vi "UHR-Fleezers Control (host) - Mau_02.vi"() -> ()   [LabVIEW 2012]
uses:
  <vilib>/Utility/miscctls.llb/LVPoint32TypeDef.ctl
  <vilib>/Utility/miscctls.llb/LVMinMaxIncTypeDef.ctl
  <vilib>/userdefined/High Color/nirio_resource_hc.ctl
  <vilib>/Platform/TimedLoop/XDataNode/timing_clust.ctl
  <vilib>/Platform/TimedLoop/XDataNode/nitl_modes.ctl
  <vilib>/Platform/TimedLoop/XDataNode/wakeup.ctl
  <vilib>/FPGAPlugInAG/PCIe-7852R/niLvFpga_Open_PCIe-7852R.vi
  <vilib>/FPGAPlugInAG/PCIe-7852R/niLvFpga_Reset_PCIe-7852R.vi
  <vilib>/Utility/error.llb/Error Cluster From Error Code.vi
  <vilib>/rvi/errors/niLvFpgaAdjustHostInterfaceError.vi
  <vilib>/FPGAPlugInAG/PCIe-7852R/niLvFpga_Run_PCIe-7852R.vi
  <vilib>/Analysis/baseanly.llb/Mean (DBL).vi
  <vilib>/express/express analysis/Spectral/Block/exnSpectralBlock spectral measurements PSD poly.vi
  <vilib>/express/express analysis/Spectral/Block/exnSpectralBlock spectral measurements PSD WFM.vi
  <vilib>/Waveform/WDTOps.llb/WDT Append Waveforms DBL.vi
  <vilib>/FPGAPlugInAG/PCIe-7852R/niLvFpga_Abort_PCIe-7852R.vi
  <vilib>/FPGAPlugInAG/PCIe-7852R/niLvFpga_Close_PCIe-7852R.vi
  openfpgaref.8.6.ctl
  <vilib>/Platform/TimedLoop/XDataNode/XDataNode.xnode
  <vilib>/rvi/interface/nirviOpenFPGA/nirviOpenFPGA.xnode
  FPGA Bitfiles/UHR-FleezersInst_FPGATarget_UHR-FleezersCont_0F5B06C4.lvbitx
  UHR-Fleezers Control (fpga) - 10.3.vi
  <vilib>/rvi/interface/nirviMethod/nirviMethod.xnode
  <vilib>/rvi/interface/nirviReadWriteControl/nirviReadWriteControl.xnode
  <vilib>/express/express analysis/Spectral/XNode/ExpressSpectralMeasurementsBlockNode.xnode
  <vilib>/rvi/interface/nirviCloseFPGA/nirviCloseFPGA.xnode
  <vilib>/Analysis/NI_AALBase.lvlib
  <vilib>/Platform/TimedLoop/XDataNode/XDNodeRunTimeDep.lvlib
  <vilib>/vision/NI_Vision_Development_Module.lvlib
  NiFpgaLv.dll
  <vilib>/FPGAPlugInAG/PCIe-7852R/niLvFpga_ConfigureFifo_PCIe-7852R.vi
  <vilib>/rvi/errors/niLvFpgaMergeErrorWithErrorCode.vi
  <vilib>/FPGAPlugInAG/PCIe-7852R/niLvFpga_ReadFifo_PCIe-7852R.vi
panel:
  out "Location path":path=path "D:/UnifiedHighRes_VIs/Locations.txt"
  out "Location Matrix":string[][](array[string])=[["N.D.\r\n", "N.D.\r\n", "N.D.\r\n"], ["0.19233\r\n", "0.00156\r\n", "0.20615\r\n"], ["N.D.\r\n", "N.D.\r\n", "N.D.\r\n"], ["N.D.\r\n", "N.D.\r\n", "N.D.\r\n"]]
  in  "radius":i32=10 min=1 max=20
  in  "clear markers":bool
  in  "trap\nmarkers?":bool
  in  "Sample Channel Flow":bool
  in  "Pump 3 contents":string="Bottom: ADig beads" caption="contents"
  in  "Pump 1 contents":string="Top: DNA beads" caption="contents"
  in  "Scripts":T1(tab)
  in  "Take Stepping Data":bool
  in  "Got DNA bead":bool
  in  "Got ADig bead":bool
  in  "Cap 1 Flow ON":bool=TRUE
  in  "Move Cap. 1 (DNA Top)":bool
  in  "Cal/Data Acq. Spot":bool
  in  "Dump Beads":bool
  in  "Cap 1 T ON":bool=TRUE
  in  "Cap 1 Samp Flow ON":bool=TRUE
  in  "Offset 2 Set":dbl=2.0
  in  "Offset 1 Set":dbl=1.0
  in  "Cal @ (MHz)":dbl=20.0
  in  "W/ Offset 1":bool=TRUE
  in  "Offset 1 Start (MHz)":dbl=13.0
  in  "W/ Offset 2":bool
  in  "Offset 2 Start (MHz)":dbl=16.0
  in  "Pause at Closest Delta (s)":dbl
  in  "Move to Delta 2 (MHz)":dbl=41.0
  in  "Attempt Limit":dbl=30.0 caption="Limit"
  out "Attempts":dbl=1.0
  in  "Wait Before Save (s)":u32=1
  in  "Fish for Tether":bool
  in  "Closest Delta (MHz)":dbl=13.0 step=0.25
  in  "Stop F (pN)":dbl=10.0
  in  "Then...":string(combo)="2"
  in  "Move to Delta 1 (MHz)":dbl=15.0
  in  "Tether Alarm?":bool=TRUE
  out "Tether":bool
  in  "TA Cancel Save?":bool=TRUE
  in  "TA Green Off?":bool=TRUE
  in  "Raster Set Upon Tether":u32=1
  in  "Save at end (5, 6)":bool
  in  "N Steps":dbl=20.0
  in  "Step Size (nm)":dbl=0.34
  in  "Save ave factor":dbl=1.0
  in  "Dip Trap Delta 1 (MHz)":dbl=15.0
  in  "Move Trap Before?":bool
  in  "Save Data After?":bool
  in  "Green ON After?":bool
  in  "Dip Trap Delta 2 (MHz)":dbl=15.0
  in  "Move Trap After?":bool
  in  "Duration (s)":dbl=1.0
  in  "Dip for Protein":bool
  in  "APD to Watch":bool
  out "Duration (s)":dbl
  in  "Action":string(combo)="Yank"
  in  "Fl. Triggered...":bool
  in  "Fl. Delta Thresh. (kHz)":dbl=0.6
  out "Waiting":bool
  out "Fl. High":bool
  in  "N pts to average":u16=6
  in  "Yank Delay (s)":dbl=3.5
  in  "Yank to Delta Array (MHz)":dbl[](array[numeric])=[16.3, 15.85, 14.85]
  in  "N Array El":u8=3 min=1 step=1
  in  "Random Choice":bool=TRUE
  in  "Force Yank":bool
  in  "Force Reset":bool
  in  "Y change (mm)":dbl
  in  "Profile":bool
  out "Sigma/Mean 2":dbl=nan caption="Sigma/Mean" format="%#_2g"
  out "Rate sigma (Hz) 2":dbl caption="Sigma (Hz)" format="%0.2f"
  out "APD 2 Rate (Hz)":dbl format="%#_3p"
  out "Primary Video Display":T2(plugin-control)
  out "Waveform Graph":dbl[](graph) caption="APD Line Scan"
  in  "Inject Top":bool caption="Inject Pump 3"
  in  "Inject Bottom":bool caption="Inject Pump 1"
  out "Messages":string="7:59 AM\tUHR-Fleezers ready.\r"
  in  "APD Ave N":dbl=10.0
  out "Int. Time (s)":dbl=3.0
  in  "Stop All":bool=TRUE
  out "Sigma/Mean":dbl=nan format="%#_2g"
  out "Rate sigma (Hz)":dbl caption="Sigma (Hz)" format="%0.2f"
  in  "Tab Control 6":T3(tab)=enum."Imaging"
  in  "APD 2 Offset":dbl
  in  "APD 1 Offset":dbl
  out "RMS (Ang)":dbl=nan format="%_2g"
  in  "Bead Sep. Int. Time (s)":dbl=5.0 caption="Int. Time (s)"
  in  "Below (kHz)":dbl=0.5
  in  "Above (kHz)":dbl=2.0
  in  "Adjust Scale\nto Mean":bool
  in  "Rescale on Mean":bool
  in  "Offset (nm)":dbl
  out "Mean":dbl=nan caption="Mean (V)" format="%#_3g"
  out "Force":waveform(dbl)[](graph)=[{"t0"=timestamp(12.90000000000001 s since 1904-01-01), "dt"=0.15, "Y"=[nan, nan], "attributes"=variant("NI_ChannelName"=variant(string "T1 X"))}, {"t0"=timestamp(12.90000000000001 s since 1904-01-01), "dt"=0.15, "Y"=[nan, nan], "attributes"=variant("NI_ChannelName"=variant(string "T2 X"))}]
  out "APD Chart":waveform(dbl)[](graph)=[{"t0"=timestamp(12.90000000000001 s since 1904-01-01), "dt"=0.02, "Y"=[0.0, 0.0, 0.0, 0.0, 0.0, 0.0, 0.0, 0.0, 0.0, 0.0, 0.0, 0.0, 0.0, 0.0, 0.0], "attributes"=variant("NI_ChannelName"=variant(string "APD 1"))}, {"t0"=timestamp(12.90000000000001 s since 1904-01-01), "dt"=0.02, "Y"=[0.0, 0.0, 0.0, 0.0, 0.0, 0.0, 0.0, 0.0, 0.0, 0.0, 0.0, 0.0, 0.0, 0.0, 0.0], "attributes"=variant("NI_ChannelName"=variant(string "APD 2"))}]
  in  "Calibration":u16(ring) items=["None", "Position", "Force"]
  out "T1 X":dbl=nan caption="T1 X (V)" format="%0.2f"
  out "T2 X":dbl=nan caption="T2 X (V)" format="%0.2f"
  out "Bead Separation":waveform(dbl)(graph)={"t0"=timestamp(12.90000000000001 s since 1904-01-01), "dt"=0.15, "Y"=[nan, nan], "attributes"=variant("NI_ChannelName"=variant(string "T1 X"))}
  in  "Amplitude (nm)":dbl=3.0
  out "Bead Mean (nm)":dbl=nan caption="Mean (nm)" format="%0.2f"
  out "Difference":dbl=nan caption="Difference (V)" format="%.2g"
  in  "Take Detection Laser\nImage":bool
  out "APD 2":T2(plugin-control) caption="APD 2 (Cy5)"
  in  "Flip Green Filter":bool
  in  "Set X Only":bool
  in  "Set Y Only":bool
  out "APD 1":T2(plugin-control) caption="APD 1 (Cy3)"
  out "Detection Laser Y":T2(plugin-control)
  out "Pointer Y (V)":dbl format="%_3g"
  out "Pointer X (V)":dbl format="%_3g"
  in  "Set Confocal Spot (X-Y)":bool
  out "Detection Laser X":T2(plugin-control)
  out "Saved APD":dbl[][](graph) caption="Most Recent Time Trace"
  out "Trap Delta Graph":dbl[](graph) caption="Most Recent Time Trace"
  out "Save APD Deriv":dbl[][](graph) caption="Most Recent Time Trace"
  out "Delta Fl. 1":dbl
  out "Delta Fl. 2":dbl
  out "All Signals":waveform(dbl)[](graph)=[{"t0"=timestamp(12.90000000000001 s since 1904-01-01), "dt"=0.02, "Y"=[0.0, 0.0, 0.0, 0.0, 0.0, 0.0, 0.0, 0.0, 0.0, 0.0, 0.0, 0.0, 0.0, 0.0, 0.0], "attributes"=variant("NI_ChannelName"=variant(string "APD 1"))}, {"t0"=timestamp(12.90000000000001 s since 1904-01-01), "dt"=0.02, "Y"=[0.0, 0.0, 0.0, 0.0, 0.0, 0.0, 0.0, 0.0, 0.0, 0.0, 0.0, 0.0, 0.0, 0.0, 0.0], "attributes"=variant("NI_ChannelName"=variant(string "APD 2"))}, {"t0"=timestamp(12.90000000000001 s since 1904-01-01), "dt"=0.15, "Y"=[nan, nan], "attributes"=variant("NI_ChannelName"=variant(string "T1 Y"))}, {"t0"=timestamp(12.90000000000001 s since 1904-01-01), "dt"=0.15, "Y"=[nan, nan], "attributes"=variant("NI_ChannelName"=variant(string "T1 X"))}, {"t0"=timestamp(12.90000000000001 s since 1904-01-01), "dt"=0.15, "Y"=[-0.0004235663930173644, -0.0004722739341410556], "attributes"=variant("NI_ChannelName"=variant(string "T1 Sum"))}, {"t0"=timestamp(12.90000000000001 s since 1904-01-01), "dt"=0.15, "Y"=[nan, nan], "attributes"=variant("NI_ChannelName"=variant(string "T2 Y"))}, {"t0"=timestamp(12.90000000000001 s since 1904-01-01), "dt"=0.15, "Y"=[nan, nan], "attributes"=variant("NI_ChannelName"=variant(string "T2 X"))}, {"t0"=timestamp(12.90000000000001 s since 1904-01-01), "dt"=0.15, "Y"=[-0.0005883053071687949, -0.0006281319620349712], "attributes"=variant("NI_ChannelName"=variant(string "T2 Sum"))}, {"t0"=timestamp(12.90000000000001 s since 1904-01-01), "dt"=0.15, "Y"=[nan, nan], "attributes"=variant("NI_ChannelName"=variant(string "T1 FB X"))}, {"t0"=timestamp(12.90000000000001 s since 1904-01-01), "dt"=0.15, "Y"=[-0.0004680013428144157, -0.0005167699209570592], "attributes"=variant("NI_ChannelName"=variant(string "T2 FB Sum"))}, {"t0"=timestamp(12.90000000000001 s since 1904-01-01), "dt"=0.15, "Y"=[nan, nan], "attributes"=variant("NI_ChannelName"=variant(string "T2 FB X"))}, {"t0"=timestamp(12.90000000000001 s since 1904-01-01), "dt"=0.15, "Y"=[-0.0006226691488387671, -0.0006504715109714008], "attributes"=variant("NI_ChannelName"=variant(string "T2 FB Sum"))}, {"t0"=timestamp(12.90000000000001 s since 1904-01-01), "dt"=0.15, "Y"=[-0.0007901852473525123, -0.0008601641895809732], "attributes"=variant("NI_ChannelName"=variant(string "PSD Y"))}, {"t0"=timestamp(12.90000000000001 s since 1904-01-01), "dt"=0.15, "Y"=[0.00031556138798181086, 0.0002525101474044007], "attributes"=variant("NI_ChannelName"=variant(string "PSD X"))}, {"t0"=timestamp(12.90000000000001 s since 1904-01-01), "dt"=0.15, "Y"=[-0.00019678334910122974, -0.0002453993346964931], "attributes"=variant("NI_ChannelName"=variant(string "PSD Sum"))}]
  in  "Signals to Plot":i32(listbox)
  out "Trap Disp. Freq. (Hz)":dbl=6.666666666666667 caption="Freq. (Hz)" format="%#_6p"
  out "Display Period (s)":dbl=0.15 caption="Period (s)" format="%#_6p"
  in  "Trap Disp. Downsample":dbl=10000.0 caption="Downsample" max=20000.0
  in  "APD Disp. Scale":dbl=0.1 caption="Scale (Divide,\nfor above plot only)"
  in  "APD Disp. Downsample":dbl=2.0 caption="Integrate" min=1.0 max=30.0 step=1.0
  out "APD Display Freq. (Hz)":dbl=50.0 caption="Freq. (Hz)"
  out "APD Display Period (s)":dbl=0.02 caption="Period (s)"
  out "FFT 1":cluster{"f0":dbl, "df":dbl, "magnitude":dbl[]}[](graph)=[{"f0"=0.0, "df"=16.666666666666668, "magnitude"=[-331.1367572010275, -79.05506245821404, -86.61411242440559, -88.4728176091699, -90.3181253945935, -94.12566333707997, -92.52740723119955, -94.92192587982518, -99.60936585245742, -96.87568627870715, -94.02570383337763, -83.8058550151726, -97.57441397235512, -101.59968530846606, -101.523049255742, -103.35038532190343, -101.58594091014982, -102.96098031851216, -91.39759462745924, -103.75019963279499, -104.45030075054324, -103.04245334279298, -104.0720279134107, -106.06482372394834, -103.69131867828104, -104.40395035115309, -105.96420043276396, -107.6735556337804, -106.673030006608, -107.34889066208132, -108.05626565233933, -106.25659018850432, -105.29934513380842, -105.43096056709592, -108.3728498841465, -106.0555440144992, -105.78001282181421, -107.48741857324953, -108.67624970548897, -105.39976667156175, -105.91413119232612, -109.4222808198164, -107.0898971593174, -107.91164191890915, -108.26032038855709, -107.58332347164534, -108.23559688234297, -108.01271040303237, -107.66511723652701, -106.51901583170391, -109.27249501469946, -108.55647681594805, -107.93499259231463, -107.05068166453935, -109.13641475410455, -109.29679733781423, -108.19360835527803, -109.57747591546632, -109.58364591011674, -110.47061433372711, -109.8144340420426, -108.79067462293897, -107.54887553357234, -107.99559866705923, -108.85023923652685, -109.68733225238618, -108.51101278437793, -108.51620475114115, -108.22212402200637, -104.63726950302143, -110.2989919678048, -107.61796444414897, -108.68882962798736, -104.79193983043893, -103.59504263746938, -93.64633660288543, -101.9191640501395, -105.73717393151816, -108.92572458793902, -107.43962662800902, -107.79595323081325, -107.0923101993207, -108.17603277205289, -107.87074270713183, -109.20899066381877, -108.61832060412445, -109.10072003106593, -105.76480632823524, -108.60877649218978, -109.67541158970121, -110.2286232768028, -109.84952155309578, -109.33772024076384, -109.95251642394683, -110.14777282585466, -109.13825677905699, -110.05989365698167, -109.39359990189426, -110.56255614635295, -109.66477183197163, -108.9397158528824, -110.26529907650465, -109.20049464984628, -108.20183857013548, -109.09752250184418, -108.00440442238454, -108.35465963524055, -111.16774134451799, -110.34812550238405, -108.94506763426756, -108.72845542102493, -109.41512344014713, -112.44661664432377, -110.35437330889101, -111.32939440655925, -109.42989530434981, -110.98084669076195, -111.92160561143541, -108.57755551751093, -111.40042616180912, -110.15284955891853, -112.21455132279115, -111.40787773511747, -108.82949641635288, -110.13442122547907, -111.42229298204664, -112.06314940885191, -110.6015308813694, -109.51144097251623, -111.15989713761475, -110.25535755335385, -109.65868178057926, -110.51649885452997, -109.77194745285269, -108.4234206864394, -109.50892632093968, -109.46471287444389, -107.92241289271415, -109.72283805386196, -108.63426821579918, -110.37316681536255, -111.09713996884652, -110.32903619589223, -105.32012665515045, -107.36858557554393, -108.00382215905725, -110.06430686942338, -108.81666625979916, -110.01277074453823, -110.94194741225512, -109.65934609082873, -107.80979136006962, -112.81333866824724, -111.61474300955487, -109.83998277184975, -109.45953946904639, -109.79640584952526, -108.19172301667324, -109.28894656674316, -107.61471301278785, -108.83814006090513, -109.08866847726084, -108.20250571862371, -107.96222236861584, -107.03811197900873, -108.93533000393974, -107.74482548035408, -110.79811544577694, -111.1387476496877, -107.42970105883512, -109.18442281176472, -108.73546184641192, -108.71800246690864, -108.51945944378063, -108.06825856571285, -107.27210712368412, -108.12304695877637, -107.84933283677306, -109.73682373154998, -109.32284761503395, -109.31328817453769, -106.68762108642842, -109.79203616876461, -109.9020278896408, -110.27080024357275, -108.54152101558762, -111.00464391726017, -112.42244020766577, -110.82707315747889, -111.00344011890857, -109.90461839395674, -109.42877207451863, -109.73549298167016, -111.67494793393293, -108.85799077901427, -108.5348443278263, -109.803781083881, -108.30644755543659, -108.5079527456017, -111.2055351312823, -108.53089994340155, -108.01739789012176, -108.70360662855235, -107.95873456794631, -109.58297170693093, -108.9372401694271, -110.15921663527153, -109.22399119911955, -110.89883651739237, -108.92840112258382, -110.0545300523626, -109.05961065387005, -109.45831398589371, -108.61239387653227, -110.13001256174265, -108.80060224137931, -109.46327400696283, -108.0177965824709, -109.29727944627197, -110.3237255895986, -109.03258262543821, -110.97880178489321, -109.70034895077919, -111.16405638194153, -109.17324451464711, -109.65698250854277, -108.96750235822178, -112.00534231585624, -108.69274607723942, -108.98110446396657, -108.40723795464795, -111.44459094807324, -111.74799245277113, -111.1601960491512, -108.92048232753773, -110.30506377784799, -111.33145973979093, -110.91850998672503, -110.33684985776448, -108.90206518366908, -109.28458878227542, -108.98773986023751, -110.85813863075646, -109.00041591105906, -110.84543686681204, -109.84382395806176, -109.69722434763266, -108.50915601095721, -107.80829925826895, -110.59736107582401, -109.75377770317087, -109.3992084496136, -110.51151565846742, -112.49753959826434, -109.7299632589479, -109.54070743868353, -109.90314341132164, -111.05974202976806, -109.03766862152392, -109.46667095459878, -109.52800799036197, -111.3163121356807, -110.07817134522178, -108.69251657453547, -109.40472158898045, -109.71400709815576, -110.60534468715097, -109.46937396724682, -107.70342491418788, -109.86331122597839, -108.64971387994616, -110.90117371097081, -108.34928840565928, -110.04172889660904, -111.52979926554961, -110.34759300823305, -109.62712781837159, -109.24131154553284, -110.23196152450447, -108.68509612326807, -108.0246905483419, -106.61876139289784, -101.5519630114271, -80.57695480953835, -102.03744443354402, -107.1449217193017, -110.0695213407169, -106.61597783999268, -110.79221011808191, -109.58974545931426, -109.1149802216988, -109.20993813088597, -109.63768480465863, -110.10428394219181, -109.08445084271477, -108.83472375362581, -109.69508502050168, -108.05588796178941, -110.62586360101581, -109.95315261676905, -107.52208264977473, -108.80708007514875, -110.43484881098874, -110.45942171588936, -107.83804717866751, -109.98973910294193, -109.3496496054193, -108.425252911127, -110.94579264380809, -108.54181722177951, -108.67696070083541, -108.4150202151644, -109.24973583101504, -112.0454922608961, -111.29046597340738, -110.75018248960077, -109.38326363603683, -109.2033340336957, -109.45076170874889, -109.52878049853727, -109.32340869724774, -110.98123395128233, -110.75736340635505, -109.7218385823809, -107.97422606064993, -109.77313701758703, -110.95948744392717, -110.08996774172691, -108.51011830110778, -109.78063140243836, -110.65996628628228, -109.83684298615616, -110.33329049188029, -110.13755118968292, -110.3717925645783, -108.55302219178951, -106.86811628734195, -108.6302156589162, -108.75341391045045, -108.32589578384841, -108.70061474734084, -112.30742263527534, -109.16842570592085, -109.29767035534508, -108.87829025017463, -108.2255616391397, -108.4316108616088, -108.82995906929271, -110.40135575415563, -109.51623498946435, -109.79409808792403, -107.03832759632121, -108.36534528684132, -109.72010868372905, -107.90933028179892, -106.95643597294047, -111.29929166165778, -110.23001135794706, -108.98838015381585, -109.79115357104436, -108.18627479511115, -108.14988122174307, -109.12074063466532, -109.41904850488358, -111.40409873721113, -108.83156790193294, -108.77032248953847, -108.88363158686694, -108.47515048290681, -105.94172147874599, -109.38146940214403, -109.21277078848794, -108.11309390545507, -110.70840012427504, -109.5504457849329, -109.52330684534209, -110.06776026911132, -108.21949434182314, -111.21266686269992, -108.78581501170974, -108.43115799297222, -109.63260325780062, -109.84070220619535, -109.72041980780126, -110.29615941882527, -110.60316734262464, -108.79165446414692, -110.95840439895592, -109.64926233107009, -109.16526769544322, -108.65292362430982, -109.56113898129935, -109.85693046339026, -108.92316027325207, -109.79492493553914, -109.38157962945887, -110.24545136266825, -109.30031463492487, -109.0795429936869, -111.4091719525013, -108.63499083917162, -108.43863465339358, -109.23207864880891, -111.21947487191643, -109.24525201480154, -109.56842406077318, -109.46711940800672, -111.91389548262572, -108.15655736690546, -108.71882059966947, -111.26328503478568, -110.95027143873176, -108.4853106242357, -110.36902802777546, -109.9314203579182, -108.77686164101732, -108.71871020068312, -111.04829661168574, -109.95072655339462, -109.88221342875462, -109.53241732756136, -108.2625005404823, -108.00677030040697, -110.19659317581693, -108.93858924796267, -109.46817875483995, -110.78063992017232, -111.11066570318451, -110.78774336696706, -109.19199744617812, -108.54914256407436, -109.28414960420909, -110.64143585101183, -110.5855350821307, -109.47578632252726, -108.89705360836223, -109.89214013612292, -107.93271261027171, -109.32631601340563, -108.60274611341092, -109.40110159872573, -110.889237682208, -110.01391165813328, -109.99747108785071, -108.65542819213674, -110.37211847668736, -110.44656500845738, -110.8128133834973, -108.8909299260433, -110.19551227077532, -111.37647266643523, -110.83802189730321, -109.98519377913681, -110.52378970770522, -108.16970420057817, -110.70974729773344, -110.76836765494402, -110.26884275594577, -109.22041044268806, -109.87809744746195, -107.76823252107832, -109.12119474042969, -110.28066108731146, -108.55000033509207, -110.18152097767907, -110.73030521152278, -111.49470908029893, -110.2320929919509, -110.03370979233021, -109.79181668155233, -108.6673501209991, -109.86695766650877, -107.88926518046961, -110.95525003776572, -109.18130359755742, -110.42618009658618, -107.90341931158893, -111.44736855661769, -110.72634267386593, -109.29945988519303, -107.67889101961411, -108.81148059987765, -109.13375212757057, -109.8122873383549, -109.80176697684155, -109.96342275204768, -109.90406635707086, -108.75674342748256, -110.12362902701081, -109.82151095527837, -108.62543344241836, -110.09171852771195, -110.21434637862887, -109.97254504855631, -109.27043209093468, -111.35149588204125, -110.12399876776051, -111.65983675538546, -109.28788875768564, -110.86554069990251, -111.26990906470603, -108.60956517491746, -111.49613890850938, -111.79685722966795, -109.26269485364045, -110.38555615546439, -109.40641023162068, -110.966136593156, -108.78892524584494, -110.29340727375603, -111.44032043281035, -109.95212021173755, -109.79233511584334, -112.41184021118175, -109.73687851881148, -108.65493879781806, -110.76132988919045, -108.43230346094671, -110.32968175895853, -110.29890782023821, -108.77609076424456, -110.3298662333555, -109.47734504217333, -108.2677295732245, -109.21234363352882, -107.83278941978479, -108.85136784424789, -108.43241251530755, -109.76609391460555, -108.53204373005357, -110.9660641972934, -110.3152512161094, -110.72570499399905, -109.23877906286317, -111.72407743101837, -109.20311421918561, -108.06021800233717, -109.29288625761943, -108.78395253409145, -111.85250172876302, -108.78827588901797, -109.79775055719482, -109.12089297455859, -109.49896359356035, -110.34432647103819, -107.94700097960238, -109.30489238477631, -108.89170290869342, -108.82574563272509, -110.11024077194833, -107.37946433552314, -109.60167933458756, -107.80625057819019, -110.11489057210264, -107.35436859378505, -105.69819484613895, -109.11280625683739, -109.27770293057978, -107.7053735252589, -109.75022444894368, -109.3310543596577, -107.87683693707739, -108.19931495338068, -109.26462246191564, -106.71885779297867, -100.00018022217961, -92.54434511397295, -107.20472143807373, -107.39203415155283, -110.04461177268398, -108.48860496315312, -109.0057168110333, -108.37627790492552, -108.4108380728248, -109.65509454313073, -109.64243000632982, -97.04219069306761, -109.0928856629964, -107.9760697315632, -107.52611064047497, -108.87702814778996, -109.08437599027614, -110.70097118837974, -109.00969860961283, -110.38275386163214, -110.0699155421545, -106.91498895181175, -106.22178738309017, -109.36827866896039, -107.59953130968307, -109.19516217272808, -108.31502495393616, -109.384158926223, -107.11670654202719, -108.09436312738853, -110.14559230873704, -109.84997663447679, -107.83465335309926, -108.60947100624459, -108.9932479423645, -109.17174810371898, -108.79457339828916, -109.40909327982367, -109.6328723628302, -109.51081854476179, -107.63054408568418, -109.63728404010122, -108.51163794839918, -107.55002282725216, -108.97796212764939, -107.24648164623483, -112.21470452291085, -108.74294024554423, -109.62070777514892, -108.05768666239368, -109.8224946685739, -109.34575507446003, -108.53536952609525, -109.60789300457671, -107.56681538208278, -109.22777325016398, -108.79047910308894, -110.10332477250668, -108.00206387955672, -108.45604004720035, -109.00645795765472, -109.81039564269616, -108.92785144634745, -108.3978471520567, -107.94411095685999, -110.53486519304262, -108.8773780319227, -109.03345093296107, -107.30746693745031, -108.54277704832029, -108.77629108166091, -108.91111762599647, -107.74965195880401, -109.97375370738439, -109.76326492689246, -107.91717581777407, -109.0730556927617, -107.66804873204664, -110.40438871064791, -108.05794247751498, -108.80206615156494, -107.51329354700796, -108.83687012994949, -107.57713176895379, -107.94774159581414, -109.41894615439651, -107.10869425078764, -110.51480854078629, -108.92221367099775, -109.91358786461535, -110.1744263092835, -109.30795472883494, -107.91359710691006, -109.77888185049835, -109.52060975706438, -108.66686651982212, -108.71041801553639, -110.13619546359467, -108.87957097273856, -109.72150387215271, -109.00776068810654, -109.70251113927438, -110.75769213896399, -108.53234896741436, -109.69439526582246, -110.15412541604617, -108.25183374628219, -107.97402569656481, -110.34920156998648, -108.45106995186384, -108.82031145748209, -111.38690005057539, -107.01968459818563, -110.3044500039584, -110.8755481852125, -111.08915057663255, -107.94824988655199, -110.21669144934839, -109.90539774633154, -109.58985438756767, -110.12258796623348, -109.41689951612143, -109.31128210476795, -109.00258476567323, -109.11093063041056, -108.83347064311234, -108.32685287566952, -109.44770946560935, -108.40145063144861, -109.68448193892085, -108.76525439243828, -107.62837139034596, -107.39300298848994, -109.36993934990318, -109.2465218489418, -106.66307369796812, -110.15891092764934, -109.57151745419041, -108.92425698310808, -109.8036704717834, -108.79751146756549, -109.25926431818017, -108.46260574057584, -109.1967554647261, -110.63319560262356, -109.02343067385144, -111.22073171487528, -109.4731095097105, -109.69335000085164, -109.48782989577005, -107.95204227683271, -108.19468255763758, -111.36195112053247, -109.55696116543685, -110.3130767640534, -108.9621824253354, -109.99735074896789, -109.20198058456344, -108.12100614259485, -111.27227490807289, -110.09248554008288, -109.14395535060149, -110.80882692379708, -109.22632926901655, -108.64497210802793, -111.00030482190711, -111.1317849358033, -107.43140429257826, -107.9783302193555, -109.2639893652291, -108.97008485446163, -108.66556668859064, -108.12995785876932, -109.73001061107855, -108.09691302413727, -110.68391499215569, -112.78583642012705, -108.7093037763389, -110.67868795924797, -109.0190959349128, -108.36247198231372, -109.82829353258869, -108.24916379311045, -109.84154533905823, -108.55470160833775, -109.75438989348815, -108.82865632118325, -107.63622268162582, -111.00943492886312, -110.81824358463759, -109.46028423652966, -107.52479398900992, -108.99087806823736, -109.94494831750349, -110.26788355564504, -109.8954055022304, -106.9478122391182, -108.91705388158901, -107.76095584490312, -109.28456723055147, -109.7982307261767, -108.98552661346622, -109.98937979783426, -110.57907422426224, -108.68113463944836, -108.06257240208589, -110.0707224529617, -109.19515280354733, -109.35868842818849, -110.37311467065695, -109.0404734478992, -108.16686395270187, -108.61859220485148, -109.19986437876149, -108.19707189725302, -110.06564239663074, -108.87850403465154, -110.63824157544798, -107.36918104067212, -108.7008736325543, -110.9359398265406, -111.08529123080929, -108.44209934821818, -109.79529621208783, -108.38917887958179, -108.169117639508, -109.24332926356216, -110.50584058811704, -109.63592524002665, -109.32261039377495, -109.16720880524552, -109.3084314664462, -109.5812223978583, -107.70213196487856, -108.0557884982431, -110.67058020007828, -111.68459781023608, -109.66270627185824, -110.52536245663693, -109.70208409132103, -108.78645420809342, -109.23122088059863, -109.24601474121832, -111.25604763816514, -109.50225851581177, -107.32434217163818, -109.28548556764925, -107.59972621660836, -110.46928774723048, -109.25950101547609, -110.32016453935465, -107.78482761561703, -107.89462895091089, -107.51366154391481, -108.08036891159172, -109.53371809947035, -101.2452927166745, -109.32763325689056, -107.52166868423687, -109.89648659445174, -109.11350200980485, -109.81336712738089, -110.02799517445062, -108.02767143538516, -107.97850220501483, -109.50772934896838, -109.31069875721964, -108.49991657749598, -105.60880911233095, -109.79128597340213, -106.91084537903113, -107.84880087118997, -109.63628170511824, -109.03203967193224, -110.64186113413658, -110.98027990365594, -112.33841002907062, -111.01793075565425, -108.58025797022215, -110.4259296883756, -110.38643255981424, -108.93051671115133, -110.97544177116494, -108.63883100482677, -108.37581711765226, -108.90240163126536, -107.94688047875466, -109.9482937437732, -110.09097112364414, -110.09805032265376, -111.44307114024532, -109.15483789122554, -110.9713708217832, -107.8548737634672, -111.41418477109195, -109.45699779859628, -97.03595099331734, -109.16746744169623, -109.66209204485918, -112.57048704774604, -109.73989735035725, -108.16252575067017, -110.7546980664636, -108.91536673403449, -109.20509151422344, -111.0260632167785, -109.62924582406518, -110.45466277291722, -110.2973970018937, -109.67550222925419, -108.84481022020094, -107.23686414357573, -111.79004633370906, -109.85453094194085, -109.45617270081004, -110.73920606732504, -108.90879956851099, -109.67774425528265, -109.4745715721361, -110.18080454693559, -109.26079184315502, -109.41692499885505, -109.02240975088358, -107.80833423058168, -109.32657361431549, -107.87138278655101, -110.910364670719, -109.70067156846706, -108.55301754282077, -109.4243252157005, -109.77567725161107, -107.83737232063925, -110.36509412773016, -109.6371048811367, -109.49430894422814, -108.55509251499753, -108.03996302911446, -110.4385715838736, -110.08864436068788, -109.48922484379962, -109.90865554258562, -109.7491963238264, -110.04796094537969, -107.413043439116, -108.54229076126079, -108.2522516728666, -109.75464941327974, -110.26795832300996, -109.28073673851144, -108.62990200974927, -109.89408067552287, -109.09160284731726, -109.90740624925795, -109.92534708896517, -109.79578862362752, -109.97278346890566, -107.80679350393824, -112.81728446281548, -108.09689504419987, -109.89549991422173, -108.43930976031248, -109.95153099843282, -108.18277483720716, -111.89607792605433, -109.52567003805, -109.17125106979698, -109.64300739407085, -108.21045178846524, -109.64036472149706, -109.02324448538845, -109.039163008889, -110.41006510134076, -109.50289952116489, -110.4732620447796, -110.08777181504614, -110.15589511434341, -109.55705089158471, -109.2547682932589, -110.86823885471617, -109.96330502176939, -109.85995369810554, -110.63211290903473, -112.08007783432191, -110.24725218052279, -107.62861148917592, -110.08691795849435, -108.89793794632287, -111.07702220466341, -109.46946126482341, -109.19747345337464, -110.70018609416007, -109.66366205691908, -110.78032312133551, -108.05724200456513, -108.195661625627, -110.90724508408255, -110.08307674771669, -110.76863516643007, -110.46620425061583, -109.16986788877276, -109.61921294239114, -108.51159432329543, -109.96308336765689, -107.38178944242856, -111.95930944846394, -109.3329826827624, -109.59119636368249, -108.83148571828912, -110.46194288788257, -105.87694286145472, -107.985886302892, -109.2975019660806, -111.05138725716857, -109.60005889204612, -110.92871351729086, -110.73480546964537, -108.41587420326718, -109.84275465824477, -108.8249071047676, -107.65358887817105, -108.3254150042995, -111.47362100321767, -112.7287536850025, -108.8217125660507, -109.50232320231771, -110.29587061625348, -109.30644535112089, -107.69178032077258, -110.84522325672016, -109.3735891463141, -109.12506388923123, -109.65582307934665, -111.11427272192576, -112.19827973435466, -109.11306367925813, -108.19203577968261, -107.89831568266465, -108.85805249169313, -109.51100049661844, -111.71546684086955, -109.53880495724334, -107.07739286222231, -110.66836728754211, -111.5415170557177, -110.16051267940297, -110.6107546662698, -111.36389129556191, -107.77888179117923, -110.34160392509817, -109.61287125994414, -110.23791773883013, -111.00669159903549, -110.97165069538953, -109.43965413392434, -110.6813161690388, -110.31441293654314, -111.96129906273796, -108.15998218707462, -110.08095912053633, -109.41084567452768, -109.28774416263552, -110.80159950384204, -110.41956747809755, -108.85005186267244, -107.9069227847757, -108.84249369063123, -109.92569208845894, -109.34109797584448, -109.41334788055491, -108.76462023086997, -108.22069272136177, -107.0786679601274, -108.30206755098202, -108.57613406368954, -110.83330887636482, -111.93966942736989, -109.76373713473264, -108.25782074884941, -108.16490627215555, -109.93351470267982, -110.75525684428368, -108.22814762283093, -109.73442331991602, -107.53145627482685, -108.27195221226805, -110.33032779278457, -109.48951857415828, -108.12599093700939, -107.97627415508097, -108.81426859968796, -111.21764717894752, -109.80856212352333, -110.92658779118501, -109.71551885834796, -110.38682741010847, -108.87671328341361, -109.68368600774755, -108.35359806351899, -111.7519400010676, -109.89407081573103, -108.24301180922755, -110.00646944788126, -108.6685299083706, -107.52856885980722, -111.7622363038509, -111.0025144494897, -108.64719599357296, -110.62968467177518, -108.821509935539, -107.94915453463719, -111.53070432277694, -109.87282048586256, -110.71167589371663, -109.79225006081626, -109.96203471712074, -110.29921092232489, -110.10644439440416, -111.28815007382043, -111.19165661703703, -108.46024117100558, -110.22528296512183, -110.32184972386672, -110.05120383416072, -109.78792549362107, -109.00355659956696, -108.85989369286315, -113.00899556732638, -110.91756826567867, -111.25016866167897, -111.84225040552181, -110.54451635944174, -110.72722829912917, -109.60759702177283, -110.49362602516815, -108.74419542915284, -110.3379671069179, -109.66259088220754, -110.45956400953156, -109.13956157147233, -109.27130155486806, -110.83015602667983, -109.17970724944131, -109.09662765889193, -108.0447366108107, -108.9536269357457, -110.35663108940085, -108.73418835472056, -113.42965806805827, -111.81270536656905, -110.06155590173537, -108.76582224646269, -106.7488061675813, -108.5700320158723, -111.11038264410035, -110.41435767488723, -109.12763443489911, -109.30517580756394, -111.61251165371237, -109.8116632664339, -109.36845864976851, -109.00390009629231, -110.54359197165573, -109.52629258465976, -110.75932197632896, -109.50903215359567, -107.42652056246085, -107.81146496533543, -103.22224383145215, -108.53803076819163, -109.78623360072066, -109.66306634612869, -110.80245829141279, -111.87835085452016, -102.27372781471168, -111.27763038431458, -108.45838423437681, -108.79077917058028, -109.31951755762685, -110.05415097017186, -109.5535934823387, -111.62732254641111, -110.73478247119641, -109.9468722686683, -110.39698367573979, -109.30612942398305, -109.7578384694043, -109.34817295524313, -105.56944757301993, -110.1940418750125, -109.27076023513962, -111.03491935225027, -112.2980497521063, -110.65725497955563, -109.0567530102422, -110.31700596563523, -109.64508026365678, -109.6190471404421, -110.52566833759428, -109.68595899227789, -109.7431160985074, -110.4798230300751, -109.45506977604765, -110.69504157940786, -110.63067849573177, -108.06456949500138, -107.99354148885966, -108.11349194720599, -109.15944121207349, -110.61766925164031, -110.14145801314527, -110.67420842201165, -111.91532881806512, -112.15901550030345, -109.94774413630104, -109.2819568305201, -110.94623189179737, -110.17685430287735, -110.39082916961016, -109.53953238698966, -110.76940623620611, -109.89327922318515, -109.10275695043765, -110.21445972656734, -110.58968777252528, -110.57016757660259, -109.59208496373341, -109.07946946465374, -109.10762003745964, -110.36892993974607, -109.81864495218393, -112.12972189864566, -109.26185849434863, -111.56305819991357, -111.36019621828058, -110.3397604159226, -109.58675612753163, -110.58041217474447, -106.34739062044932, -108.6722699609389, -110.03906060709869, -109.16794717548382, -109.65012481802809, -109.35377624077988, -110.51889143862303, -110.03397458059777, -110.7981307056636, -110.56653507062292, -107.61367005067231, -109.99279736988825, -111.79875182878175, -108.60382315996031, -109.71381533228038, -108.60388131505613, -107.0933685540362, -107.86037690830757, -108.40980028847238, -108.83869602763895, -110.76921375395764, -109.96766364716046, -110.8256171465781, -110.13805084291067, -108.5349140035878, -110.57158437465219, -110.8920694413417, -108.71646695477324, -108.33274238445665, -108.96152108305608, -111.03750932994224, -109.48915027983756, -110.29725207211165, -110.79527247268442, -109.47969936716117, -109.79306701834035, -110.16840035577498, -110.29840230783668, -109.15306387075587, -110.72651274964761, -109.08881658764956, -110.8349724030761, -110.64653625576447, -111.40392562616867, -109.94581588927414, -108.85136340231294, -109.77228546607624, -111.48297395390018, -109.7334001251941, -109.30537415590783, -109.63937411233408, -109.69785848648013, -109.3523781030017, -112.04667421182404, -111.56311816195343, -108.18548447362308, -110.63388993686104, -111.39768634137992, -109.87157345395542, -108.6734208287271, -109.46213300216168, -111.75774769437145, -110.10245994173216, -109.52385139033495, -110.96513097775451, -111.8709319163154, -111.54948269614047, -110.29760900080463, -108.52168175904663, -111.09033925738258, -111.14752744054172, -108.83074523709202, -109.05704141259113, -111.74377805749482, -109.57200906899736, -108.84121318623825, -110.86657990204343, -109.54363603755047, -110.89448416316372, -109.58965570570145, -110.21012263847972, -110.4063470702923, -109.5021950342969, -110.33648801598177, -110.90551031296536, -109.69205870504638, -109.8648503154861, -110.28183391384131, -109.65970942950766, -108.43615680946908, -111.11790511866548, -110.89043476451553, -113.64898442872548, -113.08004494963895, -110.81525412051718, -113.91009875719509, -110.95802128672312, -110.40944585634135, -110.33464695414992, -109.98984645778987, -110.18795067005652, -110.62364351231234, -110.44029833291248, -109.01598585569788, -110.95430216511514, -109.77987141110621, -108.54452361812068, -111.41780266439777, -110.47172771858405, -109.06084635984516, -109.30794593246578, -108.8764083815745, -108.18222749506985, -110.31330487887435, -109.04176821738014, -108.8558386035048, -109.47888284507395, -110.01459604573937, -110.48596659065309, -112.6781342298378, -109.85522803775775, -109.0569534499285, -109.08991286548698, -110.89485727880403, -109.18715778948663, -111.50381433568144, -111.3545424730884, -110.07710926239977, -111.99977850157067, -109.47444853853723, -109.81605328527645, -110.74995213151195, -112.56834665925544, -108.52052472391404, -110.89121213995557, -112.02004142355113, -108.66413739656008, -111.10053848695652, -110.41241079991636, -111.80152991764473, -110.21746151515111, -110.63265128607344, -109.483042128511, -112.78639954059729, -109.47114195846122, -109.23309637902875, -108.97133643967169, -110.08909147812822, -111.01105271457081, -111.18602432128249, -110.04633990216801, -109.53453538673071, -108.81939452082017, -111.13486114285661, -111.65877073200598, -111.63763706753498, -112.14107810664572, -113.6231865196724, -109.31743865878806, -109.18551713085722, -108.74951309653638, -109.28206426212142, -112.36687029711229, -110.10933061193728, -111.29501093502684, -108.19021080564794, -109.34497312126749, -110.37228033937312, -108.63277512903049, -110.61033993911002, -111.2975761598062, -111.49780004751436, -109.91019436685814, -109.32789992989028, -111.4482538110117, -110.1538439123475, -110.66347034043578, -110.05055133068794, -108.53002033538341, -111.7522199783972, -113.49108651193104, -108.03793940563418, -110.07108694011555, -110.83958739865201, -109.62805629409038, -112.69637731014087, -109.57996950503268, -110.104850643722, -108.83376203949506, -108.69400304840181, -110.59434352922563, -110.69121011800921, -110.18694553784364, -111.90598571547098, -110.30230802494223, -109.66810649416752, -112.6017099000434, -111.00296745333219, -110.64462650261785, -111.4775358707403, -111.98753241268494, -112.26574909791167, -112.04796822399412, -110.65853064447325, -109.6623218025264, -109.40559579075378, -110.42174451813142, -109.18991987957241, -111.02050178263048, -112.77950487440032, -110.42443751566815, -111.35440372400903, -108.5263524245987, -105.07498063939795, -107.15444425741984, -110.4508720018025, -110.25163264819463, -111.1383261104107, -109.91171620173931, -110.52200560606038, -110.5299174299573, -109.34628087255733, -110.26101817411786, -109.65071853372183, -109.66953335961068, -110.83590602054682, -110.980546313788, -109.4110066989163, -111.47223607390256, -110.00281523859483, -109.4088722967626, -109.00401922839337, -109.59655302543185, -109.7359970854586, -111.46016206343049, -110.23478747568004, -109.29441275295858, -109.82941912510167, -110.43088525283673, -108.21649744751299, -108.70220592702613, -105.2334473604296, -110.60620657984927, -107.97533820921146, -110.7664079806058, -110.56406610911355, -111.76465470250328, -108.84172809688911, -111.03661078143631, -109.85351980370237, -110.70091167176791, -109.52380717508088, -108.4356492672842, -112.25498760397127, -110.69648730540193, -110.36748838594507, -109.99090797924349, -111.2678642544111, -110.42541694325627, -111.4575545259775, -109.3211175669008, -112.7465573314208, -109.56208667784249, -111.59733497772172, -109.42295730962105, -108.55804089331346, -108.71397903286748, -110.09188290952392, -108.90810063278326, -110.31333217069538, -109.69794714542728, -109.06210020835357, -112.42465112160288, -111.74630553904855, -109.99304310093493, -108.93867687355595, -113.1669287525049, -109.09193568851137, -109.27500368450697, -108.99643325722404, -110.53962759110647, -111.2052088429852, -110.05855563908841, -110.30763723153481, -110.03411001268613, -109.6161415052669, -110.6304714466923, -110.17116005754627, -109.0753171640551, -110.92564270851628, -109.60831770517053, -110.25913363817017, -107.76644895378317, -109.2619309023068, -107.64198246311884, -107.37056168314048, -107.31978563121643, -107.68171928702894, -104.57515288104209, -104.75187637758803, -105.27246893266054, -106.96524396060869, -105.93920355631757, -103.66449995825586, -104.08476660009461, -104.53081578265315, -103.0148493379086, -106.74751670818362, -104.92309629919443, -103.98320340724693, -104.81633219413234, -105.77996356028235, -107.12559309216644, -107.28196039053535, -108.84583578337953, -109.4494696919565, -109.15525441177898, -109.7634811359225, -110.79433338587495, -108.44440079452527, -108.79597700117748, -109.98590735173822, -110.72144284267539, -109.30550753718086, -109.70072152916897, -109.65801130162137, -109.65949265997646, -109.82238573025273, -110.30669821947491, -109.83394128869384, -108.90433312205332, -110.664046708231, -110.39926453734134, -110.37725911098757, -112.12508639032839, -110.26795666332589, -108.98741993218054, -107.76168841100478, -109.82334992872889, -110.83516363498563, -112.60649745671253, -111.1960726449926, -111.03919163866381, -112.05129034965563, -108.83187987662883, -109.57240688505179, -109.32857861150738, -109.54934849013647, -108.29359879300195, -111.5179112931669, -109.52702486426027, -109.95429980789645, -110.7011078611564, -109.43204524997455, -105.56031249677113, -107.70609254346495, -108.78303653454363, -108.11457060956113, -110.44215460317537, -110.78267897406572, -110.33119812901934, -109.34449539666907, -108.82636558484161, -107.1834151347969, -108.83808254322192, -108.2542825327446, -108.80298057862501, -107.59922121598055, -108.9131916496929, -109.51519107961856, -107.7704986323755, -108.79678029009878, -111.13791068210752, -110.402746275919, -111.31702623823912, -108.49812727557243, -110.63723264798182, -109.32890666586829, -110.29721723278237, -111.66560929315017, -111.04227698307153, -111.36927505376269, -112.5203298417673, -109.93967930487354, -110.14533835678606, -110.3868348991775, -110.85413569165249, -108.44519725537315, -107.93391978795047, -109.82778679299085, -109.79311153223738, -109.25261055399044, -111.47738679135526, -111.11775495397512, -108.65898844492045, -110.26505495390529, -111.02017977446526, -110.34817965403467, -107.55161094495372, -110.21667403085983, -112.43970497917284, -110.70535338255132, -110.79438078890512, -109.81809822502822, -108.99167960596515, -106.5556893069368, -97.51736665041192, -105.29926513345109, -108.72453297392224, -108.23203912463346, -109.50324111400698, -110.9939986929772, -108.05367524487318, -108.37339392211176, -109.8553291283933, -110.46179639493138, -112.48795697163695, -111.88145079973545, -110.8678969738583, -110.62677605624849, -111.83824818603244, -109.76798658735359, -109.6654742351465, -112.58543522753767, -110.3406716250781, -109.55013159400883, -108.00481229232405, -109.90793236599207, -111.28597960985334, -110.54144527494444, -110.14704702870655, -111.2652554338908, -110.97520848958668, -108.63647576273343, -110.52472680617548, -113.16137826273847, -109.62457037485827, -109.53869420402964, -110.71399284283449, -108.55435337782664, -108.09492728294455, -112.2373886856363, -110.3693019226993, -111.65116752865308, -111.3223986412311, -109.67734725401074, -111.36420709226297, -109.14293108556625, -110.5982939020188, -110.29596476096043, -112.69847120697035, -108.39052787054206, -109.06205229490357, -110.00045399262885, -110.71775009467346, -110.69530760167493, -112.54144940754935, -109.55755373438097, -107.88943697845929, -109.98578587243783, -110.14202980613851, -110.80051915904802, -109.11327182471621, -109.50637030500913, -109.77023677605327, -109.98552825925917, -110.40235854896, -109.37603004890141, -111.36989177909379, -110.8399811877331, -109.30394670937987, -112.2769814990538, -109.10893172594731, -109.17733972841754, -108.35968166480572, -112.64492569586005, -110.13779257328873, -110.64439690778532, -108.45446935516622, -108.97325006911116, -110.54637968933774, -110.66412364132371, -111.38627695224784, -109.8942998516069, -110.36392017322382, -109.92355133054227, -109.61886697310419, -109.71969465343778, -109.85627196259388, -112.1407808286419, -111.1013489416651, -110.70428953307596, -109.3454280179969, -110.22984684615578, -109.53826801613613, -107.83673208330934, -108.72742563398342, -109.5745872123195, -108.83031823548816, -110.89059911076627, -109.87842545384129, -109.21980161063786, -109.07140273870678, -109.04628915564135, -108.79255665097845, -105.20875397856382, -110.0838008881032, -109.68293832806683, -111.24644641302518, -110.01257579497496, -110.99281477454484, -108.99296184719546, -110.96495665514604, -110.70404386182749, -108.25078498739035, -100.77667501455139, -107.61479263900088, -110.06600976399395, -110.02035637581871, -111.45524052052504, -109.975541184397, -111.07333860975358, -108.4808974233161, -109.59513524582242, -110.74711589861774, -109.50005300854993, -105.23071652566294, -111.81094849223531, -109.0168079712372, -111.89029991620679, -109.90672274216391, -109.30959446424889, -108.23718655264584, -110.10868108588909, -109.21139771899594, -110.33333323577992, -110.25792318324204, -110.67825932924109, -112.33148517950511, -108.9724848367048, -110.78371843797613, -111.40913868573313, -110.2930522718577, -111.9538408094371, -108.63639312641844, -112.4462941079034, -110.40266356498321, -108.66617580940074, -109.44306834729083, -111.08962916641603, -110.52132608161017, -110.53757698855654, -111.5587344449704, -109.77722315102946, -110.40060629757771, -109.45395807961631, -108.77558572395142, -109.0151938598724, -109.80739619986889, -108.9332873172888, -112.49933978358132, -111.28667321897437, -110.40629082858706, -109.9829216820938, -108.85102919990373, -110.84179127037925, -110.27309817549309, -109.88857884367955, -112.24517967927224, -110.23377125710859, -111.26951227953063, -110.09782138347559, -109.77508406986834, -110.55359722398646, -110.09534729906368, -109.96333904888587, -110.29372855476366, -111.36651812163072, -109.97141184588116, -110.16701683369045, -112.8562627359291, -110.66651146857079, -108.78873821095968, -108.59208174618087, -110.31784275318834, -109.43177042415276, -112.80272887161644, -111.79874205007107, -111.08216899537892, -110.73699224045636, -111.04738767291953, -110.43395896705012, -111.62106163510778, -111.32599933330843, -110.29360981749807, -109.66562228449096, -109.21316193790335, -110.06363162177448, -110.54480468587292, -109.31791670875509, -112.65386492377107, -109.91857609999171, -110.57233605624137, -110.7597333064856, -111.49767138733276, -109.36548654843229, -112.34145274183716, -110.52831153822652, -111.55802243871352, -111.81399803046556, -110.17680125962372, -111.23811621944807, -110.48042049674514, -112.43786993562033, -109.56507357271987, -110.67030752598993, -110.86377249100713, -109.06001892813467, -111.37023727930494, -109.52881096984436, -112.95107295160436, -110.49467818026214, -109.29804210589607, -109.89270706931751, -109.46354468058833, -112.10350702955014, -111.06083529077077, -110.49996587015904, -111.1617248913634, -108.84725633199014, -111.42852695852422, -110.01433866707184, -109.11616968390972, -110.76961079765468, -111.80403513904453, -109.84442686379181, -109.65447921666167, -111.3378640555306, -110.8882647652338, -112.58014202075226, -109.67128881545659, -111.73429980763389, -110.82258070774773, -110.71895931098041, -112.5117489008152, -109.16182299471309, -109.71651258790612, -109.7770618808562, -111.94294809571427, -111.1629115541574, -109.57489224865171, -109.8402445779754, -111.17931450307283, -110.09045865447595, -109.23658206733491, -112.54929616847242, -110.5150381158864, -111.32296447909377, -111.64472156295191, -111.65832771066007, -111.03359562742956, -110.85303206770837, -110.80655337650862, -109.3712696310075, -110.57313454785879, -111.18525355670417, -111.67423695430561, -112.00829831274282, -111.08915434609605, -110.3298290221436, -108.68552957386795, -112.11377370993225, -110.80288297661977, -110.33640536217185, -109.5907971201988, -107.9195263775506, -108.50223113159429, -111.91191347156142, -110.29585599512956, -109.50902788911351, -110.76819145749467, -108.86899533416589, -112.09963049260891, -110.13374376572433, -110.15881393584463, -110.87392107947531, -109.18658540731009, -109.72734703956934, -110.18732487568724, -108.76554115185057, -109.94122289815374, -110.39583285609643, -111.09540935727229, -110.6618176357367, -111.6281345666718, -109.69686483639367, -110.31633402076315, -110.61246951748903, -111.73300235294965, -111.34221378834899, -109.46708370903485, -110.70412671997354, -110.7007891485379, -110.31685483435038, -111.03016917417074, -110.94517365625376, -109.46580797053619, -111.20935248224806, -109.20661126636224, -109.50147037097533, -110.14241781654353, -109.8510950344643, -111.3794198224028, -111.28966889207122, -110.43347441663424, -109.86759980279523, -111.92101892013198, -109.31594011390644, -112.92253433794441, -110.74000829597605, -110.3690783911604, -111.9386136764295, -111.04196305034188, -110.41800427558245, -110.94287511448232, -111.66035388807579, -107.53723747644062, -110.68014818358719, -111.86628806511304, -110.12097497430523, -109.69880468221378, -111.4312783987915, -109.18240866486639, -111.45649839248873, -110.1242345454651, -113.75911576151633, -112.71747598882953, -110.9614554157337, -110.92294419716129, -110.87229098694876, -111.09943759113875, -109.48107247947176, -108.62783006742795, -110.8108025857779, -111.63342408317932, -112.0221522906341, -109.96411229549527, -111.29821085030613, -110.04566676239914, -108.41674583097112, -107.50256474992416, -108.68086611003493, -110.3738906060137, -108.86763212826641, -109.81681043446049, -111.04539822346567, -111.73290882980949, -109.75238769150758, -110.55268275367449, -110.48423701377924, -112.1116140908134, -109.53952175199518, -108.538611608547, -111.3788321484912, -110.36378736224961, -110.37712171023523, -109.82150687920334, -109.17046632238393, -105.1169578108227, -110.84067642540583, -112.91626789016587, -111.32030958133453, -108.93375913686056, -112.44450956563915, -111.1596840012794, -110.17380444915341, -109.634859036508, -110.68819277718731, -110.0648098825346, -108.87385575091399, -111.99676414571755, -111.32585405719519, -110.59892045991457, -110.32589048340424, -111.1172696292077, -109.79946399891651, -110.10030723919304, -110.71841081343656, -112.23013150012054, -108.94400401141407, -109.71044551701596, -111.77560214164039, -109.68779520039777, -110.96119601299907, -113.66477058855787, -110.17794649102234, -110.30159876509862, -110.11953836266514]}, ...(2 in all)]
  out "FFT 2":cluster{"f0":dbl, "df":dbl, "magnitude":dbl[]}[](graph)=[{"f0"=0.0, "df"=16.666666666666668, "magnitude"=[-324.19011195451765, -78.1272953812706, -85.85545438627958, -89.30587144190069, -92.90590394398903, -93.63083388385274, -91.8644929119412, -95.26924857401164, -97.0710469181336, -98.01148078956652, -99.33043660296804, -95.58776817681839, -99.9570097527269, -101.45494093095093, -101.51838334751548, -101.00386616525799, -103.01963069818913, -103.20223925731209, -103.53783076500916, -103.48065647812659, -103.97797518531912, -104.58942778240602, -104.46991277190502, -104.59813972158683, -104.56685024229951, -104.69893799348945, -105.05669000016238, -106.17061117835001, -106.43303821862656, -107.39468286383597, -106.2899368267905, -105.7863846168199, -105.17170638885071, -104.53818172761852, -106.70340956723133, -106.55444321137247, -106.67654843051936, -107.79888413750199, -107.86424326005849, -106.09722609215336, -107.71648639013972, -107.79500725395155, -106.17330953637067, -105.43663624517525, -108.04970689199158, -109.92106271611999, -106.2505251183406, -110.60221373795562, -107.11377887451098, -108.4126937286195, -108.37794745021417, -113.22457316369011, -106.38281814065472, -107.55385617652075, -108.93026538982782, -106.19334142366085, -108.90462602264525, -107.63084712174981, -109.12192537022624, -107.90627042480016, -109.44472079190832, -108.91731458372392, -105.74102972706788, -105.74407510394178, -107.5989477192235, -106.2838630137392, -107.46190542725505, -107.38881299750702, -109.08024783239452, -104.97871836903269, -106.65424712290651, -107.04966019632134, -106.16202578092883, -102.98374199247179, -99.1568704142098, -87.07383781389657, -96.41471411313154, -102.65176579899618, -107.65674867775193, -102.85397890306213, -107.58658613411464, -104.79044898833125, -106.65282019869865, -108.65027966345534, -109.46169054950127, -108.69969979291741, -110.4048706652988, -108.81020193837274, -109.42808902484134, -108.85398463561398, -108.3849716744813, -109.1844457168716, -109.32787859535676, -111.01992124870878, -106.64843449415699, -108.9926343573667, -111.59837822080355, -110.57121677672183, -111.17280164669164, -110.68901970586144, -111.69013245592781, -109.90200577018311, -109.3554172126163, -110.7515368822992, -109.2863324212524, -109.66209701262974, -108.50795548698007, -110.58126481096504, -112.36093896766921, -109.78612141282203, -108.85120530917233, -109.91424431080952, -109.84698632196245, -110.93960894966105, -109.77214706089354, -110.30762971422381, -108.77791302937449, -110.79522659679036, -108.47242514643455, -111.20629758187835, -109.05996769621125, -111.13574821570619, -107.79388178889101, -111.5768481279296, -110.52058839597171, -111.58729762739313, -108.99000864386126, -111.6585121505227, -110.50715371958135, -108.87151956974363, -110.30486244367107, -108.32392040018144, -108.1769507919999, -110.43198471512189, -109.81454097966842, -110.26717009815644, -110.82924135076777, -110.34103661156989, -110.0692667126265, -109.34555682020833, -109.1694484721415, -109.9940980324044, -110.81940616215803, -108.21162003366862, -107.97087538330561, -107.55312461506225, -110.60339321606872, -110.09004629292225, -109.05860430198882, -113.1412749514818, -109.81628200948371, -108.62343219429849, -109.48172424209761, -110.85978755785311, -109.47778611557064, -108.81728552967951, -107.47864241666747, -107.61735128422292, -109.62511618983821, -110.32417726356636, -108.24287897478176, -108.60460879530194, -110.2181558494026, -107.95550802888957, -110.80234484950323, -111.09955733353904, -109.43923052503506, -108.98949130235951, -110.05778199870154, -110.36224432927585, -108.13523430027999, -110.681114579241, -110.49106131529867, -108.73493328004297, -110.07663907252234, -109.9968931372618, -112.10715231091008, -108.80994125105168, -111.63774865669372, -111.54355694032755, -111.64024217585788, -109.34986300492378, -108.88053713185408, -111.14370830146245, -111.17327416167232, -110.36311492990576, -109.99414559884396, -112.96912007380595, -111.43191437097785, -111.71327312809349, -108.77202323682606, -110.25970374932486, -112.59574277180732, -109.77247894866957, -110.09219852365874, -111.7197662726775, -109.85454092697009, -110.06789440397942, -110.38055758638309, -111.04251386932805, -111.54279434240568, -109.74385329575985, -110.98924544863415, -111.17898077762852, -110.98364252730245, -110.75024385843372, -109.24766708578407, -109.67753987004863, -110.6537235844391, -111.84436313010086, -109.12654337292446, -109.65519521121124, -111.1845162935778, -110.5009101465602, -110.22980642268818, -110.88540043278346, -110.29249073109453, -108.80459864528464, -107.49372141121728, -108.50353962704821, -110.00730069533373, -112.012876492648, -109.01283702976382, -109.07442203290057, -108.2961442983685, -111.60962842680907, -108.84312815413224, -108.6276642979969, -108.75132871638827, -109.30004903844721, -107.20359872252604, -109.12175943862074, -110.43914247337625, -109.55954680842791, -110.37116786618797, -108.55907813251434, -110.19249995041955, -106.95269845697632, -111.07027929458712, -110.1073996792702, -110.61729280468039, -109.6419175310234, -109.47995019876329, -109.66602827275211, -110.01953864498805, -108.45989120418268, -109.79778555296474, -109.94663827736616, -109.52410616839379, -110.58014441463794, -110.09182359045897, -111.0487262011397, -110.49609187214915, -110.6114701312941, -111.17752423063314, -109.74965389041003, -108.58973724447526, -108.84292130035902, -108.90689510645983, -110.69840140049361, -111.30494362640982, -111.00224390075273, -110.50848328538423, -111.59232911931113, -109.30826761863756, -108.44510893127558, -109.63744704504391, -108.95037574307332, -111.36486409910674, -112.74508631930381, -111.03952454593811, -110.57133212903979, -110.59969855145111, -108.25570461975128, -110.44617635200193, -110.32190307214704, -110.95204704643322, -112.0595421753479, -110.45342552693265, -112.50183987758867, -110.08217804938009, -108.90353583389084, -107.02032313792242, -88.3334978919524, -107.92027625495886, -109.83148570028482, -110.30427997450572, -110.92855407802753, -109.67404674397338, -111.03606345823586, -110.58277018943096, -109.77692362669393, -109.39170901729935, -110.20711662408928, -109.41601946806779, -110.34213214925832, -111.2283900972803, -111.51682597931386, -110.47069117801351, -110.93808974285523, -111.11277478000933, -112.50698886748012, -112.12918507523611, -110.46316790252011, -109.9387334819968, -109.78723249688426, -107.13037722044297, -108.16132376075751, -109.07255491017162, -108.85068428558272, -110.28038153100799, -107.77611023481016, -110.69754506886444, -110.09495581837979, -109.21214884561816, -112.62718526248648, -109.22048725312992, -109.17793923163308, -110.87372121410577, -109.71902632604333, -112.61041177225496, -109.6374750969677, -110.74738952366951, -108.93404661877067, -109.84938675700889, -112.25316361679832, -110.30788094875312, -109.26929069321925, -111.20853536783942, -110.05212566057608, -111.72448131932816, -111.55474439772887, -111.81988954424324, -108.44452452934028, -109.21897824914645, -109.55634869894358, -111.36318572800242, -110.05777399011298, -109.64458567712875, -108.73315084760529, -108.93332091319675, -108.4816455312154, -108.80120578498936, -108.1804470361839, -109.7177707524778, -109.31977709844544, -109.33603116022124, -111.46120546572519, -111.7480378245176, -109.17907150677627, -110.47970652472505, -109.73718750984082, -109.7935026884937, -110.40458408612054, -110.91781389491092, -108.39352075861481, -108.27512197925346, -109.59155075404814, -110.40183121737397, -109.25423373270381, -108.37769008625712, -107.91335995938509, -109.5576520703013, -107.27392145737491, -110.98592762117059, -108.41809950647861, -111.48163889400448, -109.70961684769624, -109.22952568656495, -109.76504719131209, -108.86928627177666, -107.97855299877004, -109.8412204399902, -109.6690048999326, -112.28329030175193, -111.54977099314607, -109.55689540119126, -107.93716711232997, -109.84247640855929, -111.5098351445789, -109.14317615215809, -110.28319116384824, -110.57901069942578, -107.2890252845352, -109.66754569546274, -110.15708115946433, -108.83782190109405, -111.60783857760667, -111.46884385151185, -109.21985333366634, -109.63605494317056, -110.87999187262697, -112.26992029775087, -111.05491095860552, -109.22795442529183, -108.99135781712076, -110.46475190704264, -109.35746113713218, -109.29125989270668, -107.40922407684049, -109.24391685563656, -110.41554602144217, -110.68952735085914, -110.62457364102458, -110.39856310555466, -108.84256124354566, -110.01614601335088, -109.8071306678428, -110.2804500736802, -108.76205061238203, -110.3962440297242, -108.98253716257014, -109.32990745926702, -111.17276766165281, -110.41113652364085, -110.36616199963426, -112.09767002991742, -108.43599666470733, -110.91876588140981, -109.05329272502944, -107.07198690769708, -108.72934463903034, -108.6666471996132, -108.97529973794413, -109.68895260146817, -109.2658844652487, -109.75690097249196, -109.38585024123027, -110.17593039468063, -107.87223111061134, -108.15261097418302, -110.09277437980633, -110.8665497655964, -108.43061614348413, -110.3052458526819, -109.22446919161898, -110.51909692711594, -110.06620699121913, -109.53439413051383, -110.31952463872884, -111.4732125902982, -110.41443606663168, -109.9579358088152, -109.930778061577, -108.5473214465574, -109.34719220288939, -109.16964653934396, -110.04824158176345, -109.42616539603762, -108.3556027482992, -110.62331917617789, -111.3652147859356, -110.12362012120938, -110.13175448595814, -111.20110099151856, -111.50643914621541, -108.11659117128028, -111.06037600347967, -109.03822892917451, -108.25678204604324, -110.82608024151122, -109.15887945314851, -109.88255674562845, -111.18322672526185, -110.95836040044516, -107.91535345885436, -110.66285812468733, -109.61906549925033, -109.58059721670746, -109.65198009505977, -109.65950565672951, -108.95264505276342, -109.23343669003113, -110.74308548011575, -106.39170014998685, -109.61471203101753, -108.24258770956924, -109.84609566640096, -107.83834185503922, -108.93052854090027, -107.55568820082641, -109.758551082242, -110.65892780872205, -111.99907420485852, -110.71043004141137, -110.62257237494617, -109.15610413532767, -106.87403836327807, -108.19175324576331, -110.27819583792918, -110.23918003777561, -108.29703377268754, -110.07182881114713, -109.60256111108491, -111.00394752430006, -110.30750337485472, -108.78309624082331, -109.24103013025798, -108.76979253891403, -109.91618737478264, -108.83915940855513, -110.92536150834754, -109.72250903746432, -108.96533939688658, -111.08949280651164, -109.20335070860871, -109.37826578362439, -109.77953166722301, -110.1867310744785, -110.07114559821346, -110.7003631567182, -107.86455899696074, -108.94113264174617, -109.35999427135138, -109.33627364788704, -108.96588828808375, -109.08716536982254, -108.73575375369026, -109.47770132070654, -109.83726171472907, -110.73516506891792, -110.56827134787686, -107.65667508354096, -109.30200115708924, -109.28406803847896, -110.55374624323233, -111.2017766725333, -108.50851279608973, -109.79494403619485, -109.08320018013063, -110.21850624918747, -108.4652936555984, -108.74837610538873, -108.81326140648238, -108.83830180036702, -108.785270477003, -110.01845876259073, -108.76030368637825, -108.57879884880157, -110.6610608456059, -108.74669367794318, -111.55956030460833, -110.22906685783455, -110.48411613865359, -109.48060880085136, -112.77556331479562, -108.2676071206087, -108.8571136162698, -108.56944905160177, -109.16406757131058, -111.42259299295839, -108.25216316582294, -110.48487127684025, -109.69532331373831, -108.13992755196784, -109.2987762526628, -109.82536192480795, -111.28650061088359, -109.12820736404241, -109.37960655471406, -108.96014976926716, -107.97535047619023, -112.31953123574708, -109.06198330523004, -107.52722515967098, -107.31555373665437, -99.89671790804692, -107.44442600896275, -110.6549218761941, -108.02265794322076, -109.63582761762919, -110.00574746987859, -109.51565124961209, -109.3550083591902, -110.4541529175301, -107.85799722437162, -105.1197113090786, -110.25038075579738, -110.39710812865657, -109.3618876098789, -107.6131301952152, -109.21529527621463, -108.7995754403799, -108.48347353145697, -106.45678488065816, -109.60427918561142, -110.81194387812535, -109.52215044127382, -109.88751598659705, -109.30205143590227, -110.74984456751768, -109.03952092986351, -110.69170786328897, -110.39236248162467, -108.65456161733339, -107.60439764386904, -109.97367926606955, -110.2754359970249, -108.81546418006434, -106.99691398176165, -108.42047325825182, -107.24499915944605, -109.28116135603187, -108.70650358781573, -108.05516916105047, -107.20893100196241, -112.07029265690055, -109.38099990478445, -111.53461820465232, -108.11312509555277, -108.76714028655223, -109.89565008459624, -107.71879172001115, -108.08434857420214, -108.79142773619792, -107.25153085963885, -110.05595039449301, -109.31604222314259, -109.94405791565286, -109.04715370361387, -108.89278831045846, -108.84682466376424, -110.0067927716526, -107.63768959294084, -108.98109382020348, -111.4720219575084, -110.76023788797733, -108.78599647633777, -106.59726674064618, -108.66715709719243, -107.99134359630926, -110.11396713841884, -107.21091759882775, -108.08576824949941, -108.80217666857972, -111.72949572713338, -107.33126296136014, -107.33731660097102, -108.04470462977443, -109.42963925921418, -111.03517778720736, -109.55293581015796, -107.99948151285162, -106.59480934999681, -107.63777243313498, -108.96490626068824, -108.8948210299064, -108.30870516747477, -109.13612869658097, -109.59971429402015, -110.2571461001396, -108.7655464686992, -109.81144209568883, -109.80796806645141, -109.20948481699544, -108.68653880881129, -109.26329796696166, -109.22428132233863, -110.12571678351438, -109.14615461144786, -107.08261621308327, -109.11338327144382, -107.75421565039201, -107.45291780756361, -109.00477000647248, -107.41031480478154, -109.98948062864928, -107.45953654921264, -106.37522884807879, -107.7786128523167, -108.03610987358499, -108.05926797128022, -108.59400205554164, -109.89620453365603, -109.03811240487515, -109.96909236705363, -109.28212981785472, -109.6772152101994, -108.26493868190678, -110.55558039199732, -106.6252818398841, -110.19075011176416, -109.56520012524705, -109.8023423576176, -111.2697570480663, -108.26752571816566, -112.00337375484828, -109.85709226796116, -109.36922081321148, -108.8424844298318, -111.2512302139209, -110.61775974680471, -110.22501328999012, -107.76874906708105, -110.71023653476604, -109.4025656165291, -107.66667684986125, -107.59759854092948, -107.94763263251238, -107.3888591871119, -108.62692803125044, -109.18012867988286, -107.78662871481455, -108.5072814073944, -109.50348958982907, -109.95177634938378, -107.78756251182895, -108.03865042797304, -110.1814993556385, -109.34937567548833, -109.52162025123161, -109.50819015441117, -108.20953105254624, -110.52154040214435, -109.3324404469266, -109.2696617050831, -109.54675609195674, -108.5940367000989, -109.40184828664549, -108.2518305610941, -108.55972691669434, -109.03647225394408, -108.48166656251695, -107.42023429066523, -109.42453054302521, -110.09532345960083, -108.78315822119662, -109.97508586102265, -108.22687406536997, -109.17110028890058, -110.15390449992647, -107.88577458651508, -108.28851074361447, -108.52030295163331, -110.03496861709483, -109.40014319167584, -107.73048113044877, -108.17571683963915, -110.34839852994926, -108.55894048192191, -108.74107339998285, -111.17734138993401, -110.22946440841412, -109.45511941802884, -108.0657300641843, -109.33797363184166, -106.95974095511333, -107.93068343723691, -109.78867669512647, -107.2087297624043, -109.542665021243, -110.05035859052961, -110.30235238883523, -109.20586170783808, -109.2796396673401, -109.14260673746566, -108.22019460542734, -109.99011886871159, -109.89103038547285, -110.36964772493243, -108.62340319923602, -109.06779821699769, -109.21830861066148, -107.7402395759509, -107.7178850938205, -113.45665085929117, -109.24039191621704, -109.30387033426037, -107.61849760982835, -109.41430582703529, -109.11482836392241, -111.89328423764577, -111.84653367963301, -109.00674896486915, -109.84488648739638, -109.41914760797953, -108.53442910169935, -109.66883322968232, -107.68762956301386, -109.82583101109167, -107.83405397804887, -108.78052031141966, -107.37842078941692, -105.40843158543845, -108.81430898189338, -109.57374640194516, -109.41111270322058, -108.82621700188898, -110.2552502368822, -110.23903890097205, -110.52171662278697, -108.21249857906324, -109.97268479379733, -108.20088823960992, -108.85682002802234, -110.11642849164285, -109.94087886999255, -111.63180946270296, -108.20899499456195, -106.73341567332112, -109.90003508676807, -110.14688274481229, -109.62259307329889, -107.57811196819495, -106.88584597822792, -109.16132624528932, -109.78677836397806, -108.59319344451784, -108.55877448618652, -109.46883711353044, -108.47309455543844, -108.09487065732198, -109.82219079158135, -109.63780237877428, -109.28348848877269, -107.62893405379826, -109.46986737961593, -108.03089712610223, -110.3931917410696, -106.06970126043262, -109.41866550703786, -105.31710372440419, -109.20218082282653, -108.28467118008108, -108.80026326744611, -107.40729224715713, -111.07322915141532, -107.1057186510818, -107.98286374205958, -108.51298722989311, -108.69632670891366, -107.96509231988331, -108.15882223414738, -106.85862416470376, -109.70705792539056, -108.64519930633055, -106.78708421443504, -109.43552377900174, -109.4474526498122, -109.10135248755788, -111.43316642580763, -109.33457343739448, -110.23547887071898, -108.95690647379442, -109.21159903769149, -108.12969562680841, -110.82751409340537, -108.55724349027832, -109.8796329603075, -108.50369978374582, -107.43145467247209, -108.60003323209516, -108.77155705999647, -109.33806063660796, -108.37500858898439, -109.65641721611547, -109.81905873737344, -108.03483220769625, -110.48028107566635, -108.60527372219985, -109.28768201151478, -99.8804125587218, -108.8913334544964, -108.23534920737794, -111.07646463287153, -108.59029790589766, -110.3405916586831, -107.66387718565608, -108.73793152614131, -110.61440166477816, -108.76211382544581, -110.23236978486065, -109.10669297094852, -109.15247609779597, -109.00539004923506, -110.14424353412238, -110.55445060661157, -109.48721312920799, -108.17040942305823, -108.77592227268228, -108.77130256578067, -107.82494496098512, -109.57266989523707, -108.75767497229612, -108.13688624150026, -107.8280716764963, -105.676279602552, -107.6370316684844, -109.73508547021689, -109.25365178573009, -108.86767843317584, -109.70969944273735, -108.91917504090888, -109.97734866522867, -112.17308993943783, -110.28356299479682, -110.7927103729386, -110.30837645846702, -107.56364161860179, -109.50188349731121, -109.36065627483853, -109.75389877587511, -109.81713476007774, -108.14524057525358, -109.43832376796216, -110.89342891210596, -108.15657882822792, -106.84106061627887, -107.83091759905821, -108.61794662682962, -109.57142366843581, -109.85402645528154, -110.12877022469837, -109.19414429724044, -110.56168468006764, -108.74720588273881, -107.90448559921305, -108.54421401507743, -105.06700039841249, -109.17937358052484, -108.94317576365822, -107.79410219455083, -109.24955437598658, -108.23334395173994, -108.98759227946937, -107.05986359444529, -107.20956512998849, -109.00295831471958, -109.43119556916457, -108.93348410522628, -108.99932477701081, -106.6448790859128, -109.06877251308666, -107.67053918439544, -109.15052780608639, -110.16878033319385, -106.55101141640301, -108.02811045752685, -111.52173447126572, -110.16854119242062, -110.93164036911654, -111.25979320890855, -108.82629030379024, -108.52004501839738, -107.09697056562636, -108.94233383169858, -107.37962568194772, -109.1239201710643, -108.93949898577122, -110.62573772949195, -110.09592372075662, -107.56136391005947, -110.45600430869621, -108.79481000016084, -109.41462449554598, -109.30248158488335, -108.70735295493108, -109.9174743694956, -109.94232543385962, -110.71725446170196, -110.0346196158573, -110.34814317845934, -110.6651078322521, -107.55409880424479, -108.71734776861287, -109.50902203986271, -110.40207542979611, -108.7847687630861, -111.10599488129682, -109.30824728923263, -108.20134064331717, -110.55959112431609, -107.77099734327174, -110.23862843385446, -108.48520797666865, -108.54205896654946, -107.79288769037599, -109.84022250170581, -108.02758364115576, -109.35132492327935, -108.87009749667932, -109.86905123364855, -109.19826752168308, -106.835240323691, -109.37910022114056, -110.80633973102931, -109.12703823829597, -111.07432699570984, -111.8064506085314, -110.09349947650527, -108.66467295777367, -108.75119108236053, -112.63983351316729, -110.90940743670113, -110.27973159222081, -109.57141664526549, -108.61645363771719, -109.31742355616147, -109.5839599160637, -110.01188998365383, -110.01923429741011, -108.94779759137936, -108.26169431000017, -109.24553201026085, -109.95709526422822, -110.68677343596859, -108.7678734483002, -110.47090469179284, -110.31604700116512, -110.10256600741997, -109.76634647265719, -110.8830805828562, -109.94609564072982, -109.20662382740542, -108.12492970530919, -110.5274435478767, -108.02351960398035, -110.6264936805739, -107.14559226383577, -109.13821777857531, -111.05324489472586, -110.15190797512811, -107.96366234783144, -110.03950681967147, -109.17476300510336, -110.41251816187909, -111.39219865477246, -111.32530426869943, -109.97369363558423, -108.98666403063845, -109.62049358645565, -109.58130494498671, -111.72738873188874, -110.39825891106616, -108.57430325757545, -111.28625510212446, -108.77421250595326, -109.75025415031793, -109.51948456745635, -108.82129398637998, -109.81362137198361, -107.86292494316123, -107.49318292857053, -109.66948564589373, -109.54288390056654, -107.99912445612077, -110.3497559614379, -108.00549349666127, -110.01361420523357, -108.4977916421456, -109.67078387286976, -109.85678367732866, -112.01237658746248, -108.4855625950998, -110.84880875737286, -110.9178674382154, -110.44187536727453, -108.75076921971127, -110.04946286646651, -109.99780941000827, -110.14242932305507, -109.56343773672316, -109.6278993388131, -108.77419573790174, -109.10543670530926, -109.7801848627463, -110.30733124104881, -113.13440550301436, -109.32709134514755, -109.74136656933283, -110.01525283266193, -109.43924662938396, -110.25325289253, -107.75460576671303, -110.60057027395933, -110.71458404922404, -110.15788509050662, -110.69167485018224, -110.96006652476157, -111.01156633983031, -111.6058448010008, -109.51364005052672, -109.76058205940885, -108.43421621088261, -109.47973949170208, -109.25533250208288, -109.47422603921065, -111.36411644613841, -107.27566171102698, -110.45098686173688, -109.93589296291184, -109.03803734663714, -110.53118128434016, -110.2408872254969, -110.0532234862915, -109.94185495614619, -110.2662004220774, -109.51094016962288, -108.5210104215432, -108.13691752270934, -110.18460088390265, -108.32609309150783, -109.89652230508281, -109.80923900768477, -109.01917388968883, -110.01248300968739, -109.43415605440147, -108.09823485138017, -107.40637725320931, -109.40632232658412, -111.97981999127656, -111.16609811629485, -111.64500793960192, -110.99793748693381, -109.55531276386903, -110.2535662621666, -108.17429802469516, -109.09425673355422, -110.23187110421917, -110.55358397926925, -109.93461124753053, -109.55604345832225, -109.44569510408274, -109.72185151080762, -109.52963702944834, -109.2303630328152, -109.74819502244243, -109.3932530349457, -109.17096788339686, -110.46153727064616, -113.1073731246639, -109.43753070459397, -108.13332547768168, -109.42294574929969, -108.45798401969856, -110.29453435046327, -112.66249403705643, -108.78314667434937, -105.9634478773668, -109.14327524669528, -108.50645190860273, -100.81571594994128, -104.4482859840643, -110.68926237051092, -109.12362553230196, -109.45234390564677, -107.91461416156068, -110.67788819353727, -110.05744935668449, -111.78333392154664, -106.83628914455993, -110.11115457346548, -109.13434608275826, -110.80006861194663, -110.35323502651462, -112.29149906501372, -109.01656376530778, -109.30871662948859, -109.79736315392456, -109.17848983603582, -108.09752397056482, -111.6039030763455, -109.27008844877828, -110.84475733314184, -109.72393917557073, -111.31060762894991, -110.78858793807466, -107.12841545099752, -109.54510865218204, -105.2805426080281, -106.28514149354733, -109.50656759582803, -110.14700878401054, -110.49737016725709, -109.19811547071924, -109.92527399676051, -110.7961615015146, -109.7447227818197, -109.49432012009893, -108.714081576733, -110.09766801550917, -109.08448507943001, -110.36154838733857, -109.86328656267403, -109.21144237434696, -112.4145136888034, -108.57567151011159, -109.66748589540896, -109.72985837578446, -109.29989238126763, -109.85868902806475, -111.01778182304162, -111.23625326328558, -110.01270868104203, -109.27067928081415, -109.71171312410247, -109.28697459293629, -110.67868067201007, -110.91353786857455, -111.21479955051575, -109.11315965407708, -109.40418681804496, -107.80511819596003, -107.37201025889816, -111.81969609169838, -109.89875624306032, -110.29328043898657, -109.74853280072202, -111.39527865400605, -109.47746221101964, -111.75141177452517, -109.31325306583483, -109.30117448911659, -109.3997781364162, -109.45356931295724, -109.60585285774386, -111.33951689512735, -107.74187210470228, -109.62706021606415, -108.72139655505221, -109.79552836110567, -110.64354037499807, -110.96138240913136, -110.02215059889615, -110.92978442698893, -110.0620778287114, -110.85019647293322, -111.77397403227091, -109.81257196800128, -109.15643451383403, -110.72777566469594, -108.7463769025616, -109.80959395914073, -111.24500986151126, -110.48863498350322, -110.30863780110901, -109.79331354195703, -110.34087081762074, -109.45183222569266, -109.6440990067103, -111.15034876658994, -112.14912485578341, -111.8886180186196, -110.57054820211916, -111.07556239924551, -110.5872832735073, -110.28912501038172, -108.91501133754849, -111.44575118962761, -109.90799859177967, -109.74421995550023, -108.70941446115883, -110.28822893097275, -109.70039554000401, -110.33701797570251, -110.79445894683306, -109.57694314608153, -108.816904416038, -109.66517126767175, -109.39501469321644, -110.85775022889956, -109.3689402795614, -112.09107318723095, -110.67985626248422, -110.32971146814747, -112.08166943494875, -109.93955548712543, -109.31722953035252, -110.2062913031861, -108.22565380081006, -110.680898028151, -111.95386604441454, -110.83354130587097, -108.5873626748948, -111.97536144124408, -109.23944159551515, -111.57859477689586, -110.80135186615524, -110.4800953731021, -110.14040729648133, -109.25873050390551, -108.87000960474569, -110.97091597211167, -110.15787270199012, -111.62434537618091, -108.5421625277294, -110.42258666403919, -110.96896115868603, -108.98253068925274, -109.54245055160168, -110.28051096122468, -109.48060498658319, -109.77618362117276, -111.64513838754992, -111.13945484239875, -110.18094280356001, -110.43757222770748, -110.81588360154201, -110.11656805555333, -108.47936291282355, -109.16476249859961, -109.3549985917136, -110.77753190334253, -111.46065694661178, -110.40387985996301, -109.95673803226478, -111.58660981285446, -108.59894875229345, -109.37333363882607, -110.26849699991793, -109.30500469266264, -109.23789020998296, -110.82000706486865, -109.25927538839868, -111.03285659417519, -111.08899832832414, -110.69361682858042, -109.45187168573815, -109.9614018482838, -109.70209527974106, -112.11903952100165, -109.59713611623246, -110.70292028698111, -110.12743849746808, -110.63315585514292, -108.60450276298175, -109.32832664986026, -109.99753023477764, -109.46644696130294, -109.1781290160558, -111.58830180575129, -111.67229040267557, -111.3750024136205, -108.33616679452298, -109.99797067800029, -110.50892429124391, -108.66074740829372, -111.17094662568759, -109.87538933985836, -109.152526628291, -110.44623159817101, -110.21603106403009, -110.64376935639365, -109.36897426842583, -108.67303022227141, -109.89327693080823, -111.50442955563923, -111.37532237834381, -109.38132821290205, -109.73509680539144, -110.53918379735906, -111.22869870340647, -109.39977573957616, -110.3674665334106, -110.5366125953241, -109.99025356764304, -109.97300035646616, -109.87631077033762, -109.64608829594286, -113.02486102973394, -108.26250283140733, -109.62234918138763, -111.18766216512655, -110.33666026406992, -110.5808115327039, -108.2971671321189, -110.10964334161903, -110.61254021379767, -109.89852549557533, -110.16562049054073, -109.41433790018287, -111.2453823439446, -110.45554802599901, -113.11454453784393, -110.7333866145056, -110.00858191882439, -108.54745315874294, -110.08430415376903, -111.9006972727596, -110.3031506154679, -110.26331790366497, -109.36797925566673, -109.04860552478912, -111.83514212681175, -111.38960737633833, -109.01429665187288, -110.96404839103826, -108.95488871107163, -109.09652004914592, -111.884304581971, -110.57566691021339, -111.95113404442795, -110.13677174050159, -108.10078686353354, -107.69442565416006, -112.42676605669463, -109.12681161784135, -109.23120766087519, -110.57649395555585, -110.22143082743162, -108.40065951773644, -109.46923168308618, -111.39095086729745, -110.46375658526013, -111.45145283328486, -112.22610823637353, -110.61090190564383, -112.22250292674809, -111.7379343196361, -110.18530386733481, -108.93867365671692, -111.89304844956082, -109.06146134986984, -110.98405731832798, -109.76366821333497, -108.08326795663608, -109.95041147835065, -112.94140614324155, -111.79814935135965, -108.07337559063119, -109.13733403265212, -111.74906646037496, -111.12228668433455, -110.02899450462209, -110.22237716929811, -109.0224776891049, -110.18135850497721, -113.32516073881047, -111.3576490243877, -110.60510094465171, -109.6935518470342, -110.36313473154901, -111.95933240129618, -109.49625308071019, -109.18827910216122, -110.54311407822692, -108.4811035913567, -112.81280225723607, -108.86530665787413, -110.85796435061886, -110.40059714639627, -108.19250716343407, -108.96956521802292, -108.61281798886506, -109.78061525370413, -111.58885511891798, -109.06279169160345, -111.43043988466789, -111.63169336321079, -109.54702536206447, -109.62860636296405, -109.47865811135546, -108.02265793654806, -109.97461304995515, -110.72549884050886, -111.57309413919933, -110.03317891949746, -110.39570411598524, -110.27606115470397, -110.63294457306095, -110.71821689302902, -110.38076268941819, -111.51223508887897, -110.40703572670697, -112.24933273737743, -109.74954300082398, -108.46020292937696, -111.05315219575881, -110.38635148390118, -109.58268303790976, -112.34211536832117, -108.45894118755307, -108.96463982695337, -110.56040438523046, -110.67803313671729, -111.07349872375121, -110.42184162876096, -111.82081126435692, -108.85923651136297, -112.57723799596502, -113.65690874668172, -112.62314325834605, -110.70357529341362, -110.959925221544, -111.26336183001875, -108.1350700630152, -107.94545932312926, -111.17610778209841, -110.20386728310686, -108.55646511121591, -109.8400922569145, -111.73466587035968, -110.47272877573613, -108.33011124048193, -107.93042857580332, -108.60928277989103, -109.25240966798974, -108.96403833602028, -106.94222615757475, -109.37086694261907, -106.72743097285155, -109.03160193412796, -107.3549903889451, -106.8543848510082, -107.83503929060929, -106.30745467433752, -108.36915807168845, -107.13065938379303, -107.84769200880969, -106.08004345082777, -108.15244601930225, -108.37254117816573, -106.57863034819223, -108.1283698227614, -108.19776505569902, -107.58283412238643, -108.17365133196301, -108.6794309781181, -107.91552140588759, -111.60122989270022, -107.04360635941174, -111.55535949001795, -109.39870426166594, -109.55937904851662, -111.81389508925734, -109.88957041098786, -110.84764586896561, -110.59130246272693, -111.15944135223884, -110.19496154041607, -111.51861903129362, -110.74798816525838, -111.37312965175558, -110.10842817220238, -110.73198099204856, -111.36708667993291, -110.30840247819665, -110.11744489669044, -110.55237850846444, -108.2073528237766, -112.70750856801911, -110.99917956040802, -109.84949484779976, -111.3403161887679, -110.08924435263565, -110.17749213365616, -112.10849123224503, -110.94270741299202, -109.29350963424746, -110.33477486966507, -112.19620157705627, -111.45484078395934, -111.86858843505124, -110.22491147345858, -108.96177661263177, -108.67862820579893, -107.55155410582937, -108.27984439169573, -108.72682528077233, -110.64231212183269, -109.32873093119183, -112.98564364754564, -110.78933114228725, -108.50921025910479, -107.91087245586935, -112.57350030929283, -111.75871577457525, -108.42095298945462, -112.31266064114303, -110.1295657579673, -109.67444664474456, -110.33749884929306, -109.16098218724147, -109.63554874360221, -109.15892392675141, -111.90580809179818, -108.81196712336858, -111.42223552606656, -109.90571484965518, -109.99739812086352, -111.64103850263211, -111.31463957090885, -110.61247447444549, -110.20960333715526, -110.1707327818923, -109.70412636554525, -110.97278093107532, -110.24386747740314, -109.81378546061525, -110.83784085086458, -109.77357954318757, -111.22663832948885, -111.14563050139252, -110.87152231402447, -110.34246044319893, -109.97174570657546, -110.23599592972218, -111.08206161770731, -110.0073315341242, -111.11748366902188, -112.04005964728601, -109.81290191679287, -109.68543639040858, -112.01143296194752, -110.13641850530031, -108.19348942447623, -109.7534468948808, -109.36697824644176, -97.56454580435337, -104.97829040517887, -108.1539132982256, -110.048991273122, -107.46172505860011, -110.49269280640675, -109.94209901400029, -109.38576869679022, -111.43699124347364, -110.89973083498887, -111.2994445418276, -109.25144782032437, -113.25676258473536, -110.82078737428088, -109.97779571182073, -113.36294799183014, -111.38584551238931, -112.17267897274873, -108.56430946159155, -112.06841286528645, -110.36822473102735, -109.54758527532016, -110.48190506674653, -110.03535695860182, -109.3951469796576, -112.41910682256774, -111.38124138857238, -109.37850389100952, -111.65544568836181, -111.55876881606889, -109.3029209617236, -109.20030046194076, -108.82610577621037, -110.53329453526098, -109.96090595542142, -109.67834229432077, -110.62303603007352, -109.8388817181171, -109.22430039793213, -108.92749786663613, -110.05794249283548, -109.58534943218437, -110.50493887507297, -109.96373022997366, -111.0645036323456, -111.28501675364454, -109.77386932343008, -108.8952247140968, -110.09242801628717, -112.90943444063141, -110.72299296247249, -109.39094335967056, -110.95165384057718, -109.59809519359453, -110.4978602309597, -109.67109981692639, -111.2489619905986, -110.0937750887109, -109.76771021128954, -108.32976315018955, -111.3058145792439, -111.09464974601362, -110.99797900696136, -109.174315000222, -109.630351559617, -110.26289147175856, -110.22688407202517, -109.96748050100612, -112.13247633583758, -110.59994952890855, -110.93023020153811, -109.22457750926695, -110.26162558926984, -110.09713110375579, -111.73858994918328, -109.78183160058515, -109.7603471824367, -110.96016892586911, -111.23309626937036, -109.83093663960678, -114.05354944347246, -111.58202863059464, -110.42281828744524, -110.9521484732059, -112.5120328206343, -111.614891937737, -109.84428787405484, -111.61119567831453, -110.43095563229411, -111.71833448430398, -110.01132196809407, -109.37558169247951, -109.14091380022785, -110.42663661754088, -110.3598013572826, -109.78207135281417, -109.94058843992468, -109.88210328447205, -108.6217811850147, -107.17834387173707, -110.6447226986756, -111.10704778101115, -111.24396771977769, -110.47849395539598, -110.75150631628034, -109.67662689396347, -109.23145032835053, -108.83780193265358, -109.43468321661163, -102.22521103859944, -106.90009867479111, -108.91580608784525, -109.58671397003187, -110.56692028436989, -108.75103142680105, -111.00795573084157, -110.75039085328763, -109.48222099288613, -111.8621134816908, -110.26507966786443, -108.885924716389, -109.30841399453053, -112.3188631425597, -111.05677697153163, -108.8268571902449, -109.63028152237679, -114.82339015806369, -107.03435216376964, -111.34847692589166, -109.61354114874855, -112.32687758049907, -109.59816404231358, -111.64248480241805, -111.84075757907273, -110.44017657636552, -110.15181635726277, -111.93813663582833, -109.11826378836209, -109.99779889778326, -109.927119030584, -109.4389650887841, -111.52448814187727, -111.38736268499642, -110.51920914917922, -108.64230614681055, -108.90307263595304, -110.57246891832371, -109.65575340646116, -109.80359672370373, -108.83368585528197, -111.09385004343437, -108.83430005497769, -112.37784208819113, -109.50005381621696, -109.67421750136593, -111.39664088797532, -109.70867599669316, -109.52498993629875, -111.12341349673187, -110.0484037026941, -109.55138667646308, -111.06614422098669, -109.4785941493091, -110.25724082617013, -110.93950616855716, -110.53487953881397, -111.45722057988401, -110.32393446412904, -110.34361936710438, -108.6610336097813, -109.53631603696368, -108.06930707969195, -107.68056561368934, -108.73860971027449, -108.87111384617579, -108.40433837098611, -110.55999576884835, -106.83832061167207, -108.28786975902513, -109.18482905697472, -107.81071696594883, -107.91047268802457, -108.79613111673706, -111.05361322310213, -109.97897453479862, -109.12920563729425, -111.20538391490288, -109.26286135293664, -111.31400407177502, -109.92167984752287, -110.70854322826071, -108.59406515713611, -109.69371333227458, -109.36664873267313, -110.35521729513704, -110.40667924006368, -112.0181844636846, -111.01529188207431, -110.59246505728431, -109.95068312717868, -110.75807466894047, -109.58596443762707, -111.12127793384956, -109.59041634463125, -111.56255571372793, -110.43405578864342, -108.39660324329928, -111.1420710307505, -113.64788483868595, -111.67645688353934, -111.36878760365944, -109.68523694561108, -110.11608766310304, -109.25670490330123, -110.73546181099229, -111.77855039399805, -107.9662794718261, -109.67483334602832, -109.891258579519, -110.24757768183042, -109.50202895993814, -110.07763831916637, -109.96891925839451, -110.97268925927641, -109.31698133827767, -112.27933593506792, -110.36206721075725, -109.47379463718867, -110.27836850941338, -110.63738280998388, -111.3611682777485, -110.72689155959884, -111.55480904927032, -111.16689658479412, -110.35555645743601, -111.56609319131051, -110.88279459952174, -114.73607246523177, -109.95813757295693, -107.64639932425493, -111.26486783320321, -112.03946356928121, -111.8915972448334, -110.35245920812773, -110.83155104803564, -110.67437747473863, -110.9959682920065, -110.7815352345103, -111.13722283763049, -112.54797265493127, -110.06894780898469, -111.65186554925783, -111.83545188116254, -110.65894756123697, -108.48458025065264, -112.43760714427981, -114.1368408201927, -110.40065777895025, -110.1066998945526, -108.60654239598591, -110.5716060205154, -110.74257357180736, -111.1136089342442, -111.53539811075092, -113.2559601458872, -109.2003227548348, -110.42285840441025, -111.4086884998834, -111.61503050693868, -110.8194303494779, -108.9701587059964, -112.58521089509063, -110.10873915265242, -112.43440038319561, -110.03468788439882, -111.57896603236308, -110.21939233582523, -109.03614470500777, -110.11738923539659, -109.55359574898291, -110.416473622654, -109.4626868574157, -111.17164025076731, -110.3579689035081, -109.04338716157822, -112.36157114517567, -109.32125615922843, -112.71105693789394, -110.11019129547768, -108.96439402555632, -111.107663418839, -111.48306369859839, -110.9317530461794, -107.98628540532181, -111.1636972328743, -110.47837837583148, -109.04649309175733, -110.27110334963734, -111.35803630614352, -110.77259078859605, -111.46352820533895, -111.16789261049541, -109.2376344776325, -111.6795794983659, -111.74292205167644, -109.40835022991612, -111.02163652600731, -108.79482078001607, -110.6718658416566, -111.08747067599332, -112.15383726791498, -109.47049126158717, -109.061574046483, -111.23993049318979, -111.02521156588335, -109.46012868444186, -110.13918914826291, -112.08180381836377, -110.61929875223015, -111.4424805369965, -111.43420275069585, -109.71347556238717, -110.24726273025648, -109.7860268673935, -109.94126895018422, -111.41948668868926, -108.90555991781676, -110.81242861886172, -109.65007052722677, -112.12672329335953, -110.01123170946096, -111.13980448279096, -113.92013682657084, -108.6000853867411, -110.66793592761913, -110.61237681642844, -110.00839105230496, -109.38083187034974, -109.46119372195675, -110.3708067287448, -108.55518656223285, -113.33935987443276, -111.92184778392033, -111.80820718236087, -107.36852757311246, -109.51077803361602, -110.066791721019, -108.756710558672, -107.91391289865918, -110.72851430959301, -111.39074956442978, -112.928843679455, -109.87348280521556, -112.21371750380071, -110.82495902297394, -109.94006136010094, -110.58757785050143, -110.2790091349881, -111.43884888223081, -108.09540986530712, -109.63783244641691, -110.19577975613292, -110.01690033746098, -112.75938920157155, -109.27158857362184, -111.19519821680541, -110.14381902425255, -110.45955291199236, -111.55660330002316, -110.75604254261134, -111.02122553784838, -111.6490091060193, -110.93362819419399, -110.49033159684308, -110.70789549836027, -110.41991882034145, -110.0264093421208, -109.18432746063652, -110.15292268755287, -112.40733942236504, -111.32869665965416, -110.95418667871114, -111.14291568823575, -111.75555369152653, -112.98146297069803, -109.73870744292117, -111.33806139459435, -110.18838799491355, -112.60408243005732, -110.26112648646833, -110.58257045107274, -109.75155437454112]}, ...(2 in all)]
  in  "FFT 1 Choice 1":u16(ring) items=["T1 Y", "T1 X", "T1 Sum", "T2 Y", "T2 X", "T2 Sum", "T1 FB X", "T1 FB Sum", "T2 FB X", "T2 FB Sum", "PSD Y", "PSD X", "PSD Y Sum", "none"]
  in  "FFT 2 Choice 1":u16(ring)=3 items=["T1 Y", "T1 X", "T1 Sum", "T2 Y", "T2 X", "T2 Sum", "T1 FB X", "T1 FB Sum", "T2 FB X", "T2 FB Sum", "PSD Y", "PSD X", "PSD Y Sum", "none"]
  in  "FFT 1 Choice 2":u16(ring)=1 items=["T1 Y", "T1 X", "T1 Sum", "T2 Y", "T2 X", "T2 Sum", "T1 FB X", "T1 FB Sum", "T2 FB X", "T2 FB Sum", "PSD Y", "PSD X", "PSD Y Sum", "none"]
  in  "FFT 2 Choice 2":u16(ring)=4 items=["T1 Y", "T1 X", "T1 Sum", "T2 Y", "T2 X", "T2 Sum", "T1 FB X", "T1 FB Sum", "T2 FB X", "T2 FB Sum", "PSD Y", "PSD X", "PSD Y Sum", "none"]
  in  "Compute FFT":bool
  in  "Reset FFT":bool
  in  "# Spectra to Ave.":dbl=25.0
  out "Ave. Time (s)":dbl=1.5
  out "1 Channel":waveform(dbl)(graph)={"t0"=timestamp(0 s since 1904-01-01), "dt"=1.4999999999999999e-05, "Y"=array[20000 elements], "attributes"=variant("NI_ChannelName"=variant(string "T1 Y"))}
  out "Slow mean":dbl=nan format="%0.2f"
  in  "Slow mean N ave.":dbl=1.0 min=1.0 step=1.0
  out "Mean Intensity":dbl=nan
  out "Sigma":dbl=nan
  out "Sigma/Mean":dbl=nan
  in  "Subtract mean":bool
  in  "High Res. Display":u16(ring) items=["T1 Y", "T1 X", "T1 Sum", "T2 Y", "T2 X", "T2 Sum", "T1 FB X", "T1 FB Sum", "T2 FB X", "T2 FB Sum", "PSD Y", "PSD X", "PSD Y Sum"]
  out "APD 1 Rate (Hz)":dbl format="%#_3p"
  in  "Tab Control":T4(tab)
  out "Stage Moving":bool
  in  "Read Cal":bool
  in  "Confocal Linescan":bool
  in  "Speed (nm/s)":dbl=100.0
  in  "Furthest Withdraw (MHz)":dbl=15.0
  in  "Confocal Image":bool
  in  "Round T1 X":bool caption="Round"
  in  "T1 offset_x (mV)":dbl=nan format="%#_2g"
  in  "T1 kappa_x (pN/nm)":dbl=nan min=0.0 step=0.001 format="%#_2g"
  out "Time (s)":dbl=6.12
  out "Total Time (s)":dbl=60.0
  in  "Start Saving":bool
  in  "Cal sets to save":u32=50 min=1 step=1
  in  "Comment (data description)":string="testing confocal setup"
  out "Calibrating Trap...":bool
  in  "Trap 2 (ON/OFF)":bool=TRUE
  in  "Trap 1 (ON/OFF)":bool=TRUE
  in  "Save Calibration":bool
  in  "N sets to save":u32=200 caption="N Sets"
  in  "Save N Sets":bool
  out "Save file name":path=path "C:/Data/110526/110526_022.dat"
  in  "Save ave N":dbl=500.0 caption="Averaging Factor"
  out "Saving...":bool
  in  "Stop Saving":bool
  out "Progress":u16(slide) scale=0.0..100.0
  out "Manipulating Trap":bool
  out "Buffer Status":dbl(slide) scale=0.0..1.0
  out "Overflow (data lost)":bool
  in  "Reset":bool
  out "Data Rate (Hz)":dbl=66666.66666666667 caption="Trap Data Rate (Hz)" format="%#_3p"
  out "Data Period (s)":dbl=1.4999999999999999e-05 caption="Trap Data Period (s)" format="%#_6p"
  out "Save Data Rate (Hz)":dbl=133.33333333333334 caption="Rate (Hz)" format="%#_6p"
  out "Save Data Period (s)":dbl=0.0075 caption="Period (s)" format="%#_6p"
  in  "T1 alpha_x (nm/V)":dbl=nan step=10.0 format="%#_3g"
  in  "T2 alpha_x (nm/V)":dbl=nan step=10.0 format="%#_3g"
  in  "T2 kappa_x (pN/nm)":dbl=nan min=0.0 step=0.001 format="%#_2g"
  in  "T2 offset_x (mV)":dbl=nan format="%#_2g"
  in  "BD 1 Frequency 2 (MHz)":dbl=80.0 caption="T2 X (MHz)" min=50.0 max=100.0 step=1.0 format="%#_6p"
  in  "Green Laser ON/Interlacing":bool=TRUE
  in  "Round T2 X":bool caption="Round"
  in  "AO1":dbl(slide) caption="Confocal Y (V)" min=0.0 max=10.0 step=0.01 scale=0.0..10.0 scale format="%_1f"
  in  "AO2":dbl(slide) caption="Confocal X (V)" min=0.0 max=10.0 step=0.01 scale=0.0..10.0 scale format="%_1f"
  in  "Trap Raster Scan":bool
  out "Raster Scanning...":bool
  in  "Trap Delta (MHz)":dbl=20.0 step=1.0
  in  "Trap Intensity\nSetpoints (V)":cluster{"Set 1":dbl, "Set 2":dbl}={"Set 1"=5.2, "Set 2"=6.6}
  in  "Index":dbl=1.0 caption="Save File Index" min=1.0 step=1.0
  in  "BD 1 Frequency 1 (MHz)":dbl=65.0 caption="T1 X (MHz)" min=50.0 max=100.0 step=1.0 format="%#_6p"
  out "Current Position":dbl[](array[numeric])=[4.2944, 4.91027471, 2.9278058] format="%7_7g"
  in  "Position Label 5":string="upper flow spot" caption="5"
  in  "Position 1 Label":string="Top capillary (SA beads)" caption="1"
  in  "Position 2 Label":string="Bottom capillary (AD) beads)" caption="2"
  in  "Position 3 Label":string="lower flow spot (ATP)" caption="3"
  in  "Position 4 Label":string="Dump beads" caption="4"
  out "Pump 3 cont disp":string="Left: ADig beads"
  out "Pump 1 cont disp":string="Right: DNA beads "
  in  "Ch 1 Inject Rate (ul/h)":dbl=50.0
  in  "Pump write delay (ms)":dbl=300.0
  in  "All Pump Parameters":T5={"Pump 1"={"Diameter (mm)"=4.61, "Units"=4.0, "Volume"=100.0, "Rate"=50.0}, "Pump 2"={"Diameter (mm)"=4.61, "Units"=3.0, "Volume"=0.0, "Rate"=0.0}, "Pump 3"={"Diameter (mm)"=4.61, "Units"=4.0, "Volume"=100.0, "Rate"=250.0}}
  in  "Ch 2 Inject Volume (uL)":dbl=100.0
  in  "Pump pause delay (ms)":u32
  in  "Ch 3 Inject Volume (uL)":dbl=100.0
  in  "Ch 3 Inject Rate (ul/h)":dbl=250.0
  in  "Flush Center Ch Volume (uL)":dbl=15.0
  in  "Flush Center Ch Rate (ul/m)":dbl=100.0
  in  "Inject Valve B":bool caption="Inject Pump 2\n(Flush Center)"
  in  "Total Volume\nFlushed (uL)":dbl
  in  "Tab Control 2":T6(tab)=enum."Feedback on Trap Intensity"
  in  "Restart RF":bool
  out "Total Counts (ticks)":u32=600
  in  "Trap ON/OFF X or Y Amp?":bool=TRUE
  in  "Oscillate Set 2":bool
  in  "Trap 1 ON":bool=TRUE
  in  "Number Interlace Sets":u8=3 min=1 max=3
  in  "DIO count 3 (ticks)":u32=200
  in  "DIO count 2 (ticks)":u32=200
  in  "DIO count 1 (ticks)":u32=200
  in  "BD 2 Amplitude 3 (%)":dbl min=0.0 max=75.0 step=1.0
  in  "BD 2 Amplitude 2 (%)":dbl min=0.0 max=75.0 step=1.0
  in  "BD 2 Amplitude 1 (%)":dbl min=0.0 max=75.0 step=1.0
  in  "BD 1 Amplitude 3 (%)":dbl min=0.0 max=75.0 step=1.0
  in  "BD 1 Amplitude 2 (%)":dbl=30.0 min=0.0 max=75.0 step=1.0
  in  "BD 1 Amplitude 1 (%)":dbl=30.0 min=0.0 max=75.0 step=1.0
  in  "BD 2 Frequency 3 (MHz)":dbl=26.0 min=50.0 max=100.0 step=1.0 format="%#_6p"
  in  "BD 1 Frequency 3 (MHz)":dbl=70.0 min=50.0 max=100.0 step=1.0 format="%#_6p"
  in  "BD 2 Frequency 2 (MHz)":dbl=26.0 min=50.0 max=100.0 step=1.0 format="%#_6p"
  in  "BD 2 Frequency 1 (MHz)":dbl=26.0 min=50.0 max=100.0 step=1.0 format="%#_6p"
  in  "Not-Interlacing Set":enum32{"Set 1", "Set 2", "Set 3"}(radio)
  in  "Interlace":bool=TRUE
  in  "Trap 2 ON":bool=TRUE
  in  "Trap 3 ON":bool
  in  "Scan axis 2":bool=TRUE
  in  "Osc. freq. (Hz)":dbl=0.25
  in  "Osc. amp. (MHz)":dbl=2.0 format="%1_3g"
  out "Coords":T7
  in  "Manipulation Scaling":cluster{"Horizontal":dbl, "Vertical":dbl}={"Horizontal"=0.075, "Vertical"=0.01}
  in  "Freq or Amp switch first":bool=TRUE
  in  "Swap F1 and F2":bool
  in  "Freq switch delay":u16
  in  "Amp switch delay":u16=5
  in  "Period":i64=2
  in  "MCL Step Increment (V_int)":dbl=3.0
  out "Time to Finish All (min)":dbl=0.122877 format="%#_2p"
  in  "Scan Speed (nm/s)":dbl=100.0
  in  "Scan Range (nm)":dbl=369.00000000000034
  in  "Step Size (nm)":dbl=1.0
  in  "MCL/AOM Scale Tweak":dbl=1.0
  in  "MCL Step Position Ratio":dbl=0.5
  in  "Move MCL Also?":bool=TRUE
  out "Final sep (nm)":dbl=4587.0
  out "Initial sep (nm)":dbl=4218.0
  out "Save index":dbl=22.0
  out "Final delta (MHz)":dbl=44.0
  out "Initial delta (MHz)":dbl=41.0
  out "Final freq. (MHz)":dbl=50.0
  out "Initial freq. (MHz)":dbl=53.0
  in  "Saved AOD Raster Scan Parameter Sets":T8(array[cluster])=[{"Scan Range AOD (nm) 2"=500.0, "Step Size AOD (nm) 2"=1.0, "Scan Speed AOD (nm/s) 2"=100.0, "Number of scans (AOD) 2"=1, "Label"="offset curve"}, {"Scan Range AOD (nm) 2"=420.0, "Step Size AOD (nm) 2"=1.0, "Scan Speed AOD (nm/s) 2"=100.0, "Number of scans (AOD) 2"=1, "Label"="hp raster check"}, {"Scan Range AOD (nm) 2"=6.8, "Step Size AOD (nm) 2"=0.34, "Scan Speed AOD (nm/s) 2"=0.34, "Number of scans (AOD) 2"=1, "Label"="3.4 kbp - 1 bp steps"}]
  in  "Load parameters":bool
  out "Scan Range (MHz)":dbl=-3.0000000000000027
  in  "Restart DMA? (AOD)":bool=TRUE caption="Restart DMA?"
  out "Incr. int (AOD)":i64=-7759651845
  out "Time/Scan (s) (AOD)":dbl=3.68631 format="%#_2p"
  out "Data points/scans":dbl=491508.0
  out "Data points/scan (f/b)":dbl=491508.0
  in  "Save scans":bool=TRUE
  out "AOD Scan I":u64 caption="Scan I"
  in  "Continuous AOD Scanning":bool caption="Continuous Scanning"
  in  "Abort AOD Scan":bool caption="Abort Scan"
  in  "Scan BD":bool=TRUE
  out "Cycles/step (AOD)":u64=666 format="%.3p"
  in  "Number of F/B Scans (AOD)":u16=1 min=1
  out "Scan steps (AOD)":u64=369
  out "Scan Increment (MHz)":dbl=-0.008152173913043485
  out "AOD Scanning":bool caption="Scanning"
  in  "Start AOD Scan":bool caption="Start Scan"
  out "N sets should be saved":dbl=24.5754
  out "Progress 2":u16(slide) caption="Progress" scale=0.0..100.0
  in  "Abort save 2":bool caption="Abort save"
  in  "Trap 1 Bead Size (nm)":dbl=2100.0
  in  "Trap 2 Bead Size (nm)":dbl=2100.0
  out "MCL Count":dbl=230502201.82069838
  in  "All FB On/Off":bool
  in  "AI2 to Setpoint":cluster{"Set 1":bool, "Set 2":bool}
  out "AI2 (V)":cluster{"Set 1":dbl, "Set 2":dbl}={"Set 1"=-0.0012207403790398877, "Set 2"=0.004577776421399579}
  in  "Reset Feedback":cluster{"Set 1":bool, "Set 2":bool}
  in  "PID Gains":T9={"Set 1"={"proportional gain (Kc)"=0, "integral gain (Kc*Ts/Ti)"=5, "derivative gain (Kc*Td/Ts)"=0}, "Set 2"={"proportional gain (Kc)"=0, "integral gain (Kc*Ts/Ti)"=5, "derivative gain (Kc*Td/Ts)"=0}}
  in  "Feedback On/Off":cluster{"Set 1":bool, "Set 2":bool}={"Set 1"=TRUE, "Set 2"=TRUE}
  in  "Set SP to Reading":bool
  out "Trap X (AI1)":T10={"Trap 1"=-1.0, "Trap 2"=0.899993896484375}
  in  "Trap Pos FB SP":fxp<+/-,16,1>=-0.092803955078125 caption="Setpoint"
  in  "Trap Pos. FB ON":bool
  in  "Reset Trap Pos. FB":bool
  out "Trap Positions":waveform(dbl)[](graph)=[{"t0"=timestamp(12.90000000000001 s since 1904-01-01), "dt"=0.15, "Y"=[-1.7479351299698465e-12, -1.7479351299698465e-12], "attributes"=variant("NI_ChannelName"=variant(string "Trap 1 Pos."))}, {"t0"=timestamp(12.90000000000001 s since 1904-01-01), "dt"=0.15, "Y"=[6.991740519879386e-12, 6.991740519879386e-12], "attributes"=variant("NI_ChannelName"=variant(string "Trap 2 Pos."))}]
  in  "Tab Control 8":enum32{"Main Setting", "Details"}(tab)
  in  "Trap Pos FB Int Count":u16=100
  in  "Trap Pos. FB Gains":T11={"proportional gain (Kc)"=10.0, "integral gain (Kc*Ts/Ti)"=10.0, "derivative gain (Kc*Td/Ts)"=0.0} {"proportional gain (Kc)" format="%.11g"; "integral gain (Kc*Ts/Ti)" format="%.11g"; "derivative gain (Kc*Td/Ts)" format="%.11g"}
  in  "Trap Pos. FB Offset Factor":i64
  in  "Trap Pos FB Negate Action":bool
  in  "Trap Pos. FB Mult Factor":i64=33554432
  in  "Trap Pos. AI1 X Pre-scale":u16
  in  "Trap Pos. FB Range":T12={"output high"=0.999969482421875, "output low"=-1.0}
  out "Trap Pos FB Int Signal":fxp<+/-,24,9> format="%.18g"
  out "Trap Pos FB Int-Norm Signal":fxp<+/-,16,1> format="%.16g"
  in  "Set SP Using...":bool
  in  "Trap Pos FB Monitor\nT1 or T2":bool
  out "Trap X AI1 (DMA)":T13={"Set 1"=0.999969482421875, "Set 2"=0.999969482421875}
  in  "N El. to Ave.":dbl=10000.0
  out "Trap Pos FB Action":i64
  out "Action (%)":dbl(knob) scale=-100.0..100.0
  in  "Trap Pos. FB Out Scale 2^n":u8=23 caption="Action Scale"
  out "Mean T1 Position (nm)":dbl=-1.7479351299698465e-12 caption="Mean T1 (nm)" format="%0.2f"
  out "Trap 1 Position RMS (A)":dbl caption="RMS (Ang)"
  in  "Tab Control 3":enum32{"Timing", "MCL Scan", "Analog Out"}(tab)
  out "APD 2 Gate Late Counter":u32
  out "APD 2 Gate Relative Phase":i16
  in  "Phase Adj. (APD 2 Gate)":i16=20
  in  "Initial Phase Adjustment (APD 2 Gate)":i16=55
  out "APD 1 Gate Late Counter":u32
  in  "- phase (APD 1 Gate)":bool
  in  "+ phase (APD 1 Gate)":bool
  out "APD 1 Gate Relative Phase":i16
  in  "Phase Adj. (APD 1 Gate)":i16=20
  in  "Initial Phase Adjustment (APD 1 Gate)":i16=60
  in  "Save APD Data\nwith Trap Data":bool=TRUE
  out "APD FIFO Elements Remaining":u32
  in  "- phase (APD Acq)":bool
  in  "+ phase (APD Acq)":bool
  out "APD Acq Late Counter":u32
  out "APD Acq Relative Phase":i16
  in  "Phase Adj. (APD Acq)":i16=20
  in  "Initial Phase Adjustment (APD Acq)":i16
  in  "Invert APD Gate":bool caption="Invert Gate"
  in  "APD Gate OFF Count":u32=450 caption="Gate OFF Count"
  in  "APD Gate ON Count":u32=150 caption="Gate ON Count"
  in  "APD Gate":enum32{"ON", "OFF", "Interlace"}(radio)=enum."Interlace"
  in  "APD Integration Time (s)":dbl=0.01 caption="Integration Time (s)"
  out "APD Acq Rate (Hz)":dbl=100.0 caption="Rate (Hz)"
  out "APD Samples/FIFO Acq.":dbl=30.0
  out "APD Elements/DMA read":u32=60
  out "APD Int. Count":u32=400000 format="%.0p"
  in  "+ phase (APD 2 Gate)":bool
  in  "- phase (APD 2 Gate)":bool
  in  "Tab Control 5":enum32{"PSD X", "PSD Y", "Other Data Channel"}(tab)
  out "Data map":dbl[][](graph)
  in  "Channel":i32=4
  in  "Abort MCL Scan":bool
  out "MCL Scan I":u64
  out "MCL Scanning":bool
  in  "Start MCL Scan":bool
  out "wait to reset values":bool
  in  "Tab Control 4":enum32{"Scan Settings", "MCL FPGA Loop Timing"}(tab)
  out "Total Time (s)":dbl=48.0
  in  "Scan lines (y)":u64=20
  in  "Fast Scan Dir":bool=TRUE
  in  "2D or 1D Scan":bool=TRUE
  out "Initial X":dbl
  out "Initial Y":dbl
  out "Time/f+b scan (s) (MCL)":dbl=2.4 caption="Time/scan (s)"
  in  "Number of scans (MCL)":u64=1 caption="Scans"
  in  "Scan steps (MCL)":u64=40 caption="Scan steps (x)"
  in  "N APD Samp/step":dbl=3.0
  in  "Scan Range (V)\n(of steps)":dbl=3.5
  in  "Restart DMA? (MCL)":bool=TRUE caption="Restart DMA?"
  in  "Continuous MCL Scanning":bool caption="Cont. Scanning"
  in  "Center Scan":bool=TRUE
  in  "Save Data (MCL)":bool=TRUE caption="Save Data"
  out "Actual Incr. int (MCL)":i16=294 caption="Incr. int"
  out "Desired incr (int)":dbl=294.0628205128205
  out "Desired Scan Incr (V)":dbl=0.08974358974358974
  out "N sets should be saved (MCL)":dbl=160.0 caption="N sets should be saved"
  out "Data points/scans (MCL)":dbl=4800.0 caption="Data points/scans"
  out "Data points/scan (f+b)":dbl=240.0 caption="points/scan (f+b)"
  out "Cycles/step (MCL)":u64=2000 caption="Cycles/step" format="%.0p"
  out "Actual MCL Inc (V)":dbl=0.08972441785943175
  in  "Phase adjust (MCL)":i16 caption="Phase adjust"
  out "Relative Phase (MCL)":i16 caption="Relative Phase"
  in  "Initial Phase Adj. (MCL)":i16 caption="Initial Phase Adj."
  in  "Update Count (MCL)":u32=600
  in  "+ phase (MCL)":bool
  in  "- phase (MCL)":bool
  out "MCL Late Counter":u32
  in  "APD 1 AO Mult.":i16=1 min=1
  in  "APD 2 AO Mult.":i16=1 min=1
  in  "Tab Control 7":enum32{"Green FB Signals", "Slow MCL Scan"}(tab)
  out "Green FB Plot":dbl(graph)=10.0
  out "MCL Scan 2":cluster{"Begin (V)":dbl, dbl, dbl[]}(graph)
  out "MCL Scan":cluster{"Begin (V)":dbl, dbl, dbl[]}(graph)
  in  "Green laser mode":enum32{"Laser ON", "Laser OFF", "Interlace"}(radio)
  in  "GI Frequency, ON count":u32=150 min=1 step=1
  in  "Invert GI":bool
  out "GI Late Counter":u32
  in  "Phase adj. (GI)":i16=5
  out "GI relative phase":i16
  in  "+ phase (GI)":bool
  in  "Initial Phase Adjustment (GI)":i16=19
  in  "GI Frequency, OFF count":u32=450 min=1 step=1
  in  "- phase (GI)":bool
  out "Green FB Signals (V)":cluster{"Y":dbl, "X":dbl, "Sum":dbl}={"Y"=1.0, "X"=1.0, "Sum"=10.0}
  out "Relative phase (Green FB)":i16
  in  "+ phase (Green FB)":bool
  in  "- phase (Green FB)":bool
  in  "Green FB Count":u32=600
  in  "Phase adj. (Green FB)":i16=10
  in  "Initial Phase Adjustment (Green FB)":i16=50
  in  "Green FB On/Off":bool
  in  "Current When FB OFF (%)":dbl=10.0 min=0.0 max=100.0 step=1.0
  in  "Green int current ON count adj":u32=150
  in  "Green FB Gains":T14={"proportional gain (Kc)"=10, "integral gain (Kc*Ts/Ti)"=5, "derivative gain (Kc*Td/Ts)"=0}
  in  "Green FB Setpoint (mV)":dbl=100.0
  in  "- phase (GI) 2":bool
  in  "Initial Phase Adjustment (GI) 2":i16=-100
  in  "+ phase (GI) 2":bool
  out "GI relative phase 2":i16
  in  "Phase adj. (GI) 2":i16=20
  out "GI Late Counter 2":u32
  in  "Trap Position FIFO Depth":u32=300000 format="%.0p"
  in  "# Samples/trap":u32=20000 format="%.0p"
  out "Trap AI Elements/DMA read":u32=320000 format="%.0p"
  out "Ave. Rate (Hz)":dbl=200000.0 format="%#_6p"
  out "Trap AI FIFO El. Rem.":u32 format="%.0p"
  in  "Phase adj. (AI1)":i16
  out "Relative phase (AI1)":i16
  in  "+ phase (AI1)":bool
  in  "- phase (AI1)":bool
  out "Late Counter (AI1)":u32
  in  "Initial Phase Adjustment (AI1)":i16=180
  out "AI rate (Hz)":dbl=200000.0 format="%#_6p"
  in  "AI Count (ticks)":u32=200
  out "# Samples/channel":u32=40000 format="%.0p"
  in  "Trap AI FIFO Depth":u32=340000 format="%.0p"
  in  "Detector Type":string(combo)="UCB Fleezers 052511"
  in  "N Acq Sets (Traps + Fl.)":i16=3
  in  "Sets to FIFO (Traps)":T15={"Set 1"=TRUE, "Set 2"=TRUE, "Set 3"=FALSE}
  in  "FPGA Ave.":dbl=1.0 min=1.0 step=1.0
  out "Ave. Period (s)":dbl=5e-06 format="%#_6p"
  out "DMA Update Period (s)":dbl=0.3
  out "FPGA Averaging":bool
  out "Trap Sets":u32=2
  out "Counts/DMA":dbl=12000000.0 format="%#_6p"
  out "Trap Pos FIFO El Remaining":u32=141
  out "Trap Pos Elements/DMA read":u32=120000 format="%.0p"
  out "Trap AI FIFO Timeout":u16
  out "Trap Pos FIFO Timeout":u16
  out "Waveform Chart":i32(graph)=320000
  out "error out 2":errorcluster
  in  "Lost Tether Alarm Threshold (pN)":dbl=0.5
  in  "AOM X Cal (nm/MHz)":dbl=168.33
  in  "MCL X Cal (nm/V)":dbl=1070.0
  out "X RF Amplitude Limits (%)":T16={"Minimum"=0.0, "Maximum"=50.0, "Increment"=1.0}
  out "X RF Frequency Limits (MHz)":T16={"Minimum"=50.0, "Maximum"=100.0, "Increment"=1.0}
  out "Y RF Frequency Limits (MHz)":T16={"Minimum"=50.0, "Maximum"=100.0, "Increment"=1.0}
  out "Y RF Amplitude Limits (%)":T16={"Minimum"=0.0, "Maximum"=50.0, "Increment"=1.0}
  in  "Manip. X?":bool=TRUE
  in  "Manip. Y?":bool
  in  "Force Manip Abort":bool
  out "Read cal error":errorcluster
  in  "DAQ Delay (ms)":u32=1000
  in  "Start Scan":bool
  in  "Scan axis":bool
  in  "Osc. amp. (V)":dbl=5.0
  in  "Osc. center (V)":dbl=5.0
  in  "Osc. freq. (Hz) 2":dbl=1.0
  in  "MCL Mode":u16(ring) items=["Manual Positioning", "Sinusoidal Wave", "Linear Scan"]
  in  "Begin (V)":dbl
  in  "End (V)":dbl=10.0
  in  "N Points":dbl=20.0
  in  "Delay to Interlace (s)":dbl
  in  "Delayed Interlace Start":bool
  in  "Read Lateness and Rel Phase":bool
  out "Vec Mean of T1 T2":dbl[](array[numeric])=[nan, nan]
  in  "Cal read wait (s)":u32=5
  out "Time tether formed":timestamp=timestamp(3371146929.513132 s since 1904-01-01)
  in  "Chemyx Syringe Pump Serial Port":refnum<visa-resource-name>="ASRL3::INSTR"
  in  "Limit Min (MHz)":dbl=10.0 caption="Min (MHz)"
  in  "Limit Max (MHz)":dbl=16.0 caption="Max (MHz)"
  in  "Limits Enable":bool=TRUE caption="Enable"
  out "AI labels":string[](array[string])=["T1 Y", "T1 X", "T1 Sum", "T2 Y", "T2 X", "T2 Sum", "T1 FB X", "T2 FB Sum", "T2 FB X", "T2 FB Sum", "PSD Y", "PSD X", "PSD Sum"]
  in  "Save Trap Pos. Data":bool=TRUE
  in  "ESP Port":refnum<visa-resource-name>="COM22"
  in  "Locations":i32(listbox)=1
  out "Selected Location":cluster{"x":string, "y":string, "z":string}={"x"="0.19233\r\n", "y"="0.00156\r\n", "z"="0.20615\r\n"}
  in  "Capture":bool
  in  "Save":bool
  in  "Goto Top (F6)":bool
  in  "Goto Exp (F8)":bool
  in  "Goto Bottom (F7)":bool
  in  "Axis 3":string="0.00500\r\n"
  in  "Axis 2":string="0.00500\r\n"
  in  "Axis 1":string="0.00500\r\n"
  in  "Axis 3":string="0.20000\r\n"
  in  "Axis 2":string="0.20000\r\n"
  in  "Axis 1":string="0.20000\r\n"
  in  "Activate Joystick":bool
  in  "ESP ZL-Limit":string="-0.09900"
  in  "ESP ZR-Limit":string="0.09900"
  out "Z Pos Pos":string="0.21899\r\n"
  out "Y Pos":string="0.00713\r\n"
  out "X Pos":string="0.20503\r\n"
  in  "error in":errorcluster
  out "error out":errorcluster
  out "Z motion":string
  out "Y Motion":string
  out "X Motion":string
  # "After"
  # "During"
  # "Trap On?"
  # "BD Flow ON?"
  # "Samp Flow ON?"
  # "1"
  # "2"
  # "Trap Display:"
  # "APD Display:"
  # "originally 10k"
  # "Trap Manipulation"
  # "DAQ"
  # "Data Saving"
  # "Central frequency 75 MHz"
  # "F9"
  # "Bead Calibration"
  # "F10"
  # "F4"
  # "Press F12 to move stage\nwith the mouse. F12 to cancel."
  # "F5"
  # "F6"
  # "F7"
  # "F8"
  # "Harvard Pump\n(sample channel for flow exp)"
  # "Chemyx Pump 2"
  # "Units: \n1 = ml/m\n2 = ml/h\n3 = ul/m\n4 = ul/h"
  # "Rate param is ul/h\nVolume param is ul"
  # "X"
  # "Y"
  # "Oscillate Set 2 freq. (debugging)"
  # "BD 1"
  # "BD 2"
  # "AOD Raster Scan"
  # "Approx. trap separations"
  # "X"
  # "Y"
  # "DON'T TURN ON\nUNTIL YOU CLOSE\nTHE LOOP"
  # "FPGA\nreading"
  # "DMA\ntransfer"
  # "APD Gates"
  # "APD 2"
  # "APD 1"
  # "X"
  # "2D"
  # "Y"
  # "1D"
  # "Green Laser Interlacing"
  # "Green FB Measurement"
  # "Digital Gate"
  # "Current Analog Control"
  # "was 87"
  # "originally 600k"
  # "Total AI Rates (NOT rates/trap)"
  # "originally 20k"
  # "(Samples/trap x Trap Sets)"
  # "(Samples/channel x\n8 if averaging (8 channels)\n4 if no averaging)"
  # "Trap 1"
  # "Trap 2"
  # "Flour./Trap 3"
  # "External Video Window"
  # "MCL Position Debugging"
  # "Temporary Control Storage\n(these used to be somewhere else, still want to keep them)"
  # "Y"
  # "X"
  # "Trap Position Difference Limits"
  # "Joystick Control"
  # "Setting Limit for the z-axis"
  # "Current Location"
  # "Save Positions of Cambers"
  # "Errors detected in determing Current Location"
  # "High Jog Velocity"
  # "Low Jog Velocity"
  # "Select the chamber to go to"
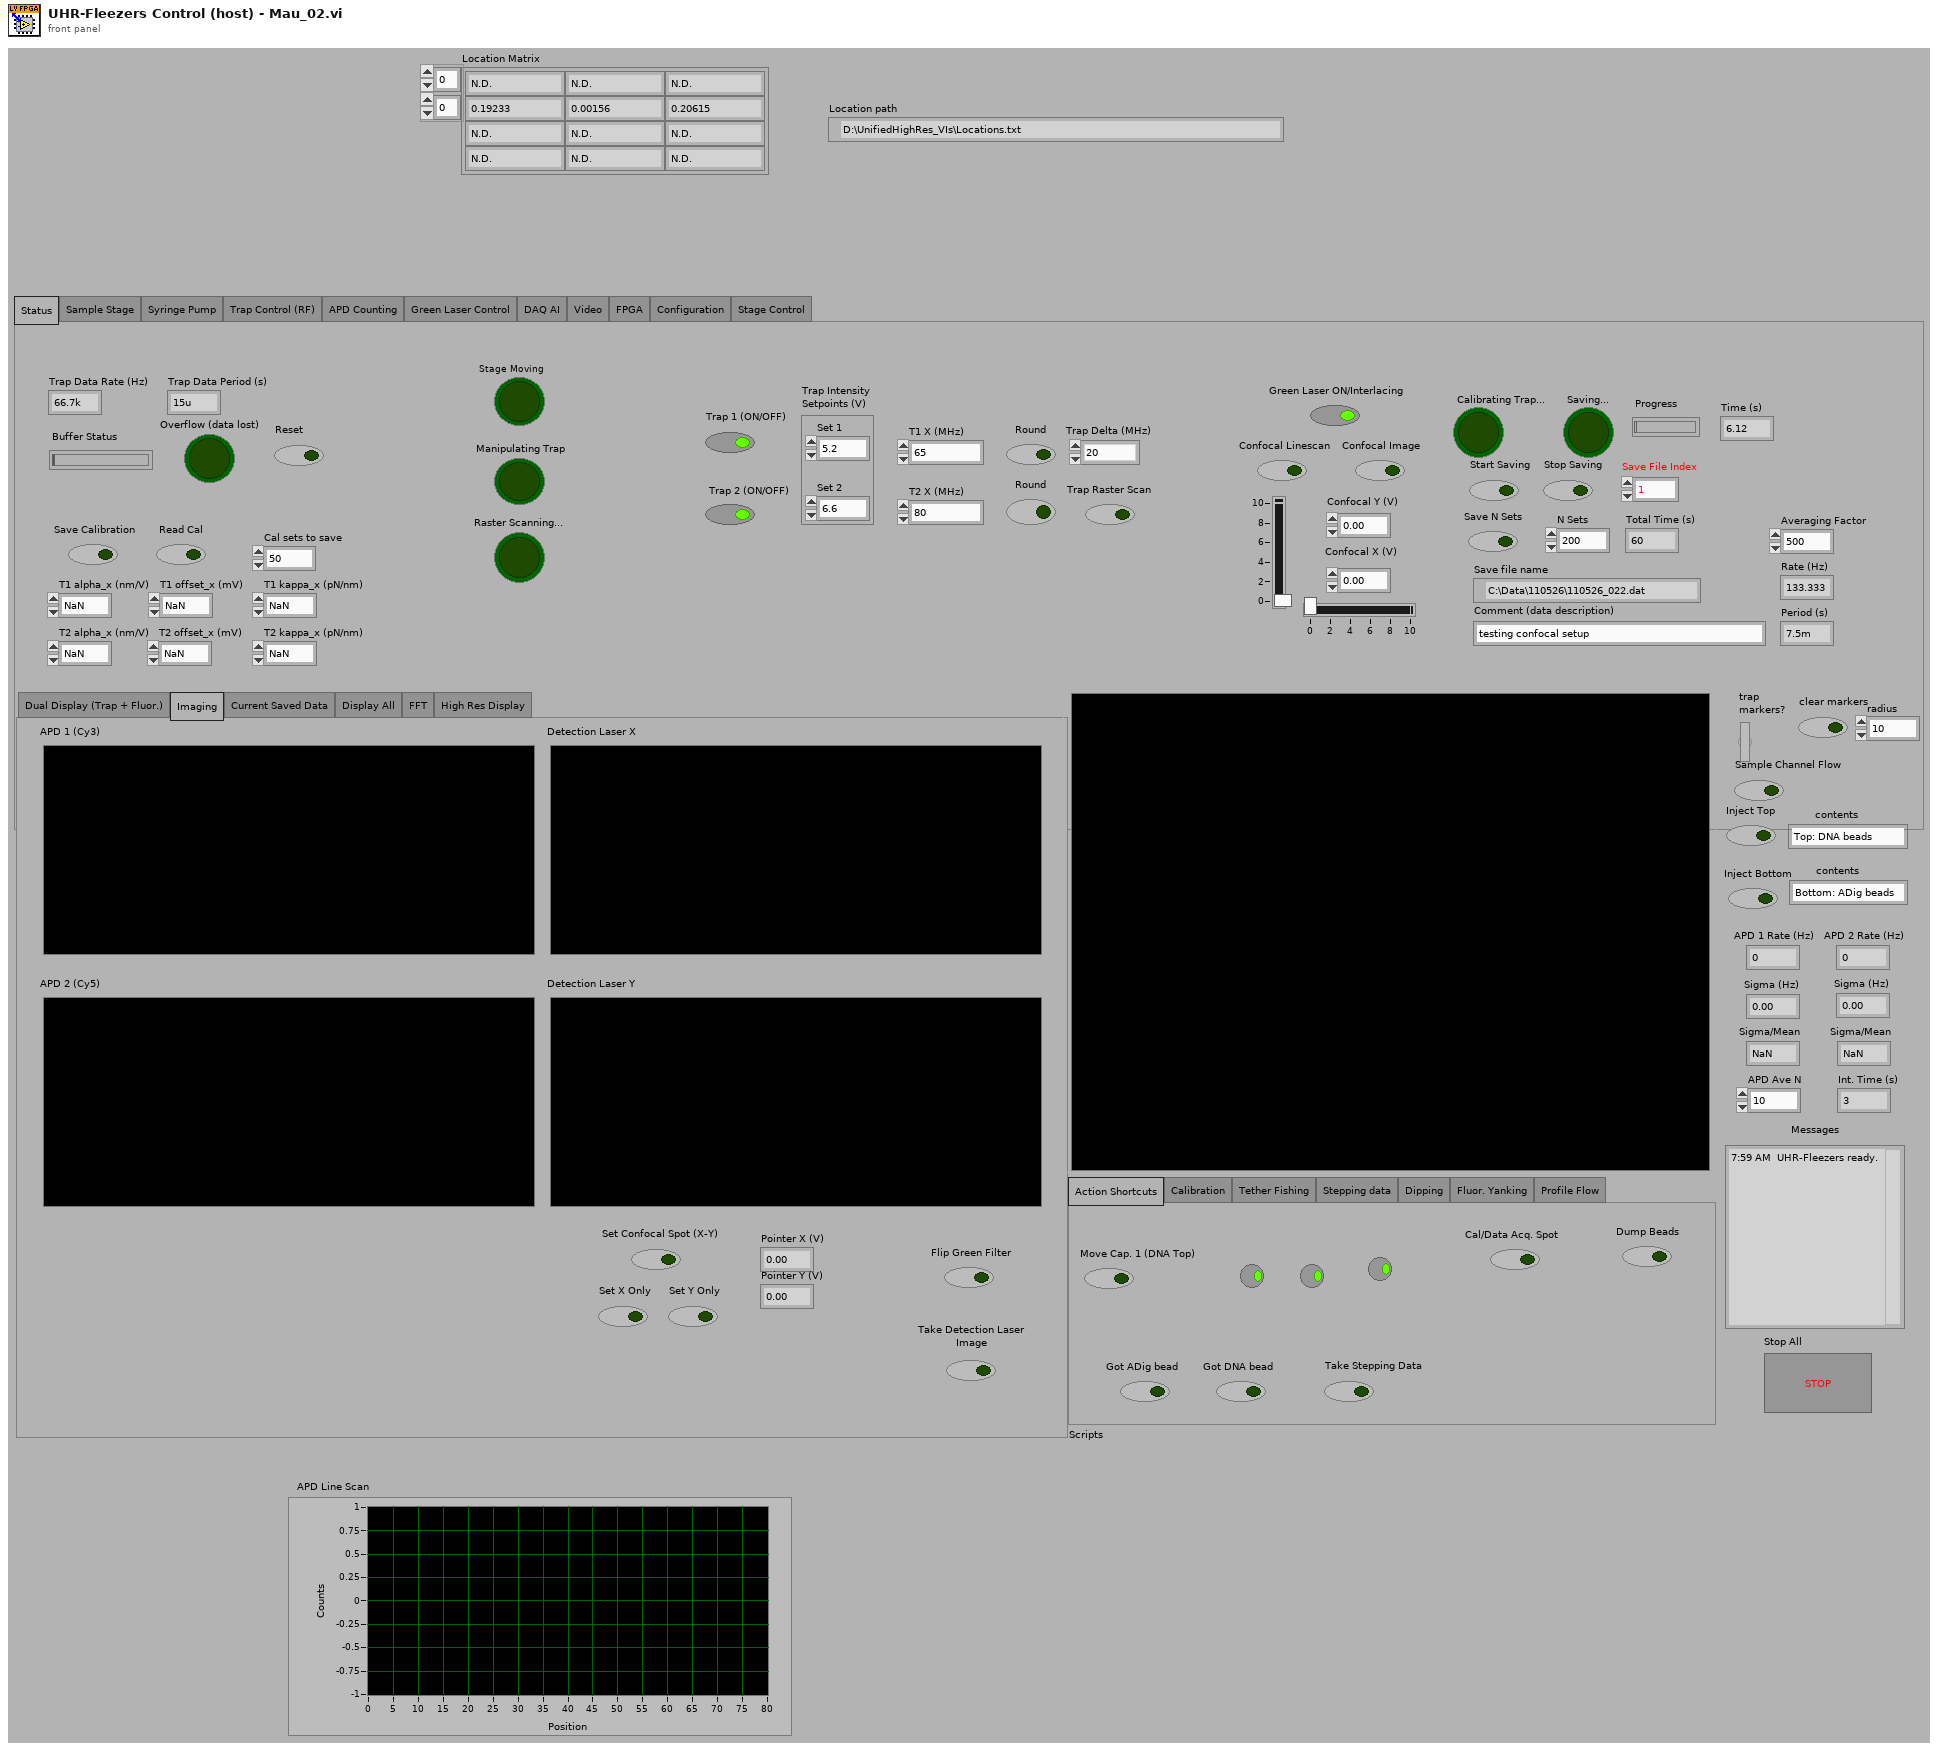
[diagram p1: front panel]
types:
  T1 = enum32{"Action Shortcuts", "Calibration", "Tether Fishing", "Stepping data", "Dipping", "Fluor. Yanking", "Profile Flow"}
  T2 = typedef "IMAQ Image.ctl" = refnum<image>
  T3 = enum32{"Dual Display (Trap + Fluor.)", "Imaging", "Current Saved Data", "Display All", "FFT", "High Res Display"}
  T4 = enum32{"Status", "Sample Stage", "Syringe Pump", "Trap Control (RF)", "APD Counting", "Green Laser Control", "DAQ AI", "Video", "FPGA", "Configuration", "Stage Control"}
  T5 = cluster{"Pump 1":cluster{"Diameter (mm)":dbl, "Units":dbl, "Volume":dbl, "Rate":dbl}, "Pump 2":cluster{"Diameter (mm)":dbl, "Units":dbl, "Volume":dbl, "Rate":dbl}, "Pump 3":cluster{"Diameter (mm)":dbl, "Units":dbl, "Volume":dbl, "Rate":dbl}}
  T6 = enum32{"IR Laser Interlacing (Direct RF Board Control Method)", "AOD Raster Scan", "Feedback on Trap Intensity", "Feedback on Trap Position"}
  T7 = typedef "LVPoint32TypeDef.ctl" = cluster{"Horizontal":i32, "Vertical":i32}
  T8 = cluster{"Scan Range AOD (nm) 2":dbl, "Step Size AOD (nm) 2":dbl, "Scan Speed AOD (nm/s) 2":dbl, "Number of scans (AOD) 2":u16, "Label":string}[]
  T9 = cluster{"Set 1":cluster{"proportional gain (Kc)":i16, "integral gain (Kc*Ts/Ti)":i16, "derivative gain (Kc*Td/Ts)":i16}, "Set 2":cluster{"proportional gain (Kc)":i16, "integral gain (Kc*Ts/Ti)":i16, "derivative gain (Kc*Td/Ts)":i16}}
  T10 = cluster{"Trap 1":fxp<+/-,16,1>, "Trap 2":fxp<+/-,16,1>}
  T11 = cluster{"proportional gain (Kc)":fxp<+/-,16,8>, "integral gain (Kc*Ts/Ti)":fxp<+/-,16,8>, "derivative gain (Kc*Td/Ts)":fxp<+/-,16,8>}
  T12 = cluster{"output high":fxp<+/-,16,1>, "output low":fxp<+/-,16,1>}
  T13 = cluster{"Set 1":fxp<+/-,16,1>, "Set 2":fxp<+/-,16,1>}
  T14 = cluster{"proportional gain (Kc)":i16, "integral gain (Kc*Ts/Ti)":i16, "derivative gain (Kc*Td/Ts)":i16}
  T15 = cluster{"Set 1":bool, "Set 2":bool, "Set 3":bool}
  T16 = typedef "LVMinMaxIncTypeDef.ctl" = cluster{"Minimum":dbl, "Maximum":dbl, "Increment":dbl}
  T17 = typedef "Image Type" = u32
  T18 = typedef "nirio_resource_hc.ctl" = tag
  T19 = typedef "openfpgaref.8.6.ctl" = refnum<k20>
  T20 = enum16{"CONNECT", "INITIALIZE VALVES", "DISCONNECT", "MOVE VALVE"}
  T21 = cluster{"New Image":T2, "New Image":T2, "New Image":T2, "New Image":T2}
  T22 = cluster{"Location Matrix[0]":string, "Location Matrix[1]":string, "Location Matrix[2]":string}
  T23 = enum16{"open", "replace", "create", "open or create", "replace or create", "replace or create with confirmation"}
  T24 = typedef "XDNodeRunTimeDep.lvlib/timing_clust.ctl" = cluster{"Expected End [f-1]":u64, "Actual End [f-1]":u64, "Finished Late? [f-1]":bool, "Expected End [i-1]":u64, "Actual End [i-1]":u64, "Finished Late? [i-1]":bool, "Expected Start [i]":u64, "Actual Start [i]":u64, "Expected Start [f]":u64, "Actual Start [f]":u64, "Source Name":string, "Structure Name":string, "Period":i64, "Deadline":i64, "Offset":i64, "Start":i64, "Priority":i32, "Timeout":i32, "Mode":T25, "Wakeup Reason":T26, "Error":errorcluster, "Source Type":string, "Secondary Source Type":string, "Global End Time":u64, "Global Start Time":u64, "Frame Duration":u64, "Iteration Duration":u64, "Assigned CPU":i32, "I/O Scan Engine Mode":u32}
  T25 = typedef "XDNodeRunTimeDep.lvlib/nitl_modes.ctl" = enum32{"No Change", "Process missed periods, maintain original phase", "Discard missed periods, maintain original phase", "Process missed periods, ignore original phase", "Discard missed periods, ignore original phase"}
  T26 = typedef "XDNodeRunTimeDep.lvlib/wakeup.ctl" = enum32{"Normal", "Aborted", "Asynchronous wakeup", "Timing source error", "Timed loop error", "Timeout"}
  T27 = cluster{"[0]":i32, "[1]":i32, "[2]":i32, "[3]":i32}
  T28 = cluster{"[0]":i32, "[1]":i32, "[2]":i32, "[3]":i32}[]
  T29 = enum16{"big-endian, network order", "native, host order", "little-endian"}
  T30 = cluster{"Scan Range AOD (nm) 2":dbl, "Step Size AOD (nm) 2":dbl, "Scan Speed AOD (nm/s) 2":dbl, "Number of scans (AOD) 2":u16, "Label":string}
  T31 = cluster{"[0]":dbl, "[1]":dbl, "[2]":dbl, "[3]":dbl, "[4]":dbl, "[5]":dbl}
  T32 = cluster{"Diameter (mm)":dbl, "Units":dbl, "Volume":dbl, "Rate":dbl}
  T33 = cluster{"Left":i32, "Top":i32, "Width":u32, "Height":u32}
  T34 = cluster{cluster{"Left":i32, "Top":i32, "Width":u32, "Height":u32}}[]
  T35 = enum32{"Normal Display", "Dual Display (APD)", "FFT", "High Res Display"}
  T36 = cluster{"Origin Pixel":cluster{"X":sgl, "Y":sgl}, "Angle Relative to Horizontal (deg)":sgl, "Axis Reference":u32}
  T37 = typedef "Simple Grid Descriptor" = cluster{"X Step":sgl, "Y Step":sgl, "Unit":T38}
  T38 = typedef "Image Unit" = enum32{"Undefined", "Angström", "Micrometer", "Millimeter", "Centimeter", "Meter", "Kilometer", "Microinch", "Inch", "Feet", "Nautical miles", "Standard miles", "Steps"}
  T39 = cluster{"averaging mode":u16, "weighting mode":u16, "number of averages":u32}
  T40 = cluster{"dB On (F)":bool, "unwrap phase (F)":bool, "convert to degree (F)":bool}
  T41 = cluster{string, string, string, string, string, string, string, string}
  T42 = cluster{string, string, string, string, string, string, string, string, string, string, string, string}
  T43 = cluster{string, string, string, string, string, string, string, string, string, string, string, string, string}
  T44 = cluster{string, string, string, string, string, string, string, string, string, string, string, string, string, string}
  T45 = cluster{"BD 1 Frequency 1 (MHz)":dbl, "BD 1 Frequency 2 (MHz)":dbl}
  T46 = cluster{"f0":dbl, "df":dbl, "magnitude":dbl[]}[][]
  T47 = cluster{"Green FB Ch 0":i16, "Green FB Ch 1":i16, "Green FB Ch 2":i16}
  T48 = cluster{"Green FB Ch 0":dbl, "Green FB Ch 1":dbl, "Green FB Ch 2":dbl}
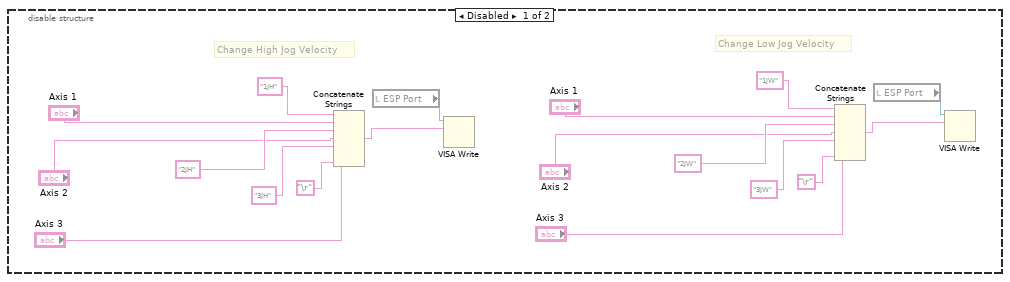
[diagram p2: hidden frame]
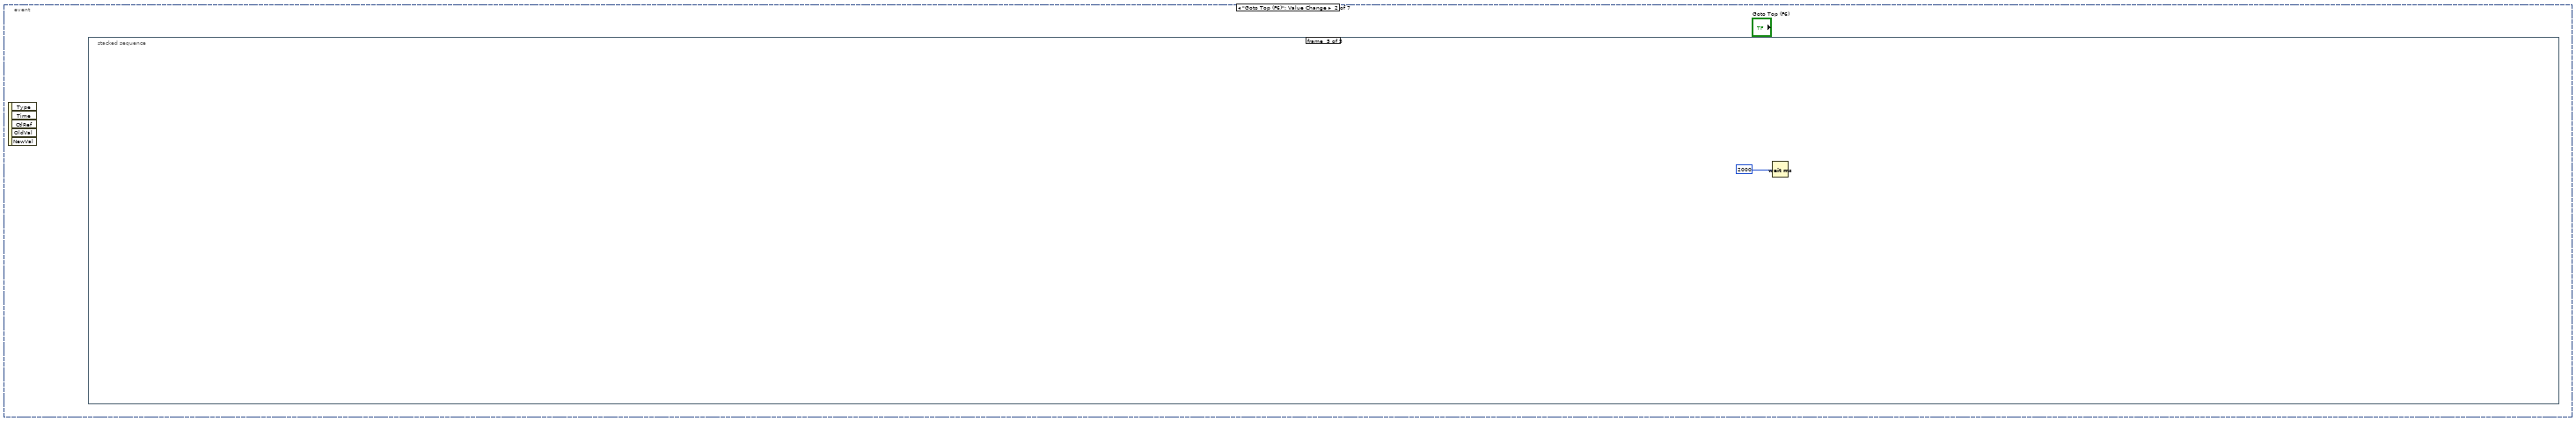
[diagram p4: hidden frame]
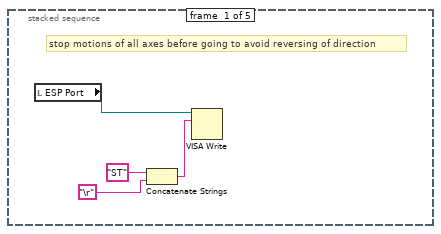
[diagram p5: hidden frame]
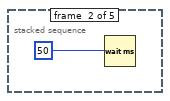
[diagram p6: hidden frame]
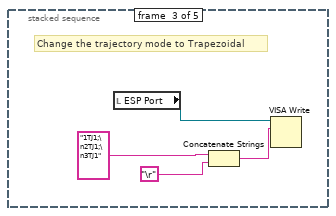
[diagram p7: hidden frame]
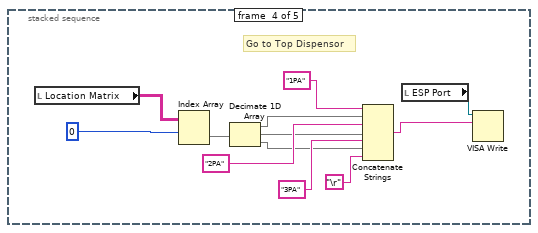
[diagram p8: hidden frame]
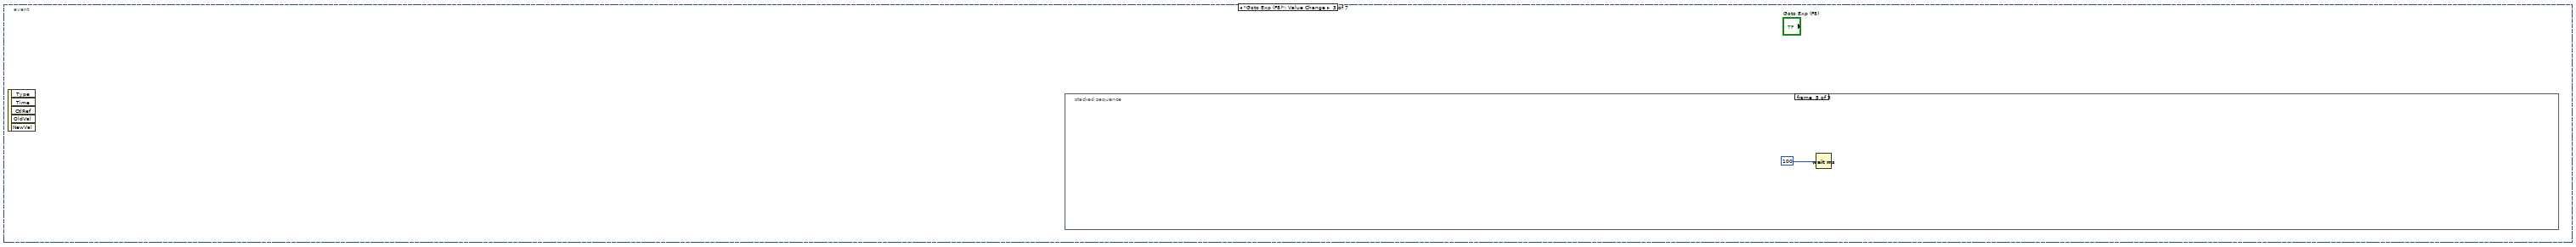
[diagram p9: hidden frame]
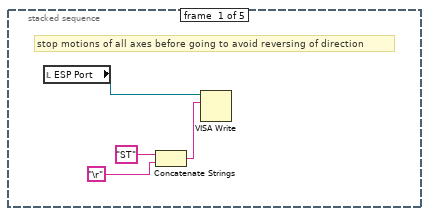
[diagram p10: hidden frame]
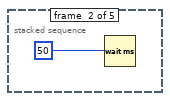
[diagram p11: hidden frame]
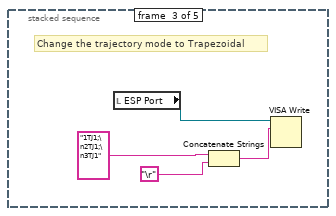
[diagram p12: hidden frame]
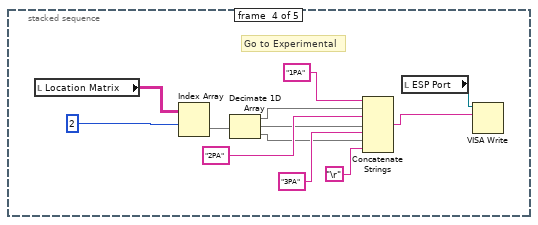
[diagram p13: hidden frame]
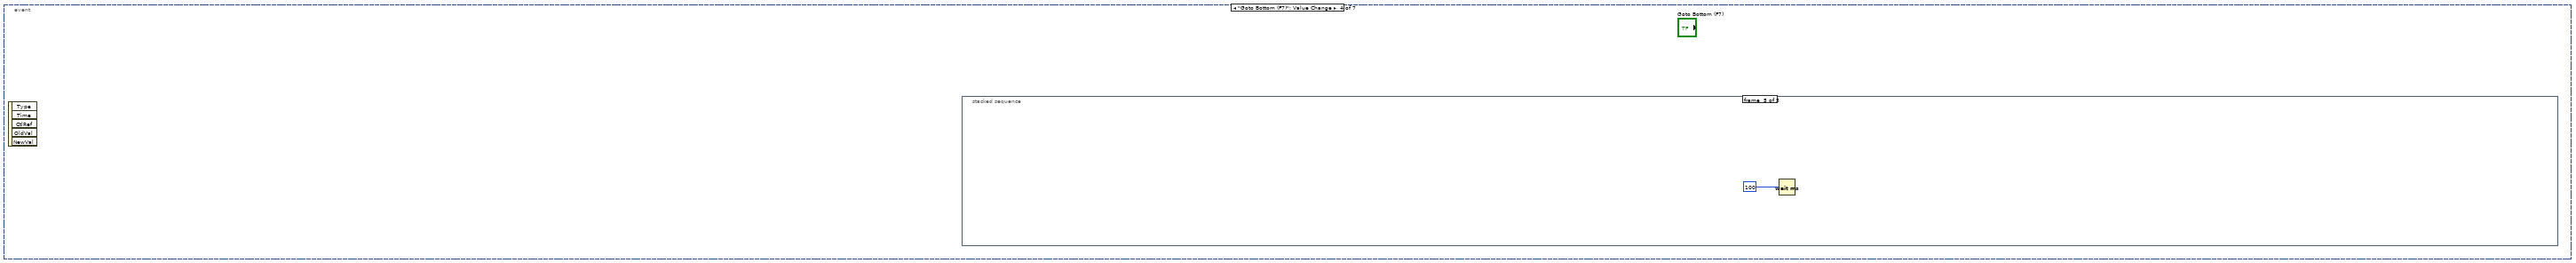
[diagram p14: hidden frame]
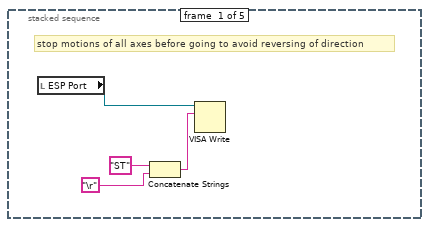
[diagram p15: hidden frame]
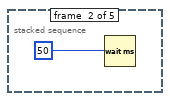
[diagram p16: hidden frame]
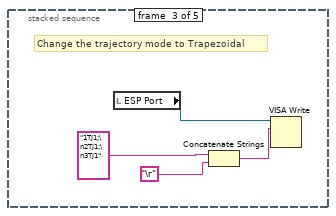
[diagram p17: hidden frame]
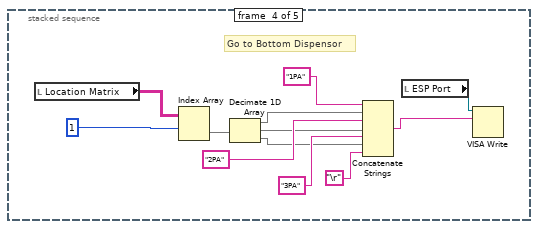
[diagram p18: hidden frame]
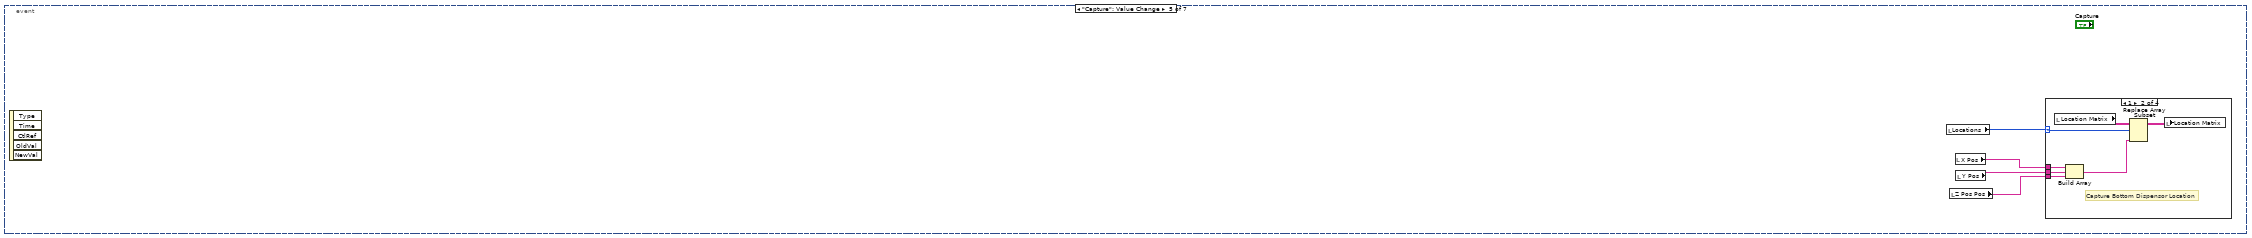
[diagram p19: hidden frame]
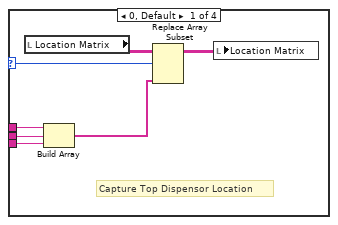
[diagram p20: hidden frame]
diagram:
  w64 = T17 2 items=["Grayscale (U8)", "Grayscale (I16)", "Grayscale (SGL)", "Complex (CSG)", "RGB (U32)", "HSL (U32)", "RGB (U64)", "Grayscale (U16)"] ("Image Type")
  w121 = cluster{"output high":i16, "output low":i16} {"output high"=3000, "output low"=0} ("FB output range 1")
  w196 = 10.0 ("y")
  w195 = 32767.0 ("y")
  w211 = 6.0  # clock mult.
  w212 = 49152000.0  # TCXO frequ.
  # "Initialize location matrix"
  n1 = Build Array("DIO count 1 (ticks)", "DIO count 2 (ticks)", "DIO count 3 (ticks)") -> (w110:u32[])
  n2 = Multiply(x="APD Integration Time (s)", y=40000000.0) -> (x*y=w128:dbl)
  n3 = Reciprocal(x="APD Integration Time (s)") -> (1/x=w125:dbl)
  n4 = local write "APD Acq Rate (Hz)"(w125) -> ()
  n5 = local read "AO1"() -> (w190:dbl)
  n6 = local read "AO2"() -> (w189:dbl)
  n7 = To Unsigned Long Integer(number=w128) -> (unsigned 32bit integer=w127:u32)
  "APD Int. Count" <- w127
  n8 = local read "Scan Increment (MHz)"() -> (w207:dbl)
  n9 = local read "Continuous MCL Scanning"() -> (w177:bool)
  n10 = local read "Fast Scan Dir"() -> (w176:bool)
  n11 = local read "Trap Intensity\nSetpoints (V)"() -> (w226:cluster{"Set 1":dbl, "Set 2":dbl})
  n12 = local read "Number of scans (MCL)"() -> (w178:u64)
  n13 = Multiply(x=w190, y=w195) -> (x*y=w192:dbl)
  n14 = Multiply(x=w189, y=w195) -> (x*y=w194:dbl)
  n15 = Divide(x=w192, y=w196) -> (x/y=w191:dbl)
  n16 = Divide(x=w194, y=w196) -> (x/y=w193:dbl)
  n17 = To Word Integer(number=w191) -> (16bit integer=w188:i16)
  n18 = To Word Integer(number=w193) -> (16bit integer=w187:i16)
  n19 = Not(x=w176) -> (.not. x?=w171:bool)
  n20 = local read "Cycles/step (MCL)"() -> (w179:u64)
  n21 = Multiply(x=w207, y=1000.0) -> (x*y=w214:dbl)
  n22 = local read "Scan steps (MCL)"() -> (w180:u64)
  n23 = local write "Trap Pos FIFO Timeout"(u16 0 ("Trap Pos FIFO Timeout")) -> ()
  n24 = local read "Desired Scan Incr (V)"() -> (w182:dbl)
  n25 = Scale By Power Of 2(n=48, x=w214) -> (x*2^n=w215:dbl)
  n26 = Multiply(x=w212, y=w211) -> (x*y=w210:dbl)
  n27 = Divide(x=w215, y=w210) -> (x/y=w209:dbl)
  n28 = local read "Number Interlace Sets"() -> (w103:u8)
  n29 = Split 1D Array(array=w110, index=w103) -> (first subarray=w112:u32[])  [unwired: 1 out]
  n30 = Add Array Elements(numeric array=w112) -> (sum=w111:u32)
  n31 = property on="AI Count (ticks)" class="DigNum (strict)"("Val(Sgnl)"="AI Count (ticks)") -> ()  [unwired: 2 in, 2 out]
  n32 = local read "# Samples/channel"() -> (w199:u32)
  n33 = local read "Number of F/B Scans (AOD)"() -> (w200:u16)
  n34 = To Quad Integer(1:w209) -> (0:w206:i64)
  n35 = local read "Not-Interlacing Set"() -> (w102:enum32{"Set 1", "Set 2", "Set 3"})
  n36 = To Unsigned Byte Integer(number=w102) -> (unsigned 8bit integer=w108:u8)
  n37 = Index Array(array=w110, index=w108) -> (element=w109:u32)
  n38 = local read "Feedback On/Off"() -> (w229:cluster{"Set 1":bool, "Set 2":bool})
  n39 = local read "PID Gains"() -> (w221:T9)
  n40 = Divide(x=40000000.0, y="AI Count (ticks)") -> (x/y=w168:dbl)
  n41 = Multiply(x=w182, y=32767.0) -> (x*y=w184:dbl)
  n42 = local read "Scan steps (AOD)"() -> (w205:u64)
  n43 = local read "All FB On/Off"() -> (w230:bool)
  n44 = local read "Cycles/step (AOD)"() -> (w204:u64)
  n45 = local write "AI rate (Hz)"(w168) -> ()
  n46 = Divide(x=w184, y=10.0) -> (x/y=w183:dbl)
  n47 = Multiply(x=w205, y=w204) -> (x*y=w203:u64)
  n48 = Multiply(x=3276.7, y=w226) -> (x*y=w225:cluster{"Set 1":dbl, "Set 2":dbl})
  n49 = To Word Integer(number=w183) -> (16bit integer=w181:i16)
  n50 = Multiply(x=w203, y=u64 2) -> (x*y=w201:u64)
  n51 = local read "Sets to FIFO (Traps)"() -> (w233:T15)
  n52 = Divide(x=w168, y="FPGA Ave.") -> (x/y=w169:dbl)
  n53 = To Word Integer(number=w225) -> (16bit integer=w224:cluster{"Set 1":i16, "Set 2":i16})
  n54 = xnode "Open FPGA VI Reference"("resource name"=T18 "750kHzDAQ") -> ("FPGA VI Reference Out"=w218:T19)  [unwired: 1 in, 1 out]
  n55 = Unbundle By Name(w221) -> ("Set 1"=w220:T14, "Set 2"=w219:T14)
  n56 = Multiply(x=w201, y=w200) -> (x*y=w198:u64)
  n57 = local write "Ave. Rate (Hz)"(w169) -> ()
  n58 = Divide(x=w198, y=w199) -> (x/y=w197:dbl)
  n59 = Unbundle By Name(w224) -> ("Set 1"=w223:i16, "Set 2"=w222:i16)
  n60 = local read "2D or 1D Scan"() -> (w122:bool)
  n61 = local write "Data points/scans"(w198) -> ()
  n62 = local read "Scan BD"() -> (w216:bool)
  n63 = And(x=w229, y=w230) -> (x .and. y?=w228:cluster{"Set 1":bool, "Set 2":bool})
  n64 = local write "Data points/scan (f/b)"(w201) -> ()
  n65 = Reciprocal(x=w169) -> (1/x=w170:dbl)
  n66 = local read "N Acq Sets (Traps + Fl.)"() -> (w161:i16)
  n67 = local write "N sets should be saved"(w197) -> ()
  n68 = Unbundle By Name(w228) -> ("Set 1"=w232:bool, "Set 2"=w231:bool)
  n69 = local read "Interlace"() -> (w104:bool)
  n70 = Select(t=w111, s=w104, f=w109) -> (s? t:f=w101:u32)
  n71 = local write "Update Count (MCL)"(w101) -> ()
  n72 = local write "Total Counts (ticks)"(w101) -> ()
  n73 = xnode "Invoke Method"("FPGA VI Reference In"=w218) -> ("FPGA VI Reference Out"=w120:T19, "error out"=w139:errorcluster)  [unwired: 1 in]
  n74 = local write "Ave. Period (s)"(w170) -> ()
  n75 = property on="2D or 1D Scan" class="Bool (strict)"("Val(Sgnl)"=w122) -> ()  [unwired: 2 in, 2 out]
  n76 = xnode "Read/Write Control"("FPGA VI Reference In"=w119, "error in"=w139, "ai count"="AI Count (ticks)", "Interlace ON/OFF"=w104, "Number Interlace Cycles"=w103, "AI1 Sets to FIFO"=w233, "FB On/Off Set 1"=w232, "FB On/Off Set 2"=w231, "Interlace Off Parameters"=w102, "FB Setpoint Set 1"=w223, "FB Setpoint Set 2"=w222, "FB Gains Set 1"=w220, "FB Gains Set 2"=w219, "FB output range 1"=w121, "FB output range 2"=w121, "Cycles per step"=w204, "Scan BD"=w216, "Number of scans"=w200, "Scan steps"=w205, "Scan freq.  increment"=w206, "AO1"=w188, "AO2"=w187, "Scan freq.  increment (MCL)"=w181, "Scan steps (MCL)"=w180, "Cycles per step (MCL)"=w179, "Number of scans (MCL)"=w178, "MCL count"=w101, "Cont. Scan (MCL)"=w177, "MCL Scan Axis"=w171, "1D or 2D Scan?"=w122, "N of AI1 Int Acq Sets"=w161, "Freq or Amp switch first"="Freq or Amp switch first", "Freq switch delay"="Freq switch delay", "Amp switch delay"="Amp switch delay", "Swap F1 and F2"="Swap F1 and F2", "APD Acq Rate Count"=w127, "APD to FIFO"=FALSE, "APD Gate Operating Mode"="APD Gate", "APD Gate ON Count"="APD Gate ON Count", "APD Gate OFF Count"="APD Gate OFF Count", "Invert APD Gate"="Invert APD Gate", "DIO count 1 (ticks)"="DIO count 1 (ticks)", "DIO count 2 (ticks)"="DIO count 2 (ticks)", "DIO count 3 (ticks)"="DIO count 3 (ticks)", "APD 1 AO scale factor"="APD 1 AO Mult.", "APD 2 AO scale factor"="APD 2 AO Mult.") -> ("FPGA VI Reference Out"=w96:T19, "error out"=w98:errorcluster)  [unwired: 1 in]
  n77 = local read "Green Laser ON/Interlacing"() -> (w99:bool)
  n78 = local read "Green laser mode"() -> (w100:enum32{"Laser ON", "Laser OFF", "Interlace"})
  n79 = local read "GI Frequency, OFF count"() -> (w92:u32)
  n80 = local read "GI Frequency, ON count"() -> (w91:u32)
  n81 = Multiply(x="Current When FB OFF (%)", y=655.35) -> (x*y=w82:dbl)
  n82 = local read "Green FB Count"() -> (w90:u32)
  n83 = Multiply(x="Green FB Setpoint (mV)", y=3.2767) -> (x*y=w79:dbl)
  n84 = To Unsigned Word Integer(number=w82) -> (unsigned 16bit integer=w80:u16)
  n85 = local read "Invert GI"() -> (w94:bool)
  n86 = To Word Integer(number=w79) -> (16bit integer=w77:i16)
  n87 = case shown="True" w99 {
    tunnel: w100 -> [_ w253]
    tunnel: [enum32{"Laser ON", "Laser OFF", "Interlace"}."Laser OFF" ("Green laser mode") w253] -> w93
    frame False {
    }
    frame True {
    }
  }
  n88 = local read "Trap Pos. AI1 X Pre-scale"() -> (w48:u16)
  n89 = local read "Trap Pos FB Monitor\nT1 or T2"() -> (w55:bool)
  n90 = local read "Trap Pos FB Int Count"() -> (w43:u16)
  n91 = local read "Trap Pos FB Negate Action"() -> (w54:bool)
  n92 = local read "Trap Pos. FB Offset Factor"() -> (w53:i64)
  n93 = local read "Trap Pos. FB Mult Factor"() -> (w52:i64)
  n94 = local read "Trap Pos. FB Gains"() -> (w50:T11)
  n95 = local read "Trap Pos. FB Range"() -> (w51:T12)
  n96 = xnode "Read/Write Control"("FPGA VI Reference In"=w96, "error in"=w98, "Green interlace ON count 2"=w91, "Green interlace OFF count 2"=w92, "Invert GI 2"=w94, "Operating Mode 2"=w93, "Green FB Gains"="Green FB Gains", "Green FB Setpoint"=w77, "Green FB On/Off"="Green FB On/Off", "Current Out"=w80, "Green int current ON count adj"="Green int current ON count adj", "Green FB Count"=w90, "Operating Mode"=w93, "Green interlace OFF count"=w92, "Green interlace ON count"=w91, "Invert GI"=w94, "Trap Pos FB Monitor T1 or T2"=w55, "Trap Pos FB Negate Action"=w54, "Trap Pos. FB Offset Factor"=w53, "Trap Pos. FB Mult Factor"=w52, "Trap Pos. FB Range"=w51, "Trap Pos. FB Gains"=w50, "Force feedback"=FALSE, "AI1 X Scale"=w48, "Trap Pos to FIFO"=TRUE, "Trap Pos FB Int Count"=w43) -> ("FPGA VI Reference Out"=w95:T19, "error out"=w97:errorcluster)
  n97 = xnode "Invoke Method"("FPGA VI Reference In"=w95, "error in"=w97, "Requested Depth"="Trap AI FIFO Depth") -> ("FPGA VI Reference Out"=w58:T19, "error out"=w57:errorcluster)  [unwired: 1 out]
  n98 = xnode "Invoke Method"("FPGA VI Reference In"=w58, "error in"=w57, "Requested Depth"="Trap Position FIFO Depth") -> ("FPGA VI Reference Out"=w45:T19, "error out"=w44:errorcluster)  [unwired: 1 out]
  n99 = flat-sequence {
    tunnel: w120 -> [w258]
    tunnel: [w258] -> w119
    tunnel: [w257] -> w118
    tunnel: [w256] -> w117
    tunnel: [w254] -> w115
    tunnel: [w255] -> w116
    frame #0 {
      w255 = T16 {"Minimum"=50.0, "Maximum"=100.0, "Increment"=1.0} ("Min Max Inc")
      w254 = T16 {"Minimum"=0.0, "Maximum"=75.0, "Increment"=1.0} ("Data Entry Limits")
      w257 = T16 {"Minimum"=50.0, "Maximum"=100.0, "Increment"=1.0} ("Min Max Inc")
      w256 = T16 {"Minimum"=0.0, "Maximum"=75.0, "Increment"=1.0} ("Data Entry Limits")
      n100 = property on="BD 2 Frequency 1 (MHz)" class="DigNum (strict)"("Data Range"=w255) -> ()  [unwired: 2 in, 2 out]
      n101 = property on="BD 2 Frequency 3 (MHz)" class="DigNum (strict)"("Data Range"=w255) -> ()  [unwired: 2 in, 2 out]
      n102 = property on="BD 2 Frequency 2 (MHz)" class="DigNum (strict)"("Data Range"=w255) -> ()  [unwired: 2 in, 2 out]
      n103 = property on="BD 1 Frequency 1 (MHz)" class="DigNum (strict)"("Data Range"=w257) -> ()  [unwired: 2 in, 2 out]
      n104 = property on="BD 1 Frequency 2 (MHz)" class="DigNum (strict)"("Data Range"=w257) -> ()  [unwired: 2 in, 2 out]
      n105 = property on="BD 1 Frequency 3 (MHz)" class="DigNum (strict)"("Data Range"=w257) -> ()  [unwired: 2 in, 2 out]
      n106 = property on="BD 2 Amplitude 1 (%)" class="DigNum (strict)"("Data Range"=w254) -> ()  [unwired: 2 in, 2 out]
      n107 = property on="BD 2 Amplitude 2 (%)" class="DigNum (strict)"("Data Range"=w254) -> ()  [unwired: 2 in, 2 out]
      n108 = property on="BD 2 Amplitude 3 (%)" class="DigNum (strict)"("Data Range"=w254) -> ()  [unwired: 2 in, 2 out]
      n109 = property on="BD 1 Amplitude 3 (%)" class="DigNum (strict)"("Data Range"=w256) -> ()  [unwired: 2 in, 2 out]
      n110 = property on="BD 1 Amplitude 2 (%)" class="DigNum (strict)"("Data Range"=w256) -> ()  [unwired: 2 in, 2 out]
      n111 = property on="BD 1 Amplitude 1 (%)" class="DigNum (strict)"("Data Range"=w256) -> ()  [unwired: 2 in, 2 out]
      "X RF Frequency Limits (MHz)" <- w257
      "X RF Amplitude Limits (%)" <- w256
      "Y RF Amplitude Limits (%)" <- w254
      "Y RF Frequency Limits (MHz)" <- w255
    }
  }
  n112 = xnode "Invoke Method"("FPGA VI Reference In"=w45, "error in"=w44) -> ("FPGA VI Reference Out"=w22:T19, "error out"=w21:errorcluster)  [unwired: 1 in]
  n113 = flat-sequence "Initial FPGA Loop Relative Phase Adjustment" {
    tunnel: "Initial Phase Adjustment (APD 2 Gate)" -> [w260]
    tunnel: "Initial Phase Adjustment (GI) 2" -> [w261]
    tunnel: "Initial Phase Adj. (MCL)" -> [w262]
    tunnel: w21 -> [w263]
    tunnel: w22 -> [w264]
    tunnel: "Initial Phase Adjustment (GI)" -> [w265]
    tunnel: "Initial Phase Adjustment (AI1)" -> [w266]
    tunnel: [w266] -> w31
    tunnel: [w265] -> w30
    tunnel: [w264] -> w29
    tunnel: [w263] -> w28
    tunnel: [w262] -> w27
    tunnel: [w261] -> w26
    tunnel: [w260] -> w25
    tunnel: [w278] -> w145
    tunnel: [w272] -> w143
    tunnel: "Initial Phase Adjustment (APD Acq)" -> [w271]
    tunnel: "Initial Phase Adjustment (APD 1 Gate)" -> [w270]
    tunnel: "Initial Phase Adjustment (Green FB)" -> [w269]
    tunnel: w31 -> [w277]
    tunnel: w30 -> [w276]
    tunnel: w29 -> [w275]
    tunnel: w28 -> [w274]
    tunnel: w27 -> [w273]
    tunnel: w26 -> [w268]
    tunnel: w25 -> [w267]
    tunnel: w145 -> [w280]
    tunnel: [w281] -> w144
    tunnel: w143 -> [w281]
    tunnel: [w280] -> w142
    tunnel: w144 -> [w284]
    tunnel: w142 -> [w283]
    tunnel: [w286] -> w141
    tunnel: [w285] -> w140
    tunnel: [w288] -> w20
    tunnel: [w289] -> w23
    tunnel: w141 -> [w289]
    tunnel: w140 -> [w288]
    frame #0 {
      n114 = Wait (ms)(milliseconds to wait=u32 1000) -> ()  [unwired: 1 out]
    }
    frame #1 {
      n115 = xnode "Read/Write Control"("FPGA VI Reference In"=w275, "error in"=w274, "Phase count adjustment"=w277, "Phase count adjustment (GI)"=w276, "Phase count adjustment (MCL)"=w273, "Phase Count Adjustment (APD Acq)"=w271, "Phase count adjustment (APD 1 Gate)"=w270, "Phase count adjustment (APD 2 Gate)"=w267, "Phase count adjustment (Green FB)"=w269, "Phase count adjustment (GI) 2"=w268) -> ("FPGA VI Reference Out"=w272:T19, "error out"=w278:errorcluster)
    }
    frame #2 {
      n116 = Wait (ms)(milliseconds to wait=u32 1000) -> ()  [unwired: 1 out]
    }
    frame #3 {
      w282 = TRUE
      n117 = xnode "Read/Write Control"("FPGA VI Reference In"=w284, "error in"=w283, "+ phase"=w282, "+ phase (GI)"=w282, "+ phase (MCL)"=w282, "+ phase (APD Acq)"=w282, "+ phase (APD 1 Gate)"=w282, "+ phase (APD 2 Gate)"=w282, "+ phase (Green FB)"=w282, "+ phase (GI) 2"=w282) -> ("FPGA VI Reference Out"=w285:T19, "error out"=w286:errorcluster)
    }
    frame #4 {
      n118 = Wait (ms)(milliseconds to wait=u32 1000) -> ()  [unwired: 1 out]
    }
  }
  n119 = local read "Phase adj. (Green FB)"() -> (w113:i16)
  n120 = local read "Phase adj. (GI) 2"() -> (w83:i16)
  n121 = local read "Phase adjust (MCL)"() -> (w172:i16)
  n122 = local read "Phase adj. (AI1)"() -> (w174:i16)
  n123 = local read "Phase adj. (GI)"() -> (w173:i16)
  n124 = xnode "Read/Write Control"("FPGA VI Reference In"=w20, "error in"=w23, "Phase count adjustment"=w174, "Phase count adjustment (GI)"=w173, "Phase count adjustment (MCL)"=w172, "Phase Count Adjustment (APD Acq)"="Phase Adj. (APD Acq)", "Phase count adjustment (APD 1 Gate)"="Phase Adj. (APD 1 Gate)", "Phase count adjustment (APD 2 Gate)"="Phase Adj. (APD 2 Gate)", "Phase count adjustment (Green FB)"=w113, "Phase count adjustment (GI) 2"=w83) -> ("FPGA VI Reference Out"=w19:T19, "error out"=w18:errorcluster)
  n125 = call "Initialize RF boards - interlace 3.vi"("error in"=w18, "FPGA VI Reference In"=w19) -> ("FPGA VI Reference Out"=w150:T19)  [unwired: 1 out]
  n126 = call "set RF board frequency - interlace.vi"("Board 2 Frequency Limits"=w116, "Board 1 Frequency Limits"=w118, "FPGA VI Reference In"=w150, "Board 2 Frequency 3 (MHz)"="BD 2 Frequency 3 (MHz)", "Board 1 Frequency 3 (MHz)"="BD 1 Frequency 3 (MHz)", "Board 2 Frequency 2 (MHz)"="BD 2 Frequency 2 (MHz)", "Board 2 Frequency 1 (MHz)"="BD 2 Frequency 1 (MHz)", "Board 1 Frequency 2 (MHz)"="BD 1 Frequency 2 (MHz)", "Board 1 Frequency 1  (MHz)"="BD 1 Frequency 1 (MHz)") -> ("error out"=w244:errorcluster, "FPGA VI Reference Out"=w245:T19)  [unwired: 1 in]
  n127 = call "set RF board amplitude - interlace.vi"("Board 2 Amplitude Limits"=w115, "Board 1 Amplitude Limits"=w117, "error in"=w244, "FPGA VI Reference In"=w245, "Board 2 Amplitude 3 (%)"="BD 2 Amplitude 3 (%)", "Board 1 Amplitude 3 (%)"="BD 1 Amplitude 3 (%)", "Board 2 Amplitude 2 (%)"="BD 2 Amplitude 2 (%)", "Board 2 Amplitude 1 (%)"="BD 2 Amplitude 1 (%)", "Board 1 Amplitude 2 (%)"="BD 1 Amplitude 2 (%)", "Board 1 Amplitude 1 (%)"="BD 1 Amplitude 1 (%)") -> ("error out"=w16:errorcluster, "FPGA VI Reference Out"=w17:T19)
  n128 = flat-sequence {
    tunnel: w17 -> [w298]
    tunnel: w16 -> [w297]
    tunnel: [w296] -> w237
    tunnel: [w295] -> w236
    tunnel: [w302] -> w235
    tunnel: w237 -> [w302]
    tunnel: [w301] -> w234
    tunnel: w236 -> [w301]
    tunnel: w235 -> [w311]
    tunnel: w234 -> [w310]
    tunnel: [w309] -> w12
    tunnel: [w304] -> w11
    tunnel: [w314] -> w40
    tunnel: [w318] -> w24
    tunnel: w12 -> [w318]
    tunnel: w11 -> [w313]
    frame #0 {
      n129 = local read "Trap 1 (ON/OFF)"() -> (w290:bool)
      n130 = xnode "Read/Write Control"("FPGA VI Reference In"=w298, "error in"=w297, "Direct RF Box  Communication"=FALSE) -> ("FPGA VI Reference Out"=w296:T19, "error out"=w295:errorcluster)
      n131 = local write "Saving..."(FALSE ("Saving Data")) -> ()
      n132 = local write "Stop All"(FALSE ("Stop All")) -> ()
      n133 = local write "Index"(1.0 ("Index")) -> ()
      n134 = property on="Trap 1 ON" class="Bool (strict)"("Value"=w290) -> ()  [unwired: 2 in, 2 out]
      "Manipulating Trap" <- FALSE ("Manipulating Trap")
    }
    frame #1 {
      n135 = local read "Trap 2 (ON/OFF)"() -> (w300:bool)
      n136 = Wait (ms)(milliseconds to wait=u32 50) -> ()  [unwired: 1 out]
      n137 = property on="Trap 2 ON" class="Bool (strict)"("Val(Sgnl)"=w300) -> ()  [unwired: 2 in, 2 out]
    }
    frame #2 {
      n138 = local read "Scan Range (nm)"() -> (w305:dbl)
      n139 = xnode "Read/Write Control"("FPGA VI Reference In"=w311, "error in"=w310, "FPGA Controls  RF Box"=TRUE ("Direct RF Box  Communication")) -> ("FPGA VI Reference Out"=w309:T19, "error out"=w304:errorcluster)
      n140 = call "Update messages.vi"("Message to add"="UHR-Fleezers ready.", "Old message string"="") -> ("New message string"=w308:string)
      n141 = local write "Messages"(w308) -> ()
      n142 = property on="Scan Range (nm)" class="DigNum (strict)"("Val(Sgnl)"=w305) -> ()  [unwired: 2 in, 2 out]
    }
    frame #3 {
      n143 = call "hamilton_controller.vi"("error in"=w313, "action"=T20."CONNECT") -> ("error out"=w315:errorcluster)  [unwired: 9 in]
      n144 = call "hamilton_controller.vi"("error in"=w315, "action"=T20."INITIALIZE VALVES") -> ("error out"=w314:errorcluster)  [unwired: 9 in]
    }
  }
  n145 = Subtract(x="BD 1 Frequency 1 (MHz)", y="BD 1 Frequency 2 (MHz)") -> (x-y=w160:dbl)
  n146 = Subtract(x="BD 2 Frequency 1 (MHz)", y="BD 2 Frequency 2 (MHz)") -> (x-y=w159:dbl)
  n147 = Square(x=w159) -> (x^2=w157:dbl)
  n148 = Square(x=w160) -> (x^2=w158:dbl)
  n149 = Add(x=w158, y=w157) -> (x+y=w156:dbl)
  n150 = Square Root(x=w156) -> (sqrt(x)=w155:dbl)
  n151 = local write "Trap Delta (MHz)"(w155) -> ()
  n152 = Current VI's Path() -> (path=w1:path)
  n153 = Strip Path(path=w1) -> (stripped path=w2:path)  [unwired: 1 out]
  n154 = Build Path(base path=w2, name or relative path="Locations.txt") -> (appended path=→"Location path":path)
  n155 = Concatenate Strings("N.D.", "\r\n") -> (w5:string)
  n156 = Initialize Array(w5, 4, 3) -> (w8:string[][])
  n157 = local write "Location Matrix"(w8) -> ()
  n158 = call "IMAQ Create"("Image Name"="APD 1 Image", "Image Type"=w64) -> ("New Image"=w63:T2)  [unwired: 3 in, 1 out]
  n159 = call "IMAQ Create"("Image Name"="APD 2 Image", "Image Type"=w64) -> ("New Image"=w62:T2)  [unwired: 3 in, 1 out]
  n160 = call "IMAQ Create"("Image Name"="Det. X Image", "Image Type"=w64) -> ("New Image"=w61:T2)  [unwired: 3 in, 1 out]
  n161 = call "IMAQ Create"("Image Name"="Det. Y Image", "Image Type"=w64) -> ("New Image"=w60:T2)  [unwired: 3 in, 1 out]
  n162 = Bundle("New Image"=w63, "New Image"=w62, "New Image"=w61, "New Image"=w60) -> (w59:T21)  [unwired: 1 in]
  n163 = while {
    stop <- w319 stop-if-true
    n164 = event shown="[0] Timeout" {
      selector: _ -> [_ _ _ _ _ _ _]
      dyn-events: _ -> [_ _ _ _ _ _ _]
      timeout: 10 -> [_ _ _ _ _ _ _]
      tunnel: [FALSE _ _ _ _ _ _] -> w319
      event Timeout {
        # "Query and display stage positions"
        # "Setting ESP300 left and right limits for Z-axis, input in mm"
        # "Display Selected Location"
        n165 = event-data() -> ()  [unwired: 1 in, 2 out]
        n166 = local read "ESP Port"() -> (w336:refnum<visa-resource-name>)
        n167 = Concatenate Strings("3SL" ("Substring"), "ESP ZL-Limit", ";3SR", "ESP ZR-Limit", "\r") -> (w335:string)
        n168 = VISA Write(VISA resource name=w336, write buffer=w335) -> ()  [unwired: 1 in, 3 out]
        n169 = disable-structure shown="Enabled" {
          frame Disabled {
            # "Change Low Jog Velocity"
            # "Change High Jog Velocity"
            n170 = Concatenate Strings("1JH" ("Substring"), "Axis 1", "2JH" ("Substring"), "Axis 2", "3JH" ("Substring"), "Axis 3", "\r") -> (w359:string)
            n171 = local read "ESP Port"() -> (w358:refnum<visa-resource-name>)
            n172 = VISA Write(VISA resource name=w358, write buffer=w359) -> ()  [unwired: 1 in, 3 out]
            n173 = Concatenate Strings("1JW" ("Substring"), "Axis 1", "2JW" ("Substring"), "Axis 2", "3JW" ("Substring"), "Axis 3", "\r") -> (w350:string)
            n174 = local read "ESP Port"() -> (w349:refnum<visa-resource-name>)
            n175 = VISA Write(VISA resource name=w349, write buffer=w350) -> ()  [unwired: 1 in, 3 out]
          }
          frame Enabled {
          }
        }
        n176 = local read "Location Matrix"() -> (w341:string[][])
        n177 = local read "Locations"() -> (w340:i32)
        n178 = Index Array(array=w341, index (row)=w340) -> (element=w339:string[])  [unwired: 1 in]
        n179 = Array To Cluster(array=w339) -> (cluster=w338:T22)
        n180 = local write "Selected Location"(w338) -> ()
        n181 = Concatenate Strings("1TP;\n2TP;\n3TP;\n1MD?;\n2MD?;\n3MD?" ("Substring"), "\r") -> (w324:string)
        n182 = local read "ESP Port"() -> (w327:refnum<visa-resource-name>)
        n183 = VISA Write(VISA resource name=w327, write buffer=w324, error in (no error)="error in") -> (VISA resource name out=w325:refnum<visa-resource-name>, error out=w323:errorcluster)  [unwired: 1 out]
        n184 = case shown="True" TRUE ("Case Constant\n(See Context Help)") {
          tunnel: w325 -> [_ w379]
          tunnel: w323 -> [w360 w378]
          tunnel: [w360 w362] -> w329
          frame False {
          }
          frame True {
            w372 = u16 10 items=["1.0"=10, "1.5"=15, "2.0"=20] ("Serial Settings:Stop Bits")
            w373 = u16 0 items=["None", "Odd", "Even", "Mark", "Space"] ("Serial Settings:Parity")
            n185 = property class="Instr"(reference=w379, error in=w378, "Baud"=u32 921600 ("Serial Settings:Baud Rate"), "Data Bits"=u16 8 ("Serial Settings:Data Bits"), "Parity"=w373, "Stop Bits"=w372) -> (reference out=w377:refnum<visa-resource-name>, error out=w376:errorcluster, "Bytes at Port"=w361:u32)
            n186 = Wait (ms)(milliseconds to wait=u32 10) -> ()  [unwired: 1 out]
            n187 = VISA Read(VISA resource name=w377, byte count=w361, error in (no error)=w376) -> (VISA resource name out=w385:refnum<visa-resource-name>, read buffer=→"X Pos":string, error out=w386:errorcluster)  [unwired: 1 out]
            n188 = VISA Read(VISA resource name=w385, byte count=w361, error in (no error)=w386) -> (VISA resource name out=w383:refnum<visa-resource-name>, read buffer=→"Y Pos":string, error out=w384:errorcluster)  [unwired: 1 out]
            n189 = VISA Read(VISA resource name=w383, byte count=w361, error in (no error)=w384) -> (VISA resource name out=w371:refnum<visa-resource-name>, read buffer=→"Z Pos Pos":string, error out=w370:errorcluster)  [unwired: 1 out]
            n190 = VISA Read(VISA resource name=w371, byte count=w361, error in (no error)=w370) -> (VISA resource name out=w367:refnum<visa-resource-name>, read buffer=→"X Motion":string, error out=w368:errorcluster)  [unwired: 1 out]
            n191 = VISA Read(VISA resource name=w367, byte count=w361, error in (no error)=w368) -> (VISA resource name out=w366:refnum<visa-resource-name>, read buffer=→"Y Motion":string, error out=w364:errorcluster)  [unwired: 1 out]
            n192 = VISA Read(VISA resource name=w366, byte count=w361, error in (no error)=w364) -> (read buffer=→"Z motion":string, error out=w362:errorcluster)  [unwired: 2 out]
          }
        }
        "error out" <- w329
      }
      event "Goto Top (F6)": Value Change {
        n193 = event-data() -> ()  [unwired: 1 in, 5 out]
        n194 = stacked-sequence {
          frame #0 {
            # "stop motions of all axes before going to avoid reversing of direction"
            n195 = local read "ESP Port"() -> (w391:refnum<visa-resource-name>)
            n196 = Concatenate Strings("ST" ("Substring"), "\r") -> (w388:string)
            n197 = VISA Write(VISA resource name=w391, write buffer=w388) -> ()  [unwired: 1 in, 3 out]
          }
          frame #1 {
            n198 = Wait (ms)(milliseconds to wait=u32 50) -> ()  [unwired: 1 out]
          }
          frame #2 {
            # "Change the trajectory mode to Trapezoidal"
            n199 = local read "ESP Port"() -> (w396:refnum<visa-resource-name>)
            n200 = Concatenate Strings("1TJ1;\n2TJ1;\n3TJ1" ("Substring"), "\r") -> (w393:string)
            n201 = VISA Write(VISA resource name=w396, write buffer=w393) -> ()  [unwired: 1 in, 3 out]
          }
          frame #3 {
            # "Go to Top Dispensor"
            n202 = local read "Location Matrix"() -> (w408:string[][])
            n203 = Index Array(array=w408, index (row)=0) -> (element=w404:string[])  [unwired: 1 in]
            n204 = Decimate 1D Array(w404) -> (w402:string[], w400:string[], w398:string[])
            n205 = Concatenate Strings("1PA" ("Substring"), w402, "2PA" ("Substring"), w400, "3PA" ("Substring"), w398, "\r") -> (w406:string)
            n206 = local read "ESP Port"() -> (w405:refnum<visa-resource-name>)
            n207 = VISA Write(VISA resource name=w405, write buffer=w406) -> ()  [unwired: 1 in, 3 out]
          }
          frame #4 {
            n208 = Wait (ms)(milliseconds to wait=u32 2000) -> ()  [unwired: 1 out]
          }
        }
      }
      event "Goto Exp (F8)": Value Change {
        n209 = event-data() -> ()  [unwired: 1 in, 5 out]
        n210 = stacked-sequence {
          frame #0 {
            # "stop motions of all axes before going to avoid reversing of direction"
            n211 = local read "ESP Port"() -> (w413:refnum<visa-resource-name>)
            n212 = Concatenate Strings("ST" ("Substring"), "\r") -> (w410:string)
            n213 = VISA Write(VISA resource name=w413, write buffer=w410) -> ()  [unwired: 1 in, 3 out]
          }
          frame #1 {
            n214 = Wait (ms)(milliseconds to wait=u32 50) -> ()  [unwired: 1 out]
          }
          frame #2 {
            # "Change the trajectory mode to Trapezoidal"
            n215 = local read "ESP Port"() -> (w418:refnum<visa-resource-name>)
            n216 = Concatenate Strings("1TJ1;\n2TJ1;\n3TJ1" ("Substring"), "\r") -> (w415:string)
            n217 = VISA Write(VISA resource name=w418, write buffer=w415) -> ()  [unwired: 1 in, 3 out]
          }
          frame #3 {
            # "Go to Experimental"
            n218 = local read "Location Matrix"() -> (w430:string[][])
            n219 = Index Array(array=w430, index (row)=2) -> (element=w426:string[])  [unwired: 1 in]
            n220 = Decimate 1D Array(w426) -> (w424:string[], w422:string[], w420:string[])
            n221 = Concatenate Strings("1PA" ("Substring"), w424, "2PA" ("Substring"), w422, "3PA" ("Substring"), w420, "\r") -> (w428:string)
            n222 = local read "ESP Port"() -> (w427:refnum<visa-resource-name>)
            n223 = VISA Write(VISA resource name=w427, write buffer=w428) -> ()  [unwired: 1 in, 3 out]
          }
          frame #4 {
            n224 = Wait (ms)(milliseconds to wait=u32 100) -> ()  [unwired: 1 out]
          }
        }
      }
      event "Goto Bottom (F7)": Value Change {
        n225 = event-data() -> ()  [unwired: 1 in, 5 out]
        n226 = stacked-sequence {
          frame #0 {
            # "stop motions of all axes before going to avoid reversing of direction"
            n227 = local read "ESP Port"() -> (w435:refnum<visa-resource-name>)
            n228 = Concatenate Strings("ST" ("Substring"), "\r") -> (w432:string)
            n229 = VISA Write(VISA resource name=w435, write buffer=w432) -> ()  [unwired: 1 in, 3 out]
          }
          frame #1 {
            n230 = Wait (ms)(milliseconds to wait=u32 50) -> ()  [unwired: 1 out]
          }
          frame #2 {
            # "Change the trajectory mode to Trapezoidal"
            n231 = local read "ESP Port"() -> (w440:refnum<visa-resource-name>)
            n232 = Concatenate Strings("1TJ1;\n2TJ1;\n3TJ1" ("Substring"), "\r") -> (w437:string)
            n233 = VISA Write(VISA resource name=w440, write buffer=w437) -> ()  [unwired: 1 in, 3 out]
          }
          frame #3 {
            # "Go to Bottom Dispensor"
            n234 = local read "Location Matrix"() -> (w452:string[][])
            n235 = Index Array(array=w452, index (row)=1) -> (element=w448:string[])  [unwired: 1 in]
            n236 = Decimate 1D Array(w448) -> (w446:string[], w444:string[], w442:string[])
            n237 = Concatenate Strings("1PA" ("Substring"), w446, "2PA" ("Substring"), w444, "3PA" ("Substring"), w442, "\r") -> (w450:string)
            n238 = local read "ESP Port"() -> (w449:refnum<visa-resource-name>)
            n239 = VISA Write(VISA resource name=w449, write buffer=w450) -> ()  [unwired: 1 in, 3 out]
          }
          frame #4 {
            n240 = Wait (ms)(milliseconds to wait=u32 100) -> ()  [unwired: 1 out]
          }
        }
      }
      event "Capture": Value Change {
        n241 = event-data() -> ()  [unwired: 1 in, 5 out]
        n242 = local read "Locations"() -> (w454:i32)
        n243 = local read "Z Pos Pos"() -> (w455:string)
        n244 = local read "X Pos"() -> (w457:string)
        n245 = local read "Y Pos"() -> (w456:string)
        n246 = case shown="1" w454 {
          selector: w454 -> [w461 w468 w475 w482]
          tunnel: w457 -> [w464 w471 w478 w485]
          tunnel: w456 -> [w463 w470 w477 w484]
          tunnel: w455 -> [w462 w469 w476 w483]
          frame 0, Default {
            # "Capture Top Dispensor Location"
            n247 = local read "Location Matrix"() -> (w460:string[][])
            n248 = Build Array(w464, w463, w462) -> (w459:string[])
            n249 = Replace Array Subset(array=w460, new element=w459, index (row)=w461) -> (w458:string[][])  [unwired: 1 in]
            n250 = local write "Location Matrix"(w458) -> ()
          }
          frame 1 {
            # "Capture Bottom Dispensor Location"
            n251 = local read "Location Matrix"() -> (w467:string[][])
            n252 = Build Array(w471, w470, w469) -> (w466:string[])
            n253 = Replace Array Subset(array=w467, new element=w466, index (row)=w468) -> (w465:string[][])  [unwired: 1 in]
            n254 = local write "Location Matrix"(w465) -> ()
          }
          frame 2 {
            # "Capture Experimental Region Location"
            n255 = local read "Location Matrix"() -> (w474:string[][])
            n256 = Build Array(w478, w477, w476) -> (w473:string[])
            n257 = Replace Array Subset(array=w474, new element=w473, index (row)=w475) -> (w472:string[][])  [unwired: 1 in]
            n258 = local write "Location Matrix"(w472) -> ()
          }
          frame 3 {
            # "Capture Other Location"
            n259 = local read "Location Matrix"() -> (w481:string[][])
            n260 = Build Array(w485, w484, w483) -> (w480:string[])
            n261 = Replace Array Subset(array=w481, new element=w480, index (row)=w482) -> (w479:string[][])  [unwired: 1 in]
            n262 = local write "Location Matrix"(w479) -> ()
          }
        }
      }
      event "Save": Value Change {
        # "reshape Location Matrix to 1-D array to write"
        n263 = event-data() -> ()  [unwired: 1 in, 5 out]
        n264 = local read "Location Matrix"() -> (w489:string[][])
        n265 = local read "Location path"() -> (w486:path)
        n266 = Reshape Array(w489, 12) -> (w487:string[])
        n267 = Write to Text File(file (use dialog)=w486, text=w487) -> ()  [unwired: 2 in, 3 out]
      }
      event "Activate Joystick": Value Change {
        n268 = event-data() -> ()  [unwired: 1 in, 5 out]
        n269 = case shown="True" "Activate Joystick" {
          frame False {
          }
          frame True {
            # "Change the trajectory mode to Jog"
            n270 = local read "ESP Port"() -> (w494:refnum<visa-resource-name>)
            n271 = Concatenate Strings("1TJ3;\n2TJ3;\n3TJ3" ("Substring"), "\r") -> (w491:string)
            n272 = VISA Write(VISA resource name=w494, write buffer=w491) -> ()  [unwired: 1 in, 3 out]
          }
        }
      }
    }
  }
  n273 = disable-structure shown="Disabled" {
    disable-tunnel: w24 -> [w523 _]
    frame Disabled {
      w518 = T17 0 items=["Grayscale (U8)", "Grayscale (I16)", "Grayscale (SGL)", "Complex (CSG)", "RGB (U32)", "HSL (U32)", "RGB (U64)", "Grayscale (U16)"] ("Image Type")
      n274 = call <vilib>:"IMAQ Init.vi"("Interface Name"="img0") -> ("error out"=w520:errorcluster, "IMAQ Session Out"=w522:refnum<k11>)  [unwired: 9 in]
      n275 = call <vilib>:"IMAQ Grab Setup.vi"("error in (no error)"=w520, "IMAQ Session In"=w522) -> ("error out"=w516:errorcluster, "IMAQ Session Out"=w517:refnum<k11>)  [unwired: 8 in]
      n276 = call "IMAQ Create"("Image Name"="untitled", "Image Type"=w518) -> ("New Image"=w515:T2)  [unwired: 3 in, 1 out]
      n277 = call <vilib>:"Application Directory.vi"() -> ("Application Directory"=w502:path)
      n278 = Build Path(base path=w502, name or relative path="_trap_screen_positions") -> (appended path=w510:path)
      n279 = Open/Create/Replace File(file path (use dialog)=w510, operation (0:open)=T23."open or create", access (0:read/write)=enum16{"read/write", "read-only", "write-only"}."read/write") -> (refnum out=w512:refnum<file>)  [unwired: 3 in, 2 out]
      n280 = local read "Trap Sets"() -> (w504:u32)
      n281 = for "Load trap positions on video screen from file." {
        N: w504 -> [_]
        tunnel: [w530] -> w505
        tunnel: w512 -> [w529]
        tunnel: [w526] -> w501 mode=indexing
        w528 = 4
        n282 = for {
          N: w528 -> [_]
          tunnel: [w534] -> w530
          tunnel: w529 -> [w533]
          tunnel: w528 -> [w532]
          tunnel: [w531] -> w527 mode=indexing
          n283 = Read from Binary File(5:w532, 11:w533) -> (2:w531:i32, 3:w534:refnum<file>)  [unwired: 4 in, 2 out]
        }
        n284 = Array To Cluster(array=w527) -> (cluster=w526:T27)
      }
      n285 = node-c288() -> (w525:T24)  [unwired: 4 in]
      n286 = timed-loop "acquire video and stage position" {
        timing: w525 -> [_]
        timing-out: [_] -> w524
        tunnel: w517 -> [w553]
        tunnel: w516 -> [w552]
        tunnel: w515 -> [w551]
        tunnel: [w550] -> w497
        tunnel: [w547] -> w498
        tunnel: [w548] -> w496
        tunnel: w523 -> [_]
        shift-right: [w544] -> w514
        shift-left: w501 -> [w545]
        tunnel: w504 -> [w542]
        stop <- w549 stop-if-true
        n287 = node-c288() -> ()  [unwired: 1 in, 1 out]
        n288 = event shown="[2] \"Primary Video Display\": Mouse Down" {
          selector: _ -> [_ _ _ _]
          dyn-events: _ -> [_ _ _ _]
          timeout: 10 -> [_ _ _ _]
          tunnel: w553 -> [w564 w579 w588 w607]
          tunnel: w552 -> [w563 w581 w586 w609]
          tunnel: w551 -> [w562 w580 w587 w608]
          tunnel: [w561 w579 w588 w607] -> w550
          tunnel: [w554 w583 FALSE FALSE] -> w549
          tunnel: [w558 w581 w586 w609] -> w548
          tunnel: [w557 w580 w587 w608] -> w547
          tunnel: "radius" -> [_ _ w593 _]
          tunnel: w545 -> [w555 w582 w591 _]
          tunnel: [w555 w582 w592 cluster{i32, i32, i32, i32}[] []] -> w544
          tunnel: w542 -> [_ _ w584 _]
          event Timeout {
            n289 = event-data() -> ()  [unwired: 1 in, 2 out]
            n290 = call <vilib>:"IMAQ Grab Acquire.vi"("error in (no error)"=w563, "Image In"=w562, "IMAQ Session In"=w564) -> ("error out"=w559:errorcluster, "Image Out"=w560:T2, "IMAQ Session Out"=w561:refnum<k11>)  [unwired: 5 in, 1 out]
            n291 = case shown="True" "trap\nmarkers?" {
              tunnel: w555 -> [_ w572]
              tunnel: w560 -> [w566 w571]
              tunnel: w559 -> [w565 w570]
              tunnel: [w565 w569] -> w558
              tunnel: [w566 w567] -> w557
              frame False {
              }
              frame True {
                n292 = for {
                  tunnel: w572 -> [w578] mode=indexing
                  shift-right: [w576] -> w567
                  shift-left: w571 -> [w577]
                  tunnel: w570 -> [w575]
                  tunnel: [w574] -> w569
                  tunnel: u32 16711680 ("Color") -> [w573]
                  n293 = call "IMAQ Overlay Oval"("Color"=w573, "error in (no error)"=w575, "Bounding Rectangle"=w578, "Image"=w577) -> ("error out"=w574:errorcluster, "Image Out"=w576:T2)  [unwired: 6 in]
                }
              }
            }
            "Primary Video Display" <- w557
            n294 = Unbundle By Name(w559) -> ("status"=w554:bool)
          }
          event "Stop All": Value Change {
            n295 = event-data() -> ()  [unwired: 1 in, 5 out]
            n296 = local read "Stop All"() -> (w583:bool)
          }
          event "Primary Video Display": Mouse Down {
            n297 = event-data() -> ()  [unwired: 1 in, 7 out]
            n298 = Array Size(array=w591) -> (size(s)=w590:i32)
            n299 = Less?(x=w590, y=w584) -> (x < y?=w589:bool)
            n300 = case shown="True" w589 {
              tunnel: w593 -> [_ w603]
              tunnel: w591 -> [w594 w597]
              tunnel: [w594 w596] -> w592
              frame False {
              }
              frame True {
                n301 = property on="Primary Video Display" class="ImageControl"() -> ("Last Mouse Position"=w595:cluster{"X":i32, "Y":i32})  [unwired: 2 in, 2 out]
                n302 = Unbundle By Name(w595) -> ("X"=w605:i32, "Y"=w604:i32)
                n303 = Add(x=w604, y=w603) -> (x+y=w601:i32)
                n304 = Subtract(x=w604, y=w603) -> (x-y=w599:i32)
                n305 = Add(x=w605, y=w603) -> (x+y=w600:i32)
                n306 = Subtract(x=w605, y=w603) -> (x-y=w602:i32)
                n307 = Bundle(w602, w601, w600, w599) -> (w598:cluster{i32, i32, i32, i32})  [unwired: 1 in]
                n308 = Build Array (concatenate)(w597, w598) -> (w596:T28)
              }
            }
          }
          event "clear markers": Value Change {
            n309 = event-data() -> ()  [unwired: 1 in, 5 out]
          }
        }
        n310 = node-c288() -> ()  [unwired: 1 in, 1 out]
      }
      n311 = node-c288(w524) -> ()  [unwired: 1 out]
      n312 = Set File Position(offset (in bytes) (0)=i64 0, refnum=w505, from (0:start)=enum16{"start", "end", "current"}."start") -> (refnum out=w506:refnum<file>)  [unwired: 1 in, 1 out]
      n313 = for "Write trap positions to file so they can be remembered\nwhen program is removed from memory" {
        tunnel: w514 -> [w538] mode=indexing
        tunnel: [w536] -> w513
        tunnel: w506 -> [w535]
        n314 = Cluster To Array(cluster=w538) -> (array=w537:i32[])
        n315 = for {
          tunnel: w537 -> [w541] mode=indexing
          tunnel: [w540] -> w536
          tunnel: w535 -> [w539]
          n316 = Write to Binary File(file (use dialog)=w539, data=w541) -> (refnum out=w540:refnum<file>)  [unwired: 4 in, 2 out]
        }
      }
      n317 = Close File(refnum=w513) -> ()  [unwired: 1 in, 2 out]
      n318 = call "IMAQ Dispose"("Image"=w498, "error in (no error)"=w496) -> ("error out"=w495:errorcluster)  [unwired: 4 in]
      n319 = call <vilib>:"IMAQ Stop.vi"("error in (no error)"=w495, "IMAQ Session In"=w497) -> ("error out"=w499:errorcluster, "IMAQ Session Out"=w500:refnum<k11>)  [unwired: 8 in]
      n320 = call <vilib>:"IMAQ Close.vi"("error in (no error)"=w499, "IMAQ Session In"=w500) -> ()  [unwired: 9 in, 1 out]
    }
    frame Enabled {
    }
  }
  n321 = node-c288(2 ("Processor")) -> (w15:T24)  [unwired: 3 in]
  n322 = node-c288() -> (w69:T24)  [unwired: 4 in]
  n323 = disable-structure shown="Enabled" {
    disable-tunnel: [w616 _] -> w35
    disable-tunnel: w24 -> [w615 _]
    frame Enabled {
      n324 = node-c288() -> (w618:T24)  [unwired: 4 out]
      n325 = timed-loop "Rough control of MCL mirror stage (debugging)" {
        tunnel: w615 -> [w621]
        tunnel: [w620] -> w616
        timing: w618 -> [_]
        timing-out: [_] -> w617
        stop <- w620 stop-if-true
        n326 = node-c288() -> ()  [unwired: 2 out]
        n327 = case shown="0, Default" "MCL Mode" {
          tunnel: w621 -> [_ w624 w671]
          frame 0, Default {
            # "manual positioning"
          }
          frame 1 {
            # "sinusoidal wave"
            n328 = node-c288() -> (w626:T24)  [unwired: 4 out]
            n329 = timed-loop "Oscillate MCL mirror" {
              timing: w626 -> [_]
              timing-out: [_] -> w625
              tunnel: w624 -> [w665]
              i -> [w664]
              stop <- w627 stop-if-true
              n330 = node-c288() -> (w663:i64)  [unwired: 1 out]
              n331 = Multiply(x="AO1", y=32767.0) -> (x*y=w659:dbl)
              n332 = Multiply(x="AO2", y=32767.0) -> (x*y=w654:dbl)
              n333 = Divide(x=w659, y=10.0) -> (x/y=w660:dbl)
              n334 = Divide(x=w654, y=10.0) -> (x/y=w655:dbl)
              n335 = To Word Integer(number=w660) -> (16bit integer=w652:i16)
              n336 = To Word Integer(number=w655) -> (16bit integer=w651:i16)
              n337 = Divide(x=w663, y=i64 1000) -> (x/y=w634:dbl)
              n338 = Multiply(x=w634, y=w664) -> (x*y=w645:dbl)
              n339 = Multiply(x="Osc. freq. (Hz) 2", y=6.283185307179586) -> (x*y=w646:dbl)
              n340 = Multiply(x=w646, y=w645) -> (x*y=w644:dbl)
              n341 = Sine(x=w644) -> (sin(x)=w643:dbl)
              n342 = Multiply(x=w643, y="Osc. amp. (V)") -> (x*y=w641:dbl)
              n343 = Add(x=w641, y="Osc. center (V)") -> (x+y=w639:dbl)
              n344 = Divide(x=w639, y=10.0) -> (x/y=w637:dbl)
              n345 = Multiply(x=w637, y=32767.0) -> (x*y=w632:dbl)
              n346 = Select(t=w632, s="Scan axis", f=w652) -> (s? t:f=w650:dbl)
              n347 = Select(t=w651, s="Scan axis", f=w632) -> (s? t:f=w649:dbl)
              n348 = local read "MCL Mode"() -> (w631:u16)
              n349 = Not Equal?(x=w631, y=u16 1) -> (x != y?=w628:bool)
              n350 = local read "Stop All"() -> (w629:bool)
              n351 = xnode "Read/Write Control"("FPGA VI Reference In"=w665, "AO1"=w650, "AO2"=w649) -> ()  [unwired: 1 in, 2 out]
              n352 = Compound Arithmetic op=OR(w629, w628) -> (w627:bool)
              n353 = node-c288() -> ()  [unwired: 2 out]
            }
            n354 = node-c288(w625) -> ()  [unwired: 1 out]
          }
          frame 2 {
            # "linear scan"
            n355 = case shown="True" "Start Scan" {
              tunnel: w671 -> [_ w683]
              frame False {
              }
              frame True {
                n356 = Subtract(x="End (V)", y="Begin (V)") -> (x-y=w679:dbl)
                n357 = Decrement(x="N Points") -> (x-1=w678:dbl)
                n358 = Divide(x=w679, y=w678) -> (x/y=w676:dbl)
                n359 = for {
                  N: "N Points" -> [_]
                  tunnel: "Begin (V)" -> [w696]
                  tunnel: w683 -> [w688]
                  tunnel: [w687] -> w682 mode=indexing
                  tunnel: w676 -> [w686]
                  tunnel: [w684] -> w675 mode=indexing
                  i -> [w695]
                  n360 = Multiply(x=w686, y=w695) -> (x*y=w694:dbl)
                  n361 = Add(x=w696, y=w694) -> (x+y=w691:dbl)
                  n362 = local read "Scan axis"() -> (w685:bool)
                  n363 = local read "AO1"() -> (w693:dbl)
                  n364 = local read "AO2"() -> (w692:dbl)
                  n365 = Select(t=w691, s=w685, f=w693) -> (s? t:f=w690:dbl)
                  n366 = Select(t=w692, s=w685, f=w691) -> (s? t:f=w689:dbl)
                  n367 = flat-sequence {
                    tunnel: w690 -> [w700]
                    tunnel: w689 -> [w699]
                    tunnel: w688 -> [w697]
                    tunnel: [w710] -> w687
                    tunnel: [w709] -> w684
                    frame #0 {
                      w703 = 10.0 ("y")
                      w698 = 32767.0 ("y")
                      n368 = Multiply(x=w700, y=w698) -> (x*y=w706:dbl)
                      n369 = Multiply(x=w699, y=w698) -> (x*y=w704:dbl)
                      n370 = Divide(x=w706, y=w703) -> (x/y=w707:dbl)
                      n371 = Divide(x=w704, y=w703) -> (x/y=w705:dbl)
                      n372 = To Word Integer(number=w707) -> (16bit integer=w701:i16)
                      n373 = To Word Integer(number=w705) -> (16bit integer=w702:i16)
                      n374 = xnode "Read/Write Control"("FPGA VI Reference In"=w697, "AO1"=w701, "AO2"=w702) -> ()  [unwired: 1 in, 2 out]
                    }
                    frame #1 {
                      n375 = Wait (ms)(milliseconds to wait="DAQ Delay (ms)") -> ()  [unwired: 1 out]
                    }
                    frame #2 {
                      n376 = local read "Slow mean"() -> (w710:dbl)
                      n377 = local read "Sigma"() -> (w709:dbl)
                    }
                  }
                }
                n378 = Bundle("Begin (V)"="Begin (V)", w676, w682) -> (→"MCL Scan":cluster{"Begin (V)":dbl, dbl, dbl[]})  [unwired: 1 out]
                n379 = Bundle("Begin (V)"="Begin (V)", w676, w675) -> (→"MCL Scan 2":cluster{"Begin (V)":dbl, dbl, dbl[]})  [unwired: 1 out]
              }
            }
          }
        }
        n380 = local read "Stop All"() -> (w620:bool)
        n381 = node-c288() -> ()  [unwired: 2 out]
      }
      n382 = node-c288(w617) -> ()  [unwired: 1 out]
    }
    frame Disabled {
    }
  }
  n383 = timed-loop "Control parameters (event loop)" {
    tunnel: w24 -> [w716]
    shift-right: [w715] -> _
    shift-left: errorcluster {"status"=FALSE, "code"=0, "source"=""} ("error out") -> [w714]
    tunnel: [w713] -> w37
    timing: w15 -> [_]
    timing-out: [_] -> w14
    stop <- w713 stop-if-true
    n384 = node-c288() -> ()  [unwired: 1 in, 1 out]
    n385 = event shown="[6] \"BD 1 Frequency 1 (MHz)\", \"BD 1 Frequency 2 (MHz)\", \"BD 1 Frequency 3 (MHz)\", \"BD 2 Frequency 1 (MHz)\", \"BD 2 Frequency 2 (MHz)\", \"BD 2 Frequency 3 (MHz)\", \"Trap Delta (MHz)\": Value Change" {
      selector: _ -> [_ _ _ _ _ _ _ _ _ _ _ _ _ _ _ _ _ _ _ _ _ _ _ _ _ _ _ _ _ _ _ _ _ _ _ _ _ _ _ _ _ _ _ _ _ _ _ _ _ _ _ _ _ _ _]
      dyn-events: _ -> [_ _ _ _ _ _ _ _ _ _ _ _ _ _ _ _ _ _ _ _ _ _ _ _ _ _ _ _ _ _ _ _ _ _ _ _ _ _ _ _ _ _ _ _ _ _ _ _ _ _ _ _ _ _ _]
      timeout: _ -> [_ _ _ _ _ _ _ _ _ _ _ _ _ _ _ _ _ _ _ _ _ _ _ _ _ _ _ _ _ _ _ _ _ _ _ _ _ _ _ _ _ _ _ _ _ _ _ _ _ _ _ _ _ _ _]
      tunnel: w716 -> [w754 _ _ _ w791 _ w813 _ w880 _ _ _ w923 _ _ w966 w972 w977 w983 w1019 w1037 w1044 w1062 w1073 w1084 w1095 w1106 w1117 w1135 w1141 w1235 _ w1244 w1282 _ w1317 w1321 w1332 w1336 w1340 _ w1348 _ _ _ _ w1481 _ w1498 w1501 w1510 w1513 w1517 _ w1534]
      tunnel: [w753 _ _ _ w781 _ w812 _ w843 _ w888 _ w902 _ _ w965 w968 w974 w980 w1018 w1035 w1043 w1056 w1067 w1078 w1089 w1100 w1111 w1133 w1140 w1233 _ w1242 w1280 _ w1315 w1319 w1322 w1334 w1338 _ w1346 _ _ _ _ w1479 _ _ _ _ _ _ _ _] -> w715
      tunnel: w714 -> [w752 _ _ _ w790 _ w811 _ w875 _ w888 _ w922 _ _ w964 w967 w973 w979 w1017 w1036 w1042 w1061 w1072 w1083 w1094 w1105 w1116 w1134 w1139 w1234 _ w1243 w1281 _ w1316 w1320 w1331 w1335 w1339 _ w1347 _ _ _ _ w1480 _ w1497 w1500 w1509 w1512 w1516 _ w1533]
      tunnel: [_ _ _ _ _ _ _ _ _ _ w887 _ _ _ _ _ _ _ _ _ _ _ _ _ _ _ _ _ _ _ _ _ _ _ _ _ _ _ _ _ _ _ _ _ _ _ _ _ _ _ _ _ _ _ _] -> w713
      tunnel: [_ _ _ _ _ _ _ "Round T1 X" _ _ _ _ _ _ _ _ _ _ _ _ _ _ _ _ _ _ _ _ _ _ _ _ _ _ _ _ _ _ _ _ _ _ _ _ _ _ _ _ _ _ _ _ _ _ _] -> _
      tunnel: [_ _ _ "Adjust Scale\nto Mean" _ _ _ _ _ _ _ _ _ _ _ _ _ _ _ _ _ _ _ _ _ _ _ _ _ _ _ _ _ _ _ _ _ _ _ _ _ _ _ _ _ _ _ _ _ _ _ _ "Set SP to Reading" _ _] -> _
      tunnel: [_ _ _ _ _ _ _ _ _ "Round T2 X" _ "Delayed Interlace Start" _ _ _ _ _ _ _ _ _ _ _ _ _ _ _ _ _ _ _ _ _ _ _ _ _ _ _ _ _ _ _ _ _ _ _ _ _ _ _ _ _ _ _] -> _
      event "AI Count (ticks)", "Sets to FIFO (Traps)", "Save ave N", "FPGA Ave.", "# Samples/channel", "N sets to save": Value Change {
        # "So that if 'Save ave N' is updated, the AOD scanning code updates too."
        n386 = event-data() -> ()  [unwired: 6 out]
        n387 = local read "AI Count (ticks)"() -> (w734:u32)
        n388 = Boolean To (0,1)(Boolean="Sets to FIFO (Traps)") -> (0, 1=w744:cluster{"Set 1":i16, "Set 2":i16, "Set 3":i16})
        n389 = xnode "Read/Write Control"("FPGA VI Reference In"=w754, "error in"=w752, "ai count"=w734, "AI1 Sets to FIFO"="Sets to FIFO (Traps)", "N of AI1 Int Acq Sets"="N Acq Sets (Traps + Fl.)") -> ("error out"=w753:errorcluster)  [unwired: 1 out]
        n390 = Cluster To Array(cluster=w744) -> (array=w743:i16[])
        n391 = To Unsigned Long Integer(number=w743) -> (unsigned 32bit integer=w723:u32[])
        n392 = local read "Scan steps (AOD)"() -> (w745:u64)
        n393 = Multiply(x=w734, y="N Acq Sets (Traps + Fl.)") -> (x*y=w732:u32)
        n394 = Divide(x=40000000.0, y=w734) -> (x/y=w726:dbl)
        "AI rate (Hz)" <- w726
        "Ave. Rate (Hz)" <- w726
        n395 = Add Array Elements(numeric array=w723) -> (sum=w735:u32)
        "Trap Sets" <- w735
        n396 = Reciprocal(x=w726) -> (1/x=→"Ave. Period (s)":dbl)
        n397 = property on="Scan steps (AOD)" class="DigNum (strict)"("Val(Sgnl)"=w745) -> ()  [unwired: 2 in, 2 out]
        n398 = Divide(x=w726, y="N Acq Sets (Traps + Fl.)") -> (x/y=w749:dbl)
        "Data Rate (Hz)" <- w749
        n399 = Reciprocal(x=w749) -> (1/x=→"Data Period (s)":dbl)
        n400 = local read "Save ave N"() -> (w748:dbl)
        n401 = Divide(x=w749, y=w748) -> (x/y=w747:dbl)
        "Save Data Rate (Hz)" <- w747
        n402 = Reciprocal(x=w747) -> (1/x=→"Save Data Period (s)":dbl)
        n403 = Multiply(x=w732, y="# Samples/trap") -> (x*y=w730:u32)
        "Counts/DMA" <- w730
        n404 = property on="Trap Disp. Downsample" class="DigNum (strict)"("Maximum"="# Samples/trap") -> ()  [unwired: 2 in, 2 out]
        n405 = Multiply(x=w735, y="# Samples/trap") -> (x*y=w724:u32)
        "# Samples/channel" <- w724
        n406 = Multiply(x=w724, y=u32 8) -> (x*y=→"Trap AI Elements/DMA read":u32)
        n407 = local read "APD Int. Count"() -> (w731:u32)
        n408 = Multiply(x=w724, y=u32 3) -> (x*y=→"Trap Pos Elements/DMA read":u32)
        n409 = Divide(x=w730, y=w731) -> (x/y=w721:dbl)
        "APD Samples/FIFO Acq." <- w721
        n410 = Divide(x=w730, y=40000000.0) -> (x/y=w728:dbl)
        "DMA Update Period (s)" <- w728
        n411 = Multiply(x=2.0, y=w721) -> (x*y=→"APD Elements/DMA read":dbl)
        n412 = property on="APD Disp. Downsample" class="DigNum (strict)"("Maximum"=w721) -> ()  [unwired: 2 in, 2 out]
        n413 = local read "N sets to save"() -> (w741:u32)
        n414 = Multiply(x=w728, y=w741) -> (x*y=→"Total Time (s)":dbl)
        "FPGA Averaging" <- FALSE ("FPGA Averaging")
      }
      event "Rescale on Mean": Value Change {
        n415 = event-data() -> ()  [unwired: 7 out]
        n416 = And(x=FALSE, y="Rescale on Mean") -> (x .and. y?=w756:bool)
        n417 = local write "Rescale on Mean"(w756) -> ()
        n418 = local read "Bead Mean (nm)"() -> (w761:dbl)
        n419 = Add(x="Amplitude (nm)", y=w761) -> (x+y=w759:dbl)
        n420 = Subtract(x=w761, y="Amplitude (nm)") -> (x-y=w758:dbl)
        n421 = property on="Bead Separation" class="WFChart (strict)"("YScale.Minimum"=w758) -> ()  [unwired: 2 in, 2 out]
        n422 = property on="Bead Separation" class="WFChart (strict)"("YScale.Maximum"=w759) -> ()  [unwired: 2 in, 2 out]
      }
      event "Detector Type": Value Change {
        n423 = event-data() -> ()  [unwired: 7 out]
        n424 = local read "AI labels"() -> (w762:string[])
        n425 = property on="High Res. Display" class="Ring (strict)"("Strings []"=w762) -> ()  [unwired: 2 in, 2 out]
        n426 = Build Array (concatenate)(w762, "none") -> (w763:string[])
        n427 = property on="FFT 1 Choice 1" class="Ring (strict)"("Strings []"=w763) -> ()  [unwired: 2 in, 2 out]
        n428 = property on="FFT 1 Choice 2" class="Ring (strict)"("Strings []"=w763) -> ()  [unwired: 2 in, 2 out]
        n429 = property on="FFT 2 Choice 1" class="Ring (strict)"("Strings []"=w763) -> ()  [unwired: 2 in, 2 out]
        n430 = property on="FFT 2 Choice 2" class="Ring (strict)"("Strings []"=w763) -> ()  [unwired: 2 in, 2 out]
        n431 = Bundle("APD 1", "APD 2") -> (w766:cluster{string, string})  [unwired: 1 out]
        n432 = Cluster To Array(cluster=w766) -> (array=w764:string[])
        n433 = Build Array (concatenate)(w764, w763) -> (w768:string[])
        n434 = Array Size(array=w768) -> (size(s)=w769:i32)
        n435 = property on="Signals to Plot" class="LstBox (strict)"("Item Names"=w768) -> ()  [unwired: 2 in, 2 out]
        n436 = property on="Signals to Plot" class="LstBox (strict)"("Number of Rows"=w769) -> ()  [unwired: 2 in, 2 out]
        n437 = property on="All Signals" class="WFChart (strict)"("LegNumRows"=w769) -> ()  [unwired: 2 in, 2 out]
      }
      event "Adjust Scale\nto Mean": Value Change {
        n438 = event-data() -> ()  [unwired: 7 out]
        n439 = local read "APD 1 Rate (Hz)"() -> (w778:dbl)
        n440 = Multiply(x=1000.0, y="Above (kHz)") -> (x*y=w776:dbl)
        n441 = Multiply(x=1000.0, y="Below (kHz)") -> (x*y=w774:dbl)
        n442 = Add(x=w776, y=w778) -> (x+y=w771:dbl)
        n443 = Subtract(x=w778, y=w774) -> (x-y=w772:dbl)
        n444 = property on="APD Chart" class="WFChart (strict)"("YScale.Minimum"=w772) -> ()  [unwired: 2 in, 2 out]
        n445 = property on="APD Chart" class="WFChart (strict)"("YScale.Maximum"=w771) -> ()  [unwired: 2 in, 2 out]
      }
      event "Phase adj. (AI1)", "+ phase (AI1)", "- phase (AI1)": Value Change {
        n446 = event-data() -> ()  [unwired: 7 out]
        n447 = Negate(x="Phase adj. (AI1)") -> (-x=w788:i16)
        n448 = Select(t=w788, s="- phase (AI1)", f="Phase adj. (AI1)") -> (s? t:f=w787:i16)
        n449 = xnode "Read/Write Control"("FPGA VI Reference In"=w791, "error in"=w790, "Phase count adjustment"=w787) -> ("FPGA VI Reference Out"=w786:T19, "error out"=w785:errorcluster)
        n450 = Or(x="- phase (AI1)", y="+ phase (AI1)") -> (x .or. y?=w782:bool)
        n451 = xnode "Read/Write Control"("FPGA VI Reference In"=w786, "error in"=w785, "+ phase"=w782) -> ("error out"=w781:errorcluster)  [unwired: 1 out]
      }
      event "Signals to Plot": Double Click {
        w794 = u32 9868950 ("Color Box")
        n452 = event-data() -> ("Row"=w796:i32)  [unwired: 9 out]
        n453 = property on="All Signals" class="WFChart (strict)"("Active Plot"=w796) -> (error out=w807:errorcluster)  [unwired: 2 in, 1 out]
        n454 = property on="All Signals" class="WFChart (strict)" props=["Plot", "Visible?", "Plot", "Plot Color"](error in=w807) -> (error out=w806:errorcluster, "Plot.Visible?"=w805:bool)  [unwired: 1 in, 2 out]
        n455 = Select(t=FALSE ("Plot.Visible"), s=w805, f=TRUE ("Plot.Visible")) -> (s? t:f=w800:bool)
        n456 = property on="All Signals" class="WFChart (strict)"(error in=w806, "Plot.Visible?"=w800) -> (error out=w802:errorcluster)  [unwired: 1 in, 1 out]
        n457 = property on="All Signals" class="WFChart (strict)"(error in=w802) -> (error out=w797:errorcluster, "Plot.Plot Color"=w801:u32)  [unwired: 1 in, 1 out]
        n458 = property on="Signals to Plot" class="LstBox (strict)"(error in=w797, "Active Row"=w796) -> (error out=w795:errorcluster)  [unwired: 1 in, 1 out]
        n459 = Select(t=w801, s=w800, f=u32 0) -> (s? t:f=w798:u32)
        n460 = property on="Signals to Plot" class="LstBox (strict)"(error in=w795, "CellFontColor"=w798, "SelColor"=w794, "CellBG"=w794, "CellFontSize"=u32 20 ("Active Row:Cell Font:Size"), "CellFontBold"=TRUE ("Active Row:Cell Font:Bold")) -> ()  [unwired: 1 in, 2 out]
      }
      event "BD 1 Frequency 1 (MHz)", "BD 1 Frequency 2 (MHz)", "BD 1 Frequency 3 (MHz)", "BD 2 Frequency 1 (MHz)", "BD 2 Frequency 2 (MHz)", "BD 2 Frequency 3 (MHz)", "Trap Delta (MHz)": Value Change {
        # "anytime one of the frequencies is changed, write it to the RF board UNLESS Set 2 is being oscillated. The oscillation\nscript writes the frequencies to the RF board."
        n461 = event-data() -> ("CtlRef"=w810:refnum<vi>)  [unwired: 6 out]
        n462 = control-ref of="Trap Delta (MHz)"() -> (w809:refnum<vi>)
        n463 = Equal?(x=w809, y=w810) -> (x = y?=w808:bool)
        n464 = case shown="False" "Oscillate Set 2" {
          tunnel: w813 -> [w836 _]
          tunnel: [w835 w839] -> w812
          tunnel: w811 -> [w834 w839]
          tunnel: w808 -> [w821 _]
          frame False {
            w815 = 75
            n465 = local read "BD 1 Frequency 2 (MHz)"() -> (w823:dbl)
            n466 = Divide(x="Trap Delta (MHz)", y=2) -> (x/y=w817:dbl)
            n467 = Subtract(x=w815, y=w817) -> (x-y=w816:dbl)
            n468 = local write "BD 1 Frequency 1 (MHz)"(w816) -> ()
            n469 = Add(x=w815, y=w817) -> (x+y=w822:dbl)
            n470 = Select(t=w822, s=w821, f=w823) -> (s? t:f=w820:dbl)
            n471 = local read "Y RF Frequency Limits (MHz)"() -> (w824:T16)
            n472 = local read "X RF Frequency Limits (MHz)"() -> (w825:T16)
            n473 = local read "BD 1 Frequency 3 (MHz)"() -> (w837:dbl)
            n474 = local write "BD 1 Frequency 2 (MHz)"(w820) -> ()
            n475 = local read "BD 2 Frequency 1 (MHz)"() -> (w828:dbl)
            n476 = local read "BD 2 Frequency 2 (MHz)"() -> (w827:dbl)
            n477 = local read "BD 2 Frequency 3 (MHz)"() -> (w838:dbl)
            n478 = call "set RF board frequency - interlace.vi"("Board 2 Frequency Limits"=w824, "Board 1 Frequency Limits"=w825, "error in"=w834, "FPGA VI Reference In"=w836, "Board 2 Frequency 3 (MHz)"=w838, "Board 1 Frequency 3 (MHz)"=w837, "Board 2 Frequency 2 (MHz)"=w827, "Board 2 Frequency 1 (MHz)"=w828, "Board 1 Frequency 2 (MHz)"=w820, "Board 1 Frequency 1  (MHz)"=w816) -> ("error out"=w835:errorcluster)  [unwired: 1 out]
            n479 = Subtract(x=w828, y=w827) -> (x-y=w832:dbl)
            n480 = Subtract(x=w820, y=w816) -> (x-y=w833:dbl)
            n481 = Square(x=w832) -> (x^2=w830:dbl)
            n482 = Square(x=w833) -> (x^2=w831:dbl)
            n483 = Add(x=w831, y=w830) -> (x+y=w829:dbl)
            n484 = Square Root(x=w829) -> (sqrt(x)=w826:dbl)
            n485 = local write "Trap Delta (MHz)"(w826) -> ()
            n486 = property on="Initial delta (MHz)" class="DigNum (strict)"("Val(Sgnl)"=w826) -> ()  [unwired: 2 in, 2 out]
          }
          frame True {
          }
        }
      }
      event "Round T1 X": Value Change {
        n487 = event-data() -> ()  [unwired: 7 out]
        n488 = local read "BD 1 Frequency 1 (MHz)"() -> (w842:dbl)
        n489 = Round To Nearest(number=w842) -> (nearest integer value=w841:dbl)
        n490 = property on="BD 1 Frequency 1 (MHz)" class="DigNum (strict)"("Val(Sgnl)"=w841) -> ()  [unwired: 2 in, 2 out]
      }
      event "Restart RF": Value Change {
        n491 = event-data() -> ()  [unwired: 7 out]
        n492 = xnode "Read/Write Control"("FPGA VI Reference In"=w880, "error in"=w875, "FPGA Controls  RF Box"=FALSE) -> ("FPGA VI Reference Out"=w879:T19, "error out"=w874:errorcluster)
        n493 = local read "Y RF Amplitude Limits (%)"() -> (w855:T16)
        n494 = local read "X RF Amplitude Limits (%)"() -> (w856:T16)
        n495 = local read "X RF Frequency Limits (MHz)"() -> (w858:T16)
        n496 = local read "Y RF Frequency Limits (MHz)"() -> (w857:T16)
        n497 = xnode "Read/Write Control"("FPGA VI Reference In"=w879, "error in"=w874, "Direct RF Box  Communication"=TRUE) -> ("FPGA VI Reference Out"=w878:T19, "error out"=w873:errorcluster)
        n498 = local read "BD 2 Frequency 3 (MHz)"() -> (w865:dbl)
        n499 = local read "BD 2 Frequency 2 (MHz)"() -> (w866:dbl)
        n500 = local read "BD 1 Frequency 3 (MHz)"() -> (w869:dbl)
        n501 = local read "BD 1 Frequency 1 (MHz)"() -> (w870:dbl)
        n502 = local read "BD 2 Frequency 1 (MHz)"() -> (w867:dbl)
        n503 = local read "BD 1 Frequency 2 (MHz)"() -> (w868:dbl)
        n504 = call "Initialize RF boards - interlace 3.vi"("error in"=w873, "FPGA VI Reference In"=w878) -> ("error out"=w872:errorcluster, "FPGA VI Reference Out"=w877:T19)
        n505 = local read "BD 2 Amplitude 2 (%)"() -> (w860:dbl)
        n506 = local read "BD 2 Amplitude 1 (%)"() -> (w861:dbl)
        n507 = local read "BD 2 Amplitude 3 (%)"() -> (w859:dbl)
        n508 = local read "BD 1 Amplitude 3 (%)"() -> (w864:dbl)
        n509 = local read "BD 1 Amplitude 1 (%)"() -> (w863:dbl)
        n510 = local read "BD 1 Amplitude 2 (%)"() -> (w862:dbl)
        n511 = call "set RF board frequency - interlace.vi"("Board 2 Frequency Limits"=w857, "Board 1 Frequency Limits"=w858, "error in"=w872, "FPGA VI Reference In"=w877, "Board 2 Frequency 3 (MHz)"=w865, "Board 1 Frequency 3 (MHz)"=w869, "Board 2 Frequency 2 (MHz)"=w866, "Board 2 Frequency 1 (MHz)"=w867, "Board 1 Frequency 2 (MHz)"=w868, "Board 1 Frequency 1  (MHz)"=w870) -> ("error out"=w871:errorcluster, "FPGA VI Reference Out"=w876:T19)
        n512 = call "set RF board amplitude - interlace.vi"("Board 2 Amplitude Limits"=w855, "Board 1 Amplitude Limits"=w856, "error in"=w871, "FPGA VI Reference In"=w876, "Board 2 Amplitude 3 (%)"=w859, "Board 1 Amplitude 3 (%)"=w864, "Board 2 Amplitude 2 (%)"=w860, "Board 2 Amplitude 1 (%)"=w861, "Board 1 Amplitude 2 (%)"=w862, "Board 1 Amplitude 1 (%)"=w863) -> ("error out"=w848:errorcluster, "FPGA VI Reference Out"=w852:T19)
        n513 = xnode "Read/Write Control"("FPGA VI Reference In"=w852, "error in"=w848, "Direct RF Box  Communication"=FALSE) -> ("FPGA VI Reference Out"=w851:T19, "error out"=w850:errorcluster)
        n514 = flat-sequence {
          tunnel: w850 -> [w881]
          tunnel: [w881] -> w849
          frame #0 {
            n515 = Wait (ms)(milliseconds to wait=u32 50) -> ()  [unwired: 1 out]
          }
        }
        n516 = xnode "Read/Write Control"("FPGA VI Reference In"=w851, "error in"=w849, "FPGA Controls  RF Box"=TRUE) -> ("error out"=w844:errorcluster)  [unwired: 1 out]
        n517 = property on="Restart RF" class="Bool (strict)"(error in=w844, "Value"=FALSE ("Restart RF")) -> (error out=w843:errorcluster)  [unwired: 1 in, 1 out]
      }
      event "Round T2 X": Value Change {
        n518 = event-data() -> ()  [unwired: 7 out]
        n519 = local read "BD 1 Frequency 2 (MHz)"() -> (w884:dbl)
        n520 = Round To Nearest(number=w884) -> (nearest integer value=w883:dbl)
        n521 = property on="BD 1 Frequency 2 (MHz)" class="DigNum (strict)"("Val(Sgnl)"=w883) -> ()  [unwired: 2 in, 2 out]
      }
      event "Stop All": Value Change {
        n522 = event-data() -> ()  [unwired: 7 out]
        n523 = call "hamilton_controller.vi"("action"=T20."DISCONNECT") -> ()  [unwired: 10 in, 1 out]
        n524 = local read "Stop All"() -> (w887:bool)
      }
      event "Delayed Interlace Start": Value Change {
        n525 = event-data() -> ()  [unwired: 7 out]
        n526 = flat-sequence {
          frame #0 {
            n527 = Multiply(x="Delay to Interlace (s)", y=1000.0) -> (x*y=w890:dbl)
            n528 = Wait (ms)(milliseconds to wait=w890) -> ()  [unwired: 1 out]
          }
          frame #1 {
            n529 = property on="Green laser mode" class="RadioBtnsControl (strict)"("Val(Sgnl)"=enum32{"Laser ON", "Laser OFF", "Interlace"}."Interlace" ("Value (Signaling)")) -> ()  [unwired: 2 in, 2 out]
          }
        }
      }
      event "BD 1 Amplitude 1 (%)", "BD 1 Amplitude 2 (%)", "BD 1 Amplitude 3 (%)", "BD 2 Amplitude 1 (%)", "BD 2 Amplitude 2 (%)", "BD 2 Amplitude 3 (%)", "Trap 1 ON", "Trap 2 ON", "Trap 3 ON", "Feedback On/Off", "All FB On/Off": Value Change {
        w914 = i16 1 ("f")
        n530 = event-data() -> ()  [unwired: 7 out]
        n531 = local write "Trap 1 (ON/OFF)"("Trap 1 ON") -> ()
        n532 = local write "Trap 2 (ON/OFF)"("Trap 2 ON") -> ()
        n533 = Boolean To (0,1)(Boolean="Trap 3 ON") -> (0, 1=w915:i16)
        n534 = Boolean To (0,1)(Boolean="Trap 1 ON") -> (0, 1=w916:i16)
        n535 = Boolean To (0,1)(Boolean="Trap 2 ON") -> (0, 1=w917:i16)
        n536 = Select(t=w917, s="Trap ON/OFF X or Y Amp?", f=w914) -> (s? t:f=w912:i16)
        n537 = Select(t=w916, s="Trap ON/OFF X or Y Amp?", f=w914) -> (s? t:f=w913:i16)
        n538 = Select(t=w915, s="Trap ON/OFF X or Y Amp?", f=w914) -> (s? t:f=w911:i16)
        n539 = Select(t=w914, s="Trap ON/OFF X or Y Amp?", f=w917) -> (s? t:f=w909:i16)
        n540 = Select(t=w914, s="Trap ON/OFF X or Y Amp?", f=w916) -> (s? t:f=w910:i16)
        n541 = Select(t=w914, s="Trap ON/OFF X or Y Amp?", f=w915) -> (s? t:f=w908:i16)
        n542 = And(x="All FB On/Off", y="Feedback On/Off") -> (x .and. y?=w906:cluster{"Set 1":bool, "Set 2":bool})
        n543 = local read "BD 1 Amplitude 1 (%)"() -> (w926:dbl)
        n544 = local read "BD 1 Amplitude 2 (%)"() -> (w925:dbl)
        n545 = local read "BD 1 Amplitude 3 (%)"() -> (w924:dbl)
        n546 = Unbundle By Name(w906) -> ("Set 1"=w901:bool, "Set 2"=w898:bool)
        n547 = local read "Y RF Amplitude Limits (%)"() -> (w894:T16)
        n548 = local read "X RF Amplitude Limits (%)"() -> (w895:T16)
        n549 = local read "BD 2 Amplitude 1 (%)"() -> (w927:dbl)
        n550 = local read "BD 2 Amplitude 2 (%)"() -> (w928:dbl)
        n551 = local read "BD 2 Amplitude 3 (%)"() -> (w929:dbl)
        n552 = And(x="Trap 2 ON", y=w898) -> (x .and. y?=w896:bool)
        n553 = And(x="Trap 1 ON", y=w901) -> (x .and. y?=w899:bool)
        n554 = Multiply(x=w913, y=w926) -> (x*y=w921:dbl)
        n555 = Multiply(x=w925, y=w912) -> (x*y=w919:dbl)
        n556 = Multiply(x=w924, y=w911) -> (x*y=w920:dbl)
        n557 = Multiply(x=w927, y=w910) -> (x*y=w930:dbl)
        n558 = Multiply(x=w928, y=w909) -> (x*y=w931:dbl)
        n559 = Multiply(x=w929, y=w908) -> (x*y=w932:dbl)
        n560 = call "set RF board amplitude - interlace.vi"("Board 2 Amplitude Limits"=w894, "Board 1 Amplitude Limits"=w895, "error in"=w922, "FPGA VI Reference In"=w923, "Board 2 Amplitude 3 (%)"=w932, "Board 1 Amplitude 3 (%)"=w920, "Board 2 Amplitude 2 (%)"=w931, "Board 2 Amplitude 1 (%)"=w930, "Board 1 Amplitude 2 (%)"=w919, "Board 1 Amplitude 1 (%)"=w921) -> ("error out"=w903:errorcluster, "FPGA VI Reference Out"=w904:T19)
        n561 = xnode "Read/Write Control"("FPGA VI Reference In"=w904, "error in"=w903, "FB On/Off Set 1"=w899, "FB On/Off Set 2"=w896) -> ("error out"=w902:errorcluster)  [unwired: 1 out]
      }
      event "Load parameters": Value Change {
        n562 = event-data() -> ()  [unwired: 7 out]
        n563 = property on="Saved AOD Raster Scan Parameter Sets" class="Arr (strict)"() -> ("Index Values"=w943:u32[])  [unwired: 2 in, 2 out]
        n564 = Index Array(array=w943, index=0) -> (element=w940:u32)
        n565 = local write "Load parameters"(FALSE ("Load parameters")) -> ()
        n566 = Index Array(array="Saved AOD Raster Scan Parameter Sets", index=w940) -> (element=w939:T30)
        n567 = Unbundle By Name(w939) -> ("Scan Range AOD (nm) 2"=w938:dbl, "Step Size AOD (nm) 2"=w937:dbl, "Scan Speed AOD (nm/s) 2"=w936:dbl, "Number of scans (AOD) 2"=w935:u16)
        n568 = flat-sequence {
          tunnel: w938 -> [w946]
          tunnel: w937 -> [w945]
          tunnel: w936 -> [w944]
          tunnel: w935 -> [w947]
          frame #0 {
            n569 = local write "Scan Speed (nm/s)"(w944) -> ()
            n570 = local write "Scan Range (nm)"(w946) -> ()
            n571 = local write "Step Size (nm)"(w945) -> ()
          }
          frame #1 {
            n572 = property on="Number of F/B Scans (AOD)" class="DigNum (strict)"("Val(Sgnl)"=w947) -> ()  [unwired: 2 in, 2 out]
          }
        }
      }
      event "Trap 1 (ON/OFF)", "Trap 2 (ON/OFF)": Value Change {
        n573 = event-data() -> ()  [unwired: 7 out]
        n574 = property on="Trap 2 ON" class="Bool (strict)"("Val(Sgnl)"="Trap 2 (ON/OFF)") -> ()  [unwired: 2 in, 2 out]
        n575 = property on="Trap 1 ON" class="Bool (strict)"("Val(Sgnl)"="Trap 1 (ON/OFF)") -> ()  [unwired: 2 in, 2 out]
      }
      event "DIO count 1 (ticks)", "DIO count 2 (ticks)", "DIO count 3 (ticks)", "Interlace", "Number Interlace Sets", "Not-Interlacing Set": Value Change {
        n576 = event-data() -> ()  [unwired: 7 out]
        n577 = local read "DIO count 3 (ticks)"() -> (w960:u32)
        n578 = local read "DIO count 1 (ticks)"() -> (w962:u32)
        n579 = local read "DIO count 2 (ticks)"() -> (w961:u32)
        n580 = To Unsigned Byte Integer(number="Not-Interlacing Set") -> (unsigned 8bit integer=w951:u8)
        n581 = Add(x=w951, y=u8 1) -> (x+y=w955:u8)
        n582 = xnode "Read/Write Control"("FPGA VI Reference In"=w966, "error in"=w964, "DIO count 1 (ticks)"=w962, "DIO count 2 (ticks)"=w961, "DIO count 3 (ticks)"=w960, "Interlace ON/OFF"="Interlace", "Number Interlace Cycles"="Number Interlace Sets", "Interlace Off Parameters"=w955) -> ("error out"=w965:errorcluster)  [unwired: 1 out]
        n583 = Build Array(w962, w961, w960) -> (w953:u32[])
        n584 = Split 1D Array(array=w953, index="Number Interlace Sets") -> (first subarray=w963:u32[])  [unwired: 1 out]
        n585 = Index Array(array=w953, index=w951) -> (element=w952:u32)
        n586 = Add Array Elements(numeric array=w963) -> (sum=w957:u32)
        n587 = Select(t=w957, s="Interlace", f=w952) -> (s? t:f=→"Total Counts (ticks)":u32)
      }
      event "Reset Feedback": Value Change {
        n588 = event-data() -> ()  [unwired: 7 out]
        n589 = Unbundle By Name("Reset Feedback") -> ("Set 1"=w970:bool, "Set 2"=w969:bool)
        n590 = xnode "Read/Write Control"("FPGA VI Reference In"=w972, "error in"=w967, "FB Reset Set 1"=w970, "FB Reset Set 2"=w969) -> ("error out"=w968:errorcluster)  [unwired: 1 out]
      }
      event "PID Gains": Value Change {
        n591 = event-data() -> ()  [unwired: 7 out]
        n592 = Unbundle By Name("PID Gains") -> ("Set 1"=w976:T14, "Set 2"=w975:T14)
        n593 = xnode "Read/Write Control"("FPGA VI Reference In"=w977, "error in"=w973, "FB Gains Set 1"=w976, "FB Gains Set 2"=w975) -> ("error out"=w974:errorcluster)  [unwired: 1 out]
      }
      event "AI2 to Setpoint", "Trap Intensity\nSetpoints (V)": Value Change {
        n594 = event-data() -> ()  [unwired: 7 out]
        n595 = xnode "Read/Write Control"("FPGA VI Reference In"=w983, "error in"=w979) -> ("FPGA VI Reference Out"=w982:T19, "error out"=w981:errorcluster, "AI2 Y Sum Set 1"=w990:i16, "AI2 Y Sum Set 2"=w989:i16)
        n596 = Cluster To Array(cluster="AI2 to Setpoint") -> (array=w993:bool[])
        n597 = local read "AI2 (V)"() -> (w991:cluster{"Set 1":dbl, "Set 2":dbl})
        n598 = Or Array Elements(Boolean array=w993) -> (logical OR=w994:bool)
        n599 = Bundle By Name(cluster=w991, "Set 1"=w990, "Set 2"=w989) -> (w988:cluster{"Set 1":dbl, "Set 2":dbl})
        n600 = Divide(x=w988, y=3276.7) -> (x/y=w987:cluster{"Set 1":dbl, "Set 2":dbl})
        "AI2 (V)" <- w987
        n601 = case shown="True" w994 {
          tunnel: [w997 w1014] -> w986
          tunnel: "AI2 to Setpoint" -> [_ w1010]
          tunnel: "Trap Intensity\nSetpoints (V)" -> [w998 w1013]
          tunnel: w987 -> [_ w1007]
          frame False {
            n602 = Multiply(x=3276.7, y=w998) -> (x*y=w999:cluster{"Set 1":dbl, "Set 2":dbl})
            n603 = To Word Integer(number=w999) -> (16bit integer=w997:cluster{"Set 1":i16, "Set 2":i16})
          }
          frame True {
            n604 = Unbundle By Name(w1007) -> ("Set 1"=w1006:dbl, "Set 2"=w1005:dbl)
            n605 = Unbundle By Name(w1013) -> ("Set 1"=w1012:dbl, "Set 2"=w1011:dbl)
            n606 = Unbundle By Name(w1010) -> ("Set 1"=w1009:bool, "Set 2"=w1008:bool)
            n607 = Select(t=w1006, s=w1009, f=w1012) -> (s? t:f=w1004:dbl)
            n608 = Select(t=w1005, s=w1008, f=w1011) -> (s? t:f=w1003:dbl)
            n609 = Bundle By Name(cluster=w1013, "Set 1"=w1004, "Set 2"=w1003) -> (w1001:cluster{"Set 1":dbl, "Set 2":dbl})
            n610 = local write "Trap Intensity\nSetpoints (V)"(w1001) -> ()
            n611 = Multiply(x=3276.7, y=w1001) -> (x*y=w1002:cluster{"Set 1":dbl, "Set 2":dbl})
            n612 = To Word Integer(number=w1002) -> (16bit integer=w1014:cluster{"Set 1":i16, "Set 2":i16})
          }
        }
        n613 = Unbundle By Name(w986) -> ("Set 1"=w985:i16, "Set 2"=w984:i16)
        n614 = xnode "Read/Write Control"("FPGA VI Reference In"=w982, "error in"=w981, "FB Setpoint Set 1"=w985, "FB Setpoint Set 2"=w984) -> ("error out"=w980:errorcluster)  [unwired: 1 out]
      }
      event "Invert GI": Value Change {
        n615 = event-data() -> ()  [unwired: 7 out]
        n616 = xnode "Read/Write Control"("FPGA VI Reference In"=w1019, "error in"=w1017, "Invert GI"="Invert GI", "Invert GI 2"="Invert GI") -> ("error out"=w1018:errorcluster)  [unwired: 1 out]
      }
      event "Green FB Setpoint (mV)", "Green FB Gains", "Green FB On/Off", "Current When FB OFF (%)", "Green int current ON count adj": Value Change {
        n617 = event-data() -> ()  [unwired: 7 out]
        n618 = local read "Green FB Setpoint (mV)"() -> (w1026:dbl)
        n619 = local read "Current When FB OFF (%)"() -> (w1029:dbl)
        n620 = Multiply(x=w1026, y=3.2767) -> (x*y=w1025:dbl)
        n621 = Multiply(x=w1029, y=655.35) -> (x*y=w1030:dbl)
        n622 = To Unsigned Word Integer(number=w1030) -> (unsigned 16bit integer=w1028:u16)
        n623 = local read "Green int current ON count adj"() -> (w1033:u32)
        n624 = local read "Green FB Gains"() -> (w1032:T14)
        n625 = local read "Green Laser ON/Interlacing"() -> (w1023:bool)
        n626 = local read "Green laser mode"() -> (w1022:enum32{"Laser ON", "Laser OFF", "Interlace"})
        n627 = local read "Green FB On/Off"() -> (w1034:bool)
        n628 = Equal?(x=w1022, y=enum32{"Laser ON", "Laser OFF", "Interlace"}."Interlace") -> (x = y?=w1020:bool)
        n629 = Compound Arithmetic op=AND(w1020, w1034, w1023) -> (w1024:bool)
        n630 = xnode "Read/Write Control"("FPGA VI Reference In"=w1037, "error in"=w1036, "Green FB Setpoint"=w1025, "Green FB On/Off"=w1024, "Current Out"=w1028, "Green int current ON count adj"=w1033, "Green FB Gains"=w1032) -> ("error out"=w1035:errorcluster)  [unwired: 1 out]
      }
      event "Green laser mode", "Green Laser ON/Interlacing": Value Change {
        n631 = event-data() -> ()  [unwired: 7 out]
        n632 = case shown="True" "Green Laser ON/Interlacing" {
          tunnel: "Green laser mode" -> [_ w1051]
          tunnel: [enum32{"Laser ON", "Laser OFF", "Interlace"}."Laser OFF" ("Green laser mode") w1051] -> w1039
          tunnel: [FALSE w1047] -> w1038
          frame False {
          }
          frame True {
            n633 = local read "Green FB On/Off"() -> (w1048:bool)
            n634 = Equal?(x=w1051, y=enum32{"Laser ON", "Laser OFF", "Interlace"}."Interlace") -> (x = y?=w1049:bool)
            n635 = And(x=w1049, y=w1048) -> (x .and. y?=w1047:bool)
          }
        }
        n636 = xnode "Read/Write Control"("FPGA VI Reference In"=w1044, "error in"=w1042, "Operating Mode"=w1039, "Operating Mode 2"=w1039, "Green FB On/Off"=w1038) -> ("error out"=w1043:errorcluster)  [unwired: 1 out]
      }
      event "- phase (APD 1 Gate)", "+ phase (APD 1 Gate)": Value Change {
        n637 = event-data() -> ()  [unwired: 7 out]
        n638 = local read "Phase Adj. (APD 1 Gate)"() -> (w1052:i16)
        n639 = Negate(x=w1052) -> (-x=w1060:i16)
        n640 = Select(t=w1060, s="- phase (APD 1 Gate)", f=w1052) -> (s? t:f=w1059:i16)
        n641 = Or(x="- phase (APD 1 Gate)", y="+ phase (APD 1 Gate)") -> (x .or. y?=w1055:bool)
        n642 = xnode "Read/Write Control"("FPGA VI Reference In"=w1062, "error in"=w1061, "Phase count adjustment (APD 1 Gate)"=w1059) -> ("FPGA VI Reference Out"=w1057:T19, "error out"=w1058:errorcluster)
        n643 = xnode "Read/Write Control"("FPGA VI Reference In"=w1057, "error in"=w1058, "+ phase (APD 1 Gate)"=w1055) -> ("error out"=w1056:errorcluster)  [unwired: 1 out]
      }
      event "+ phase (APD 2 Gate)", "- phase (APD 2 Gate)": Value Change {
        n644 = event-data() -> ()  [unwired: 7 out]
        n645 = local read "Phase Adj. (APD 2 Gate)"() -> (w1063:i16)
        n646 = Negate(x=w1063) -> (-x=w1071:i16)
        n647 = Select(t=w1071, s="- phase (APD 2 Gate)", f=w1063) -> (s? t:f=w1070:i16)
        n648 = Or(x="- phase (APD 2 Gate)", y="+ phase (APD 2 Gate)") -> (x .or. y?=w1066:bool)
        n649 = xnode "Read/Write Control"("FPGA VI Reference In"=w1073, "error in"=w1072, "Phase count adjustment (APD 2 Gate)"=w1070) -> ("FPGA VI Reference Out"=w1068:T19, "error out"=w1069:errorcluster)
        n650 = xnode "Read/Write Control"("FPGA VI Reference In"=w1068, "error in"=w1069, "+ phase (APD 2 Gate)"=w1066) -> ("error out"=w1067:errorcluster)  [unwired: 1 out]
      }
      event "Phase Adj. (APD Acq)", "+ phase (APD Acq)", "- phase (APD Acq)": Value Change {
        n651 = event-data() -> ()  [unwired: 7 out]
        n652 = local read "Phase Adj. (APD Acq)"() -> (w1076:i16)
        n653 = Negate(x=w1076) -> (-x=w1082:i16)
        n654 = Select(t=w1082, s="+ phase (APD Acq)", f=w1076) -> (s? t:f=w1081:i16)
        n655 = Or(x="+ phase (APD Acq)", y="- phase (APD Acq)") -> (x .or. y?=w1077:bool)
        n656 = xnode "Read/Write Control"("FPGA VI Reference In"=w1084, "error in"=w1083, "Phase Count Adjustment (APD Acq)"=w1081) -> ("FPGA VI Reference Out"=w1079:T19, "error out"=w1080:errorcluster)
        n657 = xnode "Read/Write Control"("FPGA VI Reference In"=w1079, "error in"=w1080, "+ phase (APD Acq)"=w1077) -> ("error out"=w1078:errorcluster)  [unwired: 1 out]
      }
      event "Phase adj. (GI)", "+ phase (GI)", "- phase (GI)": Value Change {
        n658 = event-data() -> ()  [unwired: 7 out]
        n659 = Negate(x="Phase adj. (GI)") -> (-x=w1093:i16)
        n660 = Select(t=w1093, s="+ phase (GI)", f="Phase adj. (GI)") -> (s? t:f=w1092:i16)
        n661 = Or(x="+ phase (GI)", y="- phase (GI)") -> (x .or. y?=w1088:bool)
        n662 = xnode "Read/Write Control"("FPGA VI Reference In"=w1095, "error in"=w1094, "Phase count adjustment (GI)"=w1092) -> ("FPGA VI Reference Out"=w1090:T19, "error out"=w1091:errorcluster)
        n663 = xnode "Read/Write Control"("FPGA VI Reference In"=w1090, "error in"=w1091, "+ phase (GI)"=w1088) -> ("error out"=w1089:errorcluster)  [unwired: 1 out]
      }
      event "Phase adj. (GI) 2", "+ phase (GI) 2", "- phase (GI) 2": Value Change {
        n664 = event-data() -> ()  [unwired: 7 out]
        n665 = Negate(x="Phase adj. (GI) 2") -> (-x=w1104:i16)
        n666 = Select(t=w1104, s="+ phase (GI) 2", f="Phase adj. (GI) 2") -> (s? t:f=w1103:i16)
        n667 = Or(x="+ phase (GI) 2", y="- phase (GI) 2") -> (x .or. y?=w1099:bool)
        n668 = xnode "Read/Write Control"("FPGA VI Reference In"=w1106, "error in"=w1105, "Phase count adjustment (GI) 2"=w1103) -> ("FPGA VI Reference Out"=w1101:T19, "error out"=w1102:errorcluster)
        n669 = xnode "Read/Write Control"("FPGA VI Reference In"=w1101, "error in"=w1102, "+ phase (GI) 2"=w1099) -> ("error out"=w1100:errorcluster)  [unwired: 1 out]
      }
      event "Phase adj. (Green FB)", "- phase (Green FB)", "+ phase (Green FB)": Value Change {
        n670 = event-data() -> ()  [unwired: 7 out]
        n671 = Negate(x="Phase adj. (Green FB)") -> (-x=w1115:i16)
        n672 = Select(t=w1115, s="+ phase (Green FB)", f="Phase adj. (Green FB)") -> (s? t:f=w1114:i16)
        n673 = Or(x="+ phase (Green FB)", y="- phase (Green FB)") -> (x .or. y?=w1110:bool)
        n674 = xnode "Read/Write Control"("FPGA VI Reference In"=w1117, "error in"=w1116, "Phase count adjustment (Green FB)"=w1114) -> ("FPGA VI Reference Out"=w1112:T19, "error out"=w1113:errorcluster)
        n675 = xnode "Read/Write Control"("FPGA VI Reference In"=w1112, "error in"=w1113, "+ phase (Green FB)"=w1110) -> ("error out"=w1111:errorcluster)  [unwired: 1 out]
      }
      event "Invert APD Gate", "APD Gate ON Count", "APD Gate OFF Count", "APD Gate", "APD Integration Time (s)", "APD 1 AO Mult.", "APD 2 AO Mult.": Value Change {
        n676 = event-data() -> ()  [unwired: 7 out]
        n677 = local read "APD Integration Time (s)"() -> (w1118:dbl)
        n678 = local read "APD Gate ON Count"() -> (w1131:u32)
        n679 = local read "APD Gate OFF Count"() -> (w1130:u32)
        n680 = local read "Invert APD Gate"() -> (w1132:bool)
        n681 = local read "APD Gate"() -> (w1129:enum32{"ON", "OFF", "Interlace"})
        n682 = Multiply(x=w1118, y=40000000.0) -> (x*y=w1127:dbl)
        n683 = Reciprocal(x=w1118) -> (1/x=→"APD Acq Rate (Hz)":dbl)
        n684 = To Unsigned Long Integer(number=w1127) -> (unsigned 32bit integer=w1126:u32)
        n685 = local read "DMA Update Period (s)"() -> (w1119:dbl)
        n686 = Divide(x=w1119, y=w1118) -> (x/y=w1122:dbl)
        n687 = local read "APD 1 AO Mult."() -> (w1124:i16)
        n688 = local read "APD 2 AO Mult."() -> (w1123:i16)
        n689 = Multiply(x=2.0, y=w1122) -> (x*y=w1121:dbl)
        n690 = local write "APD Samples/FIFO Acq."(w1122) -> ()
        n691 = local write "APD Elements/DMA read"(w1121) -> ()
        n692 = xnode "Read/Write Control"("FPGA VI Reference In"=w1135, "error in"=w1134, "Invert APD Gate"=w1132, "APD Gate ON Count"=w1131, "APD Gate OFF Count"=w1130, "APD Acq Rate Count"=w1126, "APD Gate Operating Mode"=w1129, "APD 1 AO scale factor"=w1124, "APD 2 AO scale factor"=w1123) -> ("error out"=w1133:errorcluster)  [unwired: 1 out]
      }
      event "GI Frequency, ON count", "Green FB Count", "GI Frequency, OFF count": Value Change {
        n693 = event-data() -> ()  [unwired: 7 out]
        n694 = xnode "Read/Write Control"("FPGA VI Reference In"=w1141, "error in"=w1139, "Green interlace ON count"="GI Frequency, ON count", "Green interlace OFF count"="GI Frequency, OFF count", "Green interlace ON count 2"="GI Frequency, ON count", "Green interlace OFF count 2"="GI Frequency, OFF count", "Green FB Count"="Green FB Count") -> ("error out"=w1140:errorcluster)  [unwired: 1 out]
      }
      event "Number of F/B Scans (AOD)", "Scan Speed (nm/s)", "Scan BD", "Initial delta (MHz)", "Step Size (nm)", "Scan Range (nm)": Value Change {
        w1203 = 123.0  # AOM cal (nm/MHz)
        n695 = event-data() -> ()  [unwired: 7 out]
        n696 = local read "BD 1 Frequency 1 (MHz)"() -> (w1186:dbl)
        n697 = local read "AOM X Cal (nm/MHz)"() -> (w1178:dbl)
        n698 = local read "X RF Frequency Limits (MHz)"() -> (w1190:T16)
        n699 = local read "Y RF Frequency Limits (MHz)"() -> (w1187:T16)
        n700 = local read "BD 2 Frequency 1 (MHz)"() -> (w1192:dbl)
        n701 = Negate(x="Scan Range (nm)") -> (-x=w1156:dbl)
        n702 = Divide(x=w1156, y=w1178) -> (x/y=w1160:dbl)
        n703 = Select(t=w1190, s="Scan BD", f=w1187) -> (s? t:f=w1189:T16)
        n704 = Select(t=w1186, s="Scan BD", f=w1192) -> (s? t:f=w1191:dbl)
        n705 = Unbundle By Name(w1189) -> ("Maximum"=w1198:dbl, "Minimum"=w1197:dbl)
        n706 = Add(x=w1160, y=w1191) -> (x+y=w1195:dbl)
        n707 = Divide(x=w1156, y="Step Size (nm)") -> (x/y=w1175:dbl)
        n708 = Divide(x="Step Size (nm)", y=w1178) -> (x/y=w1184:dbl)
        n709 = Absolute Value(x=w1175) -> (abs(x)=w1159:dbl)
        n710 = Sign(1:w1156) -> (0:w1157:dbl)
        n711 = In Range and Coerce(upper limit=w1198, x=w1195, lower limit=w1197) -> (coerced(x)=w1194:dbl, In Range?=w1196:bool)
        n712 = To Unsigned Quad Integer(1:w1159) -> (0:w1174:u64)
        "Scan steps (AOD)" <- w1174
        n713 = call "IR AOM freq to word.vi"("Frequency In (MHz)"=w1184) -> ("Frequency Word Out (double)"=w1181:dbl)
        n714 = Multiply(x=w1157, y=w1181) -> (x*y=w1158:dbl)
        n715 = Subtract(x=w1195, y=w1194) -> (x-y=w1193:dbl)
        n716 = To Quad Integer(1:w1158) -> (0:w1180:i64)
        "Incr. int (AOD)" <- w1180
        n717 = Subtract(x=w1160, y=w1193) -> (x-y=w1179:dbl)
        "Scan Range (MHz)" <- w1179
        n718 = Select(t=w1160, s=w1196, f=w1179) -> (s? t:f=w1199:dbl)
        n719 = Multiply(x=w1179, y=w1178) -> (x*y=w1177:dbl)
        n720 = Decrement(x=w1174) -> (x-1=w1227:u64)
        n721 = Negate(x=w1177) -> (-x=w1173:dbl)
        n722 = local write "Scan Range (nm)"(w1173) -> ()
        n723 = Divide(x=w1199, y=w1227) -> (x/y=w1183:dbl)
        "Scan Increment (MHz)" <- w1183
        n724 = call "IR AOM freq to word.vi"("Frequency In (MHz)"=w1183) -> ("Frequency Word Out (double)"=w1182:dbl)
        n725 = Divide(x="Step Size (nm)", y="Scan Speed (nm/s)") -> (x/y=w1170:dbl)
        n726 = To Quad Integer(1:w1182) -> ()  [unwired: 1 out]
        n727 = local read "Number Interlace Sets"() -> (w1154:u8)
        n728 = local read "AI Count (ticks)"() -> (w1155:u32)
        n729 = local read "Total Counts (ticks)"() -> (w1153:u32)
        n730 = local read "# Samples/trap"() -> (w1185:u32)
        n731 = Multiply(x=w1155, y=w1154) -> (x*y=w1152:u32)
        n732 = Divide(x=w1153, y=w1152) -> (x/y=w1151:dbl)
        n733 = Select(t=w1186, s="Scan BD", f=w1192) -> (s? t:f=w1224:dbl)
        "Initial freq. (MHz)" <- w1224
        n734 = Add(x=w1199, y=w1224) -> (x+y=→"Final freq. (MHz)":dbl)
        n735 = Divide(x=w1153, y=40000000.0) -> (x/y=w1169:dbl)
        n736 = Divide(x=w1170, y=w1169) -> (x/y=w1168:dbl)
        n737 = To Unsigned Quad Integer(1:w1168) -> (0:w1143:u64)
        n738 = Quotient & Remainder(x=w1143, y=u64 2) -> (x-y*floor(x/y)=w1147:u64)  [unwired: 1 out]
        n739 = Equal?(x=w1147, y=u64 0) -> (x = y?=w1145:bool)
        n740 = Decrement(x=w1143) -> (x-1=w1144:u64)
        n741 = Select(t=w1143, s=w1145, f=w1144) -> (s? t:f=w1142:u64)
        "Cycles/step (AOD)" <- w1142
        n742 = xnode "Read/Write Control"("FPGA VI Reference In"=w1235, "error in"=w1234, "Scan steps"=w1174, "Number of scans"="Number of F/B Scans (AOD)", "Cycles per step"=w1142, "Scan freq.  increment"=w1180, "Scan BD"="Scan BD") -> ("error out"=w1233:errorcluster)  [unwired: 1 out]
        n743 = Multiply(x=w1174, y=w1142) -> (x*y=w1228:u64)
        n744 = Multiply(x=w1228, y=u64 2) -> (x*y=w1150:u64)
        n745 = Multiply(x=w1151, y=w1150) -> (x*y=w1149:dbl)
        "Data points/scan (f/b)" <- w1149
        n746 = Multiply(x=w1149, y="Number of F/B Scans (AOD)") -> (x*y=w1231:dbl)
        "Data points/scans" <- w1231
        n747 = Divide(x=w1231, y=w1185) -> (x/y=→"N sets should be saved":dbl)
        n748 = Multiply(x=w1228, y=w1169) -> (x*y=w1167:dbl)
        "Time/Scan (s) (AOD)" <- w1167
        n749 = Select(t=w1199, s="Scan BD", f=0.0) -> (s? t:f=w1225:dbl)
        n750 = Select(t=0.0, s="Scan BD", f=w1199) -> (s? t:f=w1221:dbl)
        n751 = local read "BD 2 Frequency 2 (MHz)"() -> (w1217:dbl)
        n752 = local read "BD 1 Frequency 2 (MHz)"() -> (w1220:dbl)
        n753 = Add(x=w1221, y=w1192) -> (x+y=w1218:dbl)
        n754 = Add(x=w1186, y=w1225) -> (x+y=w1219:dbl)
        n755 = Multiply(x=w1167, y=2.0) -> (x*y=w1166:dbl)
        n756 = Multiply(x=w1166, y="Number of F/B Scans (AOD)") -> (x*y=w1163:dbl)
        n757 = Divide(x=w1163, y=60.0) -> (x/y=→"Time to Finish All (min)":dbl)
        n758 = Add(x="Trap 2 Bead Size (nm)", y="Trap 1 Bead Size (nm)") -> (x+y=w1207:dbl)
        n759 = local read "Initial delta (MHz)"() -> (w1204:dbl)
        n760 = Divide(x=w1207, y=2.0) -> (x/y=w1201:dbl)
        n761 = Subtract(x=w1218, y=w1217) -> (x-y=w1215:dbl)
        n762 = Subtract(x=w1219, y=w1220) -> (x-y=w1216:dbl)
        n763 = Square(x=w1215) -> (x^2=w1214:dbl)
        n764 = Square(x=w1216) -> (x^2=w1213:dbl)
        n765 = Add(x=w1213, y=w1214) -> (x+y=w1212:dbl)
        n766 = Square Root(x=w1212) -> (sqrt(x)=w1211:dbl)
        "Final delta (MHz)" <- w1211
        n767 = Multiply(x=w1203, y=w1211) -> (x*y=w1210:dbl)
        n768 = Multiply(x=w1204, y=w1203) -> (x*y=w1202:dbl)
        n769 = Subtract(x=w1202, y=w1201) -> (x-y=→"Initial sep (nm)":dbl)
        n770 = Subtract(x=w1210, y=w1201) -> (x-y=→"Final sep (nm)":dbl)
      }
      event "Raster Scanning...": Value Change {
        n771 = event-data() -> ("NewVal"=w1236:bool)  [unwired: 6 out]
        n772 = case shown="True" w1236 {
          frame False {
          }
          frame True {
            n773 = property on="BD 1 Frequency 1 (MHz)" class="DigNum (strict)"("Val(Sgnl)"=65.0 ("Value (Signaling)")) -> ()  [unwired: 2 in, 2 out]
          }
        }
      }
      event "Freq or Amp switch first", "Swap F1 and F2", "Freq switch delay", "Amp switch delay": Value Change {
        n774 = event-data() -> ()  [unwired: 7 out]
        n775 = local read "Freq or Amp switch first"() -> (w1238:bool)
        n776 = local read "Amp switch delay"() -> (w1239:u16)
        n777 = local read "Freq switch delay"() -> (w1241:u16)
        n778 = local read "Swap F1 and F2"() -> (w1240:bool)
        n779 = xnode "Read/Write Control"("FPGA VI Reference In"=w1244, "error in"=w1243, "Freq switch delay"=w1241, "Swap F1 and F2"=w1240, "Amp switch delay"=w1239, "Freq or Amp switch first"=w1238) -> ("error out"=w1242:errorcluster)  [unwired: 1 out]
      }
      event "Scan steps (MCL)", "Number of scans (MCL)", "Scan Range (V)\n(of steps)", "2D or 1D Scan", "N APD Samp/step", "Fast Scan Dir", "Continuous MCL Scanning", "Scan lines (y)": Value Change {
        w1246 = 32767.0 ("y")
        n780 = event-data() -> ()  [unwired: 7 out]
        n781 = Select(t="Scan lines (y)", s="2D or 1D Scan", f="Number of scans (MCL)") -> (s? t:f=w1251:u64)
        n782 = Decrement(x="Scan steps (MCL)") -> (x-1=w1267:u64)
        n783 = Divide(x="Scan Range (V)\n(of steps)", y=w1267) -> (x/y=w1266:dbl)
        "Desired Scan Incr (V)" <- w1266
        n784 = local read "APD Integration Time (s)"() -> (w1259:dbl)
        n785 = Multiply(x=w1266, y=w1246) -> (x*y=w1275:dbl)
        n786 = Divide(x=w1275, y=10.0) -> (x/y=w1265:dbl)
        "Desired incr (int)" <- w1265
        n787 = local read "Update Count (MCL)"() -> (w1271:u32)
        n788 = Round Toward -Infinity(1:w1265) -> (0:w1274:dbl)
        n789 = To Word Integer(number=w1274) -> (16bit integer=w1249:i16)
        "Actual Incr. int (MCL)" <- w1249
        n790 = Multiply(x=w1259, y=40000000.0) -> (x*y=w1272:dbl)
        n791 = Divide(x=w1272, y=w1271) -> (x/y=w1270:dbl)
        n792 = Multiply(x=i16 10, y=w1249) -> (x*y=w1247:i16)
        n793 = Multiply(x="N APD Samp/step", y=w1270) -> (x*y=w1269:dbl)
        "Cycles/step (MCL)" <- w1269
        n794 = Divide(x=w1247, y=w1246) -> (x/y=→"Actual MCL Inc (V)":dbl)
        n795 = Multiply(x="N APD Samp/step", y="Scan steps (MCL)") -> (x*y=w1261:dbl)
        n796 = local read "APD Samples/FIFO Acq."() -> (w1258:dbl)
        n797 = Multiply(x=w1261, y=u64 2) -> (x*y=w1260:dbl)
        "Data points/scan (f+b)" <- w1260
        n798 = Multiply(x=w1260, y=w1251) -> (x*y=w1278:dbl)
        "Data points/scans (MCL)" <- w1278
        n799 = Multiply(x=w1259, y=w1260) -> (x*y=w1252:dbl)
        "Time/f+b scan (s) (MCL)" <- w1252
        n800 = Divide(x=w1278, y=w1258) -> (x/y=→"N sets should be saved (MCL)":dbl)
        n801 = Multiply(x=w1252, y=w1251) -> (x*y=→"Total Time (s)":dbl)
        n802 = Not(x="Fast Scan Dir") -> (.not. x?=w1256:bool)
        n803 = xnode "Read/Write Control"("FPGA VI Reference In"=w1282, "error in"=w1281, "Scan steps (MCL)"="Scan steps (MCL)", "Number of scans (MCL)"=w1251, "Cycles per step (MCL)"=w1269, "Scan freq.  increment (MCL)"=w1249, "1D or 2D Scan?"="2D or 1D Scan", "MCL Scan Axis"=w1256, "Cont. Scan (MCL)"="Continuous MCL Scanning") -> ("error out"=w1280:errorcluster)  [unwired: 1 out]
      }
      event "Read Cal": Value Change {
        w1284 = 1000.0 ("y")
        n804 = event-data() -> ()  [unwired: 7 out]
        n805 = local read "Save file name"() -> (w1309:path)
        n806 = local write "Read Cal"(FALSE ("Read Cal")) -> ()
        n807 = Strip Path(path=w1309) -> (stripped path=w1308:path)  [unwired: 1 out]
        n808 = Path To String(path=w1308) -> (string=w1307:string)
        n809 = Concatenate Strings(w1307, "\\current.cal" ("string")) -> (w1305:string)
        n810 = String To Path(string=w1305) -> (path=w1304:path)
        n811 = Open/Create/Replace File(file path (use dialog)=w1304, operation (0:open)=T23."open", access (0:read/write)=enum16{"read/write", "read-only", "write-only"}."read-only") -> (refnum out=w1312:refnum<file>, error out=w1298:errorcluster)  [unwired: 1 in, 3 out]
        n812 = Deny Access(4:w1298, 7:w1312) -> (0:w1297:errorcluster, 3:w1303:refnum<file>)  [unwired: 1 out]
        n813 = Read from Binary File(5:0.0, 8:w1297, 9:T29."big-endian, network order" ("byte order (0:big-endian, network order)"), 10:-1 ("count (1)"), 11:w1303) -> (0:w1296:errorcluster, 2:w1294:dbl[], 3:w1299:refnum<file>)  [unwired: 2 out]
        n814 = Array To Cluster(array=w1294) -> (cluster=w1293:T31)
        n815 = Unbundle(w1293) -> ("[0]"=w1292:dbl, "[1]"=w1291:dbl, "[2]"=w1290:dbl, "[3]"=w1289:dbl, "[4]"=w1288:dbl, "[5]"=w1287:dbl)
        n816 = Close File(refnum=w1299, error in=w1296) -> (error out=→"Read cal error":errorcluster)  [unwired: 1 out]
        n817 = Multiply(x=w1287, y=w1284) -> (x*y=w1285:dbl)
        n818 = local write "T2 kappa_x (pN/nm)"(w1289) -> ()
        n819 = local write "T1 kappa_x (pN/nm)"(w1290) -> ()
        n820 = local write "T1 alpha_x (nm/V)"(w1292) -> ()
        n821 = local write "T2 alpha_x (nm/V)"(w1291) -> ()
        n822 = Multiply(x=w1288, y=w1284) -> (x*y=w1286:dbl)
        n823 = local write "T1 offset_x (mV)"(w1286) -> ()
        n824 = local write "T2 offset_x (mV)"(w1285) -> ()
      }
      event "Abort MCL Scan": Value Change {
        n825 = event-data() -> ()  [unwired: 7 out]
        n826 = local write "MCL Scanning"(FALSE ("MCL Scanning")) -> ()
        n827 = xnode "Read/Write Control"("FPGA VI Reference In"=w1317, "error in"=w1316, "Abort scan (MCL)"="Abort MCL Scan") -> ("error out"=w1315:errorcluster)  [unwired: 1 out]
      }
      event "Update Count (MCL)": Value Change {
        n828 = event-data() -> ()  [unwired: 7 out]
        n829 = xnode "Read/Write Control"("FPGA VI Reference In"=w1321, "error in"=w1320, "MCL count"="Update Count (MCL)") -> ("error out"=w1319:errorcluster)  [unwired: 1 out]
      }
      event "Phase adjust (MCL)", "+ phase (MCL)", "- phase (MCL)": Value Change {
        n830 = event-data() -> ()  [unwired: 7 out]
        n831 = Negate(x="Phase adjust (MCL)") -> (-x=w1330:i16)
        n832 = Select(t=w1330, s="- phase (MCL)", f="Phase adjust (MCL)") -> (s? t:f=w1328:i16)
        n833 = Or(x="- phase (MCL)", y="+ phase (MCL)") -> (x .or. y?=w1323:bool)
        n834 = xnode "Read/Write Control"("FPGA VI Reference In"=w1332, "error in"=w1331, "Phase count adjustment (MCL)"=w1328) -> ("FPGA VI Reference Out"=w1324:T19, "error out"=w1325:errorcluster)
        n835 = xnode "Read/Write Control"("FPGA VI Reference In"=w1324, "error in"=w1325, "+ phase (MCL)"=w1323) -> ("error out"=w1322:errorcluster)  [unwired: 1 out]
      }
      event "Abort AOD Scan": Value Change {
        n836 = event-data() -> ()  [unwired: 7 out]
        n837 = xnode "Read/Write Control"("FPGA VI Reference In"=w1336, "error in"=w1335, "Abort scan"="Abort AOD Scan") -> ("error out"=w1334:errorcluster)  [unwired: 1 out]
      }
      event "Continuous AOD Scanning": Value Change {
        n838 = event-data() -> ()  [unwired: 7 out]
        n839 = xnode "Read/Write Control"("FPGA VI Reference In"=w1340, "error in"=w1339, "Cont. Scan"="Continuous AOD Scanning") -> ("error out"=w1338:errorcluster)  [unwired: 1 out]
      }
      event "Index": Value Change {
        n840 = event-data() -> ()  [unwired: 7 out]
        n841 = call "Create new save file.vi"("Insert"="", "Ext"=".dat" ("string"), "Index In"="Index") -> ("Path Out"=→"Save file name":path, "Index Out"=w1341:dbl)
        "Save index" <- w1341
        n842 = local write "Index"(w1341) -> ()
      }
      event "AO1", "AO2": Value Change {
        w1356 = 10.0 ("y")
        w1355 = 32767.0 ("y")
        n843 = event-data() -> ()  [unwired: 7 out]
        n844 = local read "AO2"() -> (w1354:dbl)
        n845 = local read "AO1"() -> (w1351:dbl)
        n846 = Multiply(x=w1351, y=w1355) -> (x*y=w1350:dbl)
        n847 = Multiply(x=w1354, y=w1355) -> (x*y=w1353:dbl)
        n848 = Divide(x=w1350, y=w1356) -> (x/y=w1349:dbl)
        n849 = Divide(x=w1353, y=w1356) -> (x/y=w1352:dbl)
        n850 = To Word Integer(number=w1349) -> (16bit integer=w1357:i16)
        n851 = To Word Integer(number=w1352) -> (16bit integer=w1358:i16)
        n852 = xnode "Read/Write Control"("FPGA VI Reference In"=w1348, "error in"=w1347, "AO1"=w1357, "AO2"=w1358) -> ("error out"=w1346:errorcluster)  [unwired: 1 out]
      }
      event "Inject Bottom": Value Change {
        n853 = event-data() -> ()  [unwired: 7 out]
        n854 = disable-structure shown="Enabled" {
          disable-tunnel: "Inject Bottom" -> [w1360 w1400]
          frame Disabled {
            n855 = local read "Chemyx Syringe Pump Serial Port"() -> (w1361:refnum<visa-resource-name>)
            n856 = local read "Pump write delay (ms)"() -> (w1362:dbl)
            n857 = case shown="True" w1360 {
              tunnel: w1362 -> [w1368 w1382]
              tunnel: w1361 -> [w1365 w1381]
              frame False {
                n858 = flat-sequence {
                  tunnel: w1365 -> [w1369]
                  tunnel: [w1369] -> w1366
                  tunnel: w1368 -> [_]
                  tunnel: [w1372] -> w1367
                  tunnel: w1366 -> [w1372]
                  tunnel: w1367 -> [w1373]
                  tunnel: [w1373] -> w1363
                  tunnel: [w1375] -> w1364
                  tunnel: w1363 -> [w1375]
                  tunnel: w1364 -> [w1377]
                  frame #0 {
                    n859 = call "Write to pump.vi"("string"="enter pump1", "VISA resource name"=w1369) -> ()  [unwired: 1 out]
                  }
                  frame #1 {
                    n860 = Wait (ms)(milliseconds to wait="Pump pause delay (ms)") -> ()  [unwired: 1 out]
                  }
                  frame #2 {
                    n861 = call "Write to pump.vi"("string"="stop", "VISA resource name"=w1373) -> ()  [unwired: 1 out]
                  }
                  frame #3 {
                    n862 = Wait (ms)(milliseconds to wait=u32 500) -> ()  [unwired: 1 out]
                  }
                  frame #4 {
                    n863 = call "Write to pump.vi"("string"="stop", "VISA resource name"=w1377) -> ()  [unwired: 1 out]
                  }
                }
              }
              frame True {
                n864 = flat-sequence {
                  tunnel: w1381 -> [w1391]
                  tunnel: w1382 -> [w1386]
                  tunnel: w1382 -> [w1393]
                  tunnel: w1381 -> [w1394]
                  tunnel: [w1394] -> w1379
                  tunnel: [w1396] -> w1380
                  tunnel: w1379 -> [w1396]
                  tunnel: w1380 -> [w1398]
                  frame #0 {
                    n865 = local read "All Pump Parameters"() -> (w1385:T5)
                    n866 = Unbundle By Name(w1385) -> ("Pump 1"=w1392:T32)
                    n867 = call "Set pump parameters.vi"("Pump write delay (ms)"=w1386, "Volume (uL)"="Ch 2 Inject Volume (uL)", "Rate (uL/h)"="Ch 1 Inject Rate (ul/h)", "Units"=4.0, "Pump #"=1.0, "Pump Parameters In"=w1392, "VISA resource name"=w1391) -> ("Pump Parameters Out"=w1384:T32)  [unwired: 3 in]
                    n868 = Bundle By Name(cluster=w1385, "Pump 1"=w1384) -> (w1383:T5)
                    n869 = local write "All Pump Parameters"(w1383) -> ()
                  }
                  frame #1 {
                    n870 = Wait (ms)(milliseconds to wait=w1393) -> ()  [unwired: 1 out]
                  }
                  frame #2 {
                    n871 = call "Write to pump.vi"("string"="start", "VISA resource name"=w1394) -> ()  [unwired: 1 out]
                  }
                  frame #3 {
                    n872 = Wait (ms)(milliseconds to wait=u32 500) -> ()  [unwired: 1 out]
                  }
                  frame #4 {
                    n873 = call "Write to pump.vi"("string"="start", "VISA resource name"=w1398) -> ()  [unwired: 1 out]
                  }
                }
              }
            }
          }
          frame Enabled {
            n874 = call "hamilton_controller.vi"("Open?"=w1400, "valve"=enum16{"A", "B", "C", "D", "ALL"}."B", "action"=T20."MOVE VALVE") -> ()  [unwired: 8 in, 1 out]
          }
        }
      }
      event "Inject Top": Value Change {
        n875 = event-data() -> ()  [unwired: 7 out]
        n876 = disable-structure shown="Disabled" {
          disable-tunnel: "Inject Top" -> [_ w1444]
          frame Disabled {
            n877 = local read "Pump write delay (ms)"() -> (w1405:dbl)
            n878 = case shown="False" w1406 {
              tunnel: w1405 -> [w1412 w1426]
              tunnel: "Chemyx Syringe Pump Serial Port" -> [w1409 w1425]
              frame False {
                n879 = flat-sequence {
                  tunnel: w1409 -> [w1413]
                  tunnel: [w1413] -> w1410
                  tunnel: w1412 -> [_]
                  tunnel: [w1416] -> w1411
                  tunnel: w1410 -> [w1416]
                  tunnel: w1411 -> [w1417]
                  tunnel: [w1417] -> w1407
                  tunnel: [w1419] -> w1408
                  tunnel: w1407 -> [w1419]
                  tunnel: w1408 -> [w1421]
                  frame #0 {
                    n880 = call "Write to pump.vi"("string"="enter pump3", "VISA resource name"=w1413) -> ()  [unwired: 1 out]
                  }
                  frame #1 {
                    n881 = local read "Pump pause delay (ms)"() -> (w1415:u32)
                    n882 = Wait (ms)(milliseconds to wait=w1415) -> ()  [unwired: 1 out]
                  }
                  frame #2 {
                    n883 = call "Write to pump.vi"("string"="stop", "VISA resource name"=w1417) -> ()  [unwired: 1 out]
                  }
                  frame #3 {
                    n884 = Wait (ms)(milliseconds to wait=u32 0) -> ()  [unwired: 1 out]
                  }
                  frame #4 {
                    n885 = call "Write to pump.vi"("string"="stop", "VISA resource name"=w1421) -> ()  [unwired: 1 out]
                  }
                }
              }
              frame True {
                n886 = flat-sequence {
                  tunnel: w1425 -> [w1435]
                  tunnel: w1426 -> [w1430]
                  tunnel: w1426 -> [w1437]
                  tunnel: w1425 -> [w1438]
                  tunnel: [w1438] -> w1423
                  tunnel: [w1441] -> w1424
                  tunnel: w1423 -> [w1441]
                  tunnel: w1424 -> [w1442]
                  frame #0 {
                    n887 = local read "All Pump Parameters"() -> (w1429:T5)
                    n888 = Unbundle By Name(w1429) -> ("Pump 3"=w1436:T32)
                    n889 = call "Set pump parameters.vi"("Pump write delay (ms)"=w1430, "Volume (uL)"="Ch 3 Inject Volume (uL)", "Rate (uL/h)"="Ch 3 Inject Rate (ul/h)", "Units"=4.0, "Pump #"=3.0, "Pump Parameters In"=w1436, "VISA resource name"=w1435) -> ("Pump Parameters Out"=w1428:T32)  [unwired: 3 in]
                    n890 = Bundle By Name(cluster=w1429, "Pump 3"=w1428) -> (w1427:T5)
                    n891 = local write "All Pump Parameters"(w1427) -> ()
                  }
                  frame #1 {
                    n892 = Wait (ms)(milliseconds to wait=w1437) -> ()  [unwired: 1 out]
                  }
                  frame #2 {
                    n893 = call "Write to pump.vi"("string"="start", "VISA resource name"=w1438) -> ()  [unwired: 1 out]
                  }
                  frame #3 {
                    n894 = Wait (ms)(milliseconds to wait=u32 500) -> ()  [unwired: 1 out]
                  }
                  frame #4 {
                    n895 = call "Write to pump.vi"("string"="start", "VISA resource name"=w1442) -> ()  [unwired: 1 out]
                  }
                }
              }
            }
          }
          frame Enabled {
            n896 = call "hamilton_controller.vi"("Open?"=w1444, "valve"=enum16{"A", "B", "C", "D", "ALL"}."A", "action"=T20."MOVE VALVE") -> ()  [unwired: 8 in, 1 out]
          }
        }
      }
      event "Inject Valve B": Value Change {
        n897 = event-data() -> ()  [unwired: 7 out]
        n898 = disable-structure shown="Enabled" {
          disable-tunnel: "Inject Valve B" -> [w1448 w1468]
          frame Disabled {
            n899 = local read "Pump write delay (ms)"() -> (w1450:dbl)
            n900 = flat-sequence {
              tunnel: w1449 -> [w1463]
              tunnel: w1450 -> [w1459]
              tunnel: w1448 -> [_]
              tunnel: w1450 -> [w1465]
              tunnel: w1449 -> [w1466]
              frame #0 {
                n901 = local read "All Pump Parameters"() -> (w1458:T5)
                n902 = Multiply(x=60.0, y="Flush Center Ch Rate (ul/m)") -> (x*y=w1455:dbl)
                n903 = Unbundle By Name(w1458) -> ("Pump 2"=w1464:T32)
                n904 = call "Set pump parameters.vi"("Pump write delay (ms)"=w1459, "Volume (uL)"="Flush Center Ch Volume (uL)", "Rate (uL/h)"=w1455, "Units"=3.0, "Pump #"=2.0, "Pump Parameters In"=w1464, "VISA resource name"=w1463) -> ("Pump Parameters Out"=w1457:T32)  [unwired: 3 in]
                n905 = Bundle By Name(cluster=w1458, "Pump 2"=w1457) -> (w1456:T5)
                n906 = local write "All Pump Parameters"(w1456) -> ()
                n907 = Add(x="Flush Center Ch Volume (uL)", y="Total Volume\nFlushed (uL)") -> (x+y=w1452:dbl)
                n908 = local write "Total Volume\nFlushed (uL)"(w1452) -> ()
              }
              frame #1 {
                n909 = Wait (ms)(milliseconds to wait=w1465) -> ()  [unwired: 1 out]
              }
              frame #2 {
                n910 = call "Write to pump.vi"("string"="start", "VISA resource name"=w1466) -> ()  [unwired: 1 out]
              }
            }
            n911 = local read "Chemyx Syringe Pump Serial Port"() -> (w1449:refnum<visa-resource-name>)
          }
          frame Enabled {
            n912 = call "hamilton_controller.vi"("Open?"=w1468, "valve"=enum16{"A", "B", "C", "D", "ALL"}."B", "action"=T20."MOVE VALVE") -> ()  [unwired: 8 in, 1 out]
          }
        }
      }
      event "Sample Channel Flow": Value Change {
        n913 = event-data() -> ()  [unwired: 7 out]
        n914 = call "hamilton_controller.vi"("Open?"="Sample Channel Flow", "valve"=enum16{"A", "B", "C", "D", "ALL"}."C", "action"=T20."MOVE VALVE") -> ()  [unwired: 8 in, 1 out]
      }
      event "Flip Green Filter": Value Change {
        n915 = event-data() -> ()  [unwired: 7 out]
        n916 = local write "Flip Green Filter"("Flip Green Filter") -> ()
        n917 = flat-sequence {
          tunnel: w1481 -> [w1486]
          tunnel: w1480 -> [w1485]
          tunnel: [w1483] -> w1478
          tunnel: [w1482] -> w1477
          tunnel: [w1488] -> w1476
          tunnel: w1478 -> [w1488]
          tunnel: [w1487] -> w1475
          tunnel: w1477 -> [w1487]
          tunnel: w1476 -> [w1492]
          tunnel: w1475 -> [w1491]
          tunnel: [w1490] -> w1479
          frame #0 {
            n918 = xnode "Read/Write Control"("FPGA VI Reference In"=w1486, "error in"=w1485, "Green Filter Flipper"=TRUE) -> ("FPGA VI Reference Out"=w1483:T19, "error out"=w1482:errorcluster)
          }
          frame #1 {
            n919 = Wait (ms)(milliseconds to wait=u32 100) -> ()  [unwired: 1 out]
          }
          frame #2 {
            n920 = xnode "Read/Write Control"("FPGA VI Reference In"=w1492, "error in"=w1491, "Green Filter Flipper"=FALSE) -> ("error out"=w1490:errorcluster)  [unwired: 1 out]
          }
        }
      }
      event "Pump 1 contents", "Pump 3 contents": Value Change {
        n921 = event-data() -> ()  [unwired: 7 out]
        n922 = local read "Pump 1 contents"() -> (→"Pump 1 cont disp":string)
        n923 = local read "Pump 3 contents"() -> (→"Pump 3 cont disp":string)
      }
      event "Reset Trap Pos. FB": Value Change {
        n924 = event-data() -> ()  [unwired: 7 out]
        n925 = xnode "Read/Write Control"("FPGA VI Reference In"=w1498, "error in"=w1497, "Trap Pos. FB Reset"="Reset Trap Pos. FB") -> ()  [unwired: 2 out]
      }
      event "Trap Pos. FB ON": Value Change {
        n926 = event-data() -> ()  [unwired: 7 out]
        n927 = xnode "Read/Write Control"("FPGA VI Reference In"=w1501, "error in"=w1500, "Force feedback"="Trap Pos. FB ON") -> ()  [unwired: 2 out]
      }
      event "Trap Pos. FB Range", "Trap Pos. FB Gains", "Trap Pos. FB Mult Factor", "Trap Pos. FB Offset Factor", "Trap Pos FB Negate Action", "Trap Pos FB Monitor\nT1 or T2": Value Change {
        n928 = event-data() -> ()  [unwired: 7 out]
        n929 = xnode "Read/Write Control"("FPGA VI Reference In"=w1510, "error in"=w1509, "Trap Pos. FB Range"="Trap Pos. FB Range", "Trap Pos. FB Gains"="Trap Pos. FB Gains", "Trap Pos. FB Mult Factor"="Trap Pos. FB Mult Factor", "Trap Pos. FB Offset Factor"="Trap Pos. FB Offset Factor", "Trap Pos FB Negate Action"="Trap Pos FB Negate Action", "Trap Pos FB Monitor T1 or T2"="Trap Pos FB Monitor\nT1 or T2", "AI1 X Scale"="Trap Pos. AI1 X Pre-scale") -> ()  [unwired: 2 out]
      }
      event "Trap Pos FB SP": Value Change {
        n930 = event-data() -> ()  [unwired: 7 out]
        n931 = xnode "Read/Write Control"("FPGA VI Reference In"=w1513, "error in"=w1512, "Trap Pos. FB SP"="Trap Pos FB SP") -> ()  [unwired: 2 out]
      }
      event "Set SP to Reading": Value Change {
        n932 = event-data() -> ()  [unwired: 7 out]
        n933 = local read "Trap Pos FB Monitor\nT1 or T2"() -> (w1521:bool)
        n934 = local read "Trap X AI1 (DMA)"() -> (w1524:T13)
        n935 = local read "Trap X (AI1)"() -> (w1527:T10)
        n936 = Unbundle By Name(w1527) -> ("Trap 1"=w1526:fxp<+/-,16,1>, "Trap 2"=w1525:fxp<+/-,16,1>)
        n937 = Unbundle By Name(w1524) -> ("Set 1"=w1523:fxp<+/-,16,1>, "Set 2"=w1522:fxp<+/-,16,1>)
        n938 = Select(t=w1526, s=w1521, f=w1525) -> (s? t:f=w1520:fxp<+/-,16,1>)
        n939 = Select(t=w1523, s=w1521, f=w1522) -> (s? t:f=w1519:fxp<+/-,16,1>)
        n940 = Not(x="Set SP Using...") -> (.not. x?=w1514:bool)
        n941 = Select(t=w1520, s=w1514, f=w1519) -> (s? t:f=w1515:fxp<+/-,16,1>)
        n942 = xnode "Read/Write Control"("FPGA VI Reference In"=w1517, "error in"=w1516, "Trap Pos. FB SP"=w1515) -> ()  [unwired: 2 out]
        n943 = local write "Trap Pos FB SP"(w1515) -> ()
      }
      event "Trap Pos. FB Out Scale 2^n": Value Change {
        n944 = event-data() -> ()  [unwired: 7 out]
        n945 = Scale By Power Of 2(n="Trap Pos. FB Out Scale 2^n", x=ext 1.0) -> (x*2^n=w1529:ext)
        n946 = property on="Trap Pos. FB Mult Factor" class="DigNum (strict)"("Val(Sgnl)"=w1529) -> ()  [unwired: 2 in, 2 out]
      }
      event "Trap Pos FB Int Count": Value Change {
        n947 = event-data() -> ()  [unwired: 7 out]
        n948 = xnode "Read/Write Control"("FPGA VI Reference In"=w1534, "error in"=w1533, "Trap Pos FB Int Count"="Trap Pos FB Int Count") -> ()  [unwired: 2 out]
      }
    }
    "error out 2" <- w715
    n949 = node-c288() -> ()  [unwired: 1 in, 1 out]
  }
  n950 = timed-loop "Run Scripts, including: stage motion" {
    timing: w69 -> [_]
    timing-out: [_] -> w68
    tunnel: w24 -> [_]
    stop <- w1536 stop-if-true
    n951 = node-c288() -> ()  [unwired: 1 in, 1 out]
    n952 = event shown="[1] Timeout" {
      selector: _ -> [_ _ _ _ _ _ _ _ _ _ _ _]
      dyn-events: _ -> [_ _ _ _ _ _ _ _ _ _ _ _]
      timeout: 50 -> [_ _ _ _ _ _ _ _ _ _ _ _]
      tunnel: ["Move Cap. 1 (DNA Top)" _ "Cal/Data Acq. Spot" "Dump Beads" "Dip for Protein" _ "Got ADig bead" "Got DNA bead" "Take Stepping Data" _ "Take Detection Laser\nImage" _] -> _
      tunnel: [_ _ _ _ _ _ _ _ _ _ _ w1744] -> w1536
      event "Move Cap. 1 (DNA Top)": Value Change {
        n953 = event-data() -> ()  [unwired: 1 in, 5 out]
        n954 = local write "Move Cap. 1 (DNA Top)"(FALSE ("Move Cap. 1 (DNA Right)")) -> ()
        n955 = flat-sequence {
          tunnel: "Cap 1 Samp Flow ON" -> [w1542]
          frame #0 {
            n956 = local write "Stage Moving"(FALSE ("Stage Moving")) -> ()
            n957 = case "stop flow" shown="True" w1542 {
              frame False {
              }
              frame True {
                n958 = call "hamilton_controller.vi"("Open?"=FALSE, "valve"=enum16{"A", "B", "C", "D", "ALL"}."C", "action"=T20."MOVE VALVE") -> ()  [unwired: 8 in, 1 out]
              }
            }
            n959 = case shown="True" TRUE {
              tunnel: "Cap 1 T ON" -> [w1551 w1552]
              frame False {
                n960 = property on="Trap 1 (ON/OFF)" class="Bool (strict)"("Val(Sgnl)"=w1551) -> ()  [unwired: 2 in, 2 out]
              }
              frame True {
                n961 = property on="Trap 2 (ON/OFF)" class="Bool (strict)"("Val(Sgnl)"=w1552) -> ()  [unwired: 2 in, 2 out]
              }
            }
            n962 = call <vilib>:"Beep.vi"() -> ()  [unwired: 3 in, 9 out]
            n963 = case shown="True" "Cap 1 Flow ON" {
              frame False {
              }
              frame True {
                n964 = property on="Inject Top" class="Bool (strict)"("Val(Sgnl)"=TRUE ("Value (Signaling)")) -> ()  [unwired: 2 in, 2 out]
              }
            }
          }
        }
      }
      event Timeout {
        n965 = event-data() -> ()  [unwired: 1 in, 2 out]
      }
      event "Cal/Data Acq. Spot": Value Change {
        # "wait for calibration file\nto be written"
        # "signal save cal true\nthis tells the data \nacquisition loop to\nstart sending the data\nto a calibration file"
        # "separate traps to\nthe desired trap delta"
        # "move stage to data acquisition spot"
        # "CHANGE FISH FOR TETHER BACK\nTO TRUE VALUE HERE."
        n966 = event-data() -> ()  [unwired: 1 in, 5 out]
        n967 = local write "Cal/Data Acq. Spot"(FALSE ("Cal/Data Acq. Spot")) -> ()
        n968 = flat-sequence {
          tunnel: ["Cal @ (MHz)"] -> w1553
          tunnel: w1553 -> [w1563]
          tunnel: w1553 -> [w1584]
          frame #0 {
            n969 = property on="Trap Delta (MHz)" class="DigNum (strict)"("Val(Sgnl)"="Cal @ (MHz)") -> ()  [unwired: 2 in, 2 out]
            n970 = call <vilib>:"Beep.vi"() -> ()  [unwired: 3 in, 9 out]
          }
          frame #1 {
            n971 = Wait (ms)(milliseconds to wait=u32 100) -> ()  [unwired: 1 out]
          }
          frame #2 {
            n972 = property on="Save Calibration" class="Bool (strict)"("Val(Sgnl)"=TRUE ("Value (Signaling)")) -> ()  [unwired: 2 in, 2 out]
          }
          frame #3 {
            n973 = Wait (ms)(milliseconds to wait=u32 4000) -> ()  [unwired: 1 out]
          }
          frame #4 {
            n974 = while {
              stop <- w1560 stop-if-true
              n975 = local read "Saving..."() -> (w1561:bool)
              n976 = Wait (ms)(milliseconds to wait=u32 100) -> ()  [unwired: 1 out]
              n977 = Not(x=w1561) -> (.not. x?=w1560:bool)
            }
          }
          frame #5 {
            n978 = case shown="True" "W/ Offset 1" {
              tunnel: w1563 -> [_ w1565]
              frame False {
              }
              frame True {
                n979 = stacked-sequence {
                  tunnel: w1565 -> [_ _ _ _ _ _ _ w1582]
                  frame #0 {
                    n980 = Replace Array Subset(array=u32[] [0] ("Index Values"), new element="Offset 1 Set", index=0) -> (w1566:u32[])
                    n981 = property on="Saved AOD Raster Scan Parameter Sets" class="Arr (strict)"("Index Values"=w1566) -> ()  [unwired: 2 in, 2 out]
                    n982 = property on="Trap Delta (MHz)" class="DigNum (strict)"("Val(Sgnl)"="Offset 1 Start (MHz)") -> ()  [unwired: 2 in, 2 out]
                  }
                  frame #1 {
                    n983 = Wait (ms)(milliseconds to wait=u32 200) -> ()  [unwired: 1 out]
                  }
                  frame #2 {
                    n984 = property on="Load parameters" class="Bool (strict)"("Val(Sgnl)"=TRUE ("Value (Signaling)")) -> ()  [unwired: 2 in, 2 out]
                  }
                  frame #3 {
                    n985 = Wait (ms)(milliseconds to wait=u32 200) -> ()  [unwired: 1 out]
                  }
                  frame #4 {
                    n986 = property on="Trap Raster Scan" class="Bool (strict)"("Val(Sgnl)"=TRUE ("Value (Signaling)")) -> ()  [unwired: 2 in, 2 out]
                  }
                  frame #5 {
                    n987 = Wait (ms)(milliseconds to wait=u32 2000) -> ()  [unwired: 1 out]
                  }
                  frame #6 {
                    n988 = while {
                      stop <- w1579 stop-if-true
                      n989 = local read "Raster Scanning..."() -> (w1581:bool)
                      n990 = local read "Saving..."() -> (w1577:bool)
                      n991 = Wait (ms)(milliseconds to wait=u32 100) -> ()  [unwired: 1 out]
                      n992 = Not(x=w1577) -> (.not. x?=w1576:bool)
                      n993 = Not(x=w1581) -> (.not. x?=w1578:bool)
                      n994 = And(x=w1578, y=w1576) -> (x .and. y?=w1579:bool)
                    }
                  }
                  frame #7 {
                    n995 = property on="Trap Delta (MHz)" class="DigNum (strict)"("Val(Sgnl)"=w1582) -> ()  [unwired: 2 in, 2 out]
                  }
                }
              }
            }
          }
          frame #6 {
            n996 = local read "Save ave N"() -> (w1583:dbl)
            n997 = case shown="True" "W/ Offset 2" {
              tunnel: w1584 -> [_ w1590]
              tunnel: w1583 -> [_ w1589]
              frame False {
                n998 = Multiply(x="Cal read wait (s)", y=u32 1000 ("milliseconds to wait")) -> (x*y=w1587:u32)
                n999 = Wait (ms)(milliseconds to wait=w1587) -> ()  [unwired: 1 out]
              }
              frame True {
                n1000 = stacked-sequence {
                  tunnel: w1590 -> [_ _ _ _ _ _ _ _ _ w1611 _ _]
                  tunnel: w1589 -> [_ _ _ _ _ _ _ _ _ w1609 _ _]
                  frame #0 {
                    n1001 = property on="Save ave N" class="DigNum (strict)"("Val(Sgnl)"=1.0 ("Value (Signaling)")) -> ()  [unwired: 2 in, 2 out]
                  }
                  frame #1 {
                    n1002 = Wait (ms)(milliseconds to wait=u32 500) -> ()  [unwired: 1 out]
                  }
                  frame #2 {
                    n1003 = property on="Trap Delta (MHz)" class="DigNum (strict)"("Val(Sgnl)"="Offset 2 Start (MHz)") -> ()  [unwired: 2 in, 2 out]
                    n1004 = Replace Array Subset(array=u32[] [0] ("Index Values"), new element="Offset 2 Set", index=0) -> (w1595:u32[])
                    n1005 = property on="Saved AOD Raster Scan Parameter Sets" class="Arr (strict)"("Index Values"=w1595) -> ()  [unwired: 2 in, 2 out]
                  }
                  frame #3 {
                    n1006 = Wait (ms)(milliseconds to wait=u32 500) -> ()  [unwired: 1 out]
                  }
                  frame #4 {
                    n1007 = property on="Load parameters" class="Bool (strict)"("Val(Sgnl)"=TRUE ("Value (Signaling)")) -> ()  [unwired: 2 in, 2 out]
                  }
                  frame #5 {
                    n1008 = Wait (ms)(milliseconds to wait=u32 500) -> ()  [unwired: 1 out]
                  }
                  frame #6 {
                    n1009 = property on="Trap Raster Scan" class="Bool (strict)"("Val(Sgnl)"=TRUE ("Value (Signaling)")) -> ()  [unwired: 2 in, 2 out]
                  }
                  frame #7 {
                    n1010 = Wait (ms)(milliseconds to wait=u32 2000) -> ()  [unwired: 1 out]
                  }
                  frame #8 {
                    n1011 = while {
                      stop <- w1604 stop-if-true
                      n1012 = local read "Raster Scanning..."() -> (w1607:bool)
                      n1013 = local read "Saving..."() -> (w1605:bool)
                      n1014 = Wait (ms)(milliseconds to wait=u32 100) -> ()  [unwired: 1 out]
                      n1015 = Not(x=w1605) -> (.not. x?=w1603:bool)
                      n1016 = Not(x=w1607) -> (.not. x?=w1606:bool)
                      n1017 = And(x=w1606, y=w1603) -> (x .and. y?=w1604:bool)
                    }
                  }
                  frame #9 {
                    n1018 = property on="Trap Delta (MHz)" class="DigNum (strict)"("Val(Sgnl)"=w1611) -> ()  [unwired: 2 in, 2 out]
                    n1019 = property on="Saved AOD Raster Scan Parameter Sets" class="Arr (strict)"("Index Values"=u32[] [0]) -> ()  [unwired: 2 in, 2 out]
                    n1020 = property on="Save ave N" class="DigNum (strict)"("Val(Sgnl)"=w1609) -> ()  [unwired: 2 in, 2 out]
                  }
                  frame #10 {
                    n1021 = Wait (ms)(milliseconds to wait=u32 500) -> ()  [unwired: 1 out]
                  }
                  frame #11 {
                    n1022 = property on="Load parameters" class="Bool (strict)"("Val(Sgnl)"=TRUE ("Value (Signaling)")) -> ()  [unwired: 2 in, 2 out]
                  }
                }
              }
            }
          }
          frame #7 {
            n1023 = property on="Read Cal" class="Bool (strict)"("Val(Sgnl)"=TRUE ("Value (Signaling)")) -> ()  [unwired: 2 in, 2 out]
          }
          frame #8 {
            n1024 = Wait (ms)(milliseconds to wait=u32 500) -> ()  [unwired: 1 out]
          }
          frame #9 {
            n1025 = property on="Fish for Tether" class="Bool (strict)"("Val(Sgnl)"=FALSE ("Value (Signaling)")) -> ()  [unwired: 2 in, 2 out]
          }
        }
      }
      event "Dump Beads": Value Change {
        # "SCRIPT TO REMOVE BOTH BEADS FROM THE TRAPS. TURNS ON LIGHT WHICH INDICATES THAT STAGE IS MOVING. THEN STOPS SAVING DATA. \nSETS Sample Channel Flow TO TRUE. STOPS INTERLACING GREEN FLUORESCENCE. TURNS OFF Tether INDICATOR BECAUSE WE ARE THROWING IT\nAWAY. SHUTS OFF TRAP POSITION FEEDBACK."
        n1026 = event-data() -> ()  [unwired: 1 in, 5 out]
        n1027 = flat-sequence {
          frame #0 {
            w1618 = FALSE ("Fl. Triggered...")
            w1619 = TRUE ("Stage Moving")
            n1028 = local read "Saving..."() -> (w1620:bool)
            n1029 = local write "Fl. Triggered..."(w1618) -> ()
            n1030 = local write "Stage Moving"(w1619) -> ()
            n1031 = local write "Tether"(w1618) -> ()
            n1032 = property on="Green Laser ON/Interlacing" class="Bool (strict)"("Val(Sgnl)"=w1618) -> ()  [unwired: 2 in, 2 out]
            n1033 = property on="Trap Pos. FB ON" class="Bool (strict)"("Val(Sgnl)"=w1618) -> ()  [unwired: 2 in, 2 out]
            n1034 = property on="Sample Channel Flow" class="Bool (strict)"("Val(Sgnl)"=w1619) -> ()  [unwired: 2 in, 2 out]
            n1035 = local write "Stop Saving"(w1620) -> ()
          }
          frame #1 {
            w1621 = FALSE ("Value (Signaling)")
            # "TURNS TRAPS OFF SO THAT\nBEADS REMAIN AT DUMP \nBEADS POSITION"
            n1036 = property on="Trap 1 (ON/OFF)" class="Bool (strict)"("Val(Sgnl)"=w1621) -> ()  [unwired: 2 in, 2 out]
            n1037 = property on="Trap 2 (ON/OFF)" class="Bool (strict)"("Val(Sgnl)"=w1621) -> ()  [unwired: 2 in, 2 out]
            n1038 = call <vilib>:"Beep.vi"() -> ()  [unwired: 3 in, 9 out]
          }
          frame #2 {
            n1039 = property on="Goto Bottom (F7)" class="Bool (strict)"("Val(Sgnl)"=TRUE ("Value (Signaling)")) -> ()  [unwired: 2 in, 2 out]
          }
          frame #3 {
            n1040 = Wait (ms)(milliseconds to wait=u32 8000) -> ()  [unwired: 1 out]
          }
          frame #4 {
            n1041 = property on="Trap Delta (MHz)" class="DigNum (strict)"("Val(Sgnl)"=20.0 ("Value (Signaling)")) -> ()  [unwired: 2 in, 2 out]
          }
          frame #5 {
            n1042 = property on="Trap 2 (ON/OFF)" class="Bool (strict)"("Val(Sgnl)"=TRUE ("Value (Signaling)")) -> ()  [unwired: 2 in, 2 out]
          }
          frame #6 {
            n1043 = property on="Sample Channel Flow" class="Bool (strict)"("Val(Sgnl)"=FALSE ("Value (Signaling)")) -> ()  [unwired: 2 in, 2 out]
          }
        }
      }
      event "Dip for Protein": Value Change {
        n1044 = event-data() -> ()  [unwired: 1 in, 5 out]
        n1045 = flat-sequence {
          frame #0 {
            n1046 = case shown="True" "Move Trap Before?" {
              frame False {
              }
              frame True {
                n1047 = property on="Trap Delta (MHz)" class="DigNum (strict)"("Val(Sgnl)"="Dip Trap Delta 1 (MHz)") -> ()  [unwired: 2 in, 2 out]
              }
            }
          }
          frame #1 {
            n1048 = Multiply(x="Duration (s)", y=1000.0) -> (x*y=w1630:dbl)
            n1049 = Wait (ms)(milliseconds to wait=w1630) -> ()  [unwired: 1 out]
          }
          frame #2 {
            n1050 = case shown="True" "Move Trap After?" {
              frame False {
              }
              frame True {
                n1051 = property on="Trap Delta (MHz)" class="DigNum (strict)"("Val(Sgnl)"="Dip Trap Delta 2 (MHz)") -> ()  [unwired: 2 in, 2 out]
              }
            }
          }
          frame #3 {
            n1052 = case shown="True" "Green ON After?" {
              frame False {
              }
              frame True {
                n1053 = property on="Green Laser ON/Interlacing" class="Bool (strict)"("Val(Sgnl)"=TRUE ("Value (Signaling)")) -> ()  [unwired: 2 in, 2 out]
              }
            }
          }
          frame #4 {
            n1054 = Wait (ms)(milliseconds to wait=u32 500) -> ()  [unwired: 1 out]
          }
          frame #5 {
            n1055 = case shown="True" "Save Data After?" {
              frame False {
              }
              frame True {
                n1056 = property on="Start Saving" class="Bool (strict)"("Val(Sgnl)"=TRUE ("Value (Signaling)")) -> ()  [unwired: 2 in, 2 out]
              }
            }
          }
        }
      }
      event "Profile": Value Change {
        n1057 = event-data() -> ()  [unwired: 1 in, 5 out]
        n1058 = flat-sequence {
          frame #0 {
            w1640 = 0.0 ("element")
            n1059 = Build Array(w1640, "Y change (mm)", w1640) -> ()  [unwired: 1 out]
          }
          frame #1 {
            # "stop saving"
            n1060 = local write "Stop Saving"(TRUE ("Stop Saving")) -> ()
            n1061 = local write "Stage Moving"(FALSE ("Stage Moving")) -> ()
          }
        }
      }
      event "Got ADig bead": Value Change {
        n1062 = event-data() -> ()  [unwired: 1 in, 5 out]
        n1063 = property on="Move Cap. 1 (DNA Top)" class="Bool (strict)"("Val(Sgnl)"=TRUE ("Value (Signaling)")) -> ()  [unwired: 2 in, 2 out]
        n1064 = property on="Inject Bottom" class="Bool (strict)"("Val(Sgnl)"=FALSE ("Value (Signaling)")) -> ()  [unwired: 2 in, 2 out]
      }
      event "Got DNA bead": Value Change {
        n1065 = event-data() -> ()  [unwired: 1 in, 5 out]
        n1066 = property on="Cal/Data Acq. Spot" class="Bool (strict)"("Val(Sgnl)"=TRUE ("Value (Signaling)")) -> ()  [unwired: 2 in, 2 out]
        n1067 = property on="Inject Top" class="Bool (strict)"("Val(Sgnl)"=FALSE ("Value (Signaling)")) -> ()  [unwired: 2 in, 2 out]
      }
      event "Take Stepping Data": Value Change {
        n1068 = event-data() -> ()  [unwired: 1 in, 5 out]
        n1069 = local read "Save ave N"() -> (w1658:dbl)
        n1070 = flat-sequence {
          tunnel: w1658 -> [w1660]
          tunnel: [w1660] -> w1653
          tunnel: [w1662] -> w1654
          tunnel: w1653 -> [w1662]
          tunnel: [w1664] -> w1655
          tunnel: w1654 -> [w1664]
          tunnel: [w1667] -> w1656
          tunnel: w1655 -> [w1667]
          tunnel: [w1669] -> w1657
          tunnel: w1656 -> [w1669]
          tunnel: [w1671] -> w1651
          tunnel: w1657 -> [w1671]
          tunnel: w1651 -> [w1674]
          tunnel: [w1674] -> w1650
          tunnel: w1650 -> [w1675]
          tunnel: [w1675] -> w1652
          tunnel: w1652 -> [w1681]
          frame #0 {
            n1071 = property on="Save ave N" class="DigNum (strict)"("Val(Sgnl)"="Save ave factor") -> ()  [unwired: 2 in, 2 out]
          }
          frame #1 {
            n1072 = Wait (ms)(milliseconds to wait=u32 100) -> ()  [unwired: 1 out]
          }
          frame #2 {
            n1073 = local read "Offset 2 Start (MHz)"() -> (w1666:dbl)
            n1074 = property on="Saved AOD Raster Scan Parameter Sets" class="Arr (strict)"("Index Values"=u32[] [2]) -> ()  [unwired: 2 in, 2 out]
            n1075 = property on="Trap Delta (MHz)" class="DigNum (strict)"("Val(Sgnl)"=w1666) -> ()  [unwired: 2 in, 2 out]
          }
          frame #3 {
            n1076 = property on="Load parameters" class="Bool (strict)"("Val(Sgnl)"=TRUE ("Value (Signaling)")) -> ()  [unwired: 2 in, 2 out]
          }
          frame #4 {
            n1077 = Wait (ms)(milliseconds to wait=u32 100) -> ()  [unwired: 1 out]
          }
          frame #5 {
            n1078 = property on="Trap Raster Scan" class="Bool (strict)"("Val(Sgnl)"=TRUE ("Value (Signaling)")) -> ()  [unwired: 2 in, 2 out]
          }
          frame #6 {
            n1079 = Wait (ms)(milliseconds to wait=u32 1000) -> ()  [unwired: 1 out]
          }
          frame #7 {
            n1080 = while {
              stop <- w1678 stop-if-true
              n1081 = local read "Raster Scanning..."() -> (w1680:bool)
              n1082 = local read "Saving..."() -> (w1679:bool)
              n1083 = Not(x=w1679) -> (.not. x?=w1676:bool)
              n1084 = Not(x=w1680) -> (.not. x?=w1677:bool)
              n1085 = And(x=w1677, y=w1676) -> (x .and. y?=w1678:bool)
            }
          }
          frame #8 {
            n1086 = property on="Save ave N" class="DigNum (strict)"("Val(Sgnl)"=w1681) -> ()  [unwired: 2 in, 2 out]
          }
        }
      }
      event "Step Size (nm)": Value Change {
        n1087 = event-data() -> ()  [unwired: 1 in, 5 out]
        n1088 = flat-sequence {
          frame #0 {
            n1089 = property on="Saved AOD Raster Scan Parameter Sets" class="Arr (strict)"("Index Values"=u32[] [1]) -> ()  [unwired: 2 in, 2 out]
          }
          frame #1 {
            n1090 = Multiply(x="N Steps", y="Step Size (nm)") -> (x*y=w1683:dbl)
            n1091 = property on="Scan Speed AOD (nm/s) 2" class="DigNum (strict)"("Value"="Step Size (nm)") -> ()  [unwired: 2 in, 2 out]
            n1092 = property on="Step Size AOD (nm) 2" class="DigNum (strict)"("Value"="Step Size (nm)") -> ()  [unwired: 2 in, 2 out]
            n1093 = property on="Scan Range AOD (nm) 2" class="DigNum (strict)"("Value"=w1683) -> ()  [unwired: 2 in, 2 out]
          }
        }
      }
      event "Take Detection Laser\nImage": Value Change {
        n1094 = event-data() -> ()  [unwired: 1 in, 5 out]
        n1095 = flat-sequence {
          tunnel: [w1711] -> w1701
          tunnel: [w1710] -> w1694
          tunnel: [w1709] -> w1686
          tunnel: [w1714] -> w1702
          tunnel: w1701 -> [w1714]
          tunnel: [w1713] -> w1695
          tunnel: w1694 -> [w1713]
          tunnel: [w1712] -> w1687
          tunnel: w1686 -> [w1712]
          tunnel: [w1718] -> w1703
          tunnel: w1702 -> [w1718]
          tunnel: [w1717] -> w1696
          tunnel: w1695 -> [w1717]
          tunnel: [w1716] -> w1688
          tunnel: w1687 -> [w1716]
          tunnel: [w1724] -> w1704
          tunnel: w1703 -> [w1724]
          tunnel: [w1723] -> w1697
          tunnel: w1696 -> [w1723]
          tunnel: [w1722] -> w1689
          tunnel: w1688 -> [w1722]
          tunnel: [w1728] -> w1705
          tunnel: w1704 -> [w1728]
          tunnel: [w1727] -> w1698
          tunnel: w1697 -> [w1727]
          tunnel: [w1726] -> w1690
          tunnel: w1689 -> [w1726]
          tunnel: [w1732] -> w1706
          tunnel: w1705 -> [w1732]
          tunnel: [w1731] -> w1699
          tunnel: w1698 -> [w1731]
          tunnel: [w1730] -> w1691
          tunnel: w1690 -> [w1730]
          tunnel: [w1736] -> w1707
          tunnel: w1706 -> [w1736]
          tunnel: [w1735] -> w1700
          tunnel: w1699 -> [w1735]
          tunnel: [w1734] -> w1692
          tunnel: w1691 -> [w1734]
          tunnel: w1707 -> [w1742]
          tunnel: w1700 -> [w1741]
          tunnel: [w1739] -> w1693
          tunnel: w1692 -> [w1739]
          tunnel: w1693 -> [w1743]
          frame #0 {
            n1096 = local read "Green Laser ON/Interlacing"() -> (w1711:bool)
            n1097 = local read "Green laser mode"() -> (w1710:enum32{"Laser ON", "Laser OFF", "Interlace"})
            n1098 = local read "Green FB On/Off"() -> (w1709:bool)
          }
          frame #1 {
            n1099 = property on="Green FB On/Off" class="Bool (strict)"("Val(Sgnl)"=FALSE ("Value (Signaling)")) -> ()  [unwired: 2 in, 2 out]
          }
          frame #2 {
            n1100 = property on="Green Laser ON/Interlacing" class="Bool (strict)"("Val(Sgnl)"=TRUE ("Value (Signaling)")) -> ()  [unwired: 2 in, 2 out]
            n1101 = property on="Flip Green Filter" class="Bool (strict)"("Val(Sgnl)"=TRUE ("Value (Signaling)")) -> ()  [unwired: 2 in, 2 out]
            n1102 = property on="Green laser mode" class="RadioBtnsControl (strict)"("Val(Sgnl)"=enum32{"Laser ON", "Laser OFF", "Interlace"}."Laser ON" ("Value (Signaling)")) -> ()  [unwired: 2 in, 2 out]
          }
          frame #3 {
            n1103 = Wait (ms)(milliseconds to wait=u32 500) -> ()  [unwired: 1 out]
          }
          frame #4 {
            n1104 = property on="Confocal Image" class="Bool (strict)"("Val(Sgnl)"=TRUE ("Value (Signaling)")) -> ()  [unwired: 2 in, 2 out]
          }
          frame #5 {
            n1105 = Wait (ms)(milliseconds to wait=u32 2000) -> ()  [unwired: 1 out]
          }
          frame #6 {
            n1106 = while {
              stop <- w1737 stop-if-true
              n1107 = local read "Saving..."() -> (w1738:bool)
              n1108 = Not(x=w1738) -> (.not. x?=w1737:bool)
            }
          }
          frame #7 {
            n1109 = property on="Flip Green Filter" class="Bool (strict)"("Val(Sgnl)"=TRUE ("Value (Signaling)")) -> ()  [unwired: 2 in, 2 out]
            n1110 = property on="Green Laser ON/Interlacing" class="Bool (strict)"("Val(Sgnl)"=w1742) -> ()  [unwired: 2 in, 2 out]
            n1111 = property on="Green laser mode" class="RadioBtnsControl (strict)"("Val(Sgnl)"=w1741) -> ()  [unwired: 2 in, 2 out]
          }
          frame #8 {
            n1112 = property on="Green FB On/Off" class="Bool (strict)"("Val(Sgnl)"=w1743) -> ()  [unwired: 2 in, 2 out]
          }
        }
      }
      event "Stop All": Value Change {
        n1113 = event-data() -> ()  [unwired: 1 in, 5 out]
        n1114 = local read "Stop All"() -> (w1744:bool)
      }
    }
    n1115 = node-c288() -> ()  [unwired: 1 in, 1 out]
  }
  n1116 = node-c288() -> (w76:T24)  [unwired: 4 out]
  n1117 = timed-loop "Mouse control: trap position (AOM deflection), set confocal spot from image" {
    tunnel: [w1746] -> w34
    tunnel: w24 -> [w1745]
    timing: w76 -> [_]
    timing-out: [_] -> w75
    stop <- w1746 stop-if-true
    n1118 = node-c288() -> ()  [unwired: 2 out]
    n1119 = event shown="[1] \"Pane\": Mouse Move" {
      selector: _ -> [_ _]
      dyn-events: _ -> [_ _]
      timeout: _ -> [_ _]
      tunnel: w1745 -> [w1749 _]
      event Mouse Down {
        n1120 = event-data() -> ("Time"=w1751:u32, "Coords"=w1750:T7, "Button"=w1752:u16)  [unwired: 6 out]
        n1121 = case shown="1" w1752 {
          tunnel: w1751 -> [_ _ w1855]
          tunnel: w1750 -> [_ w1789 w1853]
          tunnel: w1749 -> [_ _ w1851]
          frame 0, Default {
          }
          frame 1 {
            n1122 = property on="APD 2" class="ImageControl"() -> ("Displayed Image Position"=w1759:cluster{"Left":i32, "Top":i32})  [unwired: 2 in, 2 out]
            n1123 = property on="APD 1" class="ImageControl"() -> ("Displayed Image Position"=w1788:cluster{"Left":i32, "Top":i32})  [unwired: 2 in, 2 out]
            n1124 = property on="Detection Laser X" class="ImageControl"() -> ("Displayed Image Position"=w1785:cluster{"Left":i32, "Top":i32})  [unwired: 2 in, 2 out]
            n1125 = property on="Detection Laser Y" class="ImageControl"() -> ("Displayed Image Position"=w1784:cluster{"Left":i32, "Top":i32})  [unwired: 2 in, 2 out]
            n1126 = property on="APD 2" class="ImageControl"() -> ("Displayed Image Size"=w1758:cluster{"Width":u32, "Height":u32})  [unwired: 2 in, 2 out]
            n1127 = property on="APD 1" class="ImageControl"() -> ("Displayed Image Size"=w1786:cluster{"Width":u32, "Height":u32})  [unwired: 2 in, 2 out]
            n1128 = property on="Detection Laser X" class="ImageControl"() -> ("Displayed Image Size"=w1787:cluster{"Width":u32, "Height":u32})  [unwired: 2 in, 2 out]
            n1129 = property on="Detection Laser Y" class="ImageControl"() -> ("Displayed Image Size"=w1783:cluster{"Width":u32, "Height":u32})  [unwired: 2 in, 2 out]
            n1130 = Unbundle By Name(w1758) -> ("Width"=w1755:u32, "Height"=w1754:u32)
            n1131 = Unbundle By Name(w1759) -> ("Left"=w1757:i32, "Top"=w1756:i32)
            n1132 = Unbundle By Name(w1786) -> ("Width"=w1780:u32, "Height"=w1779:u32)
            n1133 = Unbundle By Name(w1787) -> ("Width"=w1776:u32, "Height"=w1775:u32)
            n1134 = Unbundle By Name(w1783) -> ("Width"=w1772:u32, "Height"=w1771:u32)
            n1135 = Unbundle By Name(w1788) -> ("Left"=w1782:i32, "Top"=w1781:i32)
            n1136 = Unbundle By Name(w1785) -> ("Left"=w1778:i32, "Top"=w1777:i32)
            n1137 = Unbundle By Name(w1784) -> ("Left"=w1774:i32, "Top"=w1773:i32)
            n1138 = Bundle("Left"=w1757, "Top"=w1756, "Width"=w1755, "Height"=w1754) -> (w1753:T33)  [unwired: 1 in]
            n1139 = Bundle("Left"=w1782, "Top"=w1781, "Width"=w1780, "Height"=w1779) -> (w1770:T33)  [unwired: 1 in]
            n1140 = Bundle("Left"=w1778, "Top"=w1777, "Width"=w1776, "Height"=w1775) -> (w1769:T33)  [unwired: 1 in]
            n1141 = Bundle("Left"=w1774, "Top"=w1773, "Width"=w1772, "Height"=w1771) -> (w1768:T33)  [unwired: 1 in]
            n1142 = Build Cluster Array(w1753, w1770, w1769, w1768) -> (w1767:T34)
            n1143 = for {
              tunnel: w1789 -> [w1800]
              tunnel: w1767 -> [w1801] mode=indexing
              shift-right: [w1798] -> w1765
              shift-left: TRUE -> [w1799]
              shift-right: [w1797] -> w1763
              shift-left: _ -> [w1793]
              shift-right: [w1796] -> w1762
              shift-left: _ -> [w1792]
              shift-right: [w1795] -> w1761
              shift-left: _ -> [w1791]
              shift-right: [w1794] -> w1760
              shift-left: _ -> [w1790]
              n1144 = case shown="True" w1799 {
                selector: w1799 -> [w1806 _]
                tunnel: w1801 -> [_ w1815]
                tunnel: w1800 -> [_ w1813]
                tunnel: [w1806 w1811] -> w1798
                tunnel: [w1805 w1810] -> w1797
                tunnel: [w1804 w1809] -> w1796
                tunnel: [w1803 w1808] -> w1795
                tunnel: [w1802 w1807] -> w1794
                tunnel: w1793 -> [w1805 _]
                tunnel: w1792 -> [w1804 _]
                tunnel: w1791 -> [w1803 _]
                tunnel: w1790 -> [w1802 _]
                frame False {
                }
                frame True {
                  n1145 = Unbundle(w1815) -> (w1814:T33)
                  n1146 = call "isclickinwindow.vi"("Image Param"=w1814, "Point32"=w1813) -> ("4 Y"=w1807:i32, "3 Height"=w1808:i32, "2 X"=w1809:i32, "1 Width"=w1810:i32, "In image?"=w1812:bool)  [unwired: 1 in]
                  n1147 = Not(x=w1812) -> (.not. x?=w1811:bool)
                }
              }
            }
            n1148 = Not(x=w1765) -> (.not. x?=w1764:bool)
            n1149 = case shown="True" w1764 {
              tunnel: w1762 -> [_ w1828]
              tunnel: w1760 -> [_ w1827]
              tunnel: w1763 -> [_ w1826]
              tunnel: w1761 -> [_ w1825]
              frame False {
              }
              frame True {
                w1821 = FALSE ("Get Point")
                n1150 = local read "Scan lines (y)"() -> (w1830:u64)
                n1151 = local read "Actual MCL Inc (V)"() -> (w1822:dbl)
                n1152 = local read "Scan steps (MCL)"() -> (w1829:u64)
                n1153 = Divide "Y Pix/step"(x=w1825, y=w1830) -> (x/y=w1837:dbl)
                n1154 = Divide "Y V/pix"(x=w1822, y=w1837) -> (x/y=w1836:dbl)
                n1155 = Divide "Y half step offset"(x=w1822, y=2.0) -> (x/y=w1838:dbl)
                n1156 = Divide "X pix/step"(x=w1826, y=w1829) -> (x/y=w1835:dbl)
                n1157 = Negate(x=w1838) -> (-x=w1839:dbl)
                n1158 = local read "Initial Y"() -> (w1845:dbl)
                n1159 = Multiply(x=w1827, y=w1836) -> (x*y=w1846:dbl)
                n1160 = Divide "X half step offset"(x=w1822, y=2.0) -> (x/y=w1832:dbl)
                n1161 = Divide "X V/pix"(x=w1822, y=w1835) -> (x/y=w1834:dbl)
                n1162 = Multiply(x=w1822, y=w1829) -> (x*y=w1841:dbl)
                n1163 = Compound Arithmetic op=ADD(w1839, w1846, w1845) -> (w1823:dbl)
                "Pointer Y (V)" <- w1823
                n1164 = Multiply(x=w1834, y=w1828) -> (x*y=w1843:dbl)
                n1165 = Negate(x=w1832) -> (-x=w1831:dbl)
                n1166 = local read "Initial X"() -> (w1844:dbl)
                n1167 = Negate(x=w1843) -> (-x=w1842:dbl)
                n1168 = Compound Arithmetic op=ADD(w1831, w1841, w1844, w1842) -> (w1824:dbl)
                "Pointer X (V)" <- w1824
                n1169 = Or(x="Set X Only", y="Set Confocal Spot (X-Y)") -> (x .or. y?=w1817:bool)
                n1170 = Or(x="Set Confocal Spot (X-Y)", y="Set Y Only") -> (x .or. y?=w1816:bool)
                n1171 = case shown="True" w1817 {
                  tunnel: w1824 -> [_ w1847]
                  frame False {
                  }
                  frame True {
                    n1172 = property on="AO2" class="Slide (strict)"("Val(Sgnl)"=w1847) -> ()  [unwired: 2 in, 2 out]
                  }
                }
                n1173 = case shown="True" w1816 {
                  tunnel: w1823 -> [_ w1848]
                  frame False {
                  }
                  frame True {
                    n1174 = property on="AO1" class="Slide (strict)"("Val(Sgnl)"=w1848) -> ()  [unwired: 2 in, 2 out]
                  }
                }
                n1175 = local write "Set Confocal Spot (X-Y)"(w1821) -> ()
                n1176 = local write "Set X Only"(w1821) -> ()
                n1177 = local write "Set Y Only"(w1821) -> ()
              }
            }
          }
          frame 3 {
            n1178 = local read "BD 2 Frequency 1 (MHz)"() -> (w1849:dbl)
            n1179 = local read "BD 1 Frequency 1 (MHz)"() -> (w1850:dbl)
            n1180 = local write "Manipulating Trap"(TRUE ("Manipulating Trap")) -> ()
            n1181 = local write "Coords"(T7 {"Horizontal"=0, "Vertical"=0} ("Coords")) -> ()
            n1182 = while {
              tunnel: w1855 -> [w1860]
              tunnel: w1853 -> [w1859]
              tunnel: w1851 -> [w1858]
              tunnel: w1850 -> [w1857]
              tunnel: w1849 -> [w1856]
              stop <- w1861 stop-if-true
              n1183 = event shown="[0] \"Pane\": Mouse Move" {
                selector: _ -> [_ _]
                dyn-events: _ -> [_ _]
                timeout: _ -> [_ _]
                tunnel: ["Force Manip Abort" w1925] -> w1861
                tunnel: w1860 -> [w1868 _]
                tunnel: w1859 -> [w1866 _]
                tunnel: w1858 -> [w1865 _]
                tunnel: w1857 -> [w1864 _]
                tunnel: w1856 -> [w1863 _]
                event Mouse Move {
                  n1184 = event-data() -> ("Time"=w1869:u32, "Coords"=w1870:T7)  [unwired: 3 out]
                  n1185 = Less?(x=w1869, y=w1868) -> (x < y?=w1867:bool)
                  n1186 = case "Makes sure old motion events prior to mouse click aren't used" shown="False" w1867 {
                    tunnel: w1870 -> [w1912 _]
                    tunnel: w1866 -> [w1913 _]
                    tunnel: w1865 -> [w1890 _]
                    tunnel: w1864 -> [w1886 _]
                    tunnel: w1863 -> [w1885 _]
                    frame False {
                      n1187 = Subtract(x=w1912, y=w1913) -> (x-y=w1911:T7)
                      "Coords" <- w1911
                      n1188 = local read "Y RF Frequency Limits (MHz)"() -> (w1871:T16)
                      n1189 = To Double Precision Float(number=w1911) -> (double precision float=w1910:cluster{"Horizontal":dbl, "Vertical":dbl})
                      n1190 = Multiply(x=cluster{"Horizontal":dbl, "Vertical":dbl} {"Horizontal"=-1.0, "Vertical"=1.0}, y="Manipulation Scaling") -> (x*y=w1906:cluster{"Horizontal":dbl, "Vertical":dbl})
                      n1191 = local read "X RF Frequency Limits (MHz)"() -> (w1872:T16)
                      n1192 = Multiply(x=w1910, y=w1906) -> (x*y=w1908:cluster{"Horizontal":dbl, "Vertical":dbl})
                      n1193 = Unbundle By Name(w1908) -> ("Horizontal"=w1903:dbl, "Vertical"=w1907:dbl)
                      n1194 = Unbundle By Name(w1871) -> ("Maximum"=w1874:dbl, "Minimum"=w1873:dbl)
                      n1195 = Boolean To (0,1)(Boolean="Manip. X?") -> (0, 1=w1901:i16)
                      n1196 = Boolean To (0,1)(Boolean="Manip. Y?") -> (0, 1=w1898:i16)
                      n1197 = local read "BD 1 Frequency 2 (MHz)"() -> (w1888:dbl)
                      n1198 = Multiply(x=w1907, y=w1898) -> (x*y=w1900:dbl)
                      n1199 = Multiply(x=w1901, y=w1903) -> (x*y=w1904:dbl)
                      n1200 = local read "BD 2 Frequency 2 (MHz)"() -> (w1887:dbl)
                      n1201 = Unbundle By Name(w1872) -> ("Maximum"=w1876:dbl, "Minimum"=w1875:dbl)
                      n1202 = Add(x=w1885, y=w1900) -> (x+y=w1878:dbl)
                      n1203 = Add(x=w1886, y=w1904) -> (x+y=w1880:dbl)
                      n1204 = In Range and Coerce(upper limit=w1876, x=w1880, lower limit=w1875) -> (coerced(x)=w1879:dbl)  [unwired: 1 out]
                      n1205 = In Range and Coerce(upper limit=w1874, x=w1878, lower limit=w1873) -> (coerced(x)=w1877:dbl)  [unwired: 1 out]
                      n1206 = Subtract(x=w1879, y=w1888) -> (x-y=w1897:dbl)
                      n1207 = Subtract(x=w1877, y=w1887) -> (x-y=w1896:dbl)
                      n1208 = Square(x=w1897) -> (x^2=w1895:dbl)
                      n1209 = Square(x=w1896) -> (x^2=w1894:dbl)
                      n1210 = Add(x=w1895, y=w1894) -> (x+y=w1893:dbl)
                      n1211 = Square Root(x=w1893) -> (sqrt(x)=w1889:dbl)
                      n1212 = In Range and Coerce(upper limit="Limit Max (MHz)", x=w1889, lower limit="Limit Min (MHz)") -> (In Range?=w1882:bool)  [unwired: 1 out]
                      n1213 = Not(x="Limits Enable") -> (.not. x?=w1881:bool)
                      n1214 = Or(x=w1882, y=w1881) -> (x .or. y?=w1883:bool)
                      n1215 = case shown="True" w1883 {
                        tunnel: w1890 -> [_ w1923]
                        tunnel: w1889 -> [_ w1914]
                        tunnel: w1879 -> [_ w1921]
                        tunnel: w1888 -> [_ w1920]
                        tunnel: w1877 -> [_ w1919]
                        tunnel: w1887 -> [_ w1918]
                        tunnel: w1872 -> [_ w1916]
                        tunnel: w1871 -> [_ w1915]
                        frame False {
                        }
                        frame True {
                          n1216 = local read "BD 1 Frequency 3 (MHz)"() -> (w1922:dbl)
                          n1217 = local read "BD 2 Frequency 3 (MHz)"() -> (w1917:dbl)
                          n1218 = local write "Trap Delta (MHz)"(w1914) -> ()
                          n1219 = property on="Initial delta (MHz)" class="DigNum (strict)"("Val(Sgnl)"=w1914) -> ()  [unwired: 2 in, 2 out]
                          n1220 = call "set RF board frequency - interlace.vi"("Board 2 Frequency Limits"=w1915, "Board 1 Frequency Limits"=w1916, "FPGA VI Reference In"=w1923, "Board 2 Frequency 3 (MHz)"=w1917, "Board 1 Frequency 3 (MHz)"=w1922, "Board 2 Frequency 2 (MHz)"=w1918, "Board 2 Frequency 1 (MHz)"=w1919, "Board 1 Frequency 2 (MHz)"=w1920, "Board 1 Frequency 1  (MHz)"=w1921) -> ()  [unwired: 1 in, 2 out]
                          n1221 = local write "BD 2 Frequency 1 (MHz)"(w1919) -> ()
                          n1222 = local write "BD 1 Frequency 1 (MHz)"(w1921) -> ()
                        }
                      }
                    }
                    frame True {
                    }
                  }
                }
                event Mouse Up {
                  n1223 = event-data() -> ("Button"=w1924:u16)  [unwired: 8 out]
                  n1224 = case shown="3" w1924 {
                    tunnel: [FALSE TRUE] -> w1925
                    frame 0, Default {
                    }
                    frame 3 {
                      n1225 = local write "Manipulating Trap"(FALSE ("Manipulating Trap")) -> ()
                    }
                  }
                }
              }
            }
          }
        }
      }
      event Mouse Move {
        n1226 = event-data() -> ()  [unwired: 6 out]
      }
    }
    n1227 = local read "Stop All"() -> (w1746:bool)
    n1228 = node-c288() -> ()  [unwired: 2 out]
  }
  n1229 = node-c288(i64 1 ("Period"), 1 ("Processor")) -> (w164:T24)  [unwired: 2 out]
  n1230 = timed-loop "Acquire Data" {
    tunnel: w24 -> [w2183]
    tunnel: w40 -> [w2182]
    tunnel: [w2213] -> w33
    tunnel: [w2207] -> w32
    timing: w164 -> [_]
    timing-out: [_] -> w163
    tunnel: w59 -> [w2011]
    stop <- "Stop All" stop-if-true
    (unwired) u32 0 ("Number of Elements")
    w1998 = "NI_ChannelName" ("name")
    n1231 = node-c288() -> ()  [unwired: 2 out]
    n1232 = First Call?() -> (First Call?: T/F=w1964:bool)
    n1233 = Or(x="Reset", y=w1964) -> (x .or. y?=w1965:bool)
    n1234 = case "Reset data stream" shown="True" w1965 {
      tunnel: w2183 -> [w2229 w2237]
      tunnel: w2182 -> [w2228 w2236]
      tunnel: [w2229 w2231] -> w2178
      tunnel: [w2228 w2230] -> w2177
      frame False {
      }
      frame True {
        w2234 = TRUE ("AI to FIFO")
        n1235 = local write "Overflow (data lost)"(FALSE ("Overflow (data lost)")) -> ()
        n1236 = call "reset FPGA DMA.vi"("error in"=w2236, "FPGA VI Reference In"=w2237) -> ("error out"=w2232:errorcluster, "FPGA VI Reference Out"=w2233:T19)
        n1237 = xnode "Read/Write Control"("FPGA VI Reference In"=w2233, "error in"=w2232, "AI to FIFO"=w2234, "APD to FIFO"=w2234) -> ("FPGA VI Reference Out"=w2231:T19, "error out"=w2230:errorcluster)
      }
    }
    n1238 = Or(x="Start AOD Scan", y="Trap Raster Scan") -> (x .or. y?=w2128:bool)
    n1239 = case "Start AOM raster scan" shown="True" w2128 {
      tunnel: w2178 -> [w2966 w2976]
      tunnel: w2177 -> [w2965 w2975]
      tunnel: [w2966 w2969] -> w2176
      tunnel: [w2965 w2968] -> w2175
      frame False {
      }
      frame True {
        n1240 = case shown="True" "Restart DMA? (AOD)" {
          tunnel: [w3014 w3016] -> w2970
          tunnel: [w3013 w3015] -> w2971
          tunnel: w2976 -> [w3014 w3018]
          tunnel: w2975 -> [w3013 w3017]
          frame False {
          }
          frame True {
            n1241 = local write "Overflow (data lost)"(FALSE ("Overflow (data lost)")) -> ()
            n1242 = call "reset FPGA DMA.vi"("error in"=w3017, "FPGA VI Reference In"=w3018) -> ("error out"=w3015:errorcluster, "FPGA VI Reference Out"=w3016:T19)
          }
        }
        n1243 = local write "Trap Raster Scan"(FALSE ("Trap Raster Scan")) -> ()
        n1244 = case shown="False" "Move MCL Also?" {
          tunnel: w2971 -> [w2979 w3008]
          tunnel: w2970 -> [w2980 w3009]
          tunnel: [w2978 w3012] -> w2969
          tunnel: [w2977 w3011] -> w2968
          frame False {
            w2981 = TRUE ("AI to FIFO")
            n1245 = xnode "Read/Write Control"("FPGA VI Reference In"=w2980, "error in"=w2979, "AI to FIFO"=w2981, "APD to FIFO"=w2981, "Start scan"=w2981) -> ("FPGA VI Reference Out"=w2978:T19, "error out"=w2977:errorcluster)
          }
          frame True {
            w3005 = FALSE ("1D or 2D Scan?")
            w3010 = TRUE ("AI to FIFO")
            # "Count for MCL loop"
            # "N total cycles"
            # "N steps"
            # "V_int"
            n1246 = local read "Scan Range (nm)"() -> (w2987:dbl)
            n1247 = local read "Number of F/B Scans (AOD)"() -> (w3004:u16)
            n1248 = Sign(1:w2987) -> (0:w2986:dbl)
            n1249 = Compound Arithmetic op=MULTIPLY(w2987, "MCL Step Position Ratio", "MCL/AOM Scale Tweak") -> (w2991:dbl)
            n1250 = Negate(x=w2986) -> (-x=w2983:dbl)
            n1251 = Multiply(x=w2983, y="MCL Step Increment (V_int)") -> (x*y=w2985:dbl)
            n1252 = Divide(x=w2991, y="MCL X Cal (nm/V)") -> (x/y=w2997:dbl)
            n1253 = Multiply(x=32767.0 ("y"), y=w2997) -> (x*y=w3003:dbl)
            n1254 = local read "Total Counts (ticks)"() -> (w2988:u32)
            n1255 = local read "Cycles/step (AOD)"() -> (w2999:u64)
            n1256 = local read "Scan steps (AOD)"() -> (w3000:u64)
            n1257 = Divide(x=w3003, y=10.0) -> (x/y=w2996:dbl)
            n1258 = Divide(x=w2996, y="MCL Step Increment (V_int)") -> (x/y=w2994:dbl)
            n1259 = Absolute Value(x=w2994) -> (abs(x)=w2982:dbl)
            n1260 = Compound Arithmetic op=MULTIPLY(w3000, w2999, w2988) -> (w2995:u64)
            n1261 = local write "wait to reset values"(w3010) -> ()
            n1262 = local write "MCL Scanning"(w3010) -> ()
            n1263 = Divide(x=w2995, y=w2982) -> (x/y=w2992:dbl)
            "MCL Count" <- w2992
            n1264 = xnode "Read/Write Control"("FPGA VI Reference In"=w3009, "error in"=w3008, "Scan steps (MCL)"=w2982, "Number of scans (MCL)"=w3004, "Cycles per step (MCL)"=u64 1, "Scan freq.  increment (MCL)"=w2985, "1D or 2D Scan?"=w3005, "MCL Scan Axis"=w3005, "Cont. Scan (MCL)"=w3005, "MCL count"=w2992) -> ("FPGA VI Reference Out"=w3007:T19, "error out"=w3006:errorcluster)
            n1265 = xnode "Read/Write Control"("FPGA VI Reference In"=w3007, "error in"=w3006, "AI to FIFO"=w3010, "APD to FIFO"=w3010, "Start scan"=w3010, "Start scan (MCL)"=w3010) -> ("FPGA VI Reference Out"=w3012:T19, "error out"=w3011:errorcluster)
          }
        }
        "Raster Scanning..." <- TRUE ("Scanning...")
      }
    }
    n1266 = And(x="Save scans", y=w2128) -> (x .and. y?=w2174:bool)
    n1267 = Compound Arithmetic op=OR("Start MCL Scan", "Confocal Image", "Confocal Linescan") -> (w2126:bool)
    n1268 = And(x="Save Data (MCL)", y=w2126) -> (x .and. y?=w2173:bool)
    n1269 = case "Start MCL raster scan" shown="True" w2126 {
      tunnel: w2176 -> [w2520 w2535]
      tunnel: w2175 -> [w2519 w2534]
      tunnel: [w2520 w2530] -> w1933
      tunnel: [w2519 w2529] -> w1932
      tunnel: [FALSE w2528] -> w2159
      tunnel: "Start MCL Scan" -> [_ w2523]
      tunnel: "Confocal Image" -> [_ w2522]
      tunnel: "Confocal Linescan" -> [_ _]
      frame False {
      }
      frame True {
        w2528 = TRUE
        n1270 = case shown="True" "Restart DMA? (MCL)" {
          tunnel: [w2580 w2582] -> w2533
          tunnel: [w2579 w2581] -> w2532
          tunnel: w2535 -> [w2580 w2585]
          tunnel: w2534 -> [w2579 w2584]
          frame False {
          }
          frame True {
            n1271 = call "reset FPGA DMA.vi"("error in"=w2584, "FPGA VI Reference In"=w2585) -> ("error out"=w2581:errorcluster, "FPGA VI Reference Out"=w2582:T19)
            n1272 = local write "Overflow (data lost)"(FALSE ("Overflow (data lost)")) -> ()
          }
        }
        n1273 = case shown="False" w2523 {
          selector: w2523 -> [_ w2539]
          tunnel: w2522 -> [w2538 _]
          tunnel: [w2538 w2539] -> w2521
          frame False {
            n1274 = property on="2D or 1D Scan" class="Bool (strict)"("Val(Sgnl)"=w2538) -> ()  [unwired: 2 in, 2 out]
            n1275 = property on="Confocal Image" class="Bool (strict)"("Value"=FALSE ("Start Confocal Map")) -> ()  [unwired: 2 in, 2 out]
          }
          frame True {
          }
        }
        n1276 = local write "MCL Scanning"(w2528) -> ()
        n1277 = local read "AO1"() -> (w2525:dbl)
        n1278 = local read "AO2"() -> (w2524:dbl)
        n1279 = case shown="True" "Center Scan" {
          tunnel: w2533 -> [w2546 w2578]
          tunnel: w2532 -> [w2545 w2577]
          tunnel: [w2544 w2576] -> w2530
          tunnel: [w2543 w2575] -> w2529
          tunnel: [w2541 w2562] -> w2527
          tunnel: [w2540 w2561] -> w2526
          tunnel: w2525 -> [w2541 w2567]
          tunnel: w2524 -> [w2540 w2570]
          tunnel: w2521 -> [_ _]
          frame False {
            w2542 = TRUE ("AI to FIFO")
            n1280 = xnode "Read/Write Control"("FPGA VI Reference In"=w2546, "error in"=w2545, "AI to FIFO"=w2542, "APD to FIFO"=w2542, "Start scan (MCL)"=w2542) -> ("FPGA VI Reference Out"=w2544:T19, "error out"=w2543:errorcluster)
          }
          frame True {
            w2574 = TRUE ("AI to FIFO")
            n1281 = local read "Scan steps (MCL)"() -> (w2553:u64)
            n1282 = local read "Scan lines (y)"() -> (w2549:u64)
            n1283 = local read "Fast Scan Dir"() -> (w2560:bool)
            n1284 = local read "Actual MCL Inc (V)"() -> (w2550:dbl)
            n1285 = Decrement(x=w2549) -> (x-1=w2548:u64)
            n1286 = Decrement(x=w2553) -> (x-1=w2552:u64)
            n1287 = Multiply(x=w2550, y=w2548) -> (x*y=w2547:dbl)
            n1288 = Divide(x=w2547, y=2.0) -> (x/y=w2557:dbl)
            n1289 = Multiply(x=w2550, y=w2552) -> (x*y=w2551:dbl)
            n1290 = Divide(x=w2551, y=2.0) -> (x/y=w2556:dbl)
            n1291 = Select(t=w2556, s=w2560, f=w2557) -> (s? t:f=w2555:dbl)
            n1292 = Select(t=w2557, s=w2560, f=w2556) -> (s? t:f=w2559:dbl)
            n1293 = Subtract(x=w2567, y=w2559) -> (x-y=w2558:dbl)
            n1294 = Subtract(x=w2570, y=w2555) -> (x-y=w2554:dbl)
            n1295 = local read "2D or 1D Scan"() -> (w2572:bool)
            n1296 = Not(x=w2560) -> (.not. x?=w2566:bool)
            n1297 = Not(x=w2572) -> (.not. x?=w2568:bool)
            n1298 = And(x=w2560, y=w2568) -> (x .and. y?=w2569:bool)
            n1299 = And(x=w2568, y=w2566) -> (x .and. y?=w2571:bool)
            n1300 = Select(t=w2570, s=w2571, f=w2554) -> (s? t:f=w2561:dbl)
            n1301 = Select(t=w2567, s=w2569, f=w2558) -> (s? t:f=w2562:dbl)
            n1302 = call "Volt to I16.vi"("Voltage In"=w2562) -> ("I16 Voltage Out"=w2565:i16)
            n1303 = call "Volt to I16.vi"("Voltage In"=w2561) -> ("I16 Voltage Out"=w2564:i16)
            n1304 = xnode "Read/Write Control"("FPGA VI Reference In"=w2578, "error in"=w2577, "AI to FIFO"=w2574, "APD to FIFO"=w2574, "Start scan (MCL)"=w2574, "AO1"=w2565, "AO2"=w2564) -> ("FPGA VI Reference Out"=w2576:T19, "error out"=w2575:errorcluster)
          }
        }
        "Initial Y" <- w2527
        "Initial X" <- w2526
        "wait to reset values" <- w2528
      }
    }
    n1305 = local read "Trap Pos Elements/DMA read"() -> (w2007:u32)
    n1306 = local read "Trap AI Elements/DMA read"() -> (w1931:u32)
    n1307 = local read "APD Elements/DMA read"() -> (w2050:u32)
    n1308 = local read "Trap AI FIFO Depth"() -> (w2223:u32)
    n1309 = xnode "Invoke Method"("FPGA VI Reference In"=w1933, "error in"=w1932, "Number of Elements"=w2007, "Timeout (ms)"=-1) -> ("Data"=w1971:u16[], "Elements Remaining"=→"Trap Pos FIFO El Remaining":u32)  [unwired: 2 out]
    n1310 = xnode "Invoke Method"("FPGA VI Reference In"=w1933, "error in"=w1932, "Number of Elements"=w1931, "Timeout (ms)"=-1 ("Timeout")) -> ("FPGA VI Reference Out"=w1935:T19, "error out"=w1934:errorcluster, "Data"=w1930:i16[], "Elements Remaining"=w1936:u32)
    "Trap AI FIFO El. Rem." <- w1936
    n1311 = xnode "Get APD Data"("FPGA VI Reference In"=w1933, "error in"=w1932, "Number of Elements"=w2050, "Timeout (ms)"=-1) -> ("Data"=w2049:u32[], "Elements Remaining"=→"APD FIFO Elements Remaining":u32)  [unwired: 2 out]
    n1312 = Subtract(x=w2223, y=w1931) -> (x-y=w2222:u32)
    n1313 = Decimate 1D Array(w1971) -> (w1968:u16[], w1970:u16[], w1969:u16[])
    n1314 = Divide(x=w1936, y=w2222) -> (x/y=w2221:dbl)
    "Buffer Status" <- w2221
    n1315 = To Unsigned Long Integer(number=w1968) -> (unsigned 32bit integer=w1967:u32[])
    n1316 = Join Numbers(hi=w1970, lo=w1969) -> ((hi.lo)=w1966:u32[])
    n1317 = Equal?(x=w2221, y=1.0) -> (x = y?=w2219:bool)
    n1318 = Join Numbers(hi=w1967, lo=w1966) -> ((hi.lo)=w1960:u64[])
    n1319 = call "IR AOM word to freq - vec.vi"("Frequency Word In (double vec)"=w1960) -> ("Frequency Out"=w2006:dbl[])
    n1320 = case "Alert buffer overflow" shown="False" w2219 {
      frame False {
      }
      frame True {
        n1321 = call <vilib>:"Beep.vi"() -> ()  [unwired: 3 in, 9 out]
        "Overflow (data lost)" <- TRUE ("Overflow (data lost)")
      }
    }
    n1322 = Decimate 1D Array(w2006) -> (w2005:dbl[], w2004:dbl[])
    n1323 = Array Size(array=w1930) -> (size(s)=→"Waveform Chart":i32)
    n1324 = Build Array(w2005, w2004) -> (w2003:dbl[][])
    n1325 = local read "Trap Sets"() -> (w2087:u32)
    n1326 = case "Deinterlace trap data, average down PSD" shown="2" w2087 {
      tunnel: w1930 -> [w2615 w2680]
      tunnel: [w2612 w2677] -> w2080
      tunnel: [w2615 w2679] -> w1963
      tunnel: "Detector Type" -> [w2614 w2675]
      tunnel: [w2613 w2678] -> w2079
      tunnel: [w2611 w2676] -> w2194
      frame 1, Default {
        n1327 = Divide(x=w2615, y=3276.7) -> (x/y=w2616:dbl[])
        n1328 = Decimate 1D Array(w2616) -> (w2625:dbl[], w2624:dbl[], w2623:dbl[], w2622:dbl[], w2621:dbl[], w2620:dbl[], w2619:dbl[], w2618:dbl[])
        n1329 = case shown="\"IR-QPD + PSD + FB-QPD position\"" w2614 {
          tunnel: w2625 -> [w2649 w2674]
          tunnel: w2624 -> [w2648 w2673]
          tunnel: w2623 -> [w2633 w2651]
          tunnel: w2622 -> [w2634 w2661]
          tunnel: w2621 -> [w2647 w2672]
          tunnel: w2620 -> [w2646 w2671]
          tunnel: w2619 -> [w2630 w2652]
          tunnel: w2618 -> [w2629 w2650]
          tunnel: [w2628 w2658] -> w2613
          tunnel: [w2627 w2657] -> w2612
          tunnel: [w2626 w2656] -> w2611
          frame "IR-QPD + PSD + FB-QPD", Default {
            w2626 = 0  # Channel pattern
            n1330 = Divide(x=w2649, y=w2634) -> (x/y=w2636:dbl[])
            n1331 = Divide(x=w2648, y=w2634) -> (x/y=w2635:dbl[])
            n1332 = Divide(x=w2647, y=w2630) -> (x/y=w2632:dbl[])
            n1333 = Divide(x=w2646, y=w2629) -> (x/y=w2631:dbl[])
            n1334 = Build Array(w2636, w2635, w2634, w2633, w2632, w2631, w2630, w2629) -> (w2627:dbl[][])
            n1335 = Bundle("T1 Y", "T1 X", "T1 Sum", "FB Sum", "PSD Y", "PSD X", "PSD Y Sum", "PSD X Sum") -> (w2645:T41)  [unwired: 1 out]
            n1336 = Cluster To Array(cluster=w2645) -> (array=w2628:string[])
          }
          frame "IR-QPD + PSD + FB-QPD position" {
            w2656 = 3  # Channel pattern
            n1337 = Negate(x=w2652) -> (-x=w2653:dbl[])
            n1338 = Divide(x=w2674, y=w2661) -> (x/y=w2663:dbl[])
            n1339 = Divide(x=w2673, y=w2661) -> (x/y=w2662:dbl[])
            n1340 = Divide(x=w2672, y=w2652) -> (x/y=w2660:dbl[])
            n1341 = Divide(x=w2671, y=w2653) -> (x/y=w2659:dbl[])
            n1342 = Build Array(w2663, w2662, w2661, w2650, w2651, w2660, w2659, w2652) -> (w2657:dbl[][])
            n1343 = Bundle("T1 Y", "T1 X", "T1 Sum", "FB X", "FB Sum", "PSD Y", "PSD X", "PSD Y Sum") -> (w2670:T41)  [unwired: 1 out]
            n1344 = Cluster To Array(cluster=w2670) -> (array=w2658:string[])
          }
        }
      }
      frame 2 {
        n1345 = case shown="\"UCB Fleezers 052511\"" w2675 {
          tunnel: w2680 -> [w2742 w2809 w2837 w2944]
          tunnel: [w2681 w2801 w2832 w2875] -> w2679
          tunnel: [w2708 w2792 w2834 w2922] -> w2678
          tunnel: [w2707 w2756 w2811 w2889] -> w2677
          tunnel: [w2701 w2791 w2874 w2920] -> w2676
          frame "IR-QPD + PSD + FB-QPD", Default {
            w2701 = 1  # Channel pattern
            # "time average x2 the 4th signal and the 4 psd signals (detection laser)"
            # "deinterlace 3 signals from qpd"
            n1346 = Decimate 1D Array(w2742) -> (w2741:i16[], w2740:i16[], w2706:i16[], w2739:i16[], w2729:i16[], w2727:i16[], w2726:i16[], w2724:i16[])
            n1347 = call "downsample 1D array - double.vi"("Ave N"=2.0, "Array In"=w2729) -> ("Array Out"=w2728:dbl[])  [unwired: 1 out]
            n1348 = call "downsample 1D array - double.vi"("Ave N"=2.0, "Array In"=w2724) -> ("Array Out"=w2723:dbl[])  [unwired: 1 out]
            n1349 = call "downsample 1D array - double.vi"("Ave N"=2.0, "Array In"=w2726) -> ("Array Out"=w2725:dbl[])  [unwired: 1 out]
            n1350 = call "downsample 1D array - double.vi"("Ave N"=2.0, "Array In"=w2727) -> ("Array Out"=w2709:dbl[])  [unwired: 1 out]
            n1351 = Decimate 1D Array(w2741) -> (w2738:i16[], w2710:i16[])
            n1352 = Decimate 1D Array(w2740) -> (w2737:i16[], w2735:i16[])
            n1353 = Decimate 1D Array(w2739) -> (w2736:i16[], w2734:i16[])
            n1354 = Decimate 1D Array(w2706) -> (w2705:i16[], w2704:i16[])
            n1355 = Interleave 1D Arrays(w2738, w2737, w2736, w2710, w2735, w2734, w2705, w2704, w2728, w2709, w2725, w2723) -> (w2722:dbl[])
            n1356 = To Word Integer(number=w2722) -> (16bit integer=w2681:i16[])
            n1357 = Divide(x=w2722, y=3276.7) -> (x/y=w2721:dbl[])
            n1358 = Decimate 1D Array(w2721) -> (w2720:dbl[], w2719:dbl[], w2718:dbl[], w2717:dbl[], w2716:dbl[], w2715:dbl[], w2703:dbl[], w2702:dbl[], w2714:dbl[], w2713:dbl[], w2712:dbl[], w2711:dbl[])
            n1359 = Divide(x=w2720, y=w2718) -> (x/y=w2688:dbl[])
            n1360 = Divide(x=w2719, y=w2718) -> (x/y=w2687:dbl[])
            n1361 = Divide(x=w2717, y=w2715) -> (x/y=w2686:dbl[])
            n1362 = Divide(x=w2716, y=w2715) -> (x/y=w2685:dbl[])
            n1363 = Divide(x=w2714, y=w2712) -> (x/y=w2684:dbl[])
            n1364 = Divide(x=w2713, y=w2711) -> (x/y=w2683:dbl[])
            n1365 = Bundle("T1 Y", "T1 X", "T1 Sum", "T2 Y", "T2 X", "T2 Sum", "T1 FB Sum", "T2 FB Sum", "PSD Y", "PSD X", "PSD Y Sum", "PSD X Sum") -> (w2689:T42)  [unwired: 1 out]
            n1366 = Build Array(w2688, w2687, w2718, w2686, w2685, w2715, w2703, w2702, w2684, w2683, w2712, w2711) -> (w2707:dbl[][])
            n1367 = Cluster To Array(cluster=w2689) -> (array=w2708:string[])
          }
          frame "IR-QPD + PSD + FB-QPD X position" {
            w2791 = 2  # Channel pattern
            # "convert\nADC numbers\nto volts"
            # "time average x2 the 3 psd signals (detection laser)"
            # "deinterlace 3 signals from qpds"
            n1368 = Decimate 1D Array(w2809) -> (w2808:i16[], w2807:i16[], w2744:i16[], w2745:i16[], w2754:i16[], w2751:i16[], w2748:i16[], w2779:i16[])
            n1369 = Decimate 1D Array(w2808) -> (w2806:i16[], w2793:i16[])
            n1370 = call "downsample 1D array - I16.vi"("Ave N"=2.0, "Array In"=w2754) -> ("Array Out"=w2752:i16[])  [unwired: 1 in]
            n1371 = call "downsample 1D array - I16.vi"("Ave N"=2.0, "Array In"=w2751) -> ("Array Out"=w2749:i16[])  [unwired: 1 in]
            n1372 = Decimate 1D Array(w2807) -> (w2805:i16[], w2803:i16[])
            n1373 = Decimate 1D Array(w2745) -> (w2804:i16[], w2802:i16[])
            n1374 = Decimate 1D Array(w2779) -> (w2778:i16[], w2776:i16[])
            n1375 = Decimate 1D Array(w2744) -> (w2777:i16[], w2775:i16[])
            n1376 = call "downsample 1D array - I16.vi"("Ave N"=2.0, "Array In"=w2748) -> ("Array Out"=w2746:i16[])  [unwired: 1 in]
            n1377 = Interleave 1D Arrays(w2806, w2805, w2804, w2793, w2803, w2802, w2778, w2777, w2776, w2775, w2752, w2749, w2746) -> (w2801:i16[])
            n1378 = Divide(x=w2801, y=3276.7) -> (x/y=w2800:dbl[])
            n1379 = Decimate 1D Array(w2800) -> (w2799:dbl[], w2798:dbl[], w2797:dbl[], w2796:dbl[], w2795:dbl[], w2794:dbl[], w2767:dbl[], w2765:dbl[], w2764:dbl[], w2762:dbl[], w2761:dbl[], w2760:dbl[], w2757:dbl[])
            n1380 = Divide(x=w2799, y=w2797) -> (x/y=w2783:dbl[])
            n1381 = Divide(x=w2798, y=w2797) -> (x/y=w2782:dbl[])
            n1382 = Divide(x=w2796, y=w2794) -> (x/y=w2781:dbl[])
            n1383 = Divide(x=w2795, y=w2794) -> (x/y=w2780:dbl[])
            n1384 = Divide(x=w2767, y=w2765) -> (x/y=w2766:dbl[])
            n1385 = Divide(x=w2764, y=w2762) -> (x/y=w2763:dbl[])
            n1386 = Divide(x=w2761, y=w2757) -> (x/y=w2759:dbl[])
            n1387 = Negate(x=w2757) -> (-x=w2755:dbl[])
            n1388 = Divide(x=w2760, y=w2755) -> (x/y=w2758:dbl[])
            n1389 = Bundle("T1 Y", "T1 X", "T1 Sum", "T2 Y", "T2 X", "T2 Sum", "T1 FB X", "T1 FB Sum", "T2 FB X", "T2 FB Sum", "PSD Y", "PSD X", "PSD Y Sum") -> (w2784:T43)  [unwired: 1 out]
            n1390 = Build Array(w2783, w2782, w2797, w2781, w2780, w2794, w2766, w2765, w2763, w2762, w2759, w2758, w2757) -> (w2756:dbl[][])
            n1391 = Cluster To Array(cluster=w2784) -> (array=w2792:string[])
          }
          frame "UCB Fleezers 052511" {
            w2874 = 2  # Channel pattern
            n1392 = Decimate 1D Array(w2837) -> (w2872:i16[], w2871:i16[], w2836:i16[], w2835:i16[], w2829:i16[], w2826:i16[], w2825:i16[], w2824:i16[])
            n1393 = Decimate 1D Array(w2872) -> (w2870:i16[], w2855:i16[])
            n1394 = Decimate 1D Array(w2871) -> (w2869:i16[], w2867:i16[])
            n1395 = Decimate 1D Array(w2836) -> (w2868:i16[], w2866:i16[])
            n1396 = Decimate 1D Array(w2835) -> (w2831:i16[], w2830:i16[])
            n1397 = Decimate 1D Array(w2829) -> (w2828:i16[], w2827:i16[])
            n1398 = call "downsample 1D array - I16.vi"("Ave N"=2.0, "Array In"=w2826) -> ("Array Out"=w2823:i16[])  [unwired: 1 in]
            n1399 = call "downsample 1D array - I16.vi"("Ave N"=2.0, "Array In"=w2825) -> ("Array Out"=w2822:i16[])  [unwired: 1 in]
            n1400 = call "downsample 1D array - I16.vi"("Ave N"=2.0, "Array In"=w2824) -> ("Array Out"=w2821:i16[])  [unwired: 1 in]
            n1401 = Interleave 1D Arrays(w2870, w2869, w2868, w2855, w2867, w2866, w2831, w2828, w2830, w2827, w2823, w2822, w2821) -> (w2832:i16[])
            n1402 = Divide(x=w2832, y=3276.7) -> (x/y=w2862:dbl[])
            n1403 = Decimate 1D Array(w2862) -> (w2861:dbl[], w2860:dbl[], w2859:dbl[], w2858:dbl[], w2857:dbl[], w2856:dbl[], w2820:dbl[], w2818:dbl[], w2817:dbl[], w2815:dbl[], w2814:dbl[], w2813:dbl[], w2812:dbl[])
            n1404 = Divide(x=w2861, y=w2859) -> (x/y=w2842:dbl[])
            n1405 = Divide(x=w2860, y=w2859) -> (x/y=w2841:dbl[])
            n1406 = Divide(x=w2858, y=w2856) -> (x/y=w2840:dbl[])
            n1407 = Divide(x=w2857, y=w2856) -> (x/y=w2839:dbl[])
            n1408 = Divide(x=w2820, y=w2818) -> (x/y=w2819:dbl[])
            n1409 = Divide(x=w2817, y=w2815) -> (x/y=w2816:dbl[])
            n1410 = Bundle("T1 Y", "T1 X", "T1 Sum", "T2 Y", "T2 X", "T2 Sum", "T1 FB X", "T2 FB Sum", "T2 FB X", "T2 FB Sum", "PSD Y", "PSD X", "PSD Sum") -> (w2843:T43)  [unwired: 1 out]
            n1411 = Build Array(w2842, w2841, w2859, w2840, w2839, w2856, w2819, w2818, w2816, w2815, w2814, w2813, w2812) -> (w2811:dbl[][])
            n1412 = Cluster To Array(cluster=w2843) -> (array=w2834:string[])
          }
          frame "IR-QPD + PSD + FB-QPD XY positions" {
            w2920 = 4  # Channel pattern
            # "time average x2 the 3 psd signals (detection laser)"
            # "deinterlace 3 signals from qpds"
            n1413 = Decimate 1D Array(w2944) -> (w2943:i16[], w2942:i16[], w2921:i16[], w2941:i16[], w2887:i16[], w2933:i16[], w2932:i16[], w2909:i16[])
            n1414 = Decimate 1D Array "QPD Y"(w2943) -> (w2940:i16[], w2923:i16[])
            n1415 = call "downsample 1D array - double.vi"("Ave N"=2.0, "Array In"=w2933) -> ("Array Out"=w2908:dbl[])  [unwired: 1 out]
            n1416 = call "downsample 1D array - double.vi"("Ave N"=2.0, "Array In"=w2932) -> ("Array Out"=w2907:dbl[])  [unwired: 1 out]
            n1417 = Decimate 1D Array "Feedback Sum"(w2921) -> (w2905:i16[], w2903:i16[])
            n1418 = Decimate 1D Array "Feedback Y"(w2887) -> (w2886:i16[], w2885:i16[])
            n1419 = Decimate 1D Array "Feedback X"(w2909) -> (w2906:i16[], w2904:i16[])
            n1420 = Decimate 1D Array "QPD Sum"(w2941) -> (w2938:i16[], w2936:i16[])
            n1421 = Decimate 1D Array "QPD X"(w2942) -> (w2939:i16[], w2937:i16[])
            n1422 = Interleave 1D Arrays(w2940, w2939, w2938, w2923, w2937, w2936, w2886, w2906, w2905, w2885, w2904, w2903, w2908, w2907) -> (w2931:dbl[])
            n1423 = To Word Integer(number=w2931) -> (16bit integer=w2875:i16[])
            n1424 = Divide(x=w2931, y=3276.7) -> (x/y=w2930:dbl[])
            n1425 = Decimate 1D Array(w2930) -> (w2929:dbl[], w2928:dbl[], w2927:dbl[], w2926:dbl[], w2925:dbl[], w2924:dbl[], w2882:dbl[], w2896:dbl[], w2880:dbl[], w2881:dbl[], w2894:dbl[], w2878:dbl[], w2892:dbl[], w2890:dbl[])
            n1426 = Divide(x=w2929, y=w2927) -> (x/y=w2913:dbl[])
            n1427 = Divide(x=w2928, y=w2927) -> (x/y=w2912:dbl[])
            n1428 = Divide(x=w2926, y=w2924) -> (x/y=w2911:dbl[])
            n1429 = Divide(x=w2925, y=w2924) -> (x/y=w2910:dbl[])
            n1430 = Divide(x=w2882, y=w2880) -> (x/y=w2879:dbl[])
            n1431 = Divide(x=w2896, y=w2880) -> (x/y=w2895:dbl[])
            n1432 = Divide(x=w2881, y=w2878) -> (x/y=w2877:dbl[])
            n1433 = Divide(x=w2894, y=w2878) -> (x/y=w2893:dbl[])
            n1434 = Negate(x=w2890) -> (-x=w2888:dbl[])
            n1435 = Divide(x=w2892, y=w2888) -> (x/y=w2891:dbl[])
            n1436 = Bundle("T1 Y", "T1 X", "T1 Sum", "T2 Y", "T2 X", "T2 Sum", "T1 FB Y", "T1 FB X", "T1 FB Sum", "T2 FB Y", "T2 FB X", "T2 FB Sum", "PSD X", "PSD Y Sum") -> (w2876:T44)  [unwired: 1 out]
            n1437 = Build Array(w2913, w2912, w2927, w2911, w2910, w2924, w2879, w2895, w2880, w2877, w2893, w2878, w2891, w2890) -> (w2889:dbl[][])
            n1438 = Cluster To Array(cluster=w2876) -> (array=w2922:string[])
          }
        }
      }
    }
    "AI labels" <- w2079
    n1439 = Decimate 1D Array(w2049) -> (w2077:u32[], w2013:u32[])
    n1440 = local read "DMA Update Period (s)"() -> (w2088:dbl)
    n1441 = local read "BD 1 Frequency 2 (MHz)"() -> (w1955:dbl)
    n1442 = local read "BD 1 Frequency 1 (MHz)"() -> (w1956:dbl)
    n1443 = Build Array(w2077, w2013) -> (w2156:u32[][])
    n1444 = local read "Data Period (s)"() -> (w2062:dbl)
    n1445 = Decimate 1D Array(w1963) -> (w1986:i16[], w1985:i16[], w1983:i16[], w1982:i16[])  [unwired: 9 out]
    n1446 = To Double Precision Float(number=w2156) -> (double precision float=w2157:dbl[][])
    n1447 = local read "APD Integration Time (s)"() -> (w2026:dbl)
    n1448 = Divide(x=w1986, y=w1985) -> (x/y=w1987:dbl[])
    n1449 = Divide(x=w1983, y=w1982) -> (x/y=w1984:dbl[])
    n1450 = feedback #1(0.0) -> (w2000:dbl)
    n1451 = Add(x=w2088, y=w2000) -> (x+y=w2196:dbl)
    n1452 = feedback-in #1(w2196) -> ()
    n1453 = local read "AOM X Cal (nm/MHz)"() -> (w1953:dbl)
    n1454 = To Time Stamp(1:w2000) -> (0:w1999:timestamp)
    n1455 = Split 1D Array(array=w1987, index="N El. to Ave.") -> (second subarray=w1990:dbl[])  [unwired: 1 out]
    n1456 = Split 1D Array(array=w1984, index="N El. to Ave.") -> (second subarray=w1989:dbl[])  [unwired: 1 out]
    n1457 = local read "Trap X AI1 (DMA)"() -> (w1988:T13)
    n1458 = Multiply(x=w2062, y="Trap Disp. Downsample") -> (x*y=w2001:dbl)
    "Display Period (s)" <- w2001
    n1459 = Bundle("BD 1 Frequency 1 (MHz)"=w1956, "BD 1 Frequency 2 (MHz)"=w1955) -> (w1957:T45)  [unwired: 1 out]
    n1460 = for "Trap AI" {
      tunnel: [w2610] -> w2190 mode=indexing
      tunnel: w1999 -> [w2600]
      tunnel: "Trap Disp. Downsample" -> [w2608]
      tunnel: w2080 -> [w2606] mode=indexing
      tunnel: w2062 -> [w2605]
      tunnel: w2079 -> [w2604] mode=indexing
      tunnel: w1998 -> [w2603]
      tunnel: [w2602] -> w2037 mode=indexing
      tunnel: w2001 -> [w2601]
      n1461 = Bundle By Name("Y"=w2606, "dt"=w2605) -> (w2607:waveform(dbl))  [unwired: 1 out]
      n1462 = Set Waveform Attribute(5:w2604, 6:w2603, 7:w2607) -> (3:w2602:waveform(dbl))  [unwired: 1 in, 2 out]
      n1463 = call "downsample 1D array - double.vi"("Ave N"=w2608, "Array In"=w2606) -> ("Array Out"=w2609:dbl[])  [unwired: 1 out]
      n1464 = Bundle By Name(cluster=w2602, "t0"=w2600, "Y"=w2609, "dt"=w2601) -> (w2610:waveform(dbl))
    }
    n1465 = call-poly <vilib>:"Mean.vi"("X"=w1989) -> ("mean"=w1977:dbl)  [unwired: 1 out]
    n1466 = call-poly <vilib>:"Mean.vi"("X"=w1990) -> ("mean"=w1978:dbl)  [unwired: 1 out]
    n1467 = Cluster To Array(cluster=w1957) -> (array=w1954:dbl[])
    n1468 = Reciprocal(x=w2001) -> (1/x=→"Trap Disp. Freq. (Hz)":dbl)
    n1469 = local read "Data points/scans (MCL)"() -> (w2168:dbl)
    n1470 = To Fixed-Point(number=w1977) -> (fixed-point=w1975:fxp<+/-,16,1>)  [unwired: 1 in]
    n1471 = To Fixed-Point(number=w1978) -> (fixed-point=w1976:fxp<+/-,16,1>)  [unwired: 1 in]
    n1472 = Bundle("Trap 1 Pos.", "Trap 2 Pos.") -> (w1997:cluster{string, string})  [unwired: 1 out]
    n1473 = Bundle By Name(cluster=w1988, "Set 1"=w1976, "Set 2"=w1975) -> (→"Trap X AI1 (DMA)":T13)
    n1474 = Cluster To Array(cluster=w1997) -> (array=w1994:string[])
    n1475 = for "Trap Position" {
      tunnel: w2003 -> [w2250] mode=indexing
      tunnel: "Trap Disp. Downsample" -> [w2249]
      tunnel: w2001 -> [w2247]
      tunnel: w1999 -> [w2246]
      tunnel: w1998 -> [w2244]
      tunnel: w1994 -> [w2243] mode=indexing
      tunnel: [w2242] -> w1952 mode=indexing
      tunnel: w1954 -> [w2240] mode=indexing
      tunnel: w1953 -> [w2238]
      n1476 = call "downsample 1D array - double.vi"("Ave N"=w2249, "Array In"=w2250) -> ("Array Out"=w2248:dbl[])  [unwired: 1 out]
      n1477 = Subtract(x=w2248, y=w2240) -> (x-y=w2241:dbl[])
      n1478 = Multiply(x=w2238, y=w2241) -> (x*y=w2239:dbl[])
      n1479 = Bundle By Name("Y"=w2239, "dt"=w2247, "t0"=w2246) -> (w2245:waveform(dbl))  [unwired: 1 out]
      n1480 = Set Waveform Attribute(5:w2243, 6:w2244, 7:w2245) -> (3:w2242:waveform(dbl))  [unwired: 1 in, 2 out]
    }
    "Trap Positions" <- w1952
    n1481 = Bundle("APD 1", "APD 2") -> (w2189:cluster{string, string})  [unwired: 1 out]
    n1482 = Cluster To Array(cluster=w2189) -> (array=w2186:string[])
    n1483 = for "APD" {
      tunnel: w2157 -> [w2589] mode=indexing
      tunnel: w2026 -> [w2597]
      tunnel: [w2593] -> w2033 mode=indexing
      tunnel: "APD Disp. Scale" -> [w2594]
      tunnel: w1998 -> [w2592]
      tunnel: w2186 -> [w2591] mode=indexing
      tunnel: "APD Disp. Downsample" -> [w2587]
      tunnel: [w2590] -> w2185
      tunnel: w1999 -> [w2586]
      n1484 = call "integrate 1D array interval - double.vi"("Ave N"=w2587, "Array In"=w2589) -> ("Array Out"=w2588:dbl[])  [unwired: 1 out]
      n1485 = Multiply(x=w2597, y=w2587) -> (x*y=w2590:dbl)
      n1486 = Divide(x=w2588, y=w2594) -> (x/y=w2595:dbl[])
      n1487 = Bundle By Name("t0"=w2586, "Y"=w2595, "dt"=w2590) -> (w2596:waveform(dbl))  [unwired: 1 out]
      n1488 = Set Waveform Attribute(5:w2591, 6:w2592, 7:w2596) -> (3:w2593:waveform(dbl))  [unwired: 1 in, 2 out]
    }
    "APD Display Period (s)" <- w2185
    n1489 = Reciprocal(x=w2185) -> (1/x=→"APD Display Freq. (Hz)":dbl)
    n1490 = local read "Display Period (s)"() -> (w2061:dbl)
    n1491 = Increment(x=w2168) -> (x+1=w2169:dbl)
    n1492 = Index Array(array=w1952, index=0) -> (element=w1950:waveform(dbl))
    n1493 = To Double Precision Float(number=w2077) -> (double precision float=w2076:dbl[])
    n1494 = feedback #2(w2169) -> (w2172:dbl)
    n1495 = Select(t=0, s=w2159, f=w2172) -> (s? t:f=w2165:dbl)
    n1496 = Array Size(array=w2076) -> (size(s)=w2171:i32)
    n1497 = Add(x=w2171, y=w2165) -> (x+y=w2166:dbl)
    n1498 = Unbundle By Name(w1950) -> ("Y"=w1948:dbl[])
    n1499 = feedback #3(w2077) -> (w2155:u32[])
    n1500 = Build Array (concatenate)(w2155, w2077) -> (w2152:u32[])
    n1501 = feedback #4(w2013) -> (w2032:u32[])
    n1502 = Divide(x="Bead Sep. Int. Time (s)", y=w2061) -> (x/y=w1946:dbl)
    n1503 = Build Array (concatenate)(w2032, w2013) -> (w2031:u32[])
    n1504 = Greater?(x=w2166, y=w2168) -> (0:w2167:bool)
    n1505 = feedback #5(w1948) -> (w1949:dbl[])
    n1506 = Build Array (concatenate)(w1948, w1949) -> (w1947:dbl[])
    n1507 = Select(t=w2165, s=w2167, f=w2166) -> (s? t:f=w2164:dbl)
    n1508 = feedback-in #2(w2164) -> ()
    n1509 = Array Size(array=w2152) -> (size(s)=w2149:i32)
    n1510 = Array Size(array=w2077) -> (size(s)=w2151:i32)
    n1511 = local read "MCL Scanning"() -> (w2162:bool)
    n1512 = local read "APD Integration Time (s)"() -> (w2040:dbl)
    n1513 = Build Array (concatenate)(w2033, w2190) -> (w2035:waveform(dbl)[])
    "All Signals" <- w2035
    n1514 = Split 1D Array(array=w1947, index=w1946) -> (first subarray=w1940:dbl[])  [unwired: 1 out]
    n1515 = feedback-in #5(w1940) -> ()
    n1516 = Multiply(x=w2151, y="APD Ave N") -> (x*y=w2150:dbl)
    n1517 = Greater?(x=w2149, y=w2150) -> (0:w2153:bool)
    n1518 = Not(x=w2167) -> (.not. x?=w2161:bool)
    n1519 = To Double Precision Float(number=w2013) -> (double precision float=w2012:dbl[])
    n1520 = call-poly <vilib>:"Mean.vi"("X"=w1940) -> ("mean"=w1939:dbl)  [unwired: 1 out]
    "Mean T1 Position (nm)" <- w1939
    n1521 = Subtract(x=w1940, y=w1939) -> (x-y=w1945:dbl[])
    n1522 = Square(x=w1945) -> (x^2=w1944:dbl[])
    n1523 = And(x=w2161, y=w2162) -> (x .and. y?=w2163:bool)
    n1524 = call-poly <vilib>:"Mean.vi"("X"=w1944) -> ("mean"=w1943:dbl)  [unwired: 1 out]
    n1525 = case shown="True" w2153 {
      tunnel: w2152 -> [w2370 w2377]
      tunnel: [w2370 w2375] -> w2093
      tunnel: w2150 -> [_ w2372]
      tunnel: w2149 -> [_ w2376]
      tunnel: w2031 -> [w2369 w2374]
      tunnel: [w2369 w2371] -> w2028
      frame False {
      }
      frame True {
        n1526 = Subtract(x=w2376, y=w2372) -> (x-y=w2373:dbl)
        n1527 = Array Subset(array=w2377, index=w2373, length=w2372) -> (w2375:u32[])
        n1528 = Array Subset(array=w2374, index=w2373, length=w2372) -> (w2371:u32[])
      }
    }
    n1529 = feedback-in #3(w2093) -> ()
    n1530 = feedback-in #4(w2028) -> ()
    n1531 = Or(x=w2163, y=w2159) -> (x .or. y?=w2160:bool)
    n1532 = Square Root(x=w1943) -> (sqrt(x)=w1942:dbl)
    n1533 = Equal?(x="Tab Control 6", y=T35."High Res Display") -> (x = y?=w2083:bool)
    n1534 = Multiply(x="APD Disp. Scale", y=w2033) -> (x*y=w2042:waveform(dbl)[])
    n1535 = Multiply(x="APD Disp. Downsample", y=w2040) -> (x*y=w2038:dbl)
    n1536 = Multiply(x=10.0, y=w1942) -> (x*y=→"Trap 1 Position RMS (A)":dbl)
    n1537 = Divide(x=w2042, y=w2038) -> (x/y=w2010:waveform(dbl)[])
    n1538 = Index Array(array=w2010, index=0) -> (element=w2020:waveform(dbl))
    n1539 = case "For computing FFTs for display" shown="True" "Compute FFT" {
      tunnel: w2037 -> [_ w3047]
      frame False {
      }
      frame True {
        n1540 = Build Array("FFT 1 Choice 1", "FFT 1 Choice 2", "FFT 2 Choice 1", "FFT 2 Choice 2") -> (w3040:u16[])
        n1541 = Array Size(array=w3047) -> (size(s)=w3046:i32)
        n1542 = feedback-in #6(w3040) -> ()
        n1543 = feedback #6(u16[] [100, 100, 100, 100]) -> (w3041:u16[])
        n1544 = feedback-in #7("# Spectra to Ave.") -> ()
        n1545 = feedback #7("# Spectra to Ave.") -> (w3038:dbl)
        n1546 = Not Equal?(x="# Spectra to Ave.", y=w3038) -> (x != y?=w3037:bool)
        n1547 = Not Equal?(x=w3040, y=w3041) -> (x != y?=w3039:bool)
        n1548 = feedback #8(1.0) -> (w3024:dbl)
        n1549 = Compound Arithmetic op=OR("Reset FFT", w3039, w3037) -> (w3022:bool)
        n1550 = Select(t=1.0, s=w3022, f=w3024) -> (s? t:f=w3026:dbl)
        n1551 = Greater?(x=w3026, y="# Spectra to Ave.") -> (0:w3045:bool)
        n1552 = Increment(x=w3026) -> (x+1=w3025:dbl)
        n1553 = feedback-in #8(w3025) -> ()
        n1554 = local read "DMA Update Period (s)"() -> (w3020:dbl)
        n1555 = Multiply(x="# Spectra to Ave.", y=w3020) -> (x*y=→"Ave. Time (s)":dbl)
        n1556 = Build Array(cluster{"f0":dbl, "df":dbl, "magnitude":dbl[]} {"f0"=0.0, "df"=0.0, "magnitude"=[]} ("PSD")) -> (w3029:cluster{"f0":dbl, "df":dbl, "magnitude":dbl[]}[])
        n1557 = Build Array(w3029, w3029, w3029, w3029) -> (w3031:T46)
        n1558 = feedback #9(w3031) -> (w3036:T46)
        n1559 = for {
          N: 4 -> [_]
          tunnel: w3040 -> [w3069] mode=indexing
          tunnel: w3047 -> [w3070]
          tunnel: w3046 -> [w3072]
          tunnel: w3022 -> [w3065]
          tunnel: w3045 -> [w3064]
          tunnel: "# Spectra to Ave." -> [w3063]
          tunnel: [w3062] -> w3035 mode=indexing
          tunnel: w3036 -> [w3067] mode=indexing
          tunnel: [w3066] -> w3023 mode=indexing
          tunnel: w3026 -> [w3061]
          n1560 = Less?(x=w3069, y=w3072) -> (x < y?=w3071:bool)
          n1561 = Index Array(array=w3070, index=w3069) -> (element=w3068:waveform(dbl))
          n1562 = case shown="True" w3071 {
            tunnel: w3068 -> [_ w3089]
            tunnel: w3067 -> [w3074 w3087]
            tunnel: [w3074 w3075] -> w3066
            tunnel: w3065 -> [_ w3086]
            tunnel: w3064 -> [_ w3079]
            tunnel: w3063 -> [_ w3078]
            tunnel: [cluster{"f0":dbl, "df":dbl, "magnitude":dbl[]} {"f0"=0.0, "df"=0.0, "magnitude"=[]} ("PSD") w3080] -> w3062
            tunnel: w3061 -> [_ w3077]
            frame False {
            }
            frame True {
              n1563 = call <vilib>:"Std Deviation and Variance.vi"("X"=w3089) -> ("mean"=w3090:dbl)  [unwired: 1 in, 2 out]
              n1564 = Subtract(x=w3089, y=w3090) -> (x-y=w3088:waveform(dbl))
              n1565 = xnode "Spectral Measurements"("Signals"=w3088) -> ("PSD"=w3082:cluster{"f0":dbl, "df":dbl, "magnitude":dbl[]})  [unwired: 1 in, 1 out]
              n1566 = case shown="False" w3086 {
                tunnel: w3087 -> [w3099 _]
                tunnel: [w3095 w3104] -> w3075
                tunnel: w3082 -> [w3098 w3105]
                tunnel: w3079 -> [w3097 _]
                frame False {
                  n1567 = Build Array (concatenate)(w3099, w3098) -> (w3096:cluster{"f0":dbl, "df":dbl, "magnitude":dbl[]}[])
                  n1568 = case shown="True" w3097 {
                    tunnel: w3096 -> [w3100 w3103]
                    tunnel: [w3100 w3101] -> w3095
                    frame False {
                    }
                    frame True {
                      n1569 = Delete From Array(array=w3103, index=0) -> (array with subset deleted=w3101:cluster{"f0":dbl, "df":dbl, "magnitude":dbl[]}[])  [unwired: 1 in, 1 out]
                    }
                  }
                }
                frame True {
                  n1570 = Build Array(w3105) -> (w3104:cluster{"f0":dbl, "df":dbl, "magnitude":dbl[]}[])
                }
              }
              n1571 = for {
                tunnel: w3075 -> [w3094] mode=indexing
                tunnel: [w3093] -> w3085 mode=indexing
                workers-P: _ -> [_]
                n1572 = Unbundle By Name(w3094) -> ("magnitude"=w3093:dbl[])
              }
              n1573 = Transpose 2D Array(2D array=w3085) -> (transposed array=w3084:dbl[][])
              n1574 = for {
                tunnel: w3084 -> [w3092] mode=indexing
                tunnel: [w3091] -> w3083 mode=indexing
                workers-P: _ -> [_]
                n1575 = Add Array Elements(numeric array=w3092) -> (sum=w3091:dbl)
              }
              n1576 = Select(t=w3078, s=w3079, f=w3077) -> (s? t:f=w3076:dbl)
              n1577 = Divide(x=w3083, y=w3076) -> (x/y=w3081:dbl[])
              n1578 = Bundle By Name(cluster=w3082, "magnitude"=w3081) -> (w3080:cluster{"f0":dbl, "df":dbl, "magnitude":dbl[]})
            }
          }
        }
        n1579 = case shown="True" w3022 {
          tunnel: w3023 -> [w3054 w3060]
          tunnel: [w3054 w3055] -> w3021
          frame False {
          }
          frame True {
            n1580 = Array Subset(array=w3060, index (row)=0 ("index"), length (row)=4 ("length"), index (col)=0 ("index"), length (col)=1 ("length")) -> (w3055:T46)
          }
        }
        n1581 = feedback-in #9(w3021) -> ()
        n1582 = Split 1D Array(array=w3035, index=2) -> (first subarray=→"FFT 1":cluster{"f0":dbl, "df":dbl, "magnitude":dbl[]}[], second subarray=→"FFT 2":cluster{"f0":dbl, "df":dbl, "magnitude":dbl[]}[])
      }
    }
    n1583 = Index Array(array=w2010, index=1) -> (element=w2018:waveform(dbl))
    n1584 = case "For displaying the high resolution display (no downsampling)" shown="True" w2083 {
      tunnel: w2037 -> [_ w2270]
      frame False {
      }
      frame True {
        n1585 = Index Array(array=w2270, index="High Res. Display") -> (element=w2271:waveform(dbl))
        n1586 = call <vilib>:"Std Deviation and Variance.vi"("X"=w2271) -> ("mean"=w2278:dbl, "standard deviation"=w2283:dbl)  [unwired: 1 in, 1 out]
        "Mean Intensity" <- w2278
        "Sigma" <- w2283
        n1587 = Subtract(x=w2271, y=w2278) -> (x-y=w2277:waveform(dbl))
        n1588 = Select(t=w2277, s="Subtract mean", f=w2271) -> (s? t:f=→"1 Channel":waveform(dbl))
        n1589 = Divide(x=w2283, y=w2278) -> (x/y=→"Sigma/Mean":dbl)
        n1590 = feedback #10(1) -> (w2272:i32)
        n1591 = Greater Or Equal?(x=w2272, y="Slow mean N ave.") -> (x >= y?=w2285:bool)
        n1592 = Increment(x=w2272) -> (x+1=w2287:i32)
        n1593 = Select(t=1, s=w2285, f=w2287) -> (s? t:f=w2274:i32)
        n1594 = feedback-in #10(w2274) -> ()
        n1595 = feedback #11() -> (w2275:waveform(dbl))  [unwired: 1 out]
        n1596 = case shown="Default" w2272 {
          tunnel: [w2290 w2293] -> w2276
          tunnel: w2275 -> [w2292 _]
          tunnel: w2271 -> [w2291 w2293]
          frame Default {
            n1597 = call-poly <vilib>:"Append Waveforms.vi"("waveform B"=w2291, "waveform A"=w2292) -> ("waveform out"=w2290:waveform(dbl))  [unwired: 1 in, 8 out]
          }
          frame 1 {
          }
        }
        n1598 = feedback-in #11(w2276) -> ()
        n1599 = case shown="True" w2285 {
          tunnel: w2276 -> [_ w2289]
          frame False {
          }
          frame True {
            n1600 = call-poly <vilib>:"Mean.vi"("X"=w2289) -> ("mean"=→"Slow mean":dbl)  [unwired: 1 out]
          }
        }
      }
    }
    n1601 = case "For plotting results of scanning MCL" shown="True" w2160 {
      tunnel: w2159 -> [_ w2410]
      tunnel: w2076 -> [_ w2506]
      tunnel: w2168 -> [_ _]
      tunnel: w2037 -> [_ w2480]
      tunnel: w2012 -> [_ w2411]
      tunnel: w2011 -> [_ w2384]
      frame False {
      }
      frame True {
        w2391 = u32 0 items=["Horizontal", "Vertical", "Central", "1st Diagonal", "2nd Diagonal"] ("Type of Symmetry")
        w2419 = u32 0 items=["Horizontal", "Vertical", "Central", "1st Diagonal", "2nd Diagonal"] ("Type of Symmetry")
        w2422 = u32 0 items=["Horizontal", "Vertical", "Central", "1st Diagonal", "2nd Diagonal"] ("Type of Symmetry")
        w2451 = u32 0 items=["Horizontal", "Vertical", "Central", "1st Diagonal", "2nd Diagonal"] ("Type of Symmetry")
        n1602 = Index Array(array=w2480, index=10) -> (element=w2486:waveform(dbl))
        n1603 = Index Array(array=w2480, index=11) -> (element=w2483:waveform(dbl))
        n1604 = local read "Cycles/step (MCL)"() -> (w2436:u64)
        n1605 = Index Array(array=w2480, index="Channel") -> (element=w2482:waveform(dbl))
        n1606 = Unbundle(w2384) -> ("New Image"=w2383:T2, "New Image"=w2382:T2, "New Image"=w2381:T2, "New Image"=w2380:T2)
        n1607 = Unbundle By Name(w2486) -> ("Y"=w2438:dbl[])
        n1608 = Unbundle By Name(w2483) -> ("Y"=w2440:dbl[])
        n1609 = Unbundle By Name(w2482) -> ("Y"=w2445:dbl[])
        n1610 = call "downsample 1D array - double.vi"("Ave N"=w2436, "Array In"=w2438) -> ("Array Out"=w2437:dbl[])  [unwired: 1 out]
        n1611 = call "downsample 1D array - double.vi"("Ave N"=w2436, "Array In"=w2440) -> ("Array Out"=w2439:dbl[])  [unwired: 1 out]
        n1612 = call "downsample 1D array - double.vi"("Ave N"=w2436, "Array In"=w2445) -> ("Array Out"=w2444:dbl[])  [unwired: 1 out]
        n1613 = feedback #12(w2506) -> (w2507:dbl[])
        n1614 = Build Array (concatenate)(w2507, w2506) -> (w2488:dbl[])
        n1615 = feedback #13(w2411) -> (w2413:dbl[])
        n1616 = Build Array (concatenate)(w2413, w2411) -> (w2412:dbl[])
        n1617 = local read "Scan steps (MCL)"() -> (w2393:u64)
        n1618 = Select(t=w2506, s=w2410, f=w2488) -> (s? t:f=w2492:dbl[])
        n1619 = feedback-in #12(w2492) -> ()
        n1620 = Select(t=w2411, s=w2410, f=w2412) -> (s? t:f=w2394:dbl[])
        n1621 = feedback-in #13(w2394) -> ()
        n1622 = local read "Scan lines (y)"() -> (w2379:u64)
        n1623 = local read "N APD Samp/step"() -> (w2395:dbl)
        n1624 = feedback #14(w2437) -> (w2494:dbl[])
        n1625 = Build Array (concatenate)(w2494, w2437) -> (w2485:dbl[])
        n1626 = feedback #15(w2444) -> (w2504:dbl[])
        n1627 = Build Array (concatenate)(w2504, w2444) -> (w2503:dbl[])
        n1628 = feedback #16(w2439) -> (w2496:dbl[])
        n1629 = Build Array (concatenate)(w2496, w2439) -> (w2497:dbl[])
        n1630 = Select(t=w2437, s=w2410, f=w2485) -> (s? t:f=w2441:dbl[])
        n1631 = feedback-in #14(w2441) -> ()
        n1632 = Select(t=w2444, s=w2410, f=w2503) -> (s? t:f=w2443:dbl[])
        n1633 = feedback-in #15(w2443) -> ()
        n1634 = Select(t=w2439, s=w2410, f=w2497) -> (s? t:f=w2442:dbl[])
        n1635 = feedback-in #16(w2442) -> ()
        n1636 = Multiply(x=w2393, y=u64 2) -> (x*y=w2378:u64)
        n1637 = call "integrate 1D array interval - double.vi"("Ave N"=w2395, "Array In"=w2394) -> ("Array Out"=w2406:dbl[])  [unwired: 1 out]
        n1638 = call "integrate 1D array interval - double.vi"("Ave N"=w2395, "Array In"=w2492) -> ("Array Out"=w2491:dbl[])  [unwired: 1 out]
        n1639 = Array Size(array=w2406) -> (size(s)=w2407:i32)
        n1640 = Array Size(array=w2491) -> (size(s)=w2493:i32)
        n1641 = Multiply(x=w2379, y=w2378) -> (x*y=w2409:u64)
        n1642 = Multiply(x=w2379, y=w2378) -> (x*y=w2501:u64)
        n1643 = call-poly <vilib>:"Mean.vi"("X"=w2441) -> ("mean"=w2425:dbl)  [unwired: 1 out]
        n1644 = Subtract(x=w2409, y=w2407) -> (x-y=w2400:u64)
        n1645 = call-poly <vilib>:"Mean.vi"("X"=w2443) -> ("mean"=w2430:dbl)  [unwired: 1 out]
        n1646 = call-poly <vilib>:"Mean.vi"("X"=w2442) -> ("mean"=w2428:dbl)  [unwired: 1 out]
        n1647 = call-poly <vilib>:"Mean.vi"("X"=w2406) -> ("mean"=w2397:dbl)  [unwired: 1 out]
        n1648 = Subtract(x=w2501, y=w2493) -> (x-y=w2435:u64)
        n1649 = call-poly <vilib>:"Mean.vi"("X"=w2491) -> ("mean"=w2432:dbl)  [unwired: 1 out]
        n1650 = Initialize Array(1.0 ("element"), w2400) -> (w2396:dbl[])
        n1651 = Initialize Array(1.0 ("element"), w2435) -> (w2426:dbl[])
        n1652 = Multiply(x=w2396, y=w2397) -> (x*y=w2398:dbl[])
        n1653 = Multiply(x=w2426, y=w2428) -> (x*y=w2429:dbl[])
        n1654 = Multiply(x=w2426, y=w2430) -> (x*y=w2431:dbl[])
        n1655 = Multiply(x=w2426, y=w2425) -> (x*y=w2427:dbl[])
        n1656 = Multiply(x=w2426, y=w2432) -> (x*y=w2433:dbl[])
        n1657 = Build Array (concatenate)(w2441, w2427) -> (w2495:dbl[])
        n1658 = Build Array (concatenate)(w2443, w2431) -> (w2499:dbl[])
        n1659 = Build Array (concatenate)(w2442, w2429) -> (w2498:dbl[])
        n1660 = Build Array (concatenate)(w2406, w2398) -> (w2408:dbl[])
        n1661 = Build Array (concatenate)(w2491, w2433) -> (w2500:dbl[])
        n1662 = Reshape Array(w2495, w2379, w2378) -> (w2461:dbl[][])
        n1663 = Reshape Array(w2408, w2379, w2378) -> (w2404:dbl[][])
        n1664 = Reshape Array(w2499, w2379, w2378) -> (w2453:dbl[][])
        n1665 = Reshape Array(w2498, w2379, w2378) -> (w2468:dbl[][])
        n1666 = Reshape Array(w2500, w2379, w2378) -> (w2478:dbl[][])
        n1667 = Array Subset(array=w2468, index (col)=0 ("index"), length (col)=w2393) -> (w2473:dbl[][])  [unwired: 2 in]
        n1668 = Array Subset(array=w2468, index (col)=w2393) -> (w2471:dbl[][])  [unwired: 3 in]
        n1669 = Array Subset(array=w2453, index (col)=0 ("index"), length (col)=w2393) -> (w2459:dbl[][])  [unwired: 2 in]
        n1670 = Array Subset(array=w2453, index (col)=w2393) -> (w2457:dbl[][])  [unwired: 3 in]
        n1671 = Array Subset(array=w2404, index (col)=0 ("index"), length (col)=w2393) -> (w2403:dbl[][])  [unwired: 2 in]
        n1672 = Array Subset(array=w2404, index (col)=w2393) -> (w2401:dbl[][])  [unwired: 3 in]
        n1673 = Array Subset(array=w2478, index (col)=0 ("index"), length (col)=w2393) -> (w2477:dbl[][])  [unwired: 2 in]
        n1674 = Array Subset(array=w2478, index (col)=w2393) -> (w2475:dbl[][])  [unwired: 3 in]
        n1675 = Array Subset(array=w2461, index (col)=0 ("index"), length (col)=w2393) -> (w2466:dbl[][])  [unwired: 2 in]
        n1676 = Array Subset(array=w2461, index (col)=w2393) -> (w2464:dbl[][])  [unwired: 3 in]
        n1677 = for {
          tunnel: w2473 -> [w2515] mode=indexing
          tunnel: [w2514] -> w2472 mode=indexing
          workers-P: _ -> [_]
          n1678 = Reverse 1D Array(array=w2515) -> (reversed array=w2514:dbl[])
        }
        n1679 = for {
          tunnel: w2459 -> [w2511] mode=indexing
          tunnel: [w2510] -> w2458 mode=indexing
          workers-P: _ -> [_]
          n1680 = Reverse 1D Array(array=w2511) -> (reversed array=w2510:dbl[])
        }
        n1681 = for {
          tunnel: w2403 -> [w2509] mode=indexing
          tunnel: [w2508] -> w2402 mode=indexing
          workers-P: _ -> [_]
          n1682 = Reverse 1D Array(array=w2509) -> (reversed array=w2508:dbl[])
        }
        n1683 = for {
          tunnel: w2477 -> [w2517] mode=indexing
          tunnel: [w2516] -> w2476 mode=indexing
          workers-P: _ -> [_]
          n1684 = Reverse 1D Array(array=w2517) -> (reversed array=w2516:dbl[])
        }
        n1685 = for {
          tunnel: w2466 -> [w2513] mode=indexing
          tunnel: [w2512] -> w2465 mode=indexing
          workers-P: _ -> [_]
          n1686 = Reverse 1D Array(array=w2513) -> (reversed array=w2512:dbl[])
        }
        n1687 = Index Array(array=w2478, index (row)=0) -> (element=→"Waveform Graph":dbl[])  [unwired: 1 in]
        n1688 = Add(x=w2472, y=w2471) -> (x+y=w2470:dbl[][])
        n1689 = Add(x=w2458, y=w2457) -> (x+y=w2456:dbl[][])
        n1690 = Add(x=w2402, y=w2401) -> (x+y=w2386:dbl[][])
        n1691 = Add(x=w2476, y=w2475) -> (x+y=w2450:dbl[][])
        n1692 = Add(x=w2465, y=w2464) -> (x+y=w2463:dbl[][])
        n1693 = Divide(x=w2456, y=2) -> (x/y=w2454:dbl[][])
        n1694 = Divide(x=w2470, y=2) -> (x/y=w2415:dbl[][])
        n1695 = Divide(x=w2463, y=2) -> (x/y=w2417:dbl[][])
        n1696 = To Single Precision Float(number=w2450) -> (single precision float=w2449:sgl[][])
        n1697 = Transpose 2D Array(2D array=w2454) -> (transposed array=→"Data map":dbl[][])
        n1698 = To Single Precision Float(number=w2386) -> (single precision float=w2390:sgl[][])
        n1699 = To Single Precision Float(number=w2415) -> (single precision float=w2421:sgl[][])
        n1700 = To Single Precision Float(number=w2417) -> (single precision float=w2418:sgl[][])
        n1701 = call "IMAQ ArrayToImage"("Image Pixels (Float)"=w2449, "Image"=w2383) -> ("Image Out"=w2452:T2)  [unwired: 8 in, 1 out]
        n1702 = call "IMAQ ArrayToImage"("Image Pixels (Float)"=w2390, "Image"=w2382) -> ("Image Out"=w2392:T2)  [unwired: 8 in, 1 out]
        n1703 = call "IMAQ ArrayToImage"("Image Pixels (Float)"=w2421, "Image"=w2381) -> ("Image Out"=w2423:T2)  [unwired: 8 in, 1 out]
        n1704 = call "IMAQ ArrayToImage"("Image Pixels (Float)"=w2418, "Image"=w2380) -> ("Image Out"=w2420:T2)  [unwired: 8 in, 1 out]
        n1705 = call "IMAQ Symmetry"("Type of Symmetry"=w2451, "Image Src"=w2452) -> ("Image Dst Out"=w2447:T2)  [unwired: 3 in, 1 out]
        n1706 = call "IMAQ Symmetry"("Type of Symmetry"=w2391, "Image Src"=w2392) -> ("Image Dst Out"=w2388:T2)  [unwired: 3 in, 1 out]
        n1707 = call "IMAQ Symmetry"("Type of Symmetry"=w2422, "Image Src"=w2423) -> ("Image Dst Out"=→"Detection Laser X":T2)  [unwired: 3 in, 1 out]
        n1708 = call "IMAQ Symmetry"("Type of Symmetry"=w2419, "Image Src"=w2420) -> ("Image Dst Out"=→"Detection Laser Y":T2)  [unwired: 3 in, 1 out]
        n1709 = call "IMAQ Set Simple Calibration"("Calibration Axis Info"=T36 {"Origin Pixel"={"X"=0.0, "Y"=0.0}, "Angle Relative to Horizontal (deg)"=0.0, "Axis Reference"=0}, "Grid Descriptor"=T37 {"X Step"=0.3, "Y Step"=0.3, "Unit"=enum."Undefined"}, "Image"=w2447) -> ("Calibrated Image"=→"APD 1":T2)  [unwired: 7 in, 1 out]
        n1710 = call "IMAQ Set Simple Calibration"("Calibration Axis Info"=T36 {"Origin Pixel"={"X"=0.0, "Y"=0.0}, "Angle Relative to Horizontal (deg)"=0.0, "Axis Reference"=0}, "Grid Descriptor"=T37 {"X Step"=0.3, "Y Step"=0.3, "Unit"=enum."Undefined"}, "Image"=w2388) -> ("Calibrated Image"=→"APD 2":T2)  [unwired: 7 in, 1 out]
      }
    }
    n1711 = Subtract(x=w2018, y="APD 2 Offset") -> (x-y=w2015:waveform(dbl))
    n1712 = Subtract(x=w2020, y="APD 1 Offset") -> (x-y=w2016:waveform(dbl))
    n1713 = Index Array(array=w2035, index=3) -> (element=w2104:waveform(dbl))
    n1714 = Index Array(array=w2035, index=6) -> (element=w2101:waveform(dbl))
    n1715 = Build Array(w2016, w2015) -> (→"APD Chart":waveform(dbl)[])
    n1716 = Array Size(array=w2093) -> (size(s)=w2148:i32)
    n1717 = call <vilib>:"Std Deviation and Variance.vi"("X"=w2028) -> ("standard deviation"=w2027:dbl)  [unwired: 1 in, 2 out]
    n1718 = Add Array Elements(numeric array=w2028) -> (sum=w2030:u32)
    n1719 = Add Array Elements(numeric array=w2093) -> (sum=w2158:u32)
    n1720 = call <vilib>:"Std Deviation and Variance.vi"("X"=w2093) -> ("standard deviation"=w2092:dbl)  [unwired: 1 in, 2 out]
    n1721 = Divide(x="T1 offset_x (mV)", y=1000.0) -> (x/y=w2105:dbl)
    n1722 = Divide(x=w2027, y=w2026) -> (x/y=w2023:dbl)
    "Rate sigma (Hz) 2" <- w2023
    n1723 = Multiply(x=w2026, y=w2148) -> (x*y=w2029:dbl)
    "Int. Time (s)" <- w2029
    n1724 = Divide(x=w2030, y=w2029) -> (x/y=w2024:dbl)
    "APD 2 Rate (Hz)" <- w2024
    n1725 = Divide(x=w2158, y=w2029) -> (x/y=w2090:dbl)
    "APD 1 Rate (Hz)" <- w2090
    n1726 = Divide(x=w2092, y=w2026) -> (x/y=w2091:dbl)
    "Rate sigma (Hz)" <- w2091
    n1727 = Divide(x=w2023, y=w2024) -> (x/y=→"Sigma/Mean 2":dbl)
    n1728 = Divide(x=w2091, y=w2090) -> (x/y=→"Sigma/Mean":dbl)
    n1729 = Divide(x="T2 offset_x (mV)", y=1000.0) -> (x/y=w2103:dbl)
    n1730 = case shown="1" "Calibration" {
      tunnel: "T1 alpha_x (nm/V)" -> [_ w2346 w2367]
      tunnel: "T1 kappa_x (pN/nm)" -> [_ _ w2357]
      tunnel: "T2 alpha_x (nm/V)" -> [_ w2345 w2365]
      tunnel: "T2 kappa_x (pN/nm)" -> [_ _ w2358]
      tunnel: w2104 -> [w2328 w2343 w2363]
      tunnel: w2101 -> [w2327 w2341 w2361]
      tunnel: [w2328 w2340 w2360] -> w2134
      tunnel: [w2327 w2339 w2359] -> w2133
      tunnel: ["T1 X (V)" ("Label.Text") "T1 X (nm)" ("Label.Text") "T1 X (pN)" ("Label.Text")] -> w2122
      tunnel: ["T2 X (V)" ("Label.Text") "T2 X (nm)" ("Label.Text") "T2 X (pN)" ("Label.Text")] -> w2121
      tunnel: ["Position (V)" ("Label.Text") "Position (nm)" ("Label.Text") "Force (pN)" ("Label.Text")] -> w2123
      tunnel: w2103 -> [_ w2331 w2350]
      tunnel: w2105 -> [_ w2334 w2352]
      tunnel: ["Mean (V)" ("Label.Text") "Mean (nm)" ("Label.Text") "Mean (pN)" ("Label.Text")] -> w2118
      tunnel: ["Difference (V)" ("Label.Text") "Difference (nm)" ("Label.Text") "Difference (pN)" ("Label.Text")] -> w2043
      frame 0, Default {
      }
      frame 1 {
        # "position"
        n1731 = Unbundle By Name(w2343) -> ("Y"=w2347:dbl[])
        n1732 = Unbundle By Name(w2341) -> ("Y"=w2332:dbl[])
        n1733 = Subtract(x=w2347, y=w2334) -> (x-y=w2335:dbl[])
        n1734 = Subtract(x=w2332, y=w2331) -> (x-y=w2333:dbl[])
        n1735 = Multiply(x=w2333, y=w2345) -> (x*y=w2342:dbl[])
        n1736 = Multiply(x=w2346, y=w2335) -> (x*y=w2344:dbl[])
        n1737 = Bundle By Name(cluster=w2341, "Y"=w2342) -> (w2339:waveform(dbl))
        n1738 = Bundle By Name(cluster=w2343, "Y"=w2344) -> (w2340:waveform(dbl))
      }
      frame 2 {
        # "force"
        n1739 = Unbundle By Name(w2363) -> ("Y"=w2368:dbl[])
        n1740 = Unbundle By Name(w2361) -> ("Y"=w2366:dbl[])
        n1741 = Subtract(x=w2366, y=w2350) -> (x-y=w2351:dbl[])
        n1742 = Subtract(x=w2368, y=w2352) -> (x-y=w2353:dbl[])
        n1743 = Compound Arithmetic op=MULTIPLY(w2351, w2365, w2358) -> (w2362:dbl[])
        n1744 = Compound Arithmetic op=MULTIPLY(w2357, w2367, w2353) -> (w2364:dbl[])
        n1745 = Bundle By Name(cluster=w2361, "Y"=w2362) -> (w2359:waveform(dbl))
        n1746 = Bundle By Name(cluster=w2363, "Y"=w2364) -> (w2360:waveform(dbl))
      }
    }
    n1747 = feedback-in #17("Calibration") -> ()
    n1748 = feedback #17(u16 1 ("Calibration")) -> (w2125:u16)
    n1749 = Not Equal?(x=w2125, y="Calibration") -> (x != y?=w2081:bool)
    n1750 = Unbundle By Name(w2104) -> ("Y"=w2107:dbl[])
    n1751 = Unbundle By Name(w2101) -> ("Y"=w2110:dbl[])
    n1752 = Subtract(x=w2107, y=w2105) -> (x-y=w2108:dbl[])
    n1753 = Subtract(x=w2110, y=w2103) -> (x-y=w2109:dbl[])
    n1754 = disable-structure shown="Enabled" {
      disable-tunnel: [-1.0 ("y") 1.0] -> w2111
      frame Disabled {
      }
      frame Enabled {
      }
    }
    n1755 = Multiply(x=w2109, y="T2 alpha_x (nm/V)") -> (x*y=w2100:dbl[])
    n1756 = Multiply(x="T1 alpha_x (nm/V)", y=w2108) -> (x*y=w2099:dbl[])
    n1757 = Multiply(x=w2133, y=w2111) -> (x*y=w2112:waveform(dbl))
    n1758 = case shown="False" "Read Lateness and Rel Phase" {
      tunnel: w1935 -> [w2294 w2316]
      tunnel: w1934 -> [w2295 w2315]
      tunnel: [w2294 w2314] -> w2096
      tunnel: [w2295 w2313] -> w2095
      frame False {
      }
      frame True {
        n1759 = xnode "Read/Write Control"("FPGA VI Reference In"=w2316, "error in"=w2315) -> ("FPGA VI Reference Out"=w2314:T19, "error out"=w2313:errorcluster, "GI Relative phase"=→"GI relative phase":i16, "Relative phase"=→"Relative phase (AI1)":i16, "AI Late Counter"=→"Late Counter (AI1)":u16, "GI Late Counter"=→"GI Late Counter":u16, "MCL Late Counter"=→"MCL Late Counter":u16, "MCL Relative Phase"=→"Relative Phase (MCL)":i16, "APD Acq Relative Phase"=→"APD Acq Relative Phase":i16, "APD 1 Gate Relative Phase"=→"APD 1 Gate Relative Phase":i16, "APD 2 Gate Relative Phase"=→"APD 2 Gate Relative Phase":i16, "APD Acq Late Counter"=→"APD Acq Late Counter":u16, "APD 1 Gate Late Counter"=→"APD 1 Gate Late Counter":u16, "APD 2 Gate Late Counter"=→"APD 2 Gate Late Counter":u16, "Green FB Relative Phase"=→"Relative phase (Green FB)":i16, "GI Relative phase 2"=→"GI relative phase 2":i16, "GI Late Counter 2"=→"GI Late Counter 2":u16, "Trap Pos FIFO Timeout"=→"Trap Pos FIFO Timeout":u16, "Trap AI FIFO Timeout"=→"Trap AI FIFO Timeout":u16)
      }
    }
    n1760 = Subtract(x=w2100, y=w2099) -> (x-y=w2098:dbl[])
    n1761 = Unbundle By Name(w2133) -> ("Y"=w2068:dbl[])
    n1762 = Unbundle By Name(w2134) -> ("Y"=w2069:dbl[])
    n1763 = Build Array(w2134, w2112) -> (→"Force":waveform(dbl)[])
    n1764 = Subtract(x=w2098, y="Offset (nm)") -> (x-y=w2066:dbl[])
    n1765 = call-poly <vilib>:"Mean.vi"("X"=w2068) -> ("mean"=w2047:dbl)  [unwired: 1 out]
    "T2 X" <- w2047
    n1766 = Absolute Value(x=w2069) -> (abs(x)=w2070:dbl[])
    n1767 = Absolute Value(x=w2068) -> (abs(x)=w2071:dbl[])
    n1768 = call-poly <vilib>:"Mean.vi"("X"=w2069) -> ("mean"=w2048:dbl)  [unwired: 1 out]
    "T1 X" <- w2048
    n1769 = Add(x=w2070, y=w2071) -> (x+y=w2072:dbl[])
    n1770 = Bundle By Name(cluster=w2104, "Y"=w2066) -> (w2034:waveform(dbl))
    "Bead Separation" <- w2034
    n1771 = Divide(x=w2072, y=2.0) -> (x/y=→"Vec Mean of T1 T2":dbl[])
    n1772 = case shown="True" w2081 {
      tunnel: w2123 -> [_ w2321]
      tunnel: w2122 -> [_ w2320]
      tunnel: w2121 -> [_ w2319]
      tunnel: w2118 -> [_ w2318]
      tunnel: w2043 -> [_ w2317]
      frame False {
      }
      frame True {
        n1773 = property on="Force" class="WFChart (strict)"("YScale.NameLbl.Text"=w2321) -> ()  [unwired: 2 in, 2 out]
        n1774 = property on="T2 X" class="DigNum (strict)"("Caption.Text"=w2319) -> ()  [unwired: 2 in, 2 out]
        n1775 = property on="T1 X" class="DigNum (strict)"("Caption.Text"=w2320) -> ()  [unwired: 2 in, 2 out]
        n1776 = property on="Mean" class="DigNum (strict)"("Caption.Text"=w2318) -> ()  [unwired: 2 in, 2 out]
        n1777 = property on="Difference" class="DigNum (strict)"("Caption.Text"=w2317) -> ()  [unwired: 2 in, 2 out]
      }
    }
    n1778 = local read "Tether"() -> (w2075:bool)
    n1779 = Absolute Value(x=w2048) -> (abs(x)=w2045:dbl)
    n1780 = Absolute Value(x=w2047) -> (abs(x)=w2044:dbl)
    n1781 = Add(x=w2045, y=w2044) -> (x+y=w2120:dbl)
    n1782 = Subtract(x=w2045, y=w2044) -> (x-y=→"Difference":dbl)
    n1783 = feedback #18(w2066) -> (w2065:dbl[])
    n1784 = Divide(x=w2120, y=2.0) -> (x/y=w2074:dbl)
    "Mean" <- w2074
    n1785 = case shown="True" w2075 {
      tunnel: w2074 -> [_ w2253]
      frame False {
      }
      frame True {
        n1786 = Greater?(x="Lost Tether Alarm Threshold (pN)", y=w2253) -> (0:w2251:bool)
        n1787 = case shown="True" w2251 {
          frame False {
          }
          frame True {
            n1788 = flat-sequence {
              frame #0 {
                # "stop only if saving"
                n1789 = local read "Saving..."() -> (w2266:bool)
                n1790 = And(x=w2266, y="TA Cancel Save?") -> (x .and. y?=w2265:bool)
                n1791 = local write "Stop Saving"(w2265) -> ()
              }
              frame #1 {
                n1792 = case shown="True" "TA Green Off?" {
                  frame False {
                  }
                  frame True {
                    w2269 = FALSE ("Fl. Triggered...")
                    n1793 = local write "Fl. Triggered..."(w2269) -> ()
                    n1794 = property on="Green Laser ON/Interlacing" class="Bool (strict)"("Val(Sgnl)"=w2269) -> ()  [unwired: 2 in, 2 out]
                  }
                }
              }
            }
            n1795 = local read "Time tether formed"() -> (w2260:timestamp)
            n1796 = Get Date/Time In Seconds() -> (seconds since 1Jan1904=w2261:timestamp)
            n1797 = Subtract(x=w2261, y=w2260) -> (x-y=w2259:dbl)
            n1798 = Number To Decimal String(number=w2259) -> (decimal integer string=w2256:string)  [unwired: 1 out]
            n1799 = local read "Messages"() -> (w2263:string)
            n1800 = call <vilib>:"Beep.vi"() -> ()  [unwired: 3 in, 9 out]
            n1801 = Concatenate Strings("Lost tether (" ("Message to add"), w2256, " s)." ("string")) -> (w2258:string)
            n1802 = local write "Tether"(FALSE ("Tether")) -> ()
            n1803 = call "Update messages.vi"("Message to add"=w2258, "Old message string"=w2263) -> ("New message string"=w2262:string)
            n1804 = local write "Messages"(w2262) -> ()
            n1805 = property on="Trap Pos. FB ON" class="Bool (strict)"("Val(Sgnl)"=FALSE ("Value (Signaling)")) -> ()  [unwired: 2 in, 2 out]
          }
        }
      }
    }
    n1806 = Build Array (concatenate)(w2066, w2065) -> (w2064:dbl[])
    n1807 = Split 1D Array(array=w2064, index=w1946) -> (first subarray=w2060:dbl[])  [unwired: 1 out]
    n1808 = feedback-in #18(w2060) -> ()
    n1809 = call-poly <vilib>:"Mean.vi"("X"=w2060) -> ("mean"=w2059:dbl)  [unwired: 1 out]
    "Bead Mean (nm)" <- w2059
    n1810 = Subtract(x=w2060, y=w2059) -> (x-y=w2058:dbl[])
    n1811 = Square(x=w2058) -> (x^2=w2057:dbl[])
    n1812 = call-poly <vilib>:"Mean.vi"("X"=w2057) -> ("mean"=w2056:dbl)  [unwired: 1 out]
    n1813 = Square Root(x=w2056) -> (sqrt(x)=w2055:dbl)
    n1814 = Multiply(x=10.0, y=w2055) -> (x*y=→"RMS (Ang)":dbl)
    n1815 = xnode "Read/Write Control"("FPGA VI Reference In"=w2096, "error in"=w2095) -> ("FPGA VI Reference Out"=w2214:T19, "error out"=w2208:errorcluster, "AI2 Y Sum Set 1"=w2204:i16, "AI2 Y Sum Set 2"=w2203:i16, "AI1 X Set 1"=w1980:fxp<+/-,16,1>, "AI1 X Set 2"=w1979:fxp<+/-,16,1>, "Trap Pos FB Int Signal"=→"Trap Pos FB Int Signal":fxp<+/-,24,9>, "Trap Pos FB Int-Norm Signal"=→"Trap Pos FB Int-Norm Signal":fxp<+/-,16,1>, "Trap Pos FB Action"=w1973:i64, "Scanning"=→"AOD Scanning":bool, "Scan I"=→"AOD Scan I":u64, "Scanning MCL"=w2206:bool, "Scan I (MCL)"=→"MCL Scan I":u64, "Green FB Signals"=w2143:T47)  [unwired: 1 out]
    "MCL Scanning" <- w2206
    "Trap Pos FB Action" <- w1973
    n1816 = local read "AI2 (V)"() -> (w2205:cluster{"Set 1":dbl, "Set 2":dbl})
    n1817 = Bundle By Name(cluster=w2205, "Set 1"=w2204, "Set 2"=w2203) -> (w2201:cluster{"Set 1":dbl, "Set 2":dbl})
    n1818 = Divide(x=w1973, y=327.67) -> (x/y=→"Action (%)":dbl)
    n1819 = local read "Trap X (AI1)"() -> (w1993:T10)
    n1820 = Divide(x=w2201, y=3276.7) -> (x/y=w2200:cluster{"Set 1":dbl, "Set 2":dbl})
    n1821 = local write "AI2 (V)"(w2200) -> ()
    n1822 = Bundle(cluster=w1993, "Trap 1"=w1980, "Trap 2"=w1979) -> (→"Trap X (AI1)":T10)
    n1823 = Divide(x=w2143, y=3276.7) -> (x/y=w2139:T48)
    n1824 = Unbundle By Name(w2139) -> ("Green FB Ch 0"=w2142:dbl, "Green FB Ch 1"=w2141:dbl, "Green FB Ch 2"=w2140:dbl)
    n1825 = Divide(x=w2142, y=w2140) -> (x/y=w2138:dbl)
    n1826 = Divide(x=w2141, y=w2140) -> (x/y=w2137:dbl)
    n1827 = flat-sequence "To save data" {
      tunnel: [w3143] -> w2225
      tunnel: [w3144] -> w2224
      tunnel: w2174 -> [w3137]
      tunnel: w2062 -> [w3141]
      tunnel: ["Save Calibration"] -> w2197
      tunnel: w2194 -> [w3140]
      tunnel: [w3133] -> w2193
      tunnel: [w3130] -> w2192
      tunnel: [w3127] -> w2191
      tunnel: w2173 -> [w3129]
      tunnel: w2079 -> [w3123]
      tunnel: [w3123] -> w2078
      tunnel: ["Start Saving"] -> w2036
      tunnel: [w3117] -> w1962
      tunnel: [w3116] -> w1961
      tunnel: w2225 -> [w3378]
      tunnel: w2224 -> [w3377]
      tunnel: w1963 -> [w3376]
      tunnel: w2197 -> [w3375]
      tunnel: w2193 -> [w3373]
      tunnel: w2192 -> [w3372]
      tunnel: w2191 -> [w3371]
      tunnel: w2049 -> [w3370]
      tunnel: w2088 -> [w3369]
      tunnel: w2078 -> [w3368]
      tunnel: w2036 -> [w3367]
      tunnel: w2034 -> [w3366]
      tunnel: w2010 -> [w3365]
      tunnel: w1962 -> [w3364]
      tunnel: w1961 -> [w3363]
      tunnel: w1960 -> [w3362]
      frame #0 {
        n1828 = Or(x="Save N Sets", y="Start Saving") -> (x .or. y?=w3124:bool)
        n1829 = To Double Precision Float(number=w3140) -> (double precision float=w3134:dbl)
        n1830 = Build Array(w3124, "Save Calibration", w3137, w3129) -> (w3139:bool[])
        n1831 = Compound Arithmetic op=OR("Save Calibration", w3137, w3124, w3129) -> (w3142:bool)
        n1832 = Boolean Array To Number(Boolean array=w3139) -> (number=w3136:u32)
        n1833 = feedback #19(FALSE ("Save APD Data\nwith Trap Data")) -> (w3118:bool)
        n1834 = feedback #20(refnum<k0> refnum) -> (w3145:refnum<file>)
        n1835 = feedback #21(refnum<k0> refnum) -> (w3120:refnum<file>)
        n1836 = feedback #22(FALSE ("Save APD Data\nwith Trap Data")) -> (w3128:bool)
        n1837 = feedback #23(refnum<k0> refnum) -> (w3131:refnum<file>)
        n1838 = feedback #24(0) -> (w3147:i32)
        n1839 = feedback #25() -> (w3135:u32)  [unwired: 1 out]
        n1840 = case shown="True" w3142 {
          tunnel: [w3154 1] -> w3143
          tunnel: w3147 -> [w3156 _]
          tunnel: [w3155 w3174] -> w3144
          tunnel: w3145 -> [w3155 _]
          tunnel: w3141 -> [_ w3194]
          tunnel: w3134 -> [_ w3192]
          tunnel: w3136 -> [_ w3195]
          tunnel: [w3153 w3173] -> w3133
          tunnel: w3135 -> [w3153 _]
          tunnel: [w3152 w3171] -> w3130
          tunnel: w3131 -> [w3152 _]
          tunnel: [w3151 w3170] -> w3127
          tunnel: w3128 -> [w3151 _]
          tunnel: "Start Saving" -> [_ w3168]
          tunnel: w3123 -> [_ w3167]
          tunnel: [w3150 w3158] -> w3116
          tunnel: w3120 -> [w3150 _]
          tunnel: [w3149 w3157] -> w3117
          tunnel: w3118 -> [w3149 _]
          frame False {
            n1841 = Increment(x=w3156) -> (x+1=w3154:i32)
          }
          frame True {
            w3164 = FALSE ("Start Saving")
            w3169 = 9.0  # File Version
            w3177 = FALSE ("prepend array or string size? (T)")
            w3175 = T29."big-endian, network order" ("byte order (0:big-endian, network order)")
            # "write file headers"
            n1842 = local read "BD 1 Frequency 1 (MHz)"() -> (w3191:dbl)
            n1843 = local read "BD 2 Frequency 1 (MHz)"() -> (w3190:dbl)
            n1844 = local read "BD 1 Frequency 2 (MHz)"() -> (w3189:dbl)
            n1845 = local read "BD 2 Frequency 2 (MHz)"() -> (w3188:dbl)
            n1846 = local read "BD 1 Frequency 3 (MHz)"() -> (w3187:dbl)
            n1847 = local read "BD 2 Frequency 3 (MHz)"() -> (w3186:dbl)
            n1848 = Array Size(array=w3167) -> (size(s)=w3166:i32)
            n1849 = To Double Precision Float(number=w3166) -> (double precision float=w3165:dbl)
            n1850 = local write "Save Calibration"(w3164) -> ()
            n1851 = local write "Start Saving"(w3164) -> ()
            n1852 = Build Array("Save APD Data\nwith Trap Data", "Save Trap Pos. Data") -> (w3161:bool[])
            n1853 = Boolean Array To Number(Boolean array=w3161) -> (number=w3160:u32)
            n1854 = Build Array(w3191, w3190, w3189, w3188, w3187, w3186) -> (w3185:dbl[])
            n1855 = case shown="4" w3195 {
              tunnel: w3194 -> [w3266 w3286 w3302 w3340]
              tunnel: w3165 -> [w3271 w3293 w3322 w3359]
              tunnel: w3192 -> [w3270 w3292 w3321 w3358]
              tunnel: [w3267 w3288 w3313 w3350] -> w3183
              tunnel: [w3258 "Cal sets to save" w3303 w3341] -> w3173
              tunnel: w3185 -> [w3268 w3289 w3315 w3352]
              tunnel: "Save APD Data\nwith Trap Data" -> [w3265 _ w3299 w3338]
              tunnel: [w3265 w3280 w3299 w3338] -> w3170
              tunnel: w3169 -> [w3261 w3281 w3297 w3336]
              tunnel: w3168 -> [w3260 _ _ _]
              tunnel: [w3251 w3280 w3296 w3326] -> w3157
              tunnel: "Save Trap Pos. Data" -> [w3251 _ w3296 w3326]
              tunnel: w3160 -> [w3250 _ w3295 w3325]
              frame 1, Default {
                # "timeseries"
                n1856 = case shown="True" "Profile" {
                  tunnel: [w3274 w3277] -> w3255
                  tunnel: [w3274 w3276] -> w3254
                  tunnel: [w3274 w3275] -> w3253
                  tunnel: [w3274 w3279] -> w3252
                  frame False {
                    w3274 = 0.0 ("f")
                  }
                  frame True {
                    n1857 = local read "Current Position"() -> (w3278:dbl[])
                    n1858 = local read "Y change (mm)"() -> (w3279:dbl)
                    n1859 = call "subVI_explode3array.vi"("Array"=w3278) -> ("x"=w3277:dbl, "y"=w3276:dbl, "z"=w3275:dbl)  [unwired: 12 in]
                  }
                }
                n1860 = local read "Save ave N"() -> (w3273:dbl)
                n1861 = Multiply(x=w3273, y=w3266) -> (x*y=w3272:dbl)
                n1862 = To Double Precision Float(number=w3250) -> (double precision float=w3264:dbl)
                n1863 = Build Array(w3261, w3266, w3272, w3271, w3270, 0.0 ("f")) -> (w3269:dbl[])
                n1864 = Build Array(w3264, w3255, w3254, w3253, w3252) -> (w3262:dbl[])
                n1865 = Select(t=u32 4000000000, s=w3260, f="N sets to save") -> (s? t:f=w3258:u32)
                n1866 = Build Array (concatenate)(w3269, w3268, w3262) -> (w3267:dbl[])
              }
              frame 2 {
                w3283 = 0.0 ("f")
                w3280 = FALSE ("Save APD Data\nwith Trap Data")
                # "calibration"
                n1867 = Boolean To (0,1)(Boolean=w3280) -> (0, 1=w3285:i16)
                n1868 = To Double Precision Float(number=w3285) -> (double precision float=w3284:dbl)
                n1869 = Build Array(w3284, w3283, w3283, w3283, w3283) -> (w3282:dbl[])
                n1870 = Build Array(w3281, w3286, w3286, w3293, w3292, 1.0 ("t")) -> (w3290:dbl[])
                n1871 = Build Array (concatenate)(w3290, w3289, w3282) -> (w3288:dbl[])
                "Calibrating Trap..." <- TRUE ("Calibrating...")
              }
              frame 4 {
                w3300 = 0.0 ("f")
                # "write file header for a trap \nraster scan"
                # "scan dir (x/y = 0/1)"
                # "cycles/step"
                # "n scans (f/b)"
                # "steps"
                # "freq. range"
                # "AOD raster scan"
                n1872 = local read "Number of F/B Scans (AOD)"() -> (w3307:u16)
                n1873 = local read "Cycles/step (AOD)"() -> (w3309:u64)
                n1874 = local read "Scan Range (MHz)"() -> (w3312:dbl)
                n1875 = local read "Scan steps (AOD)"() -> (w3311:u64)
                n1876 = local read "Scan BD"() -> (w3319:bool)
                n1877 = local read "Save ave N"() -> (w3324:dbl)
                n1878 = Boolean To (0,1)(Boolean=w3319) -> (0, 1=w3318:i16)
                n1879 = To Double Precision Float(number=w3307) -> (double precision float=w3306:dbl)
                n1880 = To Double Precision Float(number=w3311) -> (double precision float=w3310:dbl)
                n1881 = To Double Precision Float(number=w3309) -> (double precision float=w3308:dbl)
                n1882 = To Double Precision Float(number=w3318) -> (double precision float=w3317:dbl)
                n1883 = Multiply(x=w3324, y=w3302) -> (x*y=w3323:dbl)
                n1884 = To Double Precision Float(number=w3295) -> (double precision float=w3301:dbl)
                n1885 = Build Array(w3301, w3300, w3300, w3300, w3300) -> (w3298:dbl[])
                n1886 = local read "N sets should be saved"() -> (w3304:dbl)
                n1887 = Build Array(w3317, w3312, w3310, w3308, w3306) -> (w3314:dbl[])
                n1888 = Build Array(w3297, w3302, w3323, w3322, w3321, 2.0 ("t")) -> (w3316:dbl[])
                n1889 = Round Toward +Infinity(x=w3304) -> (ceil(x): smallest int >= x=w3305:dbl)
                n1890 = Build Array (concatenate)(w3316, w3315, w3298, w3314) -> (w3313:dbl[])
                n1891 = To Unsigned Long Integer(number=w3305) -> (unsigned 32bit integer=w3303:u32)
              }
              frame 8 {
                w3333 = 0.0 ("f")
                # "MCL raster scan"
                n1892 = local read "Number of scans (MCL)"() -> (w3328:u64)
                n1893 = local read "Scan lines (y)"() -> (w3327:u64)
                n1894 = local read "2D or 1D Scan"() -> (w3330:bool)
                n1895 = local read "Scan Range (V)\n(of steps)"() -> (w3349:dbl)
                n1896 = local read "Fast Scan Dir"() -> (w3356:bool)
                n1897 = local read "Cycles/step (MCL)"() -> (w3346:u64)
                n1898 = local read "Scan steps (MCL)"() -> (w3348:u64)
                n1899 = Select(t=w3327, s=w3330, f=w3328) -> (s? t:f=w3329:u64)
                n1900 = Boolean To (0,1)(Boolean=w3330) -> (0, 1=w3332:i16)
                n1901 = local read "Save ave N"() -> (w3361:dbl)
                n1902 = local read "Initial X"() -> (w3335:dbl)
                n1903 = local read "Initial Y"() -> (w3334:dbl)
                n1904 = To Double Precision Float(number=w3332) -> (double precision float=w3331:dbl)
                n1905 = Boolean To (0,1)(Boolean=w3356) -> (0, 1=w3355:i16)
                n1906 = To Double Precision Float(number=w3329) -> (double precision float=w3344:dbl)
                n1907 = To Double Precision Float(number=w3348) -> (double precision float=w3347:dbl)
                n1908 = To Double Precision Float(number=w3346) -> (double precision float=w3345:dbl)
                n1909 = To Double Precision Float(number=w3355) -> (double precision float=w3354:dbl)
                n1910 = Multiply(x=w3361, y=w3340) -> (x*y=w3360:dbl)
                n1911 = To Double Precision Float(number=w3325) -> (double precision float=w3339:dbl)
                n1912 = local read "N sets should be saved (MCL)"() -> (w3342:dbl)
                n1913 = Build Array(w3339, w3331, w3333, w3333, w3333) -> (w3337:dbl[])
                n1914 = Build Array(w3354, w3349, w3347, w3345, w3344, w3335, w3334) -> (w3351:dbl[])
                n1915 = Build Array(w3336, w3340, w3360, w3359, w3358, 3.0 ("t")) -> (w3353:dbl[])
                n1916 = Round Toward +Infinity(x=w3342) -> (ceil(x): smallest int >= x=w3343:dbl)
                n1917 = Build Array (concatenate)(w3353, w3352, w3337, w3351) -> (w3350:dbl[])
                n1918 = To Unsigned Long Integer(number=w3343) -> (unsigned 32bit integer=w3341:u32)
              }
            }
            n1919 = local read "Index"() -> (w3200:dbl)
            n1920 = call "Create new save file.vi"("Insert"="", "Ext"=".dat", "Index In"=w3200) -> ("Path Out"=w3159:path, "Index Out"=w3172:dbl)
            n1921 = local write "Save file name"(w3159) -> ()
            n1922 = local write "Index"(w3172) -> ()
            n1923 = local write "Save index"(w3172) -> ()
            n1924 = Array Size(array=w3183) -> (size(s)=w3184:i32)
            n1925 = Open/Create/Replace File(file path (use dialog)=w3159, operation (0:open)=T23."create", access (0:read/write)=enum16{"read/write", "read-only", "write-only"}."write-only") -> (refnum out=w3197:refnum<file>)  [unwired: 1 in, 4 out]
            n1926 = local write "Saving..."(TRUE ("Saving...")) -> ()
            n1927 = To Double Precision Float(number=w3184) -> (double precision float=w3182:dbl)
            n1928 = String Length(string="Comment (data description)") -> (length=w3180:i32)
            n1929 = To Double Precision Float(number=w3180) -> (double precision float=w3179:dbl)
            n1930 = Deny Access(7:w3197) -> (3:w3196:refnum<file>)  [unwired: 1 in, 2 out]
            n1931 = Build Array (concatenate)(w3182, w3183, w3179) -> (w3181:dbl[])
            n1932 = case "If fluorescence data to be saved" shown="True" w3170 {
              tunnel: w3159 -> [_ w3249]
              tunnel: [refnum<k0> refnum w3229] -> w3171
              frame False {
              }
              frame True {
                w3228 = 0.0
                n1933 = local read "APD Integration Time (s)"() -> (w3234:dbl)
                n1934 = local read "N APD Samp/step"() -> (w3227:dbl)
                n1935 = Path To String(path=w3249) -> (string=w3248:string)
                n1936 = String Length(string=w3248) -> (length=w3247:i32)
                n1937 = Subtract(x=w3247, y=4) -> (x-y=w3245:i32)
                n1938 = String Subset(string=w3248, length (rest)=w3245) -> (substring=w3244:string)  [unwired: 1 out]
                n1939 = Build Array(w3234, w3227, w3228, w3228, w3228, w3228, w3228, w3228) -> (w3231:dbl[])
                n1940 = Concatenate Strings(w3244, "_fl.dat" ("string")) -> (w3242:string)
                n1941 = Array Size(array=w3231) -> (size(s)=w3233:i32)
                n1942 = String To Path(string=w3242) -> (path=w3238:path)
                n1943 = Open/Create/Replace File(file path (use dialog)=w3238, operation (0:open)=T23."create", access (0:read/write)=enum16{"read/write", "read-only", "write-only"}."write-only") -> (refnum out=w3239:refnum<file>)  [unwired: 1 in, 4 out]
                n1944 = Deny Access(7:w3239) -> (3:w3235:refnum<file>)  [unwired: 1 in, 2 out]
                n1945 = To Double Precision Float(number=w3233) -> (double precision float=w3232:dbl)
                n1946 = Build Array (concatenate)(w3232, w3231) -> (w3230:dbl[])
                n1947 = Write to Binary File(file (use dialog)=w3235, data=w3230, 5:FALSE ("prepend array or string size? (T)"), 9:T29."big-endian, network order" ("byte order (0:big-endian, network order)")) -> (refnum out=w3229:refnum<file>)  [unwired: 1 in, 3 out]
              }
            }
            n1948 = case shown="True" w3157 {
              tunnel: w3159 -> [_ w3211]
              tunnel: [refnum<k0> refnum w3210] -> w3158
              frame False {
              }
              frame True {
                w3206 = 0.0 ("element")
                n1949 = Path To String(path=w3211) -> (string=w3225:string)
                n1950 = Build Array(w3206, w3206, w3206, w3206, w3206, w3206, w3206, w3206) -> (w3207:dbl[])
                n1951 = String Length(string=w3225) -> (length=w3224:i32)
                n1952 = Subtract(x=w3224, y=4) -> (x-y=w3222:i32)
                n1953 = Array Size(array=w3207) -> (size(s)=w3209:i32)
                n1954 = String Subset(string=w3225, length (rest)=w3222) -> (substring=w3221:string)  [unwired: 1 out]
                n1955 = To Double Precision Float(number=w3209) -> (double precision float=w3208:dbl)
                n1956 = Concatenate Strings(w3221, "_pos.dat" ("string")) -> (w3219:string)
                n1957 = Build Array (concatenate)(w3208, w3207) -> (w3205:dbl[])
                n1958 = String To Path(string=w3219) -> (path=w3215:path)
                n1959 = Open/Create/Replace File(file path (use dialog)=w3215, operation (0:open)=T23."create", access (0:read/write)=enum16{"read/write", "read-only", "write-only"}."write-only") -> (refnum out=w3216:refnum<file>)  [unwired: 1 in, 4 out]
                n1960 = Deny Access(7:w3216) -> (3:w3212:refnum<file>)  [unwired: 1 in, 2 out]
                n1961 = Write to Binary File(file (use dialog)=w3212, data=w3205, 5:FALSE ("prepend array or string size? (T)"), 9:T29."big-endian, network order" ("byte order (0:big-endian, network order)")) -> (refnum out=w3210:refnum<file>)  [unwired: 1 in, 3 out]
              }
            }
            n1962 = Write to Binary File(file (use dialog)=w3196, data=w3181, 5:w3177, 9:w3175) -> (refnum out=w3178:refnum<file>)  [unwired: 1 in, 3 out]
            n1963 = Write to Binary File(file (use dialog)=w3178, data="Comment (data description)", 5:w3177, 9:w3175) -> (refnum out=w3174:refnum<file>)  [unwired: 1 in, 3 out]
          }
        }
        n1964 = feedback-in #19(w3117) -> ()
        n1965 = feedback-in #20(w3144) -> ()
        n1966 = feedback-in #21(w3116) -> ()
        n1967 = feedback-in #22(w3127) -> ()
        n1968 = feedback-in #23(w3130) -> ()
        n1969 = feedback-in #24(w3143) -> ()
        n1970 = feedback-in #25(w3133) -> ()
      }
      frame #1 {
        n1971 = local read "Saving..."() -> (w3374:bool)
        n1972 = case shown="True" w3374 {
          tunnel: w3378 -> [_ w3388]
          tunnel: w3377 -> [_ w3402]
          tunnel: w3376 -> [_ w3398]
          tunnel: w3375 -> [_ w3397]
          tunnel: w3373 -> [_ w3396]
          tunnel: w3372 -> [_ w3391]
          tunnel: w3371 -> [_ w3390]
          tunnel: w3370 -> [_ w3389]
          tunnel: w3369 -> [_ w3387]
          tunnel: w3368 -> [_ w3385]
          tunnel: w3367 -> [_ w3384]
          tunnel: w3366 -> [_ w3383]
          tunnel: w3365 -> [_ w3382]
          tunnel: w3364 -> [_ w3381]
          tunnel: w3363 -> [_ w3380]
          tunnel: w3362 -> [_ w3379]
          frame False {
          }
          frame True {
            n1973 = Multiply(x=w3388, y=w3387) -> (x*y=→"Time (s)":dbl)
            n1974 = Less Or Equal?(x=w3388, y=w3396) -> (x <= y?=w3400:bool)
            n1975 = Or(x="Stop Saving", y="Abort save 2") -> (x .or. y?=w3392:bool)
            n1976 = Not(x=w3392) -> (.not. x?=w3401:bool)
            n1977 = And(x=w3400, y=w3401) -> (x .and. y?=w3399:bool)
            n1978 = case shown="False" w3399 {
              tunnel: w3402 -> [w3409 w3477]
              tunnel: [0.0 w3480] -> w3395
              tunnel: w3388 -> [_ w3478]
              tunnel: w3396 -> [_ w3479]
              tunnel: w3398 -> [_ w3474]
              tunnel: w3397 -> [_ _]
              tunnel: w3391 -> [w3407 w3467]
              tunnel: w3390 -> [w3406 w3468]
              tunnel: w3389 -> [_ w3466]
              tunnel: w3385 -> [_ w3465]
              tunnel: w3384 -> [_ w3419]
              tunnel: w3383 -> [_ w3458]
              tunnel: w3382 -> [_ w3436]
              tunnel: w3381 -> [w3404 w3417]
              tunnel: w3380 -> [w3405 w3416]
              tunnel: w3379 -> [_ w3413]
              frame False {
                w3403 = FALSE
                n1979 = Close File(refnum=w3409) -> ()  [unwired: 1 in, 2 out]
                n1980 = case shown="True" w3406 {
                  tunnel: w3407 -> [_ w3411]
                  frame False {
                  }
                  frame True {
                    n1981 = Close File(refnum=w3411) -> ()  [unwired: 1 in, 2 out]
                  }
                }
                n1982 = case shown="True" w3404 {
                  tunnel: w3405 -> [_ w3410]
                  frame False {
                  }
                  frame True {
                    n1983 = Close File(refnum=w3410) -> ()  [unwired: 1 in, 2 out]
                  }
                }
                n1984 = local write "Calibrating Trap..."(w3403) -> ()
                n1985 = call <vilib>:"Beep.vi"() -> ()  [unwired: 3 in, 9 out]
                n1986 = local write "Stop Saving"(w3403) -> ()
                n1987 = property on="Raster Scanning..." class="Bool (strict)"("Val(Sgnl)"=w3403) -> ()  [unwired: 2 in, 2 out]
                "Saving..." <- w3403
              }
              frame True {
                n1988 = local read "Calibrating Trap..."() -> (w3469:bool)
                n1989 = case "Write fl. data" shown="True" w3468 {
                  tunnel: w3467 -> [_ w3503]
                  tunnel: w3466 -> [_ w3502]
                  frame False {
                  }
                  frame True {
                    n1990 = Write to Binary File(file (use dialog)=w3503, data=w3502, 5:FALSE ("prepend array or string size? (T)"), 9:T29."big-endian, network order" ("byte order (0:big-endian, network order)")) -> ()  [unwired: 1 in, 4 out]
                  }
                }
                n1991 = Greater?(x="Save ave N", y=1.0) -> (0:w3472:bool)
                n1992 = Not(x=w3469) -> (.not. x?=w3471:bool)
                n1993 = And(x=w3471, y=w3472) -> (x .and. y?=w3414:bool)
                n1994 = case shown="True" w3414 {
                  tunnel: w3413 -> [w3483 w3494]
                  tunnel: [w3483 w3486] -> w3412
                  tunnel: "Save ave N" -> [_ w3487]
                  frame False {
                  }
                  frame True {
                    w3484 = 2 ("dimension size")
                    n1995 = Array Size(array=w3494) -> (size(s)=w3488:i32)
                    n1996 = Divide(x=w3488, y=w3484) -> (x/y=w3492:dbl)
                    n1997 = Reshape Array(w3494, w3492, w3484) -> (w3493:u64[][])
                    n1998 = Transpose 2D Array(2D array=w3493) -> (transposed array=w3491:u64[][])
                    n1999 = for {
                      tunnel: w3491 -> [w3496] mode=indexing
                      tunnel: [w3495] -> w3485 mode=indexing
                      tunnel: w3487 -> [w3497]
                      workers-P: _ -> [_]
                      n2000 = call "downsample 1D array - U64.vi"("Ave N"=w3497, "Array In"=w3496) -> ("Array Out"=w3495:u64[])  [unwired: 1 in]
                    }
                    n2001 = Transpose 2D Array(2D array=w3485) -> (transposed array=w3490:u64[][])
                    n2002 = Divide(x=w3488, y=w3487) -> (x/y=w3489:dbl)
                    n2003 = Reshape Array(w3490, w3489) -> (w3486:u64[])
                  }
                }
                n2004 = case shown="True" w3414 {
                  tunnel: w3474 -> [w3506 w3518]
                  tunnel: [w3506 w3510] -> w3470
                  tunnel: "Save ave N" -> [_ w3511]
                  tunnel: w3465 -> [_ w3509]
                  frame False {
                    # "don't downsample data for trap calibration"
                  }
                  frame True {
                    n2005 = Array Size(array=w3518) -> (size(s)=w3512:i32)
                    n2006 = Array Size(array=w3509) -> (size(s)=w3508:i32)
                    n2007 = Divide(x=w3512, y=w3508) -> (x/y=w3516:dbl)
                    n2008 = Reshape Array(w3518, w3516, w3508) -> (w3517:i16[][])
                    n2009 = Transpose 2D Array(2D array=w3517) -> (transposed array=w3515:i16[][])
                    n2010 = for {
                      tunnel: w3515 -> [w3521] mode=indexing
                      tunnel: [w3520] -> w3507 mode=indexing
                      tunnel: w3511 -> [w3519]
                      workers-P: _ -> [_]
                      n2011 = call "downsample 1D array - I16.vi"("Ave N"=w3519, "Array In"=w3521) -> ("Array Out"=w3520:i16[])  [unwired: 1 out]
                    }
                    n2012 = Transpose 2D Array(2D array=w3507) -> (transposed array=w3514:i16[][])
                    n2013 = Divide(x=w3512, y=w3511) -> (x/y=w3513:dbl)
                    n2014 = Reshape Array(w3514, w3513) -> (w3510:i16[])
                  }
                }
                n2015 = Index Array(array=w3436, index=1) -> (element=w3439:waveform(dbl))
                n2016 = Index Array(array=w3436, index=0) -> (element=w3441:waveform(dbl))
                n2017 = Unbundle By Name(w3439) -> ("Y"=w3443:dbl[])
                n2018 = Unbundle By Name(w3441) -> ("Y"=w3451:dbl[])
                n2019 = case "Write trap pos. data" shown="True" w3417 {
                  tunnel: w3416 -> [_ w3499]
                  tunnel: w3412 -> [_ w3498]
                  frame False {
                  }
                  frame True {
                    n2020 = Write to Binary File(file (use dialog)=w3499, data=w3498, 5:FALSE ("prepend array or string size? (T)"), 9:T29."big-endian, network order" ("byte order (0:big-endian, network order)")) -> ()  [unwired: 1 in, 4 out]
                  }
                }
                n2021 = Write to Binary File(file (use dialog)=w3477, data=w3470, 5:FALSE ("prepend array or string size? (T)"), 9:T29."big-endian, network order" ("byte order (0:big-endian, network order)")) -> ()  [unwired: 1 in, 4 out]
                n2022 = feedback #26(w3443) -> (w3445:dbl[])
                n2023 = Build Array (concatenate)(w3445, w3443) -> (w3444:dbl[])
                n2024 = Select(t=w3443, s=w3419, f=w3444) -> (s? t:f=w3429:dbl[])
                n2025 = feedback-in #26(w3429) -> ()
                n2026 = feedback #27(w3451) -> (w3464:dbl[])
                n2027 = Build Array (concatenate)(w3464, w3451) -> (w3463:dbl[])
                n2028 = Select(t=w3451, s=w3419, f=w3463) -> (s? t:f=w3438:dbl[])
                n2029 = feedback-in #27(w3438) -> ()
                n2030 = Divide(x=w3478, y=w3479) -> (x/y=w3481:dbl)
                n2031 = Multiply(x=w3481, y=100.0) -> (x*y=w3480:dbl)
                n2032 = Build Array(w3438, w3429) -> (→"Saved APD":dbl[][])
                n2033 = Array Size(array=w3438) -> (size(s)=w3456:i32)
                n2034 = Unbundle By Name(w3458) -> ("Y"=w3462:dbl[])
                n2035 = Subtract(x=w3456, y="N pts to average") -> (x-y=w3432:i32)
                n2036 = Multiply(x="N pts to average", y=u16 2) -> (x*y=w3433:u16)
                n2037 = Subtract(x=w3456, y=w3433) -> (x-y=w3431:i32)
                n2038 = feedback #28(w3462) -> (w3461:dbl[])
                n2039 = Build Array (concatenate)(w3461, w3462) -> (w3460:dbl[])
                n2040 = Select(t=w3462, s=w3419, f=w3460) -> (s? t:f=w3459:dbl[])
                "Trap Delta Graph" <- w3459
                n2041 = feedback-in #28(w3459) -> ()
                n2042 = Array Subset(array=w3438, index=w3432, length="N pts to average") -> (w3455:dbl[])
                n2043 = Array Subset(array=w3438, index=w3431, length="N pts to average") -> (w3454:dbl[])
                n2044 = Array Subset(array=w3429, index=w3432, length="N pts to average") -> (w3435:dbl[])
                n2045 = Array Subset(array=w3429, index=w3431, length="N pts to average") -> (w3434:dbl[])
                n2046 = call-poly <vilib>:"Mean.vi"("X"=w3455) -> ("mean"=w3453:dbl)  [unwired: 1 out]
                n2047 = call-poly <vilib>:"Mean.vi"("X"=w3435) -> ("mean"=w3428:dbl)  [unwired: 1 out]
                n2048 = call-poly <vilib>:"Mean.vi"("X"=w3454) -> ("mean"=w3452:dbl)  [unwired: 1 out]
                n2049 = call-poly <vilib>:"Mean.vi"("X"=w3434) -> ("mean"=w3427:dbl)  [unwired: 1 out]
                n2050 = Subtract(x=w3428, y=w3427) -> (x-y=w3418:dbl)
                "Delta Fl. 2" <- w3418
                n2051 = Subtract(x=w3453, y=w3452) -> (x-y=w3450:dbl)
                "Delta Fl. 1" <- w3450
                n2052 = Initialize Array(w3450, 1 ("dimension size")) -> (w3447:dbl[])
                n2053 = Initialize Array(w3418, 1 ("dimension size")) -> (w3424:dbl[])
                n2054 = feedback #29(w3447) -> (w3448:dbl[])
                n2055 = Build Array (concatenate)(w3448, w3447) -> (w3446:dbl[])
                n2056 = feedback #30(w3424) -> (w3425:dbl[])
                n2057 = Build Array (concatenate)(w3425, w3424) -> (w3423:dbl[])
                n2058 = Select(t=w3447, s=w3419, f=w3446) -> (s? t:f=w3422:dbl[])
                n2059 = feedback-in #29(w3422) -> ()
                n2060 = Select(t=w3424, s=w3419, f=w3423) -> (s? t:f=w3421:dbl[])
                n2061 = feedback-in #30(w3421) -> ()
                n2062 = Build Array(w3422, w3421) -> (→"Save APD Deriv":dbl[][])
              }
            }
            "Progress" <- w3395
            "Progress 2" <- w3395
          }
        }
      }
    }
    n2063 = Bundle By Name(cluster=w2139, "Green FB Ch 0"=w2138, "Green FB Ch 1"=w2137) -> (w2117:T48)
    "Green FB Signals (V)" <- w2117
    n2064 = Unbundle By Name(w2117) -> ("Green FB Ch 2"=→"Green FB Plot":dbl)
    n2065 = local read "wait to reset values"() -> (w2209:bool)
    n2066 = Not(x=w2206) -> (.not. x?=w2210:bool)
    n2067 = And(x=w2210, y=w2209) -> (x .and. y?=w2211:bool)
    n2068 = case "Part of MCL raster scanning: returns to initial positions after scan done" shown="False" w2211 {
      tunnel: w2214 -> [w2947 w2954]
      tunnel: [w2947 w2953] -> w2213
      tunnel: w2208 -> [w2946 w2952]
      tunnel: [w2946 w2951] -> w2207
      frame False {
      }
      frame True {
        w2962 = 10.0 ("y")
        w2961 = 32767.0 ("y")
        # "to return scan values\nafter a synchronous \nAOM scan"
        n2069 = local read "AO2"() -> (w2955:dbl)
        n2070 = local read "AO1"() -> (w2956:dbl)
        n2071 = local write "wait to reset values"(FALSE ("wait to reset values")) -> ()
        n2072 = Multiply(x=w2956, y=w2961) -> (x*y=w2958:dbl)
        n2073 = Multiply(x=w2955, y=w2961) -> (x*y=w2960:dbl)
        n2074 = Divide(x=w2958, y=w2962) -> (x/y=w2957:dbl)
        n2075 = Divide(x=w2960, y=w2962) -> (x/y=w2959:dbl)
        n2076 = To Word Integer(number=w2957) -> (16bit integer=w2963:i16)
        n2077 = To Word Integer(number=w2959) -> (16bit integer=w2964:i16)
        n2078 = local read "Total Counts (ticks)"() -> (w2948:u32)
        n2079 = xnode "Read/Write Control"("FPGA VI Reference In"=w2954, "error in"=w2952, "AO1"=w2963, "AO2"=w2964, "MCL count"=w2948) -> ("FPGA VI Reference Out"=w2953:T19, "error out"=w2951:errorcluster)
        n2080 = local read "Scan Range (V)\n(of steps)"() -> (w2949:dbl)
        n2081 = property on="Scan Range (V)\n(of steps)" class="DigNum (strict)"("Val(Sgnl)"=w2949) -> ()  [unwired: 2 in, 2 out]
      }
    }
    n2082 = node-c288() -> ()  [unwired: 2 out]
  }
  n2083 = node-c288(3 ("Processor")) -> (w74:T24)  [unwired: 3 out]
  n2084 = timed-loop "Oscillate AOD (debugging)" {
    tunnel: w24 -> [w3523]
    tunnel: [w3522] -> w36
    timing: w74 -> [_]
    timing-out: [_] -> w73
    stop <- w3522 stop-if-true
    n2085 = node-c288() -> ()  [unwired: 2 out]
    n2086 = event shown="[0] \"Oscillate Set 2\", \"Fish for Tether\": Value Change" {
      selector: _ -> [_ _ _]
      dyn-events: _ -> [_ _ _]
      timeout: _ -> [_ _ _]
      tunnel: w3523 -> [w3530 _ _]
      tunnel: [FALSE ("Stop All") _ w3798] -> w3522
      event "Oscillate Set 2", "Fish for Tether": Value Change {
        n2087 = event-data() -> ()  [unwired: 6 out]
        n2088 = local read "Oscillate Set 2"() -> (w3529:bool)
        n2089 = Or(x=w3529, y="Fish for Tether") -> (x .or. y?=w3527:bool)
        n2090 = case shown="True" w3527 {
          tunnel: w3530 -> [_ w3533]
          tunnel: "Fish for Tether" -> [_ w3532]
          frame False {
          }
          frame True {
            n2091 = case shown="True" w3532 {
              frame False {
              }
              frame True {
                n2092 = local write "Scan axis 2"(TRUE) -> ()
                n2093 = local write "Tether"(FALSE ("Tether")) -> ()
              }
            }
            n2094 = node-c288("Period") -> (w3535:T24)  [unwired: 3 out]
            n2095 = timed-loop "Oscillate AOD" {
              timing: w3535 -> [_]
              timing-out: [_] -> w3534
              tunnel: w3533 -> [w3545]
              tunnel: w3532 -> [w3544]
              i -> [w3547]
              stop <- w3543 stop-if-true
              n2096 = node-c288() -> (w3546:i64)  [unwired: 1 out]
              n2097 = flat-sequence {
                tunnel: w3547 -> [w3573]
                tunnel: w3546 -> [w3572]
                tunnel: w3545 -> [w3556]
                tunnel: w3544 -> [w3558]
                tunnel: [w3558] -> w3542
                tunnel: [w3557] -> w3541
                tunnel: [w3555] -> w3540
                tunnel: [w3552] -> w3538
                tunnel: w3542 -> [w3609]
                tunnel: w3541 -> [w3607]
                tunnel: w3540 -> [w3606]
                tunnel: [w3605] -> w3539
                tunnel: w3538 -> [w3604]
                tunnel: [w3673] -> w3543
                tunnel: w3539 -> [w3671]
                frame #0 {
                  n2098 = Divide(x=w3572, y=i64 1000) -> (x/y=w3567:dbl)
                  n2099 = Multiply(x=w3567, y=w3573) -> (x*y=w3569:dbl)
                  n2100 = Multiply(x="Osc. freq. (Hz)", y=6.283185307179586) -> (x*y=w3570:dbl)
                  n2101 = Multiply(x=w3570, y=w3569) -> (x*y=w3554:dbl)
                  n2102 = local read "BD 1 Frequency 2 (MHz)"() -> (w3551:dbl)
                  n2103 = local read "BD 1 Frequency 1 (MHz)"() -> (w3548:dbl)
                  n2104 = case shown="True" w3558 {
                    tunnel: w3554 -> [w3579 w3586]
                    tunnel: w3551 -> [_ w3596]
                    tunnel: [w3576 w3580] -> w3559
                    tunnel: [FALSE w3589] -> w3555
                    tunnel: [0.0 w3582] -> w3552
                    tunnel: w3548 -> [_ w3581]
                    frame False {
                      n2105 = Sine(x=w3579) -> (sin(x)=w3577:dbl)
                      n2106 = Multiply(x=w3577, y="Osc. amp. (MHz)") -> (x*y=w3576:dbl)
                    }
                    frame True {
                      n2107 = Cosine(x=w3586) -> (cos(x)=w3599:dbl)
                      n2108 = Subtract(x=w3596, y=w3581) -> (x-y=w3595:dbl)
                      n2109 = Decrement(x=w3599) -> (x-1=w3598:dbl)
                      n2110 = Subtract(x=w3595, y="Closest Delta (MHz)") -> (x-y=w3592:dbl)
                      n2111 = Divide(x=w3598, y=2.0) -> (x/y=w3593:dbl)
                      n2112 = Multiply(x=w3593, y=w3592) -> (x*y=w3580:dbl)
                      n2113 = local read "Vec Mean of T1 T2"() -> (w3588:dbl[])
                      n2114 = Greater?(x=w3588, y="Stop F (pN)") -> (0:w3590:bool[])
                      n2115 = Or Array Elements(Boolean array=w3590) -> (logical OR=w3589:bool)
                      n2116 = Divide(x=w3586, y=6.283185307179586) -> (x/y=w3585:dbl)
                      n2117 = Round Toward +Infinity(x=w3585) -> (ceil(x): smallest int >= x=w3582:dbl)
                      "Attempts" <- w3582
                      n2118 = Greater?(x=w3582, y="Attempt Limit") -> (0:w3584:bool)
                      n2119 = case shown="True" w3584 {
                        frame False {
                        }
                        frame True {
                          n2120 = local write "Fish for Tether"(FALSE ("Fish for Tether")) -> ()
                          n2121 = call <vilib>:"Beep.vi"() -> ()  [unwired: 3 in, 9 out]
                          n2122 = local read "Messages"() -> (w3601:string)
                          n2123 = call "Update messages.vi"("Message to add"="Tether fishing timeout." ("Messages"), "Old message string"=w3601) -> ("New message string"=→"Messages":string)
                        }
                      }
                    }
                  }
                  n2124 = local read "Y RF Frequency Limits (MHz)"() -> (w3560:T16)
                  n2125 = local read "X RF Frequency Limits (MHz)"() -> (w3561:T16)
                  n2126 = local read "BD 1 Frequency 3 (MHz)"() -> (w3566:dbl)
                  n2127 = local read "BD 2 Frequency 2 (MHz)"() -> (w3550:dbl)
                  n2128 = Select(t=w3551, s="Scan axis 2", f=w3550) -> (s? t:f=w3562:dbl)
                  n2129 = Add(x=w3559, y=w3562) -> (x+y=w3557:dbl)
                  n2130 = Select(t=w3557, s="Scan axis 2", f=w3551) -> (s? t:f=w3549:dbl)
                  n2131 = Select(t=w3550, s="Scan axis 2", f=w3557) -> (s? t:f=w3564:dbl)
                  n2132 = local read "BD 2 Frequency 3 (MHz)"() -> (w3565:dbl)
                  n2133 = call "set RF board frequency - interlace.vi"("Board 2 Frequency Limits"=w3560, "Board 1 Frequency Limits"=w3561, "FPGA VI Reference In"=w3556, "Board 2 Frequency 3 (MHz)"=w3565, "Board 1 Frequency 3 (MHz)"=w3566, "Board 2 Frequency 2 (MHz)"=w3550, "Board 2 Frequency 1 (MHz)"=w3564, "Board 1 Frequency 2 (MHz)"=w3549, "Board 1 Frequency 1  (MHz)"=w3548) -> ()  [unwired: 1 in, 2 out]
                }
                frame #1 {
                  n2134 = And(x=w3609, y=w3606) -> (x .and. y?=w3608:bool)
                  n2135 = case "Only if were fishing and now formed tether" shown="True" w3608 {
                    tunnel: w3607 -> [w3611 w3623]
                    tunnel: [w3610 w3622] -> w3605
                    tunnel: w3604 -> [_ w3618]
                    frame False {
                      n2136 = local read "Fish for Tether"() -> (w3610:bool)
                      n2137 = case shown="True" w3610 {
                        tunnel: w3611 -> [_ _]
                        frame False {
                        }
                        frame True {
                        }
                      }
                    }
                    frame True {
                      w3622 = FALSE ("Fish for Tether")
                      n2138 = call <vilib>:"Beep.vi"() -> ()  [unwired: 3 in, 9 out]
                      n2139 = Number To Decimal String(number=w3618, width (-)=i16 1) -> (decimal integer string=w3616:string)
                      n2140 = case shown="\"2\", \"3\", \"4\", \"5\", \"6\"" "Then..." {
                        selector: "Then..." -> [_ w3626]
                        tunnel: w3623 -> [w3625 _]
                        frame "1", Default {
                          # "do nothing"
                          n2141 = property on="BD 1 Frequency 1 (MHz)" class="DigNum (strict)"("Val(Sgnl)"=w3625) -> ()  [unwired: 2 in, 2 out]
                        }
                        frame "2", "3", "4", "5", "6" {
                          n2142 = flat-sequence {
                            tunnel: w3626 -> [w3628]
                            frame #0 {
                              n2143 = property on="Trap Delta (MHz)" class="DigNum (strict)"("Val(Sgnl)"="Move to Delta 1 (MHz)") -> ()  [unwired: 2 in, 2 out]
                            }
                            frame #1 {
                              n2144 = case shown="\"5\", \"6\"" w3628 {
                                selector: w3628 -> [w3631 w3641 _]
                                frame "3", "4" {
                                n2145 = flat-sequence {
                                tunnel: w3631 -> [w3632]
                                tunnel: [w3632] -> w3629
                                tunnel: [w3634] -> w3630
                                tunnel: w3629 -> [w3634]
                                tunnel: w3630 -> [w3638]
                                frame #0 {
                                n2146 = property on="Green Laser ON/Interlacing" class="Bool (strict)"("Val(Sgnl)"=TRUE ("Value (Signaling)")) -> ()  [unwired: 2 in, 2 out]
                                }
                                frame #1 {
                                n2147 = Multiply(x="Wait Before Save (s)", y=u32 1000 ("x")) -> (x*y=w3636:u32)
                                n2148 = Wait (ms)(milliseconds to wait=w3636) -> ()  [unwired: 1 out]
                                }
                                frame #2 {
                                n2149 = property on="Start Saving" class="Bool (strict)"("Value"=TRUE ("Start Saving")) -> ()  [unwired: 2 in, 2 out]
                                n2150 = case shown="Default" w3638 {
                                frame Default {
                                }
                                frame "4" {
                                n2151 = property on="Fl. Triggered..." class="Bool (strict)"("Val(Sgnl)"=TRUE ("Value (Signaling)")) -> ()  [unwired: 2 in, 2 out]
                                }
                                }
                                }
                                }
                                }
                                frame "5", "6" {
                                n2152 = stacked-sequence {
                                tunnel: w3641 -> [_ _ _ _ _ _ _ _ w3658 _ _]
                                frame #0 {
                                n2153 = Replace Array Subset(array=u32[] [0] ("Index Values"), new element="Raster Set Upon Tether", index=0) -> (w3642:u32[])
                                n2154 = property on="Saved AOD Raster Scan Parameter Sets" class="Arr (strict)"("Index Values"=w3642) -> ()  [unwired: 2 in, 2 out]
                                }
                                frame #1 {
                                n2155 = Wait (ms)(milliseconds to wait=u32 500) -> ()  [unwired: 1 out]
                                }
                                frame #2 {
                                n2156 = property on="Load parameters" class="Bool (strict)"("Val(Sgnl)"=TRUE ("Value (Signaling)")) -> ()  [unwired: 2 in, 2 out]
                                }
                                frame #3 {
                                n2157 = Wait (ms)(milliseconds to wait=u32 500) -> ()  [unwired: 1 out]
                                }
                                frame #4 {
                                n2158 = property on="Trap Raster Scan" class="Bool (strict)"("Val(Sgnl)"=TRUE ("Value (Signaling)")) -> ()  [unwired: 2 in, 2 out]
                                }
                                frame #5 {
                                n2159 = Wait (ms)(milliseconds to wait=u32 2000) -> ()  [unwired: 1 out]
                                }
                                frame #6 {
                                n2160 = while {
                                stop <- w3653 stop-if-true
                                n2161 = local read "Raster Scanning..."() -> (w3652:bool)
                                n2162 = local read "Saving..."() -> (w3655:bool)
                                n2163 = Wait (ms)(milliseconds to wait=u32 100) -> ()  [unwired: 1 out]
                                n2164 = Not(x=w3655) -> (.not. x?=w3654:bool)
                                n2165 = Not(x=w3652) -> (.not. x?=w3651:bool)
                                n2166 = And(x=w3654, y=w3651) -> (x .and. y?=w3653:bool)
                                }
                                }
                                frame #7 {
                                n2167 = property on="Trap Delta (MHz)" class="DigNum (strict)"("Val(Sgnl)"="Move to Delta 2 (MHz)") -> ()  [unwired: 2 in, 2 out]
                                }
                                frame #8 {
                                n2168 = local read "Tether"() -> (w3659:bool)
                                n2169 = case shown="True" w3659 {
                                tunnel: w3658 -> [_ w3660]
                                frame False {
                                }
                                frame True {
                                n2170 = flat-sequence {
                                tunnel: w3660 -> [w3662]
                                frame #0 {
                                n2171 = Wait (ms)(milliseconds to wait=u32 500) -> ()  [unwired: 1 out]
                                }
                                frame #1 {
                                n2172 = case shown="\"6\"" w3662 {
                                frame Default {
                                }
                                frame "6" {
                                n2173 = property on="Green Laser ON/Interlacing" class="Bool (strict)"("Val(Sgnl)"=TRUE ("Green Laser ON/Interlacing")) -> ()  [unwired: 2 in, 2 out]
                                }
                                }
                                }
                                frame #2 {
                                n2174 = Wait (ms)(milliseconds to wait=u32 500) -> ()  [unwired: 1 out]
                                }
                                frame #3 {
                                n2175 = local write "Start Saving"("Save at end (5, 6)") -> ()
                                }
                                }
                                }
                                }
                                }
                                frame #9 {
                                n2176 = local read "Bead Sep. Int. Time (s)"() -> (w3668:dbl)
                                n2177 = Multiply(x=w3668, y=1000.0) -> (x*y=w3667:dbl)
                                n2178 = Wait (ms)(milliseconds to wait=w3667) -> ()  [unwired: 1 out]
                                }
                                frame #10 {
                                n2179 = property on="Rescale on Mean" class="Bool (strict)"("Val(Sgnl)"=TRUE ("Value (Signaling)")) -> ()  [unwired: 2 in, 2 out]
                                }
                                }
                                }
                                frame "2", Default {
                                }
                              }
                            }
                          }
                        }
                      }
                      n2180 = Concatenate Strings("Formed tether in ", w3616, " attempt(s)." ("string")) -> (w3613:string)
                      n2181 = local read "Messages"() -> (w3620:string)
                      n2182 = local write "Fish for Tether"(w3622) -> ()
                      n2183 = call "Update messages.vi"("Message to add"=w3613, "Old message string"=w3620) -> ("New message string"=w3619:string)
                      n2184 = local write "Messages"(w3619) -> ()
                      n2185 = Get Date/Time In Seconds() -> (seconds since 1Jan1904=→"Time tether formed":timestamp)
                      "Tether" <- "Tether Alarm?"
                    }
                  }
                }
                frame #2 {
                  n2186 = local read "Oscillate Set 2"() -> (w3672:bool)
                  n2187 = local read "Stop All"() -> (w3674:bool)
                  n2188 = Not Or(1:w3671, 2:w3672) -> (0:w3670:bool)
                  n2189 = Compound Arithmetic op=OR(w3674, w3670) -> (w3673:bool)
                }
              }
              n2190 = node-c288() -> ()  [unwired: 2 out]
            }
            n2191 = node-c288(w3534) -> ()  [unwired: 1 out]
          }
        }
      }
      event "Fl. Triggered...": Value Change {
        n2192 = event-data() -> ()  [unwired: 7 out]
        n2193 = case shown="True" "Fl. Triggered..." {
          frame False {
          }
          frame True {
            n2194 = node-c288() -> (w3686:T24)  [unwired: 4 out]
            n2195 = timed-loop {
              timing: w3686 -> [_]
              timing-out: [_] -> w3685
              tunnel: "Action" -> [w3690]
              shift-right: [w3687] -> _
              shift-left: u8 255 -> [w3689]
              stop <- w3691 stop-if-true
              n2196 = node-c288() -> ()  [unwired: 2 out]
              n2197 = flat-sequence {
                tunnel: w3690 -> [w3703]
                tunnel: w3689 -> [w3700]
                tunnel: [w3699] -> w3688
                tunnel: [w3789] -> w3691
                tunnel: w3688 -> [w3788]
                tunnel: [w3788] -> w3687
                frame #0 {
                  n2198 = local read "Delta Fl. 2"() -> (w3694:dbl)
                  n2199 = local read "Delta Fl. 1"() -> (w3695:dbl)
                  n2200 = Select(t=w3695, s="APD to Watch", f=w3694) -> (s? t:f=w3693:dbl)
                  n2201 = Multiply(x="Fl. Delta Thresh. (kHz)", y=1000.0) -> (x*y=w3702:dbl)
                  n2202 = Greater?(x=w3693, y=w3702) -> (0:w3697:bool)
                  n2203 = Or(x="Force Yank", y=w3697) -> (x .or. y?=w3698:bool)
                  n2204 = case shown="True" w3698 {
                    tunnel: w3703 -> [_ w3713]
                    tunnel: w3700 -> [w3705 w3709]
                    tunnel: [w3705 w3706] -> w3699
                    frame False {
                    }
                    frame True {
                      n2205 = flat-sequence {
                        tunnel: w3710 -> [w3719]
                        tunnel: [w3719] -> w3714
                        tunnel: w3713 -> [w3718]
                        tunnel: [w3718] -> w3712
                        tunnel: [w3717] -> w3711
                        tunnel: w3709 -> [w3716]
                        tunnel: [w3715] -> w3708
                        tunnel: w3714 -> [w3744]
                        tunnel: w3712 -> [w3743]
                        tunnel: w3711 -> [w3742]
                        tunnel: w3708 -> [w3741]
                        tunnel: [w3741] -> w3707
                        tunnel: w3707 -> [w3786]
                        tunnel: [w3786] -> w3706
                        frame #0 {
                          n2206 = call <vilib>:"Beep.vi"() -> ()  [unwired: 3 in, 9 out]
                          n2207 = local write "Waiting"(FALSE ("Waiting")) -> ()
                          n2208 = Increment(x=w3716) -> (x+1=w3715:u8)
                          n2209 = case shown="\"Yank\"" w3718 {
                            tunnel: w3715 -> [_ _ w3725]
                            frame "Image" {
                              n2210 = property on="Confocal Image" class="Bool (strict)"("Val(Sgnl)"=TRUE ("Value (Signaling)")) -> ()  [unwired: 2 in, 2 out]
                            }
                            frame "Alarm", Default {
                            }
                            frame "Yank" {
                              n2211 = flat-sequence {
                                tunnel: w3725 -> [w3728]
                                tunnel: [w3727] -> w3724
                                tunnel: ["N Array El"] -> w3723
                                tunnel: w3724 -> [w3738]
                                tunnel: w3723 -> [w3734]
                                frame #0 {
                                n2212 = Multiply(x="Yank Delay (s)", y=1000.0) -> (x*y=w3731:dbl)
                                n2213 = Quotient & Remainder(x=w3728, y="N Array El") -> (x-y*floor(x/y)=w3727:u8)  [unwired: 1 out]
                                n2214 = Wait (ms)(milliseconds to wait=w3731) -> ()  [unwired: 1 out]
                                }
                                frame #1 {
                                n2215 = Random Number (0-1)() -> (number: 0 to 1=w3735:dbl)
                                n2216 = Multiply(x=w3734, y=w3735) -> (x*y=w3733:dbl)
                                n2217 = Round Toward -Infinity(1:w3733) -> (0:w3732:dbl)
                                n2218 = Select(t=w3732, s="Random Choice", f=w3738) -> (s? t:f=w3736:dbl)
                                n2219 = Index Array(array="Yank to Delta Array (MHz)", index=w3736) -> (element=w3739:dbl)
                                n2220 = property on="Trap Delta (MHz)" class="DigNum (strict)"("Val(Sgnl)"=w3739) -> ()  [unwired: 2 in, 2 out]
                                }
                              }
                            }
                          }
                          n2221 = local read "Time (s)"() -> (w3717:dbl)
                          "Fl. High" <- TRUE ("Yanking")
                        }
                        frame #1 {
                          n2222 = node-c288() -> (w3746:T24)  [unwired: 4 out]
                          n2223 = timed-loop {
                            timing: w3746 -> [_]
                            timing-out: [_] -> w3745
                            tunnel: w3744 -> [w3762]
                            tunnel: w3743 -> [w3760]
                            tunnel: w3742 -> [w3759]
                            stop <- w3761 stop-if-true
                            n2224 = node-c288() -> ()  [unwired: 2 out]
                            n2225 = local read "Fl. Delta Thresh. (kHz)"() -> (w3754:dbl)
                            n2226 = local read "Fl. Triggered..."() -> (w3763:bool)
                            n2227 = local read "Delta Fl. 1"() -> (w3750:dbl)
                            n2228 = local read "Delta Fl. 2"() -> (w3748:dbl)
                            n2229 = local read "Stop All"() -> (w3757:bool)
                            n2230 = local read "APD to Watch"() -> (w3749:bool)
                            n2231 = Select(t=w3750, s=w3749, f=w3748) -> (s? t:f=w3747:dbl)
                            n2232 = Not(x=w3763) -> (.not. x?=w3758:bool)
                            n2233 = Multiply(x=w3754, y=1000.0) -> (x*y=w3753:dbl)
                            n2234 = Negate(x=w3753) -> (-x=w3752:dbl)
                            n2235 = Less?(x=w3747, y=w3752) -> (x < y?=w3756:bool)
                            n2236 = Compound Arithmetic op=OR(w3756, w3757, w3758, "Force Reset") -> (w3761:bool)
                            n2237 = case shown="True" w3761 {
                              tunnel: w3762 -> [_ w3774]
                              tunnel: w3760 -> [_ w3773]
                              tunnel: w3759 -> [_ w3771]
                              frame False {
                              }
                              frame True {
                                n2238 = case shown="\"Yank\"" w3773 {
                                tunnel: w3774 -> [_ w3775]
                                frame "Image", Default {
                                }
                                frame "Yank" {
                                n2239 = flat-sequence {
                                tunnel: [w3780] -> w3776
                                tunnel: w3775 -> [w3780]
                                tunnel: w3776 -> [w3781]
                                frame #0 {
                                n2240 = local read "Yank Delay (s)"() -> (w3779:dbl)
                                n2241 = Multiply(x=w3779, y=1000.0) -> (x*y=w3777:dbl)
                                n2242 = Wait (ms)(milliseconds to wait=w3777) -> ()  [unwired: 1 out]
                                }
                                frame #1 {
                                n2243 = property on="Trap Delta (MHz)" class="DigNum (strict)"("Val(Sgnl)"=w3781) -> ()  [unwired: 2 in, 2 out]
                                }
                                }
                                }
                                }
                                n2244 = local read "Time (s)"() -> (w3772:dbl)
                                n2245 = Subtract(x=w3772, y=w3771) -> (x-y=w3768:dbl)
                                "Duration (s)" <- w3768
                                n2246 = Number To Decimal String(number=w3768, width (-)=i16 0) -> (decimal integer string=w3766:string)
                                n2247 = Concatenate Strings(w3766, " s fluorescence event." ("string")) -> (w3764:string)
                                n2248 = local read "Messages"() -> (w3770:string)
                                n2249 = call "Update messages.vi"("Message to add"=w3764, "Old message string"=w3770) -> ("New message string"=w3769:string)
                                n2250 = call <vilib>:"Beep.vi"() -> ()  [unwired: 3 in, 9 out]
                                n2251 = local write "Messages"(w3769) -> ()
                              }
                            }
                            n2252 = node-c288() -> ()  [unwired: 2 out]
                          }
                          n2253 = node-c288(w3745) -> ()  [unwired: 1 out]
                        }
                        frame #2 {
                          n2254 = local write "Fl. High"(FALSE ("Yanking")) -> ()
                        }
                      }
                      n2255 = local read "Trap Delta (MHz)"() -> (w3710:dbl)
                    }
                  }
                }
                frame #1 {
                  n2256 = local read "Stop All"() -> (w3792:bool)
                  n2257 = local read "Fl. Triggered..."() -> (w3790:bool)
                  n2258 = Not(x=w3790) -> (.not. x?=w3791:bool)
                  n2259 = Or(x=w3791, y=w3792) -> (x .or. y?=w3789:bool)
                  n2260 = Not(x=w3789) -> (.not. x?=→"Waiting":bool)
                }
              }
              n2261 = node-c288() -> ()  [unwired: 2 out]
            }
            n2262 = node-c288(w3685) -> ()  [unwired: 1 out]
          }
        }
      }
      event "Stop All": Value Change {
        n2263 = event-data() -> ()  [unwired: 7 out]
        n2264 = local read "Stop All"() -> (w3798:bool)
      }
    }
    n2265 = node-c288() -> ()  [unwired: 2 out]
  }
  n2266 = node-c288(w14) -> ()  [unwired: 1 out]
  n2267 = node-c288(w68) -> ()  [unwired: 1 out]
  n2268 = node-c288(w75) -> ()  [unwired: 1 out]
  n2269 = node-c288(w73) -> ()  [unwired: 1 out]
  n2270 = node-c288(w163) -> ()  [unwired: 1 out]
  n2271 = flat-sequence {
    tunnel: w33 -> [w3803]
    tunnel: [w3802] -> w39
    tunnel: [w3799] -> w38
    tunnel: w37 -> [_]
    tunnel: w36 -> [_]
    tunnel: w35 -> [_]
    tunnel: w34 -> [_]
    tunnel: w32 -> [w3800]
    tunnel: w39 -> [w3806]
    tunnel: w38 -> [w3805]
    frame #0 {
      w3801 = FALSE ("APD to FIFO")
      n2272 = xnode "Read/Write Control"("FPGA VI Reference In"=w3803, "error in"=w3800, "APD to FIFO"=w3801, "AI to FIFO"=w3801) -> ("FPGA VI Reference Out"=w3802:T19, "error out"=w3799:errorcluster)
    }
    frame #1 {
      n2273 = xnode "Invoke Method"("FPGA VI Reference In"=w3806, "error in"=w3805) -> ("FPGA VI Reference Out"=w3804:T19)  [unwired: 1 out]
      n2274 = xnode "Close FPGA VI Reference"("FPGA VI Reference In"=w3804) -> ()  [unwired: 1 in, 1 out]
    }
  }
